vi "PrefDialog.vi"(8 "error in (no error)":errorcluster, 11 "MyPluginsBase in":refnum<class "NHRGridSim.lvclass">) -> (0 "error out":errorcluster, 1 "Save As":bool, 2 "Changed":bool, 3 "MyPluginsBase out":refnum<class "NHRGridSim.lvclass">)   [LabVIEW 2018, in "AcPwrPlugins.lvlib" / "NHRGridSim.lvclass"]
doc: "This VI opens up the modal preference dialog window and allows a user to configure the properties with new values, or keep the existing values from the last time the function was called. The user can also save the new values to a new file name and new type name using the save as button."
uses:
  NHRGridSim.lvclass
  C:/Program Files (x86)/National Instruments/LabVIEW 2018/user.lib/NIST/BaseClasses/BasePlugin_class/BasePlugin.lvclass
  C:/Users/Public/Projects/ICDAS/NistPluggableModules/AcPwr/AcPwrPlugins/AcPwrBaseClass/AcPwrBase.lvclass
  Measurements.ctl
  TypeDefs/MeasurementType.ctl
  TypeDefs/NHRGrid_Modes.ctl
  TypeDefs/Device(s)Settings.ctl
  TypeDefs/NHRGrid_InstrumentCluster_Tabs.ctl
  TypeDefs/NHRGrid_Configure_Tabs.ctl
  TypeDefs/NHRGrid_Ranges_Tabs.ctl
  TypeDefs/NHRGrid_SafetyTrips_Tabs.ctl
  TypeDefs/NHRGrid_SlewRates_Tabs.ctl
  TypeDefs/NHRGrid_Phases_Tabs.ctl
  TypeDefs/NHRGrid_UpdateSettings.ctl
  <userlib>/NIST/BaseClasses/BasePlugin_class/BasePlugin.lvclass/BasePlugin.ctl
  AcPwrBaseClass/AcPwrBase.lvclass/AcPwrBase.ctl
  TypeDefs/NHRGrid_ModeAdjust_Tabs.ctl
  <userlib>/NIST/BaseClasses/BasePlugin_class/Accessors/Read PluginIniFilePath.vi
  AcPwrBaseClass/Accessors/Read BaseConfig.vi
  AcPwrBaseClass/Accessors/Read BaseMeasurements.vi
  <userlib>/NIST/BaseClasses/BasePlugin_class/Accessors/Write PluginIniFilePath.vi
  <vilib>/Utility/config.llb/NI_LVConfig.lvlib
panel:
  in  "ModeVal":u8
  in  "ChassisTxt":string
  in  "Update":bool
  in  "Device(s)Settings":T1={"MeasName"="", "Instr1"={"Name"="", "Vout (V)"=0.0, "VType"="", "FreqOut (Hz)"=60.0, "Aperture (cycles)"=1, "Synchronization"=0, "Ranges"={"Voltage (V)"=0, "Current (A)"=1}, "Safety Trips"={"Vmin (V)"=0.0, "Vmin Time (s)"=-1.0, "Vmax (V)"=0.0, "Vmax Time (s)"=-1.0, "Imax Source (A)"=0.0, "I Src Time (s)"=-1.0, "Imax Sink (A)"=0.0, "I Snk Time (s)"=-1.0, "Pmax Source (W)"=0.0, "P Src Time (s)"=-1.0, "Pmax Sink (W)"=0.0, "P Snk Time (s)"=-1.0, "Abs Volt Peak"=0.0, "Enable Vpk"=FALSE, "Abs Curr Peak"=0.0, "Enable Ipk"=FALSE}, "Slew Rates"={"Voltage (V/s)"=866030.0, "Current (A/s)"=100000.0, "Power (W/s)"=3000000.0, "Frequency (Hz/s)"=500.0, "Phase Angle (Deg/s)"=50000.0}, "Phases"={"A-Volts (V)"=0.0, "B-Volts (V)"=0.0, "C-Volts (V)"=0.0, "A-Change at..."=0, "B-Angle (Deg)"=240, "C-Angle (Deg)"=120, "B-Change at..."=0, "C-Change at..."=0, "AngleTxt"="", "A-Wave Shape"=0, "B-Wave Shape"=0, "C-Wave Shape"=0}}, "Instr2"={"Name"="", "Vout (V)"=0.0, "VType"="", "FreqOut (Hz)"=60.0, "Aperture (cycles)"=1, "Synchronization"=0, "Ranges"={"Voltage (V)"=0, "Current (A)"=1}, "Safety Trips"={"Vmin (V)"=0.0, "Vmin Time (s)"=-1.0, "Vmax (V)"=0.0, "Vmax Time (s)"=-1.0, "Imax Source (A)"=0.0, "I Src Time (s)"=-1.0, "Imax Sink (A)"=0.0, "I Snk Time (s)"=-1.0, "Pmax Source (W)"=0.0, "P Src Time (s)"=-1.0, "Pmax Sink (W)"=0.0, "P Snk Time (s)"=-1.0, "Abs Volt Peak"=0.0, "Enable Vpk"=FALSE, "Abs Curr Peak"=0.0, "Enable Ipk"=FALSE}, "Slew Rates"={"Voltage (V/s)"=866030.0, "Current (A/s)"=100000.0, "Power (W/s)"=3000000.0, "Frequency (Hz/s)"=500.0, "Phase Angle (Deg/s)"=50000.0}, "Phases"={"A-Volts (V)"=0.0, "B-Volts (V)"=0.0, "C-Volts (V)"=0.0, "A-Change at..."=0, "B-Angle (Deg)"=240, "C-Angle (Deg)"=120, "B-Change at..."=0, "C-Change at..."=0, "AngleTxt"="", "A-Wave Shape"=0, "B-Wave Shape"=0, "C-Wave Shape"=0}}, "Instr3"={"Name"="", "Vout (V)"=0.0, "VType"="", "FreqOut (Hz)"=60.0, "Aperture (cycles)"=1, "Synchronization"=0, "Ranges"={"Voltage (V)"=0, "Current (A)"=1}, "Safety Trips"={"Vmin (V)"=0.0, "Vmin Time (s)"=-1.0, "Vmax (V)"=0.0, "Vmax Time (s)"=-1.0, "Imax Source (A)"=0.0, "I Src Time (s)"=-1.0, "Imax Sink (A)"=0.0, "I Snk Time (s)"=-1.0, "Pmax Source (W)"=0.0, "P Src Time (s)"=-1.0, "Pmax Sink (W)"=0.0, "P Snk Time (s)"=-1.0, "Abs Volt Peak"=0.0, "Enable Vpk"=FALSE, "Abs Curr Peak"=0.0, "Enable Ipk"=FALSE}, "Slew Rates"={"Voltage (V/s)"=866030.0, "Current (A/s)"=100000.0, "Power (W/s)"=3000000.0, "Frequency (Hz/s)"=500.0, "Phase Angle (Deg/s)"=50000.0}, "Phases"={"A-Volts (V)"=0.0, "B-Volts (V)"=0.0, "C-Volts (V)"=0.0, "A-Change at..."=0, "B-Angle (Deg)"=240, "C-Angle (Deg)"=120, "B-Change at..."=0, "C-Change at..."=0, "AngleTxt"="", "A-Wave Shape"=0, "B-Wave Shape"=0, "C-Wave Shape"=0}}, "Handle"="", "Reset"=FALSE, "Mode"=0, "ID Query"=FALSE, "Connected"=FALSE, "Chassis"=1, "VRangeVals1"=[], "SyncList1"=[], "Wave1A"=[], "Wave1B"=[], "Wave1C"=[], "SyncList2"=[], "SyncList3"=[], "VRangeVals3"=[], "VRangeVals2"=[], "CRangeVals1"=[], "CRangeVals3"=[], "CRangeVals2"=[], "TabPages"=[], "Wave2A"=[], "Wave2B"=[], "Wave2C"=[], "Wave3A"=[], "Wave3B"=[], "Wave3C"=[], "EnableCtrls"=[[1, 0, 0, 0, 0, 0, 0, 0, 0, 0, 0, 0, 0, 0, 0, 0, 0, 0], [1, 0, 0, 0, 0, 0, 0, 0, 0, 0, 0, 0, 0, 0, 0, 0, 0, 0], [1, 0, 0, 0, 0, 0, 0, 0, 0, 0, 0, 0, 0, 0, 0, 0, 0, 0]]} {"Chassis" min=1 max=8 step=1; "Mode" items=["3-Phase AC"=0, "AC"=1, "DC"=2, "AC - AC"=7, "AC - DC"=8, "DC - AC"=11, "DC - DC"=12, "2-Phase AC - AC"=5, "2-Phase AC - DC"=6, "AC - AC - AC"=3, "DC - DC - DC"=4, "AC - AC - DC"=9, "AC - DC - DC"=10, "AC - DC - AC"=13, "DC - AC - AC"=14, "DC - AC - DC"=15]; "Instr3"."Phases"."C-Wave Shape" items=["Sine", "User1", "User2", "User3"]; "Instr3"."Phases"."B-Wave Shape" items=["Sine", "User1", "User2", "User3"]; "Instr3"."Phases"."A-Wave Shape" items=["Sine", "User1", "User2", "User3"]; "Instr3"."Phases"."C-Change at..." min=0 max=359; "Instr3"."Phases"."B-Change at..." min=0 max=359; "Instr3"."Phases"."A-Change at..." min=0 max=359; "Instr3"."Phases"."C-Angle (Deg)" min=0 max=359; "Instr3"."Phases"."B-Angle (Deg)" min=0 max=359; "Instr3"."Phases"."C-Volts (V)" min=0.0 max=606.0; "Instr3"."Phases"."B-Volts (V)" min=0.0 max=606.0; "Instr3"."Phases"."A-Volts (V)" min=0.0 max=606.0; "Instr3"."Slew Rates"."Phase Angle (Deg/s)" min=0.1 max=50000.0; "Instr3"."Slew Rates"."Frequency (Hz/s)" min=0.01 max=500.0; "Instr3"."Slew Rates"."Power (W/s)" min=2.0 max=8000000.0; "Instr3"."Slew Rates"."Current (A/s)" min=0.2 max=2400000.0; "Instr3"."Slew Rates"."Voltage (V/s)" min=0.01 max=2000000.0; "Instr3"."Safety Trips"."Abs Curr Peak" min=0.0; "Instr3"."Safety Trips"."Abs Volt Peak" min=0.0; "Instr3"."Safety Trips"."P Snk Time (s)" min=-1.0 max=3600.0; "Instr3"."Safety Trips"."Pmax Sink (W)" min=0.0 max=436000.0 format="%#_7g"; "Instr3"."Safety Trips"."P Src Time (s)" min=-1.0 max=3600.0; "Instr3"."Safety Trips"."Pmax Source (W)" min=0.0 max=436000.0 format="%#_7g"; "Instr3"."Safety Trips"."I Snk Time (s)" min=-1.0 max=3600.0; "Instr3"."Safety Trips"."Imax Sink (A)" min=0.0 max=720.0; "Instr3"."Safety Trips"."I Src Time (s)" min=-1.0 max=3600.0; "Instr3"."Safety Trips"."Imax Source (A)" min=0.0 max=720.0; "Instr3"."Safety Trips"."Vmax Time (s)" min=-1.0 max=3600.0; "Instr3"."Safety Trips"."Vmax (V)" min=0.0 max=606.0; "Instr3"."Safety Trips"."Vmin Time (s)" min=-1.0 max=3600.0; "Instr3"."Safety Trips"."Vmin (V)" min=0.0 max=606.0; "Instr3"."Ranges"."Current (A)" items=["6", "30"]; "Instr3"."Ranges"."Voltage (V)" items=["303", "606"]; "Instr3"."Synchronization" items=["Immediate", "Sync to Phase A"]; "Instr3"."Aperture (cycles)" min=0 max=64; "Instr3"."FreqOut (Hz)" min=30.0 max=880.0; "Instr3"."Vout (V)" min=0.0 max=606.0; "Instr2"."Phases"."C-Wave Shape" items=["Sine", "User1", "User2", "User3"]; "Instr2"."Phases"."B-Wave Shape" items=["Sine", "User1", "User2", "User3"]; "Instr2"."Phases"."A-Wave Shape" items=["Sine", "User1", "User2", "User3"]; "Instr2"."Phases"."C-Change at..." min=0 max=359; "Instr2"."Phases"."B-Change at..." min=0 max=359; "Instr2"."Phases"."A-Change at..." min=0 max=359; "Instr2"."Phases"."C-Angle (Deg)" min=0 max=359; "Instr2"."Phases"."B-Angle (Deg)" min=0 max=359; "Instr2"."Phases"."C-Volts (V)" min=0.0 max=606.0; "Instr2"."Phases"."B-Volts (V)" min=0.0 max=606.0; "Instr2"."Phases"."A-Volts (V)" min=0.0 max=606.0; "Instr2"."Slew Rates"."Phase Angle (Deg/s)" min=0.1 max=50000.0; "Instr2"."Slew Rates"."Frequency (Hz/s)" min=0.01 max=500.0; "Instr2"."Slew Rates"."Power (W/s)" min=2.0 max=8000000.0; "Instr2"."Slew Rates"."Current (A/s)" min=0.2 max=2400000.0; "Instr2"."Slew Rates"."Voltage (V/s)" min=0.01 max=2000000.0; "Instr2"."Safety Trips"."Abs Curr Peak" min=0.0; "Instr2"."Safety Trips"."Abs Volt Peak" min=0.0; "Instr2"."Safety Trips"."P Snk Time (s)" min=-1.0 max=3600.0; "Instr2"."Safety Trips"."Pmax Sink (W)" min=0.0 max=436000.0 format="%#_7g"; "Instr2"."Safety Trips"."P Src Time (s)" min=-1.0 max=3600.0; "Instr2"."Safety Trips"."Pmax Source (W)" min=0.0 max=436000.0 format="%#_7g"; "Instr2"."Safety Trips"."I Snk Time (s)" min=-1.0 max=3600.0; "Instr2"."Safety Trips"."Imax Sink (A)" min=0.0 max=720.0; "Instr2"."Safety Trips"."I Src Time (s)" min=-1.0 max=3600.0; "Instr2"."Safety Trips"."Imax Source (A)" min=0.0 max=720.0; "Instr2"."Safety Trips"."Vmax Time (s)" min=-1.0 max=3600.0; "Instr2"."Safety Trips"."Vmax (V)" min=0.0 max=606.0; "Instr2"."Safety Trips"."Vmin Time (s)" min=-1.0 max=3600.0; "Instr2"."Safety Trips"."Vmin (V)" min=0.0 max=606.0; "Instr2"."Ranges"."Current (A)" items=["6", "30"]; "Instr2"."Ranges"."Voltage (V)" items=["303", "606"]; "Instr2"."Synchronization" items=["Immediate", "Sync to Phase A"]; "Instr2"."Aperture (cycles)" min=0 max=64; "Instr2"."FreqOut (Hz)" min=30.0 max=880.0; "Instr2"."Vout (V)" min=0.0 max=606.0; "Instr1"."Phases"."C-Wave Shape" items=["Sine", "User1", "User2", "User3"]; "Instr1"."Phases"."B-Wave Shape" items=["Sine", "User1", "User2", "User3"]; "Instr1"."Phases"."A-Wave Shape" items=["Sine", "User1", "User2", "User3"]; "Instr1"."Phases"."C-Change at..." min=0 max=359; "Instr1"."Phases"."B-Change at..." min=0 max=359; "Instr1"."Phases"."A-Change at..." min=0 max=359; "Instr1"."Phases"."C-Angle (Deg)" min=0 max=359; "Instr1"."Phases"."B-Angle (Deg)" min=0 max=359; "Instr1"."Phases"."C-Volts (V)" min=0.0 max=606.0; "Instr1"."Phases"."B-Volts (V)" min=0.0 max=606.0; "Instr1"."Phases"."A-Volts (V)" min=0.0 max=606.0; "Instr1"."Slew Rates"."Phase Angle (Deg/s)" min=0.1 max=50000.0; "Instr1"."Slew Rates"."Frequency (Hz/s)" min=0.01 max=500.0; "Instr1"."Slew Rates"."Power (W/s)" min=2.0 max=8000000.0; "Instr1"."Slew Rates"."Current (A/s)" min=0.2 max=2400000.0; "Instr1"."Slew Rates"."Voltage (V/s)" min=0.01 max=2000000.0; "Instr1"."Safety Trips"."Abs Curr Peak" min=0.0; "Instr1"."Safety Trips"."Abs Volt Peak" min=0.0; "Instr1"."Safety Trips"."P Snk Time (s)" min=-1.0 max=3600.0; "Instr1"."Safety Trips"."Pmax Sink (W)" min=0.0 max=436000.0 format="%#_7g"; "Instr1"."Safety Trips"."P Src Time (s)" min=-1.0 max=3600.0; "Instr1"."Safety Trips"."Pmax Source (W)" min=0.0 max=436000.0 format="%#_7g"; "Instr1"."Safety Trips"."I Snk Time (s)" min=-1.0 max=3600.0; "Instr1"."Safety Trips"."Imax Sink (A)" min=0.0 max=720.0; "Instr1"."Safety Trips"."I Src Time (s)" min=-1.0 max=3600.0; "Instr1"."Safety Trips"."Imax Source (A)" min=0.0 max=720.0; "Instr1"."Safety Trips"."Vmax Time (s)" min=-1.0 max=3600.0; "Instr1"."Safety Trips"."Vmax (V)" min=0.0 max=606.0; "Instr1"."Safety Trips"."Vmin Time (s)" min=-1.0 max=3600.0; "Instr1"."Safety Trips"."Vmin (V)" min=0.0 max=606.0; "Instr1"."Ranges"."Current (A)" items=["6", "30"]; "Instr1"."Ranges"."Voltage (V)" items=["303", "606"]; "Instr1"."Synchronization" items=["Immediate", "Sync to Phase A"]; "Instr1"."Aperture (cycles)" min=0 max=64; "Instr1"."FreqOut (Hz)" min=30.0 max=880.0; "Instr1"."Vout (V)" min=0.0 max=606.0}
  in  "Chassis":i32=1 min=1 max=8 step=1
  in  "MeasName":string
  out "Connected":bool
  in  "ID Query":bool
  in  "Mode":T8 items=["3-Phase AC"=0, "AC"=1, "DC"=2, "AC - AC"=7, "AC - DC"=8, "DC - AC"=11, "DC - DC"=12, "2-Phase AC - AC"=5, "2-Phase AC - DC"=6, "AC - AC - AC"=3, "DC - DC - DC"=4, "AC - AC - DC"=9, "AC - DC - DC"=10, "AC - DC - AC"=13, "DC - AC - AC"=14, "DC - AC - DC"=15]
  in  "Reset":bool
  in  "Handle":string
  in  "Instruments":enum32{"Page 1", "Page 2", "Page 3"}(tab)
  in  "Instr1":T2={"Name"="", "Vout (V)"=0.0, "VType"="", "FreqOut (Hz)"=60.0, "Aperture (cycles)"=1, "Synchronization"=0, "Ranges"={"Voltage (V)"=0, "Current (A)"=1}, "Safety Trips"={"Vmin (V)"=0.0, "Vmin Time (s)"=-1.0, "Vmax (V)"=0.0, "Vmax Time (s)"=-1.0, "Imax Source (A)"=0.0, "I Src Time (s)"=-1.0, "Imax Sink (A)"=0.0, "I Snk Time (s)"=-1.0, "Pmax Source (W)"=0.0, "P Src Time (s)"=-1.0, "Pmax Sink (W)"=0.0, "P Snk Time (s)"=-1.0, "Abs Volt Peak"=0.0, "Enable Vpk"=FALSE, "Abs Curr Peak"=0.0, "Enable Ipk"=FALSE}, "Slew Rates"={"Voltage (V/s)"=866030.0, "Current (A/s)"=100000.0, "Power (W/s)"=3000000.0, "Frequency (Hz/s)"=500.0, "Phase Angle (Deg/s)"=50000.0}, "Phases"={"A-Volts (V)"=0.0, "B-Volts (V)"=0.0, "C-Volts (V)"=0.0, "A-Change at..."=0, "B-Angle (Deg)"=240, "C-Angle (Deg)"=120, "B-Change at..."=0, "C-Change at..."=0, "AngleTxt"="", "A-Wave Shape"=0, "B-Wave Shape"=0, "C-Wave Shape"=0}} {"Phases"."C-Wave Shape" items=["Sine", "User1", "User2", "User3"]; "Phases"."B-Wave Shape" items=["Sine", "User1", "User2", "User3"]; "Phases"."A-Wave Shape" items=["Sine", "User1", "User2", "User3"]; "Phases"."C-Change at..." min=0 max=359; "Phases"."B-Change at..." min=0 max=359; "Phases"."A-Change at..." min=0 max=359; "Phases"."C-Angle (Deg)" min=0 max=359; "Phases"."B-Angle (Deg)" min=0 max=359; "Phases"."C-Volts (V)" min=0.0 max=606.0; "Phases"."B-Volts (V)" min=0.0 max=606.0; "Phases"."A-Volts (V)" min=0.0 max=606.0; "Slew Rates"."Phase Angle (Deg/s)" min=0.1 max=50000.0; "Slew Rates"."Frequency (Hz/s)" min=0.01 max=500.0; "Slew Rates"."Power (W/s)" min=2.0 max=8000000.0; "Slew Rates"."Current (A/s)" min=0.2 max=2400000.0; "Slew Rates"."Voltage (V/s)" min=0.01 max=2000000.0; "Safety Trips"."Abs Curr Peak" min=0.0; "Safety Trips"."Abs Volt Peak" min=0.0; "Safety Trips"."P Snk Time (s)" min=-1.0 max=3600.0; "Safety Trips"."Pmax Sink (W)" min=0.0 max=436000.0 format="%#_7g"; "Safety Trips"."P Src Time (s)" min=-1.0 max=3600.0; "Safety Trips"."Pmax Source (W)" min=0.0 max=436000.0 format="%#_7g"; "Safety Trips"."I Snk Time (s)" min=-1.0 max=3600.0; "Safety Trips"."Imax Sink (A)" min=0.0 max=720.0; "Safety Trips"."I Src Time (s)" min=-1.0 max=3600.0; "Safety Trips"."Imax Source (A)" min=0.0 max=720.0; "Safety Trips"."Vmax Time (s)" min=-1.0 max=3600.0; "Safety Trips"."Vmax (V)" min=0.0 max=606.0; "Safety Trips"."Vmin Time (s)" min=-1.0 max=3600.0; "Safety Trips"."Vmin (V)" min=0.0 max=606.0; "Ranges"."Current (A)" items=["6", "30"]; "Ranges"."Voltage (V)" items=["303", "606"]; "Synchronization" items=["Immediate", "Sync to Phase A"]; "Aperture (cycles)" min=0 max=64; "FreqOut (Hz)" min=30.0 max=880.0; "Vout (V)" min=0.0 max=606.0}
  in  "Instr2":T2={"Name"="", "Vout (V)"=0.0, "VType"="", "FreqOut (Hz)"=60.0, "Aperture (cycles)"=1, "Synchronization"=0, "Ranges"={"Voltage (V)"=0, "Current (A)"=1}, "Safety Trips"={"Vmin (V)"=0.0, "Vmin Time (s)"=-1.0, "Vmax (V)"=0.0, "Vmax Time (s)"=-1.0, "Imax Source (A)"=0.0, "I Src Time (s)"=-1.0, "Imax Sink (A)"=0.0, "I Snk Time (s)"=-1.0, "Pmax Source (W)"=0.0, "P Src Time (s)"=-1.0, "Pmax Sink (W)"=0.0, "P Snk Time (s)"=-1.0, "Abs Volt Peak"=0.0, "Enable Vpk"=FALSE, "Abs Curr Peak"=0.0, "Enable Ipk"=FALSE}, "Slew Rates"={"Voltage (V/s)"=866030.0, "Current (A/s)"=100000.0, "Power (W/s)"=3000000.0, "Frequency (Hz/s)"=500.0, "Phase Angle (Deg/s)"=50000.0}, "Phases"={"A-Volts (V)"=0.0, "B-Volts (V)"=0.0, "C-Volts (V)"=0.0, "A-Change at..."=0, "B-Angle (Deg)"=240, "C-Angle (Deg)"=120, "B-Change at..."=0, "C-Change at..."=0, "AngleTxt"="", "A-Wave Shape"=0, "B-Wave Shape"=0, "C-Wave Shape"=0}} {"Phases"."C-Wave Shape" items=["Sine", "User1", "User2", "User3"]; "Phases"."B-Wave Shape" items=["Sine", "User1", "User2", "User3"]; "Phases"."A-Wave Shape" items=["Sine", "User1", "User2", "User3"]; "Phases"."C-Change at..." min=0 max=359; "Phases"."B-Change at..." min=0 max=359; "Phases"."A-Change at..." min=0 max=359; "Phases"."C-Angle (Deg)" min=0 max=359; "Phases"."B-Angle (Deg)" min=0 max=359; "Phases"."C-Volts (V)" min=0.0 max=606.0; "Phases"."B-Volts (V)" min=0.0 max=606.0; "Phases"."A-Volts (V)" min=0.0 max=606.0; "Slew Rates"."Phase Angle (Deg/s)" min=0.1 max=50000.0; "Slew Rates"."Frequency (Hz/s)" min=0.01 max=500.0; "Slew Rates"."Power (W/s)" min=2.0 max=8000000.0; "Slew Rates"."Current (A/s)" min=0.2 max=2400000.0; "Slew Rates"."Voltage (V/s)" min=0.01 max=2000000.0; "Safety Trips"."Abs Curr Peak" min=0.0; "Safety Trips"."Abs Volt Peak" min=0.0; "Safety Trips"."P Snk Time (s)" min=-1.0 max=3600.0; "Safety Trips"."Pmax Sink (W)" min=0.0 max=436000.0 format="%#_7g"; "Safety Trips"."P Src Time (s)" min=-1.0 max=3600.0; "Safety Trips"."Pmax Source (W)" min=0.0 max=436000.0 format="%#_7g"; "Safety Trips"."I Snk Time (s)" min=-1.0 max=3600.0; "Safety Trips"."Imax Sink (A)" min=0.0 max=720.0; "Safety Trips"."I Src Time (s)" min=-1.0 max=3600.0; "Safety Trips"."Imax Source (A)" min=0.0 max=720.0; "Safety Trips"."Vmax Time (s)" min=-1.0 max=3600.0; "Safety Trips"."Vmax (V)" min=0.0 max=606.0; "Safety Trips"."Vmin Time (s)" min=-1.0 max=3600.0; "Safety Trips"."Vmin (V)" min=0.0 max=606.0; "Ranges"."Current (A)" items=["6", "30"]; "Ranges"."Voltage (V)" items=["303", "606"]; "Synchronization" items=["Immediate", "Sync to Phase A"]; "Aperture (cycles)" min=0 max=64; "FreqOut (Hz)" min=30.0 max=880.0; "Vout (V)" min=0.0 max=606.0}
  in  "Instr3":T2={"Name"="", "Vout (V)"=0.0, "VType"="", "FreqOut (Hz)"=60.0, "Aperture (cycles)"=1, "Synchronization"=0, "Ranges"={"Voltage (V)"=0, "Current (A)"=1}, "Safety Trips"={"Vmin (V)"=0.0, "Vmin Time (s)"=-1.0, "Vmax (V)"=0.0, "Vmax Time (s)"=-1.0, "Imax Source (A)"=0.0, "I Src Time (s)"=-1.0, "Imax Sink (A)"=0.0, "I Snk Time (s)"=-1.0, "Pmax Source (W)"=0.0, "P Src Time (s)"=-1.0, "Pmax Sink (W)"=0.0, "P Snk Time (s)"=-1.0, "Abs Volt Peak"=0.0, "Enable Vpk"=FALSE, "Abs Curr Peak"=0.0, "Enable Ipk"=FALSE}, "Slew Rates"={"Voltage (V/s)"=866030.0, "Current (A/s)"=100000.0, "Power (W/s)"=3000000.0, "Frequency (Hz/s)"=500.0, "Phase Angle (Deg/s)"=50000.0}, "Phases"={"A-Volts (V)"=0.0, "B-Volts (V)"=0.0, "C-Volts (V)"=0.0, "A-Change at..."=0, "B-Angle (Deg)"=240, "C-Angle (Deg)"=120, "B-Change at..."=0, "C-Change at..."=0, "AngleTxt"="", "A-Wave Shape"=0, "B-Wave Shape"=0, "C-Wave Shape"=0}} {"Phases"."C-Wave Shape" items=["Sine", "User1", "User2", "User3"]; "Phases"."B-Wave Shape" items=["Sine", "User1", "User2", "User3"]; "Phases"."A-Wave Shape" items=["Sine", "User1", "User2", "User3"]; "Phases"."C-Change at..." min=0 max=359; "Phases"."B-Change at..." min=0 max=359; "Phases"."A-Change at..." min=0 max=359; "Phases"."C-Angle (Deg)" min=0 max=359; "Phases"."B-Angle (Deg)" min=0 max=359; "Phases"."C-Volts (V)" min=0.0 max=606.0; "Phases"."B-Volts (V)" min=0.0 max=606.0; "Phases"."A-Volts (V)" min=0.0 max=606.0; "Slew Rates"."Phase Angle (Deg/s)" min=0.1 max=50000.0; "Slew Rates"."Frequency (Hz/s)" min=0.01 max=500.0; "Slew Rates"."Power (W/s)" min=2.0 max=8000000.0; "Slew Rates"."Current (A/s)" min=0.2 max=2400000.0; "Slew Rates"."Voltage (V/s)" min=0.01 max=2000000.0; "Safety Trips"."Abs Curr Peak" min=0.0; "Safety Trips"."Abs Volt Peak" min=0.0; "Safety Trips"."P Snk Time (s)" min=-1.0 max=3600.0; "Safety Trips"."Pmax Sink (W)" min=0.0 max=436000.0 format="%#_7g"; "Safety Trips"."P Src Time (s)" min=-1.0 max=3600.0; "Safety Trips"."Pmax Source (W)" min=0.0 max=436000.0 format="%#_7g"; "Safety Trips"."I Snk Time (s)" min=-1.0 max=3600.0; "Safety Trips"."Imax Sink (A)" min=0.0 max=720.0; "Safety Trips"."I Src Time (s)" min=-1.0 max=3600.0; "Safety Trips"."Imax Source (A)" min=0.0 max=720.0; "Safety Trips"."Vmax Time (s)" min=-1.0 max=3600.0; "Safety Trips"."Vmax (V)" min=0.0 max=606.0; "Safety Trips"."Vmin Time (s)" min=-1.0 max=3600.0; "Safety Trips"."Vmin (V)" min=0.0 max=606.0; "Ranges"."Current (A)" items=["6", "30"]; "Ranges"."Voltage (V)" items=["303", "606"]; "Synchronization" items=["Immediate", "Sync to Phase A"]; "Aperture (cycles)" min=0 max=64; "FreqOut (Hz)" min=30.0 max=880.0; "Vout (V)" min=0.0 max=606.0}
  in  "Measurements":T9 {"Instrument Number" items=["1", "2", "3"]}
  in  "btnSaveAs":bool
  in  "Measurement RefreshTime (ms)":u32
  in  "btnSave":bool
  in  "btnCancel":bool
  # "@ 12 kW each"
  # "Row = Instrument\nColumn: 0-Name, 1-FreqOut, 2-Sync, 3-AVolts, 4-BVolts, 5-CVolts, 6-BAngle, 7-CAngle, 8-AChange, 9-BChange, 10-CChange, 11-AWave, 12-BWave, 13-CWave, 14-SlewCurr, 15-SlewPower, 16-SlewFreq, 17-SlewPhase"
  # "0= Enabled, 1= Disabled, 2= Disabled and Greyed"
  # "Degrees with Respect to Phase A"
  # "Voltages (L-N)"
  # "Degrees for Synchronization"
  # "AC Phase Waveform"
  # "Degrees with Respect to Phase A"
  # "Voltages (L-N)"
  # "Degrees for Synchronization"
  # "AC Phase Waveform"
  # "Degrees with Respect to Phase A"
  # "Voltages (L-N)"
  # "Degrees for Synchronization"
  # "AC Phase Waveform"
  # "Degrees with Respect to Phase A"
  # "Voltages (L-N)"
  # "Degrees for Synchronization"
  # "AC Phase Waveform"
  # "Degrees with Respect to Phase A"
  # "Voltages (L-N)"
  # "Degrees for Synchronization"
  # "AC Phase Waveform"
  # "Degrees with Respect to Phase A"
  # "Voltages (L-N)"
  # "Degrees for Synchronization"
  # "AC Phase Waveform"
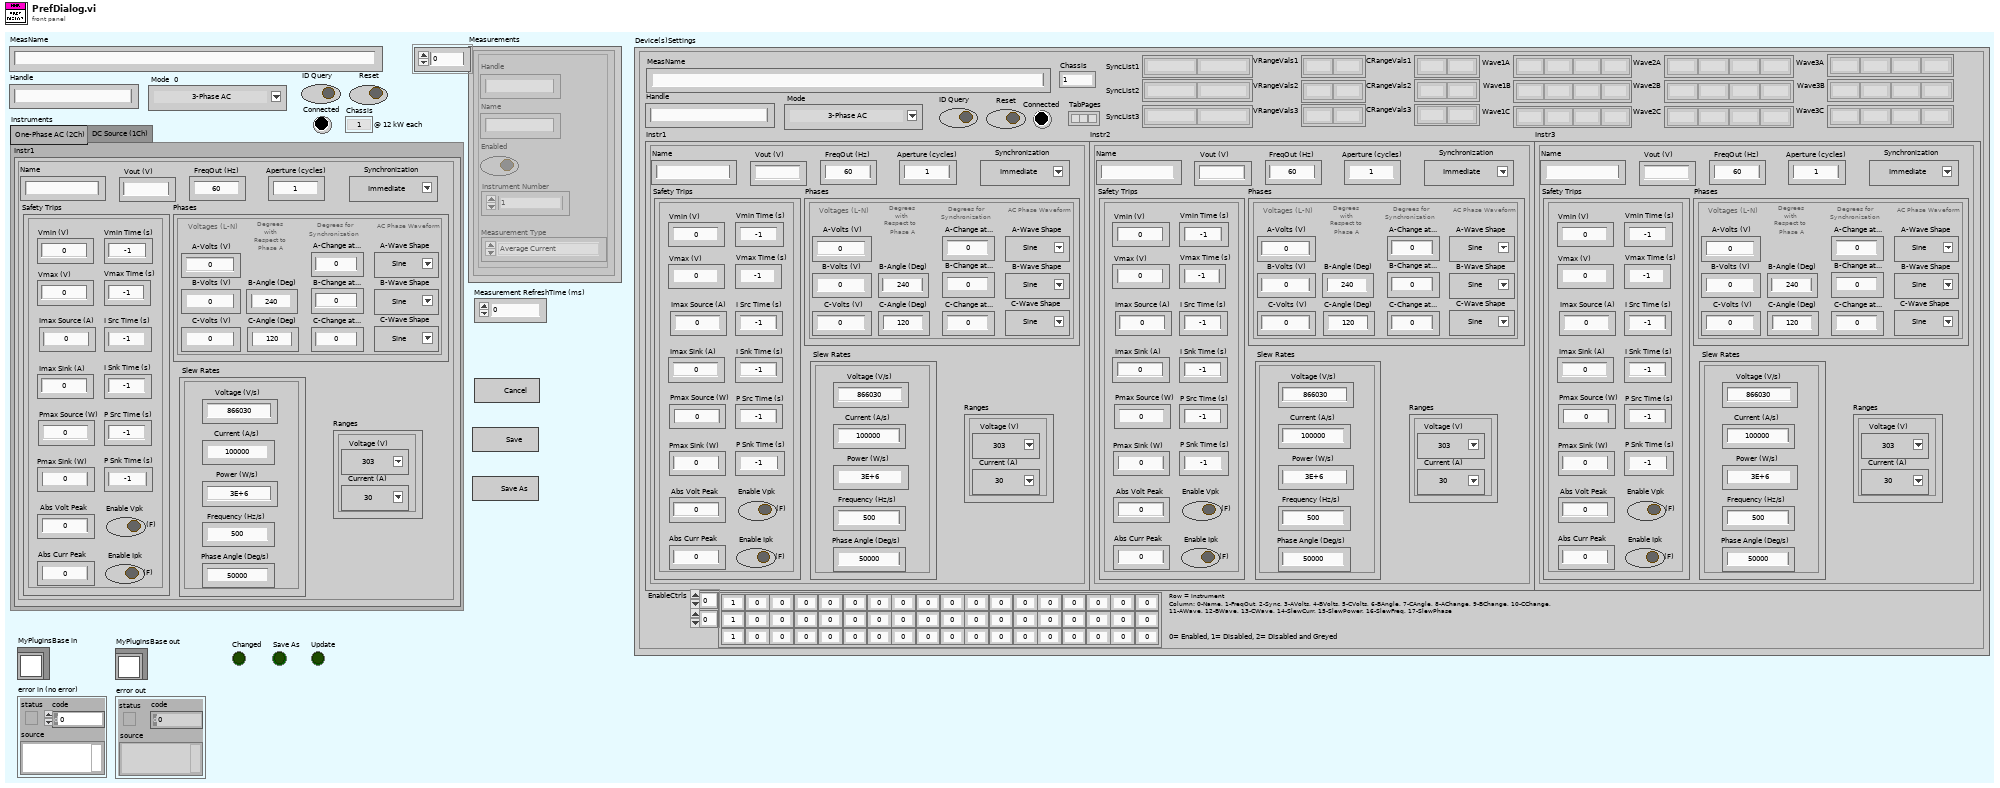
[diagram p1: front panel]
types:
  T1 = typedef "AcPwrPlugins.lvlib/NHRGridSim.lvclass/Device(s)Settings.ctl" = cluster{"MeasName":string, "Instr1":T2, "Instr2":T2, "Instr3":T2, "Handle":string, "Reset":bool, "Mode":T8, "ID Query":bool, "Connected":bool, "Chassis":i32, "VRangeVals1":string[], "SyncList1":string[], "Wave1A":string[], "Wave1B":string[], "Wave1C":string[], "SyncList2":string[], "SyncList3":string[], "VRangeVals3":string[], "VRangeVals2":string[], "CRangeVals1":string[], "CRangeVals3":string[], "CRangeVals2":string[], "TabPages":bool[], "Wave2A":string[], "Wave2B":string[], "Wave2C":string[], "Wave3A":string[], "Wave3B":string[], "Wave3C":string[], "EnableCtrls":i8[][]}
  T2 = typedef "AcPwrPlugins.lvlib/NHRGridSim.lvclass/NHRGrid_InstrumentCluster_Tabs.ctl" = cluster{"Name":string, "Vout (V)":dbl, "VType":string, "FreqOut (Hz)":dbl, "Aperture (cycles)":i32, "Synchronization":T3, "Ranges":T4, "Safety Trips":T5, "Slew Rates":T6, "Phases":T7}
  T3 = typedef "AcPwrPlugins.lvlib/NHRGridSim.lvclass/NHRGrid_Configure_Tabs.ctl" = u16
  T4 = typedef "AcPwrPlugins.lvlib/NHRGridSim.lvclass/NHRGrid_Ranges_Tabs.ctl" = cluster{"Voltage (V)":u16, "Current (A)":u16}
  T5 = typedef "AcPwrPlugins.lvlib/NHRGridSim.lvclass/NHRGrid_SafetyTrips_Tabs.ctl" = cluster{"Vmin (V)":dbl, "Vmin Time (s)":dbl, "Vmax (V)":dbl, "Vmax Time (s)":dbl, "Imax Source (A)":dbl, "I Src Time (s)":dbl, "Imax Sink (A)":dbl, "I Snk Time (s)":dbl, "Pmax Source (W)":dbl, "P Src Time (s)":dbl, "Pmax Sink (W)":dbl, "P Snk Time (s)":dbl, "Abs Volt Peak":dbl, "Enable Vpk":bool, "Abs Curr Peak":dbl, "Enable Ipk":bool}
  T6 = typedef "AcPwrPlugins.lvlib/NHRGridSim.lvclass/NHRGrid_SlewRates_Tabs.ctl" = cluster{"Voltage (V/s)":dbl, "Current (A/s)":dbl, "Power (W/s)":dbl, "Frequency (Hz/s)":dbl, "Phase Angle (Deg/s)":dbl}
  T7 = typedef "AcPwrPlugins.lvlib/NHRGridSim.lvclass/NHRGrid_Phases_Tabs.ctl" = cluster{"A-Volts (V)":dbl, "B-Volts (V)":dbl, "C-Volts (V)":dbl, "A-Change at...":i32, "B-Angle (Deg)":i32, "C-Angle (Deg)":i32, "B-Change at...":i32, "C-Change at...":i32, "AngleTxt":string, "A-Wave Shape":u16, "B-Wave Shape":u16, "C-Wave Shape":u16}
  T8 = typedef "AcPwrPlugins.lvlib/NHRGridSim.lvclass/NHRGrid_Modes.ctl" = u8
  T9 = typedef "AcPwrPlugins.lvlib/NHRGridSim.lvclass/Measurements.ctl" = cluster{"Handle":string, "Name":string, "Enabled ":bool, "Measurement Value":dbl, "Instrument Number ":i32, "Measurement Type ":T10}[]
  T10 = typedef "AcPwrPlugins.lvlib/NHRGridSim.lvclass/MeasurementType.ctl" = enum16{"Average Current", "Average Voltage"}
  T11 = enum32{"Invalid", "Default", "Floating", "Floating/Auto-Hide", "Modal"}
  T12 = enum32{"Invalid", "Standard", "Closed", "Hidden", "Minimized", "Maximized"}
  T13 = typedef "AcPwrPlugins.lvlib/NHRGridSim.lvclass/NHRGrid_UpdateSettings.ctl" = enum16{"VRanges", "CRanges", "Syncs", "Waves", "Load", "Tabs", "Values", "Waves1", "Waves2", "Waves3", "EnableNames", "EnableFreq", "EnableSync", "EnableVoltsA", "EnableVoltsB", "EnableVoltsC", "EnablePhaseB", "EnablePhaseC", "EnableChangeA", "EnableChangeB", "EnableChangeC", "EnableWavesA", "EnableWavesB", "EnableWavesC", "EnableCurrSlew", "EnablePowSlew", "EnableFreqSlew", "EnablePhaseSlew", "SaveEnables1", "SaveEnables2", "SaveEnables3", "SaveEnables4", "SaveEnables5", "SaveEnables6", "Array"}
  T14 = typedef "AcPwrPlugins.lvlib/NHRGridSim.lvclass/NHRGrid_ModeAdjust_Tabs.ctl" = enum16{"ShowTabs", "InstrNames", "VoltRanges", "ConfigSync", "Safety", "Phases", "FreqOut", "PhaseEnable", "ChangeEnable", "VoltsEnable", "Vtype", "Description", "CurrRanges", "VoutCoerce", "VSlewCoerce", "CSlewCoerce", "PSlewCoerce", "F&PhCoerce", "--- Available ---", "TripTCoerce1", "TripTCoerce2", "TripTCoerce3", "VPhaseCoerce", "WaveLists", "SetMode", "SetAperture", "Set V Slew", "Set I Slew", "Set F Slew", "Set P Slew", "Set Ang Slew", "SetVout", "WaveEnable", "SyncEnable", "SlewsCurr", "SlewsPow", "SlewsFreq", "SlewsPhase"}
  T15 = enum8{"Enabled", "Disabled", "Disabled and Grayed Out"}
  T16 = typedef "AcPwrPlugins.lvlib/AcPwrBase.lvclass/BaseConfig.ctl" = cluster{"Frequency":dbl, "FrequencyRange":dbl[], "Phases":T17[], "Name":string, "PluginConfigVariant":variant, "PluginMeasVariant":variant}
  T17 = typedef "AcPwrPlugins.lvlib/AcPwrBase.lvclass/Phase.ctl" = cluster{"Name":string, "Enabled":bool, "VoltageLevel":dbl, "Handle":string, "VoltageRange":dbl[], "Connected":bool, "CurrentLimit":dbl, "Waveform":string}
  T18 = typedef "AcPwrPlugins.lvlib/AcPwrBase.lvclass/BaseMeasurements.ctl" = cluster{"Handle":string, "Name":string, "Enabled":bool, "Measurement Value":dbl, "btnMeasFetch":bool, "Chroma Hold Peak Current Measurement":bool, "Chroma Measurement Type":T19, "Chroma Protection Status String":string, "NHRDC Fetch Method":i32, "NHRDC Fetch Time (s)":sgl, "NHRDC Measurement Type":i32, "NHRGridSim Measurement Type ":enum16{"Average Current", "Max Current", "Min Current", "Average Voltage", "Max Voltage", "Min Voltage", "Average True Power", "Max True Power", "Min True Power", "Average Apparent Power", "Max Apparent Power", "Min Apparent Power", "Power Factor", "Crest Factor"}, "NHRGridSim Phase ":i32, "PPS Measurement Type ":enum16{"Voltage RMS L-N", "Voltage RMS L-L", "Frequency", "Current RMS", "Current Peak", "Crest Factor", "Power Factor", "Power VA", "Real Power"}, "PPS Channel Name":enum16{"A", "B", "C"}}[]
  T19 = typedef "AcPwrPlugins.lvlib/ChromaAcLoad.lvclass/MeasurementType.ctl" = enum16{"Voltage (Vrms or V)", "Current (Arms or A)", "Power (W)", "Peak Voltage (V)", "Peak Current (A)", "Peak Power (W)", "Frequency (Hz)", "Resistance (Ohms)", "Voltage Overshoot (V)", "Positive Peak Current (A)", "Voltage Undershoot (V)", "Negative Peak Current (A)", "Apparent Power (VA)", "Reacitive Power (VAR)", "Voltage THD", "Power Factor", "Current's Crest Factor"}
  T20 = typedef "NI_LVConfig.lvlib/Config Data RefNum.ctl" = refnum<k1>
  T21 = enum8{"Enabled", "Disabled", "Disabled and Grayed Out"}[]
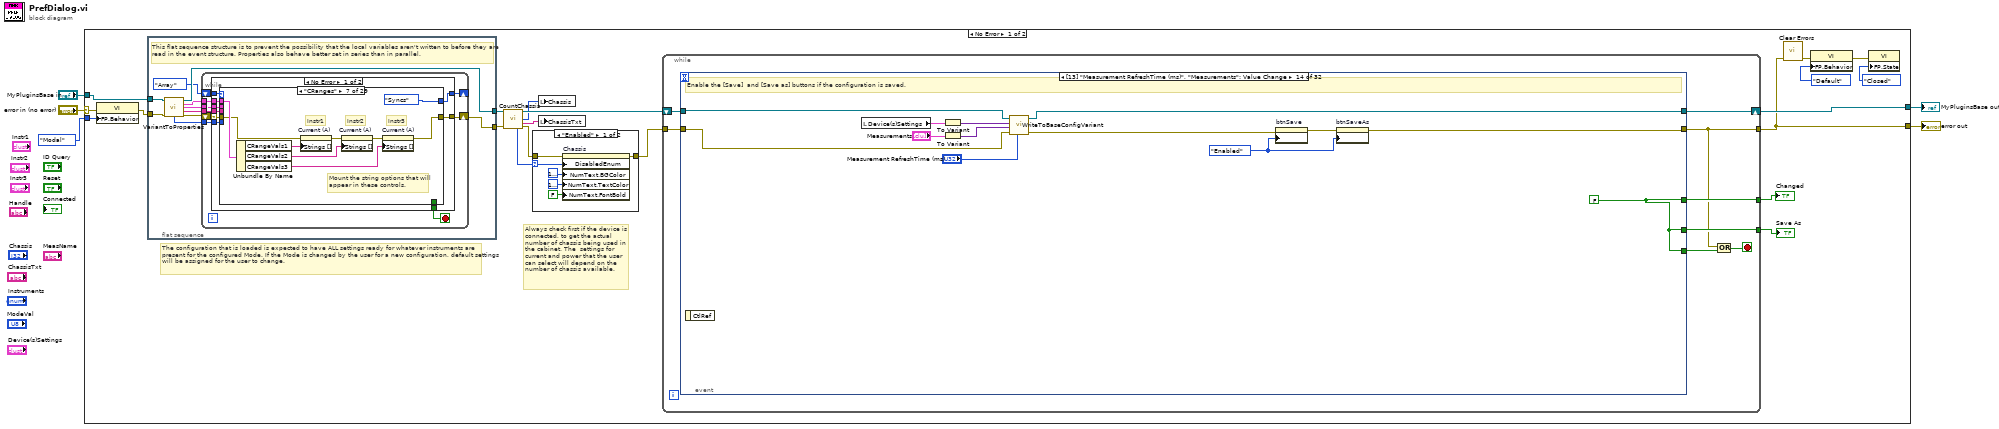
[diagram p0: block diagram]
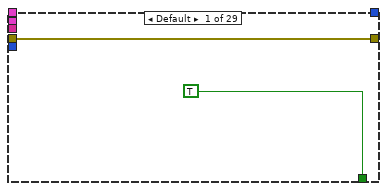
[diagram p2: hidden frame]
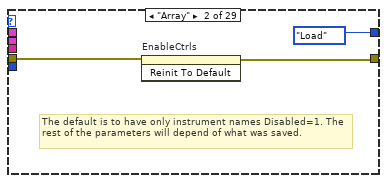
[diagram p3: hidden frame]
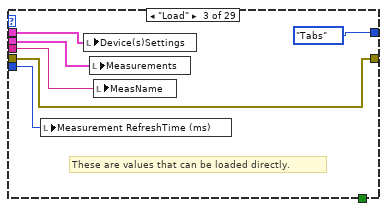
[diagram p4: hidden frame]
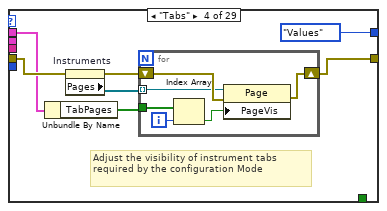
[diagram p5: hidden frame]
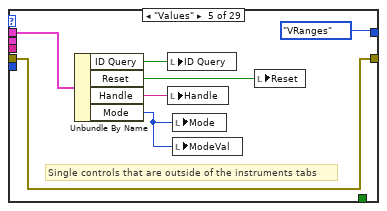
[diagram p6: hidden frame]
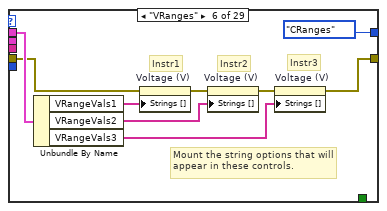
[diagram p7: hidden frame]
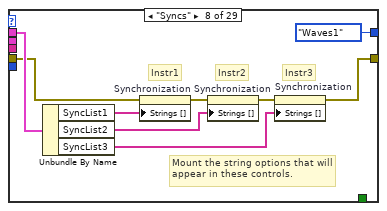
[diagram p8: hidden frame]
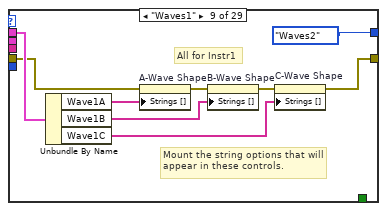
[diagram p9: hidden frame]
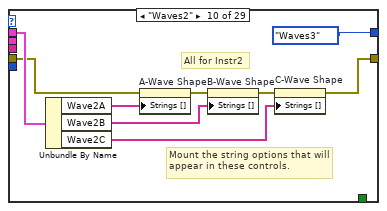
[diagram p10: hidden frame]
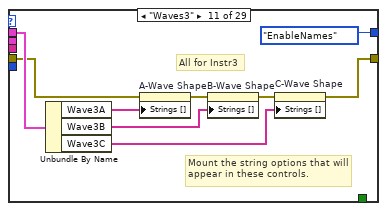
[diagram p11: hidden frame]
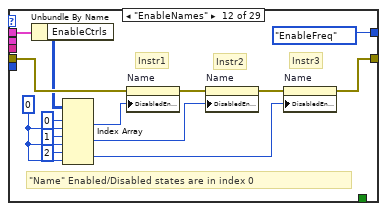
[diagram p12: hidden frame]
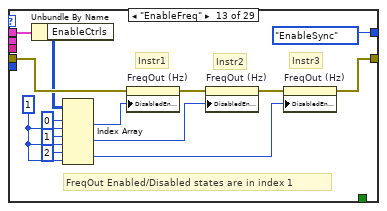
[diagram p13: hidden frame]
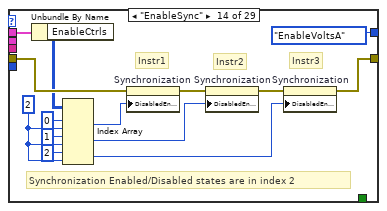
[diagram p14: hidden frame]
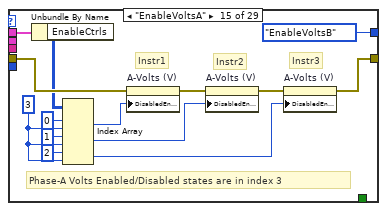
[diagram p15: hidden frame]
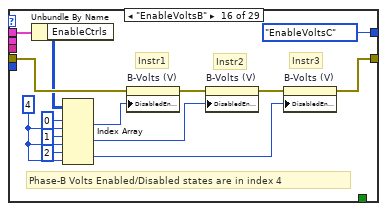
[diagram p16: hidden frame]
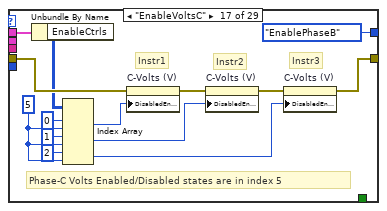
[diagram p17: hidden frame]
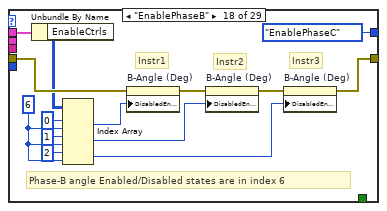
[diagram p18: hidden frame]
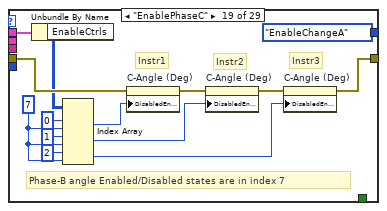
[diagram p19: hidden frame]
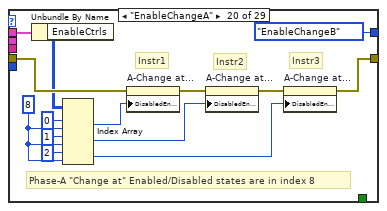
[diagram p20: hidden frame]
diagram:
  n1 = case shown="No Error" "error in (no error)" {
    selector: "error in (no error)" -> [w24 w3636]
    tunnel: "MyPluginsBase in" -> [w16 w3635]
    tunnel: [w20 w3635] -> w3
    tunnel: [w15 w3636] -> w2
    tunnel: T11."Modal" ("Front Panel Window:Behavior") -> [w18 _]
    frame No Error {
      # "The configuration that is loaded is expected to have ALL settings ready for whatever instruments are present for the configured Mode. If the Mode is changed by the user for a new configuration, default settings will be assigned for the user to change."
      # "Always check first if the device is connected, to get the actual number of chassis being used in the cabinet. The  settings for current and power that the user can select will depend on the number of chassis available."
      n2 = property class="VI"(error in=w24, "FP.Behavior"=w18) -> (error out=w17:errorcluster)  [unwired: 1 in, 1 out]
      n3 = flat-sequence {
        tunnel: [w35] -> w11
        tunnel: w17 -> [w34]
        tunnel: w16 -> [w33]
        tunnel: [w27] -> w6
        frame #0 {
          # "This flat sequence structure is to prevent the possibility that the local variables aren't written to before they are read in the event structure. Properties also behave better set in series than in parallel."
          n4 = call "VariantToProperties.vi"("NHRGridSim in"=w33, "error in (no error)"=w34) -> ("NHRGridSim out"=w35:refnum<class "NHRGridSim.lvclass">, "Device(s)Settings"=w32:T1, "Measurements"=w31:T9, "MeasName"=w29:string, "Measurement Refresh Time (ms)"=w30:u32, "error out"=w28:errorcluster)  [unwired: 8 in]
          n5 = while {
            tunnel: w32 -> [w43]
            tunnel: w31 -> [w42]
            tunnel: w30 -> [w41]
            tunnel: w29 -> [w40]
            shift-right: [w38] -> w27
            shift-left: w28 -> [w39]
            shift-right: [w37] -> _
            shift-left: NHRGrid_UpdateSettings."Array" -> [w44]
            stop <- w36 stop-if-true
            n6 = case shown="No Error" w39 {
              selector: w39 -> [w48 w391]
              tunnel: w44 -> [w53 w393]
              tunnel: w43 -> [w52 _]
              tunnel: w42 -> [w51 _]
              tunnel: w41 -> [w50 _]
              tunnel: w40 -> [w49 _]
              tunnel: [w47 w391] -> w38
              tunnel: [w46 w393] -> w37
              tunnel: [w45 TRUE] -> w36
              frame No Error {
                n7 = case shown="\"CRanges\"" w53 {
                  tunnel: w52 -> [_ _ w61 w67 w83 w92 w101 w111 w119 w128 w138 w152 w166 w180 w194 w208 w222 w236 w250 w264 w278 w292 w306 w320 w334 w348 w362 w376 w390]
                  tunnel: w51 -> [_ _ w63 _ _ _ _ _ _ _ _ _ _ _ _ _ _ _ _ _ _ _ _ _ _ _ _ _ _]
                  tunnel: w50 -> [_ _ w64 _ _ _ _ _ _ _ _ _ _ _ _ _ _ _ _ _ _ _ _ _ _ _ _ _ _]
                  tunnel: w49 -> [_ _ w62 _ _ _ _ _ _ _ _ _ _ _ _ _ _ _ _ _ _ _ _ _ _ _ _ _ _]
                  tunnel: w48 -> [w55 w57 w59 w68 w78 w88 w97 w107 w115 w124 w134 w151 w165 w179 w193 w207 w221 w235 w249 w263 w277 w291 w305 w319 w333 w347 w361 w375 w389]
                  tunnel: [_ NHRGrid_UpdateSettings."Load" NHRGrid_UpdateSettings."Tabs" NHRGrid_UpdateSettings."Values" NHRGrid_UpdateSettings."VRanges" NHRGrid_UpdateSettings."CRanges" NHRGrid_UpdateSettings."Syncs" NHRGrid_UpdateSettings."Waves1" NHRGrid_UpdateSettings."Waves2" NHRGrid_UpdateSettings."Waves3" NHRGrid_UpdateSettings."EnableNames" NHRGrid_UpdateSettings."EnableFreq" NHRGrid_UpdateSettings."EnableSync" NHRGrid_UpdateSettings."EnableVoltsA" NHRGrid_UpdateSettings."EnableVoltsB" NHRGrid_UpdateSettings."EnableVoltsC" NHRGrid_UpdateSettings."EnablePhaseB" NHRGrid_UpdateSettings."EnablePhaseC" NHRGrid_UpdateSettings."EnableChangeA" NHRGrid_UpdateSettings."EnableChangeB" NHRGrid_UpdateSettings."EnableChangeC" NHRGrid_UpdateSettings."EnableWavesA" NHRGrid_UpdateSettings."EnableWavesB" NHRGrid_UpdateSettings."EnableWavesC" NHRGrid_UpdateSettings."EnableCurrSlew" NHRGrid_UpdateSettings."EnablePowSlew" NHRGrid_UpdateSettings."EnableFreqSlew" NHRGrid_UpdateSettings."EnablePhaseSlew" _] -> w46
                  tunnel: [w55 w56 w59 w66 w78 w85 w94 w104 w112 w121 w131 w148 w162 w176 w190 w204 w218 w232 w246 w260 w274 w288 w302 w316 w330 w344 w358 w372 w386] -> w47
                  tunnel: [TRUE _ _ _ _ _ _ _ _ _ _ _ _ _ _ _ _ _ _ _ _ _ _ _ _ _ _ _ TRUE] -> w45
                  frame Default {
                  }
                  frame "Array" {
                    # "The default is to have only instrument names Disabled=1. The rest of the parameters will depend of what was saved."
                    n8 = invoke on="EnableCtrls" class="Arr (strict)" method="Reinit To Default"(error in=w57) -> (error out=w56:errorcluster)  [unwired: 2 in, 2 out]
                  }
                  frame "Load" {
                    # "These are values that can be loaded directly."
                    n9 = local write "Measurement RefreshTime (ms)"(w64) -> ()
                    n10 = local write "Device(s)Settings"(w61) -> ()
                    n11 = local write "Measurements"(w63) -> ()
                    n12 = local write "MeasName"(w62) -> ()
                  }
                  frame "Tabs" {
                    # "Adjust the visibility of instrument tabs required by the configuration Mode"
                    n13 = Unbundle By Name(w67) -> ("TabPages"=w71:bool[])
                    n14 = property on="Instruments" class="TabCtl (strict)"(error in=w68) -> (error out=w70:errorcluster, "Pages"=w69:refnum<vi>[])  [unwired: 1 in, 1 out]
                    n15 = for {
                      tunnel: w69 -> [w73] mode=indexing
                      tunnel: w71 -> [w76]
                      shift-right: [w72] -> w66
                      shift-left: w70 -> [w74]
                      i -> [w77]
                      n16 = Index Array(array=w76, index=w77) -> (element=w75:bool)
                      n17 = property class="Page"(reference=w73, error in=w74, "PageVis"=w75) -> (error out=w72:errorcluster)  [unwired: 1 out]
                    }
                  }
                  frame "Values" {
                    # "Single controls that are outside of the instruments tabs"
                    n18 = Unbundle By Name(w83) -> ("ID Query"=w82:bool, "Reset"=w81:bool, "Handle"=w80:string, "Mode"=w79:T8)
                    n19 = local write "ID Query"(w82) -> ()
                    n20 = local write "Handle"(w80) -> ()
                    n21 = local write "Mode"(w79) -> ()
                    n22 = local write "ModeVal"(w79) -> ()
                    n23 = local write "Reset"(w81) -> ()
                  }
                  frame "VRanges" {
                    # "Mount the string options that will appear in these controls."
                    # "Instr3"
                    # "Instr2"
                    # "Instr1"
                    n24 = Unbundle By Name(w92) -> ("VRangeVals1"=w91:string[], "VRangeVals2"=w90:string[], "VRangeVals3"=w89:string[])
                    n25 = property on="Voltage (V)" class="Ring (strict)"(error in=w88, "Strings []"=w91) -> (error out=w87:errorcluster)  [unwired: 1 in, 1 out]
                    n26 = property on="Voltage (V)" class="Ring (strict)"(error in=w87, "Strings []"=w90) -> (error out=w86:errorcluster)  [unwired: 1 in, 1 out]
                    n27 = property on="Voltage (V)" class="Ring (strict)"(error in=w86, "Strings []"=w89) -> (error out=w85:errorcluster)  [unwired: 1 in, 1 out]
                  }
                  frame "CRanges" {
                    # "Mount the string options that will appear in these controls."
                    # "Instr3"
                    # "Instr2"
                    # "Instr1"
                    n28 = Unbundle By Name(w101) -> ("CRangeVals1"=w100:string[], "CRangeVals2"=w99:string[], "CRangeVals3"=w98:string[])
                    n29 = property on="Current (A)" class="Ring (strict)"(error in=w97, "Strings []"=w100) -> (error out=w96:errorcluster)  [unwired: 1 in, 1 out]
                    n30 = property on="Current (A)" class="Ring (strict)"(error in=w96, "Strings []"=w99) -> (error out=w95:errorcluster)  [unwired: 1 in, 1 out]
                    n31 = property on="Current (A)" class="Ring (strict)"(error in=w95, "Strings []"=w98) -> (error out=w94:errorcluster)  [unwired: 1 in, 1 out]
                  }
                  frame "Syncs" {
                    # "Mount the string options that will appear in these controls."
                    # "Instr3"
                    # "Instr2"
                    # "Instr1"
                    n32 = Unbundle By Name(w111) -> ("SyncList1"=w110:string[], "SyncList2"=w109:string[], "SyncList3"=w108:string[])
                    n33 = property on="Synchronization" class="Ring (strict)"(error in=w107, "Strings []"=w110) -> (error out=w106:errorcluster)  [unwired: 1 in, 1 out]
                    n34 = property on="Synchronization" class="Ring (strict)"(error in=w106, "Strings []"=w109) -> (error out=w105:errorcluster)  [unwired: 1 in, 1 out]
                    n35 = property on="Synchronization" class="Ring (strict)"(error in=w105, "Strings []"=w108) -> (error out=w104:errorcluster)  [unwired: 1 in, 1 out]
                  }
                  frame "Waves1" {
                    # "All for Instr1"
                    # "Mount the string options that will appear in these controls."
                    n36 = Unbundle By Name(w119) -> ("Wave1A"=w118:string[], "Wave1B"=w117:string[], "Wave1C"=w116:string[])
                    n37 = property on="A-Wave Shape" class="Ring (strict)"(error in=w115, "Strings []"=w118) -> (error out=w114:errorcluster)  [unwired: 1 in, 1 out]
                    n38 = property on="B-Wave Shape" class="Ring (strict)"(error in=w114, "Strings []"=w117) -> (error out=w113:errorcluster)  [unwired: 1 in, 1 out]
                    n39 = property on="C-Wave Shape" class="Ring (strict)"(error in=w113, "Strings []"=w116) -> (error out=w112:errorcluster)  [unwired: 1 in, 1 out]
                  }
                  frame "Waves2" {
                    # "Mount the string options that will appear in these controls."
                    # "All for Instr2"
                    n40 = Unbundle By Name(w128) -> ("Wave2A"=w127:string[], "Wave2B"=w126:string[], "Wave2C"=w125:string[])
                    n41 = property on="A-Wave Shape" class="Ring (strict)"(error in=w124, "Strings []"=w127) -> (error out=w123:errorcluster)  [unwired: 1 in, 1 out]
                    n42 = property on="B-Wave Shape" class="Ring (strict)"(error in=w123, "Strings []"=w126) -> (error out=w122:errorcluster)  [unwired: 1 in, 1 out]
                    n43 = property on="C-Wave Shape" class="Ring (strict)"(error in=w122, "Strings []"=w125) -> (error out=w121:errorcluster)  [unwired: 1 in, 1 out]
                  }
                  frame "Waves3" {
                    # "Mount the string options that will appear in these controls."
                    # "All for Instr3"
                    n44 = Unbundle By Name(w138) -> ("Wave3A"=w137:string[], "Wave3B"=w136:string[], "Wave3C"=w135:string[])
                    n45 = property on="A-Wave Shape" class="Ring (strict)"(error in=w134, "Strings []"=w137) -> (error out=w133:errorcluster)  [unwired: 1 in, 1 out]
                    n46 = property on="B-Wave Shape" class="Ring (strict)"(error in=w133, "Strings []"=w136) -> (error out=w132:errorcluster)  [unwired: 1 in, 1 out]
                    n47 = property on="C-Wave Shape" class="Ring (strict)"(error in=w132, "Strings []"=w135) -> (error out=w131:errorcluster)  [unwired: 1 in, 1 out]
                  }
                  frame "EnableNames" {
                    w145 = 0 ("disabled index (col)")
                    # "Instr3"
                    # "Instr2"
                    # "Instr1"
                    # "\"Name\" Enabled/Disabled states are in index 0"
                    n48 = Unbundle By Name(w152) -> ("EnableCtrls"=w146:i8[][])
                    n49 = Index Array(array=w146, index (row) #1=0 ("disabled index (row)"), index (col) #1=w145, index (row) #2=1 ("disabled index (row)"), index (col) #2=w145, index (row) #3=2 ("disabled index (row)"), index (col) #3=w145) -> (element #1=w144:i8, element #2=w140:i8, element #3=w139:i8)
                    n50 = property on="Name" class="Str"(error in=w151, "DisabledEnum"=w144) -> (error out=w150:errorcluster)  [unwired: 1 in, 1 out]
                    n51 = property on="Name" class="Str"(error in=w150, "DisabledEnum"=w140) -> (error out=w149:errorcluster)  [unwired: 1 in, 1 out]
                    n52 = property on="Name" class="Str"(error in=w149, "DisabledEnum"=w139) -> (error out=w148:errorcluster)  [unwired: 1 in, 1 out]
                  }
                  frame "EnableFreq" {
                    w159 = 1 ("disabled index (col)")
                    # "Instr3"
                    # "Instr2"
                    # "Instr1"
                    # "FreqOut Enabled/Disabled states are in index 1"
                    n53 = Unbundle By Name(w166) -> ("EnableCtrls"=w160:i8[][])
                    n54 = Index Array(array=w160, index (row) #1=0 ("disabled index (row)"), index (col) #1=w159, index (row) #2=1 ("disabled index (row)"), index (col) #2=w159, index (row) #3=2 ("disabled index (row)"), index (col) #3=w159) -> (element #1=w158:i8, element #2=w154:i8, element #3=w153:i8)
                    n55 = property on="FreqOut (Hz)" class="DigNum (strict)"(error in=w165, "DisabledEnum"=w158) -> (error out=w164:errorcluster)  [unwired: 1 in, 1 out]
                    n56 = property on="FreqOut (Hz)" class="DigNum (strict)"(error in=w164, "DisabledEnum"=w154) -> (error out=w163:errorcluster)  [unwired: 1 in, 1 out]
                    n57 = property on="FreqOut (Hz)" class="DigNum (strict)"(error in=w163, "DisabledEnum"=w153) -> (error out=w162:errorcluster)  [unwired: 1 in, 1 out]
                  }
                  frame "EnableSync" {
                    w173 = 2 ("disabled index (col)")
                    # "Instr3"
                    # "Instr2"
                    # "Instr1"
                    # "Synchronization Enabled/Disabled states are in index 2"
                    n58 = Unbundle By Name(w180) -> ("EnableCtrls"=w174:i8[][])
                    n59 = Index Array(array=w174, index (row) #1=0 ("disabled index (row)"), index (col) #1=w173, index (row) #2=1 ("disabled index (row)"), index (col) #2=w173, index (row) #3=2 ("disabled index (row)"), index (col) #3=w173) -> (element #1=w172:i8, element #2=w168:i8, element #3=w167:i8)
                    n60 = property on="Synchronization" class="Ring (strict)"(error in=w179, "DisabledEnum"=w172) -> (error out=w178:errorcluster)  [unwired: 1 in, 1 out]
                    n61 = property on="Synchronization" class="Ring (strict)"(error in=w178, "DisabledEnum"=w168) -> (error out=w177:errorcluster)  [unwired: 1 in, 1 out]
                    n62 = property on="Synchronization" class="Ring (strict)"(error in=w177, "DisabledEnum"=w167) -> (error out=w176:errorcluster)  [unwired: 1 in, 1 out]
                  }
                  frame "EnableVoltsA" {
                    w188 = 3 ("disabled index (col)")
                    # "Instr3"
                    # "Instr2"
                    # "Instr1"
                    # "Phase-A Volts Enabled/Disabled states are in index 3"
                    n63 = Unbundle By Name(w194) -> ("EnableCtrls"=w189:i8[][])
                    n64 = Index Array(array=w189, index (row) #1=0 ("disabled index (row)"), index (col) #1=w188, index (row) #2=1 ("disabled index (row)"), index (col) #2=w188, index (row) #3=2 ("disabled index (row)"), index (col) #3=w188) -> (element #1=w187:i8, element #2=w183:i8, element #3=w182:i8)
                    n65 = property on="A-Volts (V)" class="DigNum (strict)"(error in=w193, "DisabledEnum"=w187) -> (error out=w192:errorcluster)  [unwired: 1 in, 1 out]
                    n66 = property on="A-Volts (V)" class="DigNum (strict)"(error in=w192, "DisabledEnum"=w183) -> (error out=w191:errorcluster)  [unwired: 1 in, 1 out]
                    n67 = property on="A-Volts (V)" class="DigNum (strict)"(error in=w191, "DisabledEnum"=w182) -> (error out=w190:errorcluster)  [unwired: 1 in, 1 out]
                  }
                  frame "EnableVoltsB" {
                    w202 = 4 ("disabled index (col)")
                    # "Instr3"
                    # "Instr2"
                    # "Instr1"
                    # "Phase-B Volts Enabled/Disabled states are in index 4"
                    n68 = Unbundle By Name(w208) -> ("EnableCtrls"=w203:i8[][])
                    n69 = Index Array(array=w203, index (row) #1=0 ("disabled index (row)"), index (col) #1=w202, index (row) #2=1 ("disabled index (row)"), index (col) #2=w202, index (row) #3=2 ("disabled index (row)"), index (col) #3=w202) -> (element #1=w201:i8, element #2=w197:i8, element #3=w196:i8)
                    n70 = property on="B-Volts (V)" class="DigNum (strict)"(error in=w207, "DisabledEnum"=w201) -> (error out=w206:errorcluster)  [unwired: 1 in, 1 out]
                    n71 = property on="B-Volts (V)" class="DigNum (strict)"(error in=w206, "DisabledEnum"=w197) -> (error out=w205:errorcluster)  [unwired: 1 in, 1 out]
                    n72 = property on="B-Volts (V)" class="DigNum (strict)"(error in=w205, "DisabledEnum"=w196) -> (error out=w204:errorcluster)  [unwired: 1 in, 1 out]
                  }
                  frame "EnableVoltsC" {
                    w216 = 5 ("disabled index (col)")
                    # "Instr3"
                    # "Instr2"
                    # "Instr1"
                    # "Phase-C Volts Enabled/Disabled states are in index 5"
                    n73 = Unbundle By Name(w222) -> ("EnableCtrls"=w217:i8[][])
                    n74 = Index Array(array=w217, index (row) #1=0 ("disabled index (row)"), index (col) #1=w216, index (row) #2=1 ("disabled index (row)"), index (col) #2=w216, index (row) #3=2 ("disabled index (row)"), index (col) #3=w216) -> (element #1=w215:i8, element #2=w211:i8, element #3=w210:i8)
                    n75 = property on="C-Volts (V)" class="DigNum (strict)"(error in=w221, "DisabledEnum"=w215) -> (error out=w220:errorcluster)  [unwired: 1 in, 1 out]
                    n76 = property on="C-Volts (V)" class="DigNum (strict)"(error in=w220, "DisabledEnum"=w211) -> (error out=w219:errorcluster)  [unwired: 1 in, 1 out]
                    n77 = property on="C-Volts (V)" class="DigNum (strict)"(error in=w219, "DisabledEnum"=w210) -> (error out=w218:errorcluster)  [unwired: 1 in, 1 out]
                  }
                  frame "EnablePhaseB" {
                    w230 = 6 ("disabled index (col)")
                    # "Instr3"
                    # "Instr2"
                    # "Instr1"
                    # "Phase-B angle Enabled/Disabled states are in index 6"
                    n78 = Unbundle By Name(w236) -> ("EnableCtrls"=w231:i8[][])
                    n79 = Index Array(array=w231, index (row) #1=0 ("disabled index (row)"), index (col) #1=w230, index (row) #2=1 ("disabled index (row)"), index (col) #2=w230, index (row) #3=2 ("disabled index (row)"), index (col) #3=w230) -> (element #1=w229:i8, element #2=w225:i8, element #3=w224:i8)
                    n80 = property on="B-Angle (Deg)" class="DigNum (strict)"(error in=w235, "DisabledEnum"=w229) -> (error out=w234:errorcluster)  [unwired: 1 in, 1 out]
                    n81 = property on="B-Angle (Deg)" class="DigNum (strict)"(error in=w234, "DisabledEnum"=w225) -> (error out=w233:errorcluster)  [unwired: 1 in, 1 out]
                    n82 = property on="B-Angle (Deg)" class="DigNum (strict)"(error in=w233, "DisabledEnum"=w224) -> (error out=w232:errorcluster)  [unwired: 1 in, 1 out]
                  }
                  frame "EnablePhaseC" {
                    w244 = 7 ("disabled index (col)")
                    # "Instr3"
                    # "Instr2"
                    # "Instr1"
                    # "Phase-B angle Enabled/Disabled states are in index 7"
                    n83 = Unbundle By Name(w250) -> ("EnableCtrls"=w245:i8[][])
                    n84 = Index Array(array=w245, index (row) #1=0 ("disabled index (row)"), index (col) #1=w244, index (row) #2=1 ("disabled index (row)"), index (col) #2=w244, index (row) #3=2 ("disabled index (row)"), index (col) #3=w244) -> (element #1=w243:i8, element #2=w239:i8, element #3=w238:i8)
                    n85 = property on="C-Angle (Deg)" class="DigNum (strict)"(error in=w249, "DisabledEnum"=w243) -> (error out=w248:errorcluster)  [unwired: 1 in, 1 out]
                    n86 = property on="C-Angle (Deg)" class="DigNum (strict)"(error in=w248, "DisabledEnum"=w239) -> (error out=w247:errorcluster)  [unwired: 1 in, 1 out]
                    n87 = property on="C-Angle (Deg)" class="DigNum (strict)"(error in=w247, "DisabledEnum"=w238) -> (error out=w246:errorcluster)  [unwired: 1 in, 1 out]
                  }
                  frame "EnableChangeA" {
                    w258 = 8 ("disabled index (col)")
                    # "Instr3"
                    # "Instr2"
                    # "Instr1"
                    # "Phase-A \"Change at\" Enabled/Disabled states are in index 8"
                    n88 = Unbundle By Name(w264) -> ("EnableCtrls"=w259:i8[][])
                    n89 = Index Array(array=w259, index (row) #1=0 ("disabled index (row)"), index (col) #1=w258, index (row) #2=1 ("disabled index (row)"), index (col) #2=w258, index (row) #3=2 ("disabled index (row)"), index (col) #3=w258) -> (element #1=w257:i8, element #2=w253:i8, element #3=w252:i8)
                    n90 = property on="A-Change at..." class="DigNum (strict)"(error in=w263, "DisabledEnum"=w257) -> (error out=w262:errorcluster)  [unwired: 1 in, 1 out]
                    n91 = property on="A-Change at..." class="DigNum (strict)"(error in=w262, "DisabledEnum"=w253) -> (error out=w261:errorcluster)  [unwired: 1 in, 1 out]
                    n92 = property on="A-Change at..." class="DigNum (strict)"(error in=w261, "DisabledEnum"=w252) -> (error out=w260:errorcluster)  [unwired: 1 in, 1 out]
                  }
                  frame "EnableChangeB" {
                    w272 = 9 ("disabled index (col)")
                    # "Instr3"
                    # "Instr2"
                    # "Instr1"
                    # "Phase-B \"Change at\" Enabled/Disabled states are in index 9"
                    n93 = Unbundle By Name(w278) -> ("EnableCtrls"=w273:i8[][])
                    n94 = Index Array(array=w273, index (row) #1=0 ("disabled index (row)"), index (col) #1=w272, index (row) #2=1 ("disabled index (row)"), index (col) #2=w272, index (row) #3=2 ("disabled index (row)"), index (col) #3=w272) -> (element #1=w271:i8, element #2=w267:i8, element #3=w266:i8)
                    n95 = property on="B-Change at..." class="DigNum (strict)"(error in=w277, "DisabledEnum"=w271) -> (error out=w276:errorcluster)  [unwired: 1 in, 1 out]
                    n96 = property on="B-Change at..." class="DigNum (strict)"(error in=w276, "DisabledEnum"=w267) -> (error out=w275:errorcluster)  [unwired: 1 in, 1 out]
                    n97 = property on="B-Change at..." class="DigNum (strict)"(error in=w275, "DisabledEnum"=w266) -> (error out=w274:errorcluster)  [unwired: 1 in, 1 out]
                  }
                  frame "EnableChangeC" {
                    w286 = 10 ("disabled index (col)")
                    # "Instr3"
                    # "Instr2"
                    # "Instr1"
                    # "Phase-C \"Change at\" Enabled/Disabled states are in index 10"
                    n98 = Unbundle By Name(w292) -> ("EnableCtrls"=w287:i8[][])
                    n99 = Index Array(array=w287, index (row) #1=0 ("disabled index (row)"), index (col) #1=w286, index (row) #2=1 ("disabled index (row)"), index (col) #2=w286, index (row) #3=2 ("disabled index (row)"), index (col) #3=w286) -> (element #1=w285:i8, element #2=w281:i8, element #3=w280:i8)
                    n100 = property on="C-Change at..." class="DigNum (strict)"(error in=w291, "DisabledEnum"=w285) -> (error out=w290:errorcluster)  [unwired: 1 in, 1 out]
                    n101 = property on="C-Change at..." class="DigNum (strict)"(error in=w290, "DisabledEnum"=w281) -> (error out=w289:errorcluster)  [unwired: 1 in, 1 out]
                    n102 = property on="C-Change at..." class="DigNum (strict)"(error in=w289, "DisabledEnum"=w280) -> (error out=w288:errorcluster)  [unwired: 1 in, 1 out]
                  }
                  frame "EnableWavesA" {
                    w300 = 11 ("disabled index (col)")
                    # "Instr3"
                    # "Instr2"
                    # "Instr1"
                    # "Phase-A waves Enabled/Disabled states are in index 11"
                    n103 = Unbundle By Name(w306) -> ("EnableCtrls"=w301:i8[][])
                    n104 = Index Array(array=w301, index (row) #1=0 ("disabled index (row)"), index (col) #1=w300, index (row) #2=1 ("disabled index (row)"), index (col) #2=w300, index (row) #3=2 ("disabled index (row)"), index (col) #3=w300) -> (element #1=w299:i8, element #2=w295:i8, element #3=w294:i8)
                    n105 = property on="A-Wave Shape" class="Ring (strict)"(error in=w305, "DisabledEnum"=w299) -> (error out=w304:errorcluster)  [unwired: 1 in, 1 out]
                    n106 = property on="A-Wave Shape" class="Ring (strict)"(error in=w304, "DisabledEnum"=w295) -> (error out=w303:errorcluster)  [unwired: 1 in, 1 out]
                    n107 = property on="A-Wave Shape" class="Ring (strict)"(error in=w303, "DisabledEnum"=w294) -> (error out=w302:errorcluster)  [unwired: 1 in, 1 out]
                  }
                  frame "EnableWavesB" {
                    w314 = 12 ("disabled index (col)")
                    # "Instr3"
                    # "Instr2"
                    # "Instr1"
                    # "Phase-B waves Enabled/Disabled states are in index 12"
                    n108 = Unbundle By Name(w320) -> ("EnableCtrls"=w315:i8[][])
                    n109 = Index Array(array=w315, index (row) #1=0 ("disabled index (row)"), index (col) #1=w314, index (row) #2=1 ("disabled index (row)"), index (col) #2=w314, index (row) #3=2 ("disabled index (row)"), index (col) #3=w314) -> (element #1=w313:i8, element #2=w309:i8, element #3=w308:i8)
                    n110 = property on="B-Wave Shape" class="Ring (strict)"(error in=w319, "DisabledEnum"=w313) -> (error out=w318:errorcluster)  [unwired: 1 in, 1 out]
                    n111 = property on="B-Wave Shape" class="Ring (strict)"(error in=w318, "DisabledEnum"=w309) -> (error out=w317:errorcluster)  [unwired: 1 in, 1 out]
                    n112 = property on="B-Wave Shape" class="Ring (strict)"(error in=w317, "DisabledEnum"=w308) -> (error out=w316:errorcluster)  [unwired: 1 in, 1 out]
                  }
                  frame "EnableWavesC" {
                    w328 = 13 ("disabled index (col)")
                    # "Instr3"
                    # "Instr2"
                    # "Instr1"
                    # "Phase-C waves Enabled/Disabled states are in index 13"
                    n113 = Unbundle By Name(w334) -> ("EnableCtrls"=w329:i8[][])
                    n114 = Index Array(array=w329, index (row) #1=0 ("disabled index (row)"), index (col) #1=w328, index (row) #2=1 ("disabled index (row)"), index (col) #2=w328, index (row) #3=2 ("disabled index (row)"), index (col) #3=w328) -> (element #1=w327:i8, element #2=w323:i8, element #3=w322:i8)
                    n115 = property on="C-Wave Shape" class="Ring (strict)"(error in=w333, "DisabledEnum"=w327) -> (error out=w332:errorcluster)  [unwired: 1 in, 1 out]
                    n116 = property on="C-Wave Shape" class="Ring (strict)"(error in=w332, "DisabledEnum"=w323) -> (error out=w331:errorcluster)  [unwired: 1 in, 1 out]
                    n117 = property on="C-Wave Shape" class="Ring (strict)"(error in=w331, "DisabledEnum"=w322) -> (error out=w330:errorcluster)  [unwired: 1 in, 1 out]
                  }
                  frame "EnableCurrSlew" {
                    w342 = 14 ("disabled index (col)")
                    # "Instr3"
                    # "Instr2"
                    # "Instr1"
                    # "Current slew Enabled/Disabled states are in index 14"
                    n118 = Unbundle By Name(w348) -> ("EnableCtrls"=w343:i8[][])
                    n119 = Index Array(array=w343, index (row) #1=0 ("disabled index (row)"), index (col) #1=w342, index (row) #2=1 ("disabled index (row)"), index (col) #2=w342, index (row) #3=2 ("disabled index (row)"), index (col) #3=w342) -> (element #1=w341:i8, element #2=w337:i8, element #3=w336:i8)
                    n120 = property on="Current (A/s)" class="DigNum (strict)"(error in=w347, "DisabledEnum"=w341) -> (error out=w346:errorcluster)  [unwired: 1 in, 1 out]
                    n121 = property on="Current (A/s)" class="DigNum (strict)"(error in=w346, "DisabledEnum"=w337) -> (error out=w345:errorcluster)  [unwired: 1 in, 1 out]
                    n122 = property on="Current (A/s)" class="DigNum (strict)"(error in=w345, "DisabledEnum"=w336) -> (error out=w344:errorcluster)  [unwired: 1 in, 1 out]
                  }
                  frame "EnablePowSlew" {
                    w356 = 15 ("disabled index (col)")
                    # "Instr3"
                    # "Instr2"
                    # "Instr1"
                    # "Power slew Enabled/Disabled states are in index 15"
                    n123 = Unbundle By Name(w362) -> ("EnableCtrls"=w357:i8[][])
                    n124 = Index Array(array=w357, index (row) #1=0 ("disabled index (row)"), index (col) #1=w356, index (row) #2=1 ("disabled index (row)"), index (col) #2=w356, index (row) #3=2 ("disabled index (row)"), index (col) #3=w356) -> (element #1=w355:i8, element #2=w351:i8, element #3=w350:i8)
                    n125 = property on="Power (W/s)" class="DigNum (strict)"(error in=w361, "DisabledEnum"=w355) -> (error out=w360:errorcluster)  [unwired: 1 in, 1 out]
                    n126 = property on="Power (W/s)" class="DigNum (strict)"(error in=w360, "DisabledEnum"=w351) -> (error out=w359:errorcluster)  [unwired: 1 in, 1 out]
                    n127 = property on="Power (W/s)" class="DigNum (strict)"(error in=w359, "DisabledEnum"=w350) -> (error out=w358:errorcluster)  [unwired: 1 in, 1 out]
                  }
                  frame "EnableFreqSlew" {
                    w370 = 16 ("disabled index (col)")
                    # "Instr3"
                    # "Instr2"
                    # "Instr1"
                    # "Frequency slew Enabled/Disabled states are in index 16"
                    n128 = Unbundle By Name(w376) -> ("EnableCtrls"=w371:i8[][])
                    n129 = Index Array(array=w371, index (row) #1=0 ("disabled index (row)"), index (col) #1=w370, index (row) #2=1 ("disabled index (row)"), index (col) #2=w370, index (row) #3=2 ("disabled index (row)"), index (col) #3=w370) -> (element #1=w369:i8, element #2=w365:i8, element #3=w364:i8)
                    n130 = property on="Frequency (Hz/s)" class="DigNum (strict)"(error in=w375, "DisabledEnum"=w369) -> (error out=w374:errorcluster)  [unwired: 1 in, 1 out]
                    n131 = property on="Frequency (Hz/s)" class="DigNum (strict)"(error in=w374, "DisabledEnum"=w365) -> (error out=w373:errorcluster)  [unwired: 1 in, 1 out]
                    n132 = property on="Frequency (Hz/s)" class="DigNum (strict)"(error in=w373, "DisabledEnum"=w364) -> (error out=w372:errorcluster)  [unwired: 1 in, 1 out]
                  }
                  frame "EnablePhaseSlew" {
                    w384 = 17 ("disabled index (col)")
                    # "Instr3"
                    # "Instr2"
                    # "Instr1"
                    # "Frequency slew Enabled/Disabled states are in index 17"
                    n133 = Unbundle By Name(w390) -> ("EnableCtrls"=w385:i8[][])
                    n134 = Index Array(array=w385, index (row) #1=0 ("disabled index (row)"), index (col) #1=w384, index (row) #2=1 ("disabled index (row)"), index (col) #2=w384, index (row) #3=2 ("disabled index (row)"), index (col) #3=w384) -> (element #1=w383:i8, element #2=w379:i8, element #3=w378:i8)
                    n135 = property on="Phase Angle (Deg/s)" class="DigNum (strict)"(error in=w389, "DisabledEnum"=w383) -> (error out=w388:errorcluster)  [unwired: 1 in, 1 out]
                    n136 = property on="Phase Angle (Deg/s)" class="DigNum (strict)"(error in=w388, "DisabledEnum"=w379) -> (error out=w387:errorcluster)  [unwired: 1 in, 1 out]
                    n137 = property on="Phase Angle (Deg/s)" class="DigNum (strict)"(error in=w387, "DisabledEnum"=w378) -> (error out=w386:errorcluster)  [unwired: 1 in, 1 out]
                  }
                }
              }
              frame Error {
                # "If the config file gives an error, discard the config procedure."
              }
            }
          }
        }
      }
      n138 = call-dynamic "CountChassis.vi"("NhRegenGridSim in"=w11, "error in (no error)"=w6) -> ("NhRegenGridSim out"=w13:refnum<class "NHRGridSim.lvclass">, "Chassis"=w10:u32, "ChassisTxt"=w9:string, "ChassisStatus"=w8:T15, "error out"=w7:errorcluster)  [unwired: 8 in, 1 out]
      n139 = case shown="\"Enabled\"" w8 {
        selector: w8 -> [w399 w405]
        tunnel: w7 -> [w398 w404]
        tunnel: [w397 w403] -> w12
        frame "Enabled" {
          n140 = property on="Chassis" class="DigNum (strict)"(error in=w398, "DisabledEnum"=w399, "NumText.BGColor"=u32 16777225, "NumText.TextColor"=u32 16777228, "NumText.FontBold"=FALSE ("Numeric Text.Font:Bold")) -> (error out=w397:errorcluster)  [unwired: 1 in, 1 out]
        }
        frame "Disabled", Default {
          n141 = property on="Chassis" class="DigNum (strict)"(error in=w404, "DisabledEnum"=w405, "NumText.BGColor"=u32 16777228, "NumText.TextColor"=u32 6618880, "NumText.FontBold"=TRUE ("Numeric Text.Font:Bold")) -> (error out=w403:errorcluster)  [unwired: 1 in, 1 out]
        }
      }
      n142 = local write "Chassis"(w10) -> ()
      n143 = local write "ChassisTxt"(w9) -> ()
      n144 = while {
        shift-right: [w411] -> w20
        shift-left: w13 -> [w412]
        tunnel: [w413] -> w25
        tunnel: [w409] -> w19
        tunnel: w12 -> [w410]
        tunnel: [w406] -> w15
        stop <- w408 stop-if-true
        n145 = event shown="[13] \"Measurement RefreshTime (ms)\", \"Measurements\": Value Change" {
          selector: _ -> [_ _ _ _ _ _ _ _ _ _ _ _ _ _ _ _ _ _ _ _ _ _ _ _ _ _ _ _ _ _ _ _]
          dyn-events: _ -> [_ _ _ _ _ _ _ _ _ _ _ _ _ _ _ _ _ _ _ _ _ _ _ _ _ _ _ _ _ _ _ _]
          timeout: _ -> [_ _ _ _ _ _ _ _ _ _ _ _ _ _ _ _ _ _ _ _ _ _ _ _ _ _ _ _ _ _ _ _]
          tunnel: [w414 w439 w455 _ w824 w2389 w2418 w2721 w2769 w2809 w2833 w2857 w2878 w2892 w2914 w2992 w3021 w3044 w3178 w3204 w3246 w3296 w3322 w3344 w3359 w3384 w3460 w3489 w3511 w3574 w3604 w3624] -> w413
          tunnel: [TRUE w439 w455 _ w824 w2389 w2418 w2721 w2769 w2809 w2833 w2857 w2878 w2892 w2914 w2992 w3021 w3044 w3178 w3204 w3246 w3296 w3322 w3344 w3359 w3384 w3460 w3489 w3511 w3574 w3604 w3624] -> w407
          tunnel: w412 -> [w416 w420 w454 w491 w827 w2390 w2419 w2722 w2770 w2810 w2834 w2858 w2879 w2891 w2915 w2993 w3022 w3047 w3180 w3206 w3248 w3298 w3324 w3346 w3361 w3385 w3461 w3490 w3512 w3576 w3606 w3626]
          tunnel: [w416 w428 w451 w491 w827 w2390 w2419 w2722 w2770 w2810 w2834 w2858 w2879 w2884 w2915 w2993 w3022 w3047 w3180 w3206 w3248 w3298 w3324 w3346 w3361 w3385 w3461 w3490 w3512 w3576 w3606 w3626] -> w411
          tunnel: [w415 w438 w452 w488 w820 w2386 w2395 w2719 w2767 w2807 w2831 w2855 w2872 w2880 w2910 w2988 w3017 w3035 w3172 w3198 w3243 w3293 w3319 w3339 w3354 w3375 w3451 w3480 w3508 w3571 w3601 w3621] -> w406
          tunnel: w410 -> [w415 w419 w453 w490 w825 w2380 w2405 w2703 w2751 w2799 w2823 w2853 w2873 w2885 w2903 w2980 w3009 w3037 w3173 w3199 w3236 w3286 w3312 w3340 w3355 w3372 w3449 w3478 w3505 w3567 w3597 w3617]
          tunnel: [w414 FALSE w455 _ w824 w2389 w2418 w2721 w2769 w2809 w2833 w2857 w2878 w2892 w2914 w2992 w3021 w3044 w3178 w3204 w3246 w3296 w3322 w3344 w3359 w3384 w3460 w3489 w3511 w3574 w3604 w3624] -> w409
          event "btnCancel": Value Change {
            w414 = FALSE
            # "Cancel the configuration operation with saving any changes"
            n146 = event-data() -> ()  [unwired: 1 in, 1 out]
          }
          event "btnSave": Value Change {
            w439 = TRUE ("StartMeas")
            # "Always write a false to the .ini file since the initialize function may have been called before the PrefDialog.vi"
            # "Save the changes made to the configuration properties"
            n147 = event-data() -> ()  [unwired: 1 in, 1 out]
            n148 = local read "Device(s)Settings"() -> (w418:T1)
            n149 = Bundle By Name(cluster=w418, "Connected"=FALSE) -> (w422:T1)
            n150 = local read "Measurement RefreshTime (ms)"() -> (w431:u32)
            n151 = local read "Measurements"() -> (w429:T9)
            n152 = To Variant(anything=w422) -> (Variant=w434:variant)
            n153 = To Variant(anything=w429) -> (Variant=w433:variant)
            n154 = call-dynamic "WriteToBaseConfigVariant.vi"("Measurement RefreshTime (ms)"=w431, "error in (no error)"=w419, "Meas"=w433, "Config"=w434, "NHRGridSim in"=w420) -> ("error out"=w432:errorcluster, "NHRGridSim out"=w421:refnum<class "NHRGridSim.lvclass">)  [unwired: 5 in]
            n155 = property class="NHRGridSim.lvclass"(reference=w421, error in=w432) -> (reference out=w428:refnum<class "NHRGridSim.lvclass">, error out=w427:errorcluster, "Accessors:PluginIniFilePath"=w430:path, "Accessors:BaseConfig"=w426:T16, "Accessors:BaseMeasurements"=w425:T18)
            n156 = local read "Measurement RefreshTime (ms)"() -> (w424:u32)
            n157 = call <vilib>:"Open Config Data.vi"("error in (no error)"=w427, "create file if necessary (T)"=FALSE, "configuration file path"=w430) -> ("error out"=w435:errorcluster, "refnum"=w436:T20)  [unwired: 6 in, 1 out]
            n158 = call-dynamic "WriteFile.vi"("Measurement Refresh Time (ms)"=w424, "Refnum in"=w436, "error in (no error)"=w435, "BaseMeasurements"=w425, "BaseConfiguration"=w426, "NHRGridSim in"=w421) -> ("error out"=w438:errorcluster)  [unwired: 4 in, 1 out]
          }
          event "btnSaveAs": Value Change {
            # "Save the configuration properties to a different file in the same location as the original file."
            n159 = event-data() -> ()  [unwired: 1 in, 1 out]
            n160 = property class="NHRGridSim.lvclass"(reference=w454, error in=w453) -> (reference out=w450:refnum<class "NHRGridSim.lvclass">, error out=w444:errorcluster, "Accessors:PluginIniFilePath"=w445:path)
            n161 = local read "Device(s)Settings"() -> (w447:T1)
            n162 = local read "Measurements"() -> (w449:T9)
            n163 = local read "Measurement RefreshTime (ms)"() -> (w448:u32)
            n164 = call "SaveAsFileDialog.vi"("error in"=w444, "Current File"=w445) -> ("error out"=w443:errorcluster, "Cancelled?"=w441:bool, "selected file path"=w442:path, "Current File out"=w446:path)  [unwired: 6 in]
            n165 = case shown="False" w441 {
              tunnel: [TRUE FALSE] -> w455
              tunnel: [w483 w485] -> w452
              tunnel: [w482 w487] -> w451
              tunnel: w450 -> [w469 w487]
              tunnel: w449 -> [w467 _]
              tunnel: w448 -> [w465 _]
              tunnel: w447 -> [w458 _]
              tunnel: w443 -> [w463 w485]
              tunnel: w446 -> [w462 _]
              tunnel: w442 -> [w461 _]
              frame False {
                # "Always write a false to the .ini file since the initialize function may have been called before the PrefDialog.vi"
                n166 = Bundle By Name(cluster=w458, "Connected"=FALSE) -> (w459:T1)
                n167 = Copy(8:w463, 10:w461, 11:w462) -> (0:w472:errorcluster, 3:w479:path)  [unwired: 2 in, 1 out]
                n168 = To Variant(anything=w467) -> (Variant=w466:variant)
                n169 = To Variant(anything=w458) -> (Variant=w468:variant)
                n170 = call-dynamic "WriteToBaseConfigVariant.vi"("Measurement RefreshTime (ms)"=w465, "error in (no error)"=w472, "Meas"=w466, "Config"=w468, "NHRGridSim in"=w469) -> ("error out"=w471:errorcluster, "NHRGridSim out"=w470:refnum<class "NHRGridSim.lvclass">)  [unwired: 5 in]
                n171 = property class="NHRGridSim.lvclass"(reference=w470, error in=w471, "Accessors:PluginIniFilePath"=w479) -> (reference out=w482:refnum<class "NHRGridSim.lvclass">, error out=w476:errorcluster, "Accessors:PluginIniFilePath"=w478:path, "Accessors:BaseConfig"=w477:T16, "Accessors:BaseMeasurements"=w474:T18)
                n172 = To Variant(anything=w467) -> (Variant=w473:variant)
                n173 = To Variant(anything=w459) -> (Variant=w481:variant)
                n174 = call-dynamic "WriteToBaseConfigVariant.vi"("Measurement RefreshTime (ms)"=w465, "error in (no error)"=w476, "Meas"=w473, "Config"=w481, "NHRGridSim in"=w482) -> ("error out"=w475:errorcluster, "NHRGridSim out"=w480:refnum<class "NHRGridSim.lvclass">)  [unwired: 5 in]
                n175 = call <vilib>:"Open Config Data.vi"("error in (no error)"=w475, "create file if necessary (T)"=FALSE, "configuration file path"=w478) -> ("error out"=w456:errorcluster, "refnum"=w457:T20)  [unwired: 6 in, 1 out]
                n176 = call-dynamic "WriteFile.vi"("Measurement Refresh Time (ms)"=w465, "Refnum in"=w457, "error in (no error)"=w456, "BaseMeasurements"=w474, "BaseConfiguration"=w477, "NHRGridSim in"=w480) -> ("error out"=w483:errorcluster)  [unwired: 4 in, 1 out]
              }
              frame True {
              }
            }
          }
          event "Update": Value Change {
            # "The reason to save the user available selections of the Voltage Range, Current Range, Configure Instrument, and AC Wave Shape controls is because the options that these controls will show to the user vary depending on Mode. If they were not stored in separate arrays from the index value of the present selection in the control, there would be no way to either save the options to or read them from a INI file. The Mode control doesn't need this treatment because the list of Mode options never changes. Saving the Mode value is enough."
            # "Populate the Device(s)Settings cluster every time that a change in the settings of the PrefDialog controls is made"
            n177 = event-data() -> ()  [unwired: 1 in, 1 out]
            n178 = while {
              shift-right: [w495] -> _
              shift-left: NHRGrid_UpdateSettings."VRanges" -> [w496]
              shift-right: [w492] -> w488
              shift-left: w490 -> [w493]
              stop <- w494 stop-if-true
              # "The frames are to avoid race conditions writing to the Device(s)Settings cluster."
              n179 = case shown="\"SaveEnables1\"" w496 {
                tunnel: [NHRGrid_UpdateSettings."CRanges" NHRGrid_UpdateSettings."Syncs" NHRGrid_UpdateSettings."Waves" NHRGrid_UpdateSettings."Values" NHRGrid_UpdateSettings."SaveEnables1" NHRGrid_UpdateSettings."SaveEnables2" NHRGrid_UpdateSettings."SaveEnables3" NHRGrid_UpdateSettings."SaveEnables4" NHRGrid_UpdateSettings."SaveEnables5" NHRGrid_UpdateSettings."SaveEnables6" _] -> w495
                tunnel: [FALSE FALSE FALSE FALSE FALSE FALSE FALSE FALSE FALSE FALSE TRUE] -> w494
                tunnel: w493 -> [w501 w521 w541 w561 w594 w641 w659 w687 w727 w758 w792]
                tunnel: [w498 w520 w538 w558 w593 w623 w649 w690 w724 w755 w783] -> w492
                frame "VRanges", Default {
                  # "The list of options for the Voltage Range changes depending on Mode. Save  the present list of V Range options in the instruments."
                  n180 = flat-sequence {
                    tunnel: w501 -> [w510]
                    tunnel: [w513] -> w500
                    tunnel: [w507] -> w499
                    tunnel: w500 -> [w516]
                    tunnel: [w515] -> w498
                    tunnel: w499 -> [w515]
                    frame #0 {
                      # "These are the actual ones to save."
                      # "These are only for feedback."
                      # "Instr1"
                      # "Instr2"
                      # "Instr3"
                      # "Instr3"
                      # "Instr2"
                      # "Instr1"
                      n181 = property on="Voltage (V)" class="Ring (strict)"(error in=w510) -> (error out=w512:errorcluster, "Strings []"=w503:string[])  [unwired: 1 in, 1 out]
                      n182 = property on="Voltage (V)" class="Ring (strict)"(error in=w512) -> (error out=w511:errorcluster, "Strings []"=w504:string[])  [unwired: 1 in, 1 out]
                      n183 = property on="Voltage (V)" class="Ring (strict)"(error in=w511) -> (error out=w506:errorcluster, "Strings []"=w505:string[])  [unwired: 1 in, 1 out]
                      n184 = property on="Voltage (V)" class="Ring (strict)"(error in=w506, "Strings []"=w505) -> (error out=w508:errorcluster)  [unwired: 1 in, 1 out]
                      n185 = property on="Voltage (V)" class="Ring (strict)"(error in=w508, "Strings []"=w504) -> (error out=w509:errorcluster)  [unwired: 1 in, 1 out]
                      n186 = property on="Voltage (V)" class="Ring (strict)"(error in=w509, "Strings []"=w503) -> (error out=w507:errorcluster)  [unwired: 1 in, 1 out]
                      n187 = local read "Device(s)Settings"() -> (w514:T1)
                      n188 = Bundle By Name(cluster=w514, "VRangeVals3"=w505, "VRangeVals2"=w504, "VRangeVals1"=w503) -> (w513:T1)
                    }
                    frame #1 {
                      n189 = local write "Device(s)Settings"(w516) -> ()
                    }
                  }
                }
                frame "CRanges" {
                  # "The list of options for the Current Range changes depending on Mode. Save  the present list of options in the instruments."
                  n190 = flat-sequence {
                    tunnel: w521 -> [w532]
                    tunnel: [w526] -> w519
                    tunnel: [w533] -> w518
                    tunnel: [w536] -> w520
                    tunnel: w519 -> [w536]
                    tunnel: w518 -> [w535]
                    frame #0 {
                      # "These are the actual ones to save."
                      # "These are only for feedback."
                      # "Instr1"
                      # "Instr2"
                      # "Instr3"
                      # "Instr3"
                      # "Instr2"
                      # "Instr1"
                      n191 = property on="Current (A)" class="Ring (strict)"(error in=w532) -> (error out=w531:errorcluster, "Strings []"=w523:string[])  [unwired: 1 in, 1 out]
                      n192 = property on="Current (A)" class="Ring (strict)"(error in=w531) -> (error out=w530:errorcluster, "Strings []"=w524:string[])  [unwired: 1 in, 1 out]
                      n193 = property on="Current (A)" class="Ring (strict)"(error in=w530) -> (error out=w527:errorcluster, "Strings []"=w525:string[])  [unwired: 1 in, 1 out]
                      n194 = property on="Current (A)" class="Ring (strict)"(error in=w527, "Strings []"=w525) -> (error out=w528:errorcluster)  [unwired: 1 in, 1 out]
                      n195 = property on="Current (A)" class="Ring (strict)"(error in=w528, "Strings []"=w524) -> (error out=w529:errorcluster)  [unwired: 1 in, 1 out]
                      n196 = property on="Current (A)" class="Ring (strict)"(error in=w529, "Strings []"=w523) -> (error out=w526:errorcluster)  [unwired: 1 in, 1 out]
                      n197 = local read "Device(s)Settings"() -> (w534:T1)
                      n198 = Bundle By Name(cluster=w534, "CRangeVals3"=w525, "CRangeVals2"=w524, "CRangeVals1"=w523) -> (w533:T1)
                    }
                    frame #1 {
                      n199 = local write "Device(s)Settings"(w535) -> ()
                    }
                  }
                }
                frame "Syncs" {
                  # "The list of options for the Synchronization control changes depending on Mode. Save the present list of options in the instruments."
                  n200 = flat-sequence {
                    tunnel: w541 -> [w552]
                    tunnel: [w553] -> w540
                    tunnel: [w547] -> w539
                    tunnel: w540 -> [w556]
                    tunnel: w539 -> [w555]
                    tunnel: [w555] -> w538
                    frame #0 {
                      # "Update the values in Device(s)Settings controls too"
                      # "Instr1"
                      # "Instr2"
                      # "Instr3"
                      # "Instr3"
                      # "Instr2"
                      # "Instr1"
                      n201 = property on="Synchronization" class="Ring (strict)"(error in=w552) -> (error out=w551:errorcluster, "Strings []"=w543:string[])  [unwired: 1 in, 1 out]
                      n202 = property on="Synchronization" class="Ring (strict)"(error in=w551) -> (error out=w550:errorcluster, "Strings []"=w544:string[])  [unwired: 1 in, 1 out]
                      n203 = property on="Synchronization" class="Ring (strict)"(error in=w550) -> (error out=w546:errorcluster, "Strings []"=w545:string[])  [unwired: 1 in, 1 out]
                      n204 = property on="Synchronization" class="Ring (strict)"(error in=w546, "Strings []"=w545) -> (error out=w548:errorcluster)  [unwired: 1 in, 1 out]
                      n205 = property on="Synchronization" class="Ring (strict)"(error in=w548, "Strings []"=w544) -> (error out=w549:errorcluster)  [unwired: 1 in, 1 out]
                      n206 = local read "Device(s)Settings"() -> (w554:T1)
                      n207 = property on="Synchronization" class="Ring (strict)"(error in=w549, "Strings []"=w543) -> (error out=w547:errorcluster)  [unwired: 1 in, 1 out]
                      n208 = Bundle By Name(cluster=w554, "SyncList3"=w545, "SyncList2"=w544, "SyncList1"=w543) -> (w553:T1)
                    }
                    frame #1 {
                      n209 = local write "Device(s)Settings"(w556) -> ()
                    }
                  }
                }
                frame "Waves" {
                  # "The list of options for the AC phase waveforms changes depending on Mode. Save  the present list of options in the instruments."
                  n210 = flat-sequence {
                    tunnel: w561 -> [w567]
                    tunnel: [w563] -> w560
                    tunnel: w560 -> [w578]
                    tunnel: [w573] -> w559
                    tunnel: w559 -> [w588]
                    tunnel: [w584] -> w558
                    frame #0 {
                      # "Instr1"
                      n211 = property on="A-Wave Shape" class="Ring (strict)"(error in=w567) -> (error out=w566:errorcluster, "Strings []"=w572:string[])  [unwired: 1 in, 1 out]
                      n212 = property on="B-Wave Shape" class="Ring (strict)"(error in=w567) -> (error out=w565:errorcluster, "Strings []"=w571:string[])  [unwired: 1 in, 1 out]
                      n213 = property on="C-Wave Shape" class="Ring (strict)"(error in=w567) -> (error out=w564:errorcluster, "Strings []"=w570:string[])  [unwired: 1 in, 1 out]
                      n214 = local read "Device(s)Settings"() -> (w569:T1)
                      n215 = Bundle By Name(cluster=w569, "Wave1A"=w572, "Wave1B"=w571, "Wave1C"=w570) -> (w568:T1)
                      n216 = local write "Device(s)Settings"(w568) -> ()
                      n217 = Merge Errors(w566, w565, w564) -> (w563:errorcluster)
                    }
                    frame #1 {
                      # "Instr2"
                      n218 = property on="A-Wave Shape" class="Ring (strict)"(error in=w578) -> (error out=w574:errorcluster, "Strings []"=w582:string[])  [unwired: 1 in, 1 out]
                      n219 = property on="B-Wave Shape" class="Ring (strict)"(error in=w578) -> (error out=w575:errorcluster, "Strings []"=w581:string[])  [unwired: 1 in, 1 out]
                      n220 = property on="C-Wave Shape" class="Ring (strict)"(error in=w578) -> (error out=w576:errorcluster, "Strings []"=w580:string[])  [unwired: 1 in, 1 out]
                      n221 = local read "Device(s)Settings"() -> (w579:T1)
                      n222 = Bundle By Name(cluster=w579, "Wave2A"=w582, "Wave2B"=w581, "Wave2C"=w580) -> (w577:T1)
                      n223 = local write "Device(s)Settings"(w577) -> ()
                      n224 = Merge Errors(w574, w575, w576) -> (w573:errorcluster)
                    }
                    frame #2 {
                      # "Instr3"
                      n225 = property on="A-Wave Shape" class="Ring (strict)"(error in=w588) -> (error out=w585:errorcluster, "Strings []"=w592:string[])  [unwired: 1 in, 1 out]
                      n226 = property on="B-Wave Shape" class="Ring (strict)"(error in=w588) -> (error out=w586:errorcluster, "Strings []"=w591:string[])  [unwired: 1 in, 1 out]
                      n227 = property on="C-Wave Shape" class="Ring (strict)"(error in=w588) -> (error out=w587:errorcluster, "Strings []"=w590:string[])  [unwired: 1 in, 1 out]
                      n228 = local read "Device(s)Settings"() -> (w589:T1)
                      n229 = Bundle By Name(cluster=w589, "Wave3A"=w592, "Wave3B"=w591, "Wave3C"=w590) -> (w583:T1)
                      n230 = local write "Device(s)Settings"(w583) -> ()
                      n231 = Merge Errors(w585, w586, w587) -> (w584:errorcluster)
                    }
                  }
                }
                frame "Values" {
                  # "Exchange the data that can be passed directly between the Instruments and the Device(s)Settings cluster."
                  n232 = flat-sequence {
                    tunnel: [w603] -> w597
                    tunnel: [w599] -> w595
                    tunnel: w594 -> [w599]
                    tunnel: w597 -> [w612]
                    tunnel: w595 -> [w611]
                    tunnel: [w611] -> w593
                    frame #0 {
                      # "This will take care of passing everything that is simply a value or an indexed setting choice. Some controls will share values directly. The clusters will only pass values, the properties of some of their controls need to be specified in a different way or Device(s)Settings will have no way to register them."
                      n233 = local read "Instr1"() -> (w602:T2)
                      n234 = local read "Instr3"() -> (w600:T2)
                      n235 = local read "ID Query"() -> (w609:bool)
                      n236 = local read "Reset"() -> (w607:bool)
                      n237 = local read "Instr2"() -> (w601:T2)
                      n238 = local read "MeasName"() -> (w605:string)
                      n239 = local read "Connected"() -> (w608:bool)
                      n240 = local read "Mode"() -> (w610:T8)
                      n241 = local read "Handle"() -> (w606:string)
                      n242 = local read "Device(s)Settings"() -> (w604:T1)
                      n243 = Bundle By Name(cluster=w604, "MeasName"=w605, "Instr1"=w602, "Instr2"=w601, "Instr3"=w600, "Handle"=w606, "Reset"=w607, "Connected"=w608, "ID Query"=w609, "Mode"=w610) -> (w603:T1)
                    }
                    frame #1 {
                      n244 = local write "Device(s)Settings"(w612) -> ()
                    }
                  }
                }
                frame "SaveEnables1" {
                  # "Instr3"
                  # "Instr2"
                  # "Instr1"
                  # "Instr3"
                  # "Instr2"
                  # "Instr1"
                  # "Instr3"
                  # "Instr2"
                  # "Instr1"
                  n245 = property on="Name" class="Str"(error in=w641) -> (error out=w644:errorcluster, "DisabledEnum"=w614:T15)  [unwired: 1 in, 1 out]
                  n246 = local read "Device(s)Settings"() -> (w642:T1)
                  n247 = property on="Name" class="Str"(error in=w644) -> (error out=w645:errorcluster, "DisabledEnum"=w615:T15)  [unwired: 1 in, 1 out]
                  n248 = Unbundle By Name(w642) -> ("EnableCtrls"=w617:i8[][])
                  n249 = property on="Name" class="Str"(error in=w645) -> (error out=w636:errorcluster, "DisabledEnum"=w616:T15)  [unwired: 1 in, 1 out]
                  n250 = Build Array(w614, w615, w616) -> (w613:T21)
                  n251 = property on="FreqOut (Hz)" class="DigNum (strict)"(error in=w636) -> (error out=w640:errorcluster, "DisabledEnum"=w633:T15)  [unwired: 1 in, 1 out]
                  n252 = Replace Array Subset(array=w617, new element=w613, index (col)=0 ("disabled index (col)")) -> (w618:i8[][])  [unwired: 1 in]
                  n253 = property on="FreqOut (Hz)" class="DigNum (strict)"(error in=w640) -> (error out=w639:errorcluster, "DisabledEnum"=w634:T15)  [unwired: 1 in, 1 out]
                  n254 = property on="FreqOut (Hz)" class="DigNum (strict)"(error in=w639) -> (error out=w630:errorcluster, "DisabledEnum"=w635:T15)  [unwired: 1 in, 1 out]
                  n255 = Build Array(w633, w634, w635) -> (w637:T21)
                  n256 = property on="Synchronization" class="Ring (strict)"(error in=w630) -> (error out=w632:errorcluster, "DisabledEnum"=w626:T15)  [unwired: 1 in, 1 out]
                  n257 = Replace Array Subset(array=w618, new element=w637, index (col)=1 ("disabled index (col)")) -> (w627:i8[][])  [unwired: 1 in]
                  n258 = property on="Synchronization" class="Ring (strict)"(error in=w632) -> (error out=w631:errorcluster, "DisabledEnum"=w625:T15)  [unwired: 1 in, 1 out]
                  n259 = property on="Synchronization" class="Ring (strict)"(error in=w631) -> (error out=w623:errorcluster, "DisabledEnum"=w624:T15)  [unwired: 1 in, 1 out]
                  n260 = Build Array(w626, w625, w624) -> (w628:T21)
                  n261 = local read "Device(s)Settings"() -> (w643:T1)
                  n262 = Replace Array Subset(array=w627, new element=w628, index (col)=2 ("disabled index (col)")) -> (w622:i8[][])  [unwired: 1 in]
                  n263 = Bundle By Name(cluster=w643, "EnableCtrls"=w622) -> (w621:T1)
                  n264 = local write "Device(s)Settings"(w621) -> ()
                }
                frame "SaveEnables2" {
                  # "Instr3"
                  # "Instr2"
                  # "Instr1"
                  # "Instr3"
                  # "Instr2"
                  # "Instr1"
                  # "Instr3"
                  # "Instr2"
                  # "Instr1"
                  n265 = property on="A-Volts (V)" class="DigNum (strict)"(error in=w659) -> (error out=w661:errorcluster, "DisabledEnum"=w654:T15)  [unwired: 1 in, 1 out]
                  n266 = local read "Device(s)Settings"() -> (w677:T1)
                  n267 = property on="A-Volts (V)" class="DigNum (strict)"(error in=w661) -> (error out=w660:errorcluster, "DisabledEnum"=w655:T15)  [unwired: 1 in, 1 out]
                  n268 = property on="A-Volts (V)" class="DigNum (strict)"(error in=w660) -> (error out=w658:errorcluster, "DisabledEnum"=w656:T15)  [unwired: 1 in, 1 out]
                  n269 = Unbundle By Name(w677) -> ("EnableCtrls"=w676:i8[][])
                  n270 = Build Array(w654, w655, w656) -> (w675:T21)
                  n271 = property on="B-Volts (V)" class="DigNum (strict)"(error in=w658) -> (error out=w663:errorcluster, "DisabledEnum"=w651:T15)  [unwired: 1 in, 1 out]
                  n272 = Replace Array Subset(array=w676, new element=w675, index (col)=3 ("disabled index (col)")) -> (w672:i8[][])  [unwired: 1 in]
                  n273 = property on="B-Volts (V)" class="DigNum (strict)"(error in=w663) -> (error out=w662:errorcluster, "DisabledEnum"=w652:T15)  [unwired: 1 in, 1 out]
                  n274 = property on="B-Volts (V)" class="DigNum (strict)"(error in=w662) -> (error out=w657:errorcluster, "DisabledEnum"=w653:T15)  [unwired: 1 in, 1 out]
                  n275 = Build Array(w651, w652, w653) -> (w673:T21)
                  n276 = Replace Array Subset(array=w672, new element=w673, index (col)=4 ("disabled index (col)")) -> (w669:i8[][])  [unwired: 1 in]
                  n277 = property on="C-Volts (V)" class="DigNum (strict)"(error in=w657) -> (error out=w665:errorcluster, "DisabledEnum"=w647:T15)  [unwired: 1 in, 1 out]
                  n278 = property on="C-Volts (V)" class="DigNum (strict)"(error in=w665) -> (error out=w664:errorcluster, "DisabledEnum"=w648:T15)  [unwired: 1 in, 1 out]
                  n279 = property on="C-Volts (V)" class="DigNum (strict)"(error in=w664) -> (error out=w649:errorcluster, "DisabledEnum"=w650:T15)  [unwired: 1 in, 1 out]
                  n280 = Build Array(w647, w648, w650) -> (w670:T21)
                  n281 = local read "Device(s)Settings"() -> (w679:T1)
                  n282 = Replace Array Subset(array=w669, new element=w670, index (col)=5 ("disabled index (col)")) -> (w668:i8[][])  [unwired: 1 in]
                  n283 = Bundle By Name(cluster=w679, "EnableCtrls"=w668) -> (w667:T1)
                  n284 = local write "Device(s)Settings"(w667) -> ()
                }
                frame "SaveEnables3" {
                  # "Instr3"
                  # "Instr2"
                  # "Instr1"
                  # "Instr3"
                  # "Instr2"
                  # "Instr1"
                  # "Instr3"
                  # "Instr2"
                  # "Instr1"
                  n285 = property on="B-Angle (Deg)" class="DigNum (strict)"(error in=w687) -> (error out=w695:errorcluster, "DisabledEnum"=w681:T15)  [unwired: 1 in, 1 out]
                  n286 = local read "Device(s)Settings"() -> (w711:T1)
                  n287 = property on="B-Angle (Deg)" class="DigNum (strict)"(error in=w695) -> (error out=w694:errorcluster, "DisabledEnum"=w682:T15)  [unwired: 1 in, 1 out]
                  n288 = Unbundle By Name(w711) -> ("EnableCtrls"=w710:i8[][])
                  n289 = property on="B-Angle (Deg)" class="DigNum (strict)"(error in=w694) -> (error out=w688:errorcluster, "DisabledEnum"=w683:T15)  [unwired: 1 in, 1 out]
                  n290 = Build Array(w681, w682, w683) -> (w709:T21)
                  n291 = property on="C-Angle (Deg)" class="DigNum (strict)"(error in=w688) -> (error out=w697:errorcluster, "DisabledEnum"=w684:T15)  [unwired: 1 in, 1 out]
                  n292 = Replace Array Subset(array=w710, new element=w709, index (col)=6 ("disabled index (col)")) -> (w706:i8[][])  [unwired: 1 in]
                  n293 = property on="C-Angle (Deg)" class="DigNum (strict)"(error in=w697) -> (error out=w696:errorcluster, "DisabledEnum"=w685:T15)  [unwired: 1 in, 1 out]
                  n294 = property on="C-Angle (Deg)" class="DigNum (strict)"(error in=w696) -> (error out=w689:errorcluster, "DisabledEnum"=w686:T15)  [unwired: 1 in, 1 out]
                  n295 = Build Array(w684, w685, w686) -> (w707:T21)
                  n296 = property on="A-Change at..." class="DigNum (strict)"(error in=w689) -> (error out=w699:errorcluster, "DisabledEnum"=w691:T15)  [unwired: 1 in, 1 out]
                  n297 = Replace Array Subset(array=w706, new element=w707, index (col)=7 ("disabled index (col)")) -> (w703:i8[][])  [unwired: 1 in]
                  n298 = property on="A-Change at..." class="DigNum (strict)"(error in=w699) -> (error out=w698:errorcluster, "DisabledEnum"=w692:T15)  [unwired: 1 in, 1 out]
                  n299 = property on="A-Change at..." class="DigNum (strict)"(error in=w698) -> (error out=w690:errorcluster, "DisabledEnum"=w693:T15)  [unwired: 1 in, 1 out]
                  n300 = Build Array(w691, w692, w693) -> (w704:T21)
                  n301 = local read "Device(s)Settings"() -> (w713:T1)
                  n302 = Replace Array Subset(array=w703, new element=w704, index (col)=8 ("disabled index (col)")) -> (w702:i8[][])  [unwired: 1 in]
                  n303 = Bundle By Name(cluster=w713, "EnableCtrls"=w702) -> (w701:T1)
                  n304 = local write "Device(s)Settings"(w701) -> ()
                }
                frame "SaveEnables4" {
                  # "Instr3"
                  # "Instr2"
                  # "Instr1"
                  # "Instr3"
                  # "Instr2"
                  # "Instr1"
                  # "Instr3"
                  # "Instr2"
                  # "Instr1"
                  n305 = property on="B-Change at..." class="DigNum (strict)"(error in=w727) -> (error out=w729:errorcluster, "DisabledEnum"=w715:T15)  [unwired: 1 in, 1 out]
                  n306 = local read "Device(s)Settings"() -> (w745:T1)
                  n307 = property on="B-Change at..." class="DigNum (strict)"(error in=w729) -> (error out=w728:errorcluster, "DisabledEnum"=w716:T15)  [unwired: 1 in, 1 out]
                  n308 = property on="B-Change at..." class="DigNum (strict)"(error in=w728) -> (error out=w726:errorcluster, "DisabledEnum"=w717:T15)  [unwired: 1 in, 1 out]
                  n309 = Unbundle By Name(w745) -> ("EnableCtrls"=w744:i8[][])
                  n310 = Build Array(w715, w716, w717) -> (w743:T21)
                  n311 = property on="C-Change at..." class="DigNum (strict)"(error in=w726) -> (error out=w731:errorcluster, "DisabledEnum"=w718:T15)  [unwired: 1 in, 1 out]
                  n312 = Replace Array Subset(array=w744, new element=w743, index (col)=9 ("disabled index (col)")) -> (w740:i8[][])  [unwired: 1 in]
                  n313 = property on="C-Change at..." class="DigNum (strict)"(error in=w731) -> (error out=w730:errorcluster, "DisabledEnum"=w719:T15)  [unwired: 1 in, 1 out]
                  n314 = property on="C-Change at..." class="DigNum (strict)"(error in=w730) -> (error out=w725:errorcluster, "DisabledEnum"=w720:T15)  [unwired: 1 in, 1 out]
                  n315 = Build Array(w718, w719, w720) -> (w741:T21)
                  n316 = property on="A-Wave Shape" class="Ring (strict)"(error in=w725) -> (error out=w733:errorcluster, "DisabledEnum"=w721:T15)  [unwired: 1 in, 1 out]
                  n317 = Replace Array Subset(array=w740, new element=w741, index (col)=10 ("disabled index (col)")) -> (w737:i8[][])  [unwired: 1 in]
                  n318 = property on="A-Wave Shape" class="Ring (strict)"(error in=w733) -> (error out=w732:errorcluster, "DisabledEnum"=w722:T15)  [unwired: 1 in, 1 out]
                  n319 = property on="A-Wave Shape" class="Ring (strict)"(error in=w732) -> (error out=w724:errorcluster, "DisabledEnum"=w723:T15)  [unwired: 1 in, 1 out]
                  n320 = Build Array(w721, w722, w723) -> (w738:T21)
                  n321 = local read "Device(s)Settings"() -> (w747:T1)
                  n322 = Replace Array Subset(array=w737, new element=w738, index (col)=11 ("disabled index (col)")) -> (w736:i8[][])  [unwired: 1 in]
                  n323 = Bundle By Name(cluster=w747, "EnableCtrls"=w736) -> (w735:T1)
                  n324 = local write "Device(s)Settings"(w735) -> ()
                }
                frame "SaveEnables5" {
                  # "Instr1"
                  # "Instr3"
                  # "Instr2"
                  # "Instr1"
                  # "Instr3"
                  # "Instr2"
                  # "Instr1"
                  # "Instr3"
                  # "Instr2"
                  # "Instr1"
                  n325 = property on="B-Wave Shape" class="Ring (strict)"(error in=w758) -> (error out=w763:errorcluster, "DisabledEnum"=w759:T15)  [unwired: 1 in, 1 out]
                  n326 = local read "Device(s)Settings"() -> (w779:T1)
                  n327 = property on="B-Wave Shape" class="Ring (strict)"(error in=w763) -> (error out=w762:errorcluster, "DisabledEnum"=w760:T15)  [unwired: 1 in, 1 out]
                  n328 = property on="B-Wave Shape" class="Ring (strict)"(error in=w762) -> (error out=w757:errorcluster, "DisabledEnum"=w761:T15)  [unwired: 1 in, 1 out]
                  n329 = Unbundle By Name(w779) -> ("EnableCtrls"=w778:i8[][])
                  n330 = Build Array(w759, w760, w761) -> (w777:T21)
                  n331 = property on="C-Wave Shape" class="Ring (strict)"(error in=w757) -> (error out=w765:errorcluster, "DisabledEnum"=w752:T15)  [unwired: 1 in, 1 out]
                  n332 = Replace Array Subset(array=w778, new element=w777, index (col)=12 ("disabled index (col)")) -> (w774:i8[][])  [unwired: 1 in]
                  n333 = property on="C-Wave Shape" class="Ring (strict)"(error in=w765) -> (error out=w764:errorcluster, "DisabledEnum"=w753:T15)  [unwired: 1 in, 1 out]
                  n334 = property on="C-Wave Shape" class="Ring (strict)"(error in=w764) -> (error out=w756:errorcluster, "DisabledEnum"=w754:T15)  [unwired: 1 in, 1 out]
                  n335 = Build Array(w752, w753, w754) -> (w775:T21)
                  n336 = property on="Current (A/s)" class="DigNum (strict)"(error in=w756) -> (error out=w767:errorcluster, "DisabledEnum"=w749:T15)  [unwired: 1 in, 1 out]
                  n337 = Replace Array Subset(array=w774, new element=w775, index (col)=13 ("disabled index (col)")) -> (w771:i8[][])  [unwired: 1 in]
                  n338 = property on="Current (A/s)" class="DigNum (strict)"(error in=w767) -> (error out=w766:errorcluster, "DisabledEnum"=w750:T15)  [unwired: 1 in, 1 out]
                  n339 = property on="Current (A/s)" class="DigNum (strict)"(error in=w766) -> (error out=w755:errorcluster, "DisabledEnum"=w751:T15)  [unwired: 1 in, 1 out]
                  n340 = Build Array(w749, w750, w751) -> (w772:T21)
                  n341 = local read "Device(s)Settings"() -> (w781:T1)
                  n342 = Replace Array Subset(array=w771, new element=w772, index (col)=14 ("disabled index (col)")) -> (w770:i8[][])  [unwired: 1 in]
                  n343 = Bundle By Name(cluster=w781, "EnableCtrls"=w770) -> (w769:T1)
                  n344 = local write "Device(s)Settings"(w769) -> ()
                }
                frame "SaveEnables6" {
                  # "Instr1"
                  # "Instr3"
                  # "Instr2"
                  # "Instr1"
                  # "Instr3"
                  # "Instr2"
                  # "Instr1"
                  # "Instr3"
                  # "Instr2"
                  # "Instr1"
                  n345 = property on="Power (W/s)" class="DigNum (strict)"(error in=w792) -> (error out=w797:errorcluster, "DisabledEnum"=w793:T15)  [unwired: 1 in, 1 out]
                  n346 = local read "Device(s)Settings"() -> (w812:T1)
                  n347 = property on="Power (W/s)" class="DigNum (strict)"(error in=w797) -> (error out=w796:errorcluster, "DisabledEnum"=w794:T15)  [unwired: 1 in, 1 out]
                  n348 = property on="Power (W/s)" class="DigNum (strict)"(error in=w796) -> (error out=w791:errorcluster, "DisabledEnum"=w795:T15)  [unwired: 1 in, 1 out]
                  n349 = Unbundle By Name(w812) -> ("EnableCtrls"=w811:i8[][])
                  n350 = Build Array(w793, w794, w795) -> (w810:T21)
                  n351 = property on="Frequency (Hz/s)" class="DigNum (strict)"(error in=w791) -> (error out=w799:errorcluster, "DisabledEnum"=w790:T15)  [unwired: 1 in, 1 out]
                  n352 = Replace Array Subset(array=w811, new element=w810, index (col)=15 ("disabled index (col)")) -> (w807:i8[][])  [unwired: 1 in]
                  n353 = property on="Frequency (Hz/s)" class="DigNum (strict)"(error in=w799) -> (error out=w798:errorcluster, "DisabledEnum"=w789:T15)  [unwired: 1 in, 1 out]
                  n354 = property on="Frequency (Hz/s)" class="DigNum (strict)"(error in=w798) -> (error out=w787:errorcluster, "DisabledEnum"=w788:T15)  [unwired: 1 in, 1 out]
                  n355 = Build Array(w790, w789, w788) -> (w808:T21)
                  n356 = property on="Phase Angle (Deg/s)" class="DigNum (strict)"(error in=w787) -> (error out=w801:errorcluster, "DisabledEnum"=w786:T15)  [unwired: 1 in, 1 out]
                  n357 = Replace Array Subset(array=w807, new element=w808, index (col)=16 ("disabled index (col)")) -> (w804:i8[][])  [unwired: 1 in]
                  n358 = property on="Phase Angle (Deg/s)" class="DigNum (strict)"(error in=w801) -> (error out=w800:errorcluster, "DisabledEnum"=w785:T15)  [unwired: 1 in, 1 out]
                  n359 = property on="Phase Angle (Deg/s)" class="DigNum (strict)"(error in=w800) -> (error out=w783:errorcluster, "DisabledEnum"=w784:T15)  [unwired: 1 in, 1 out]
                  n360 = Build Array(w786, w785, w784) -> (w805:T21)
                  n361 = local read "Device(s)Settings"() -> (w814:T1)
                  n362 = Replace Array Subset(array=w804, new element=w805, index (col)=17 ("disabled index (col)")) -> (w803:i8[][])  [unwired: 1 in]
                  n363 = Bundle By Name(cluster=w814, "EnableCtrls"=w803) -> (w802:T1)
                  n364 = local write "Device(s)Settings"(w802) -> ()
                }
              }
            }
          }
          event Value Change {
            w821 = T15."Enabled" ("Disabled")
            w824 = FALSE ("StartMeas")
            # "Update Device(s)Settings"
            n365 = event-data() -> ()  [unwired: 1 in, 1 out]
            n366 = while {
              shift-right: [w830] -> _
              shift-left: NHRGrid_ModeAdjust_Tabs."ShowTabs" ("AcPwrPlugins.lvlib:NHRGridSim.lvclass:NHRGrid_ModeAdjust_Tabs") -> [w832]
              shift-right: [w831] -> w818
              shift-left: w825 -> [w828]
              stop <- w829 stop-if-true
              n367 = case shown="No Error" w828 {
                selector: w828 -> [w833 w2378]
                tunnel: w832 -> [w837 w2376]
                tunnel: [w836 w2378] -> w831
                tunnel: [w835 w2376] -> w830
                tunnel: [w834 TRUE] -> w829
                frame No Error {
                  n368 = case shown="\"WaveEnable\"" w837 {
                    tunnel: w833 -> [w847 w903 w950 w1040 w1073 w1077 w1129 w1319 w1348 w1386 w1428 w1449 w1483 w1697 w1757 w1780 w1930 w1976 w2031 w2052 w2091 w2130 w2169 w2208 w2227 w2238 w2255 w2295 w2311]
                    tunnel: [w838 w893 w955 w1039 w1070 w1076 w1117 w1301 w1335 w1377 w1417 w1448 w1474 w1687 w1753 w1778 w1927 w1974 w2036 w2042 w2081 w2120 w2159 w2211 w2230 w2249 w2254 w2276 w2312] -> w836
                    tunnel: [NHRGrid_ModeAdjust_Tabs."InstrNames" ("AcPwrPlugins.lvlib:NHRGridSim.lvclass:NHRGrid_ModeAdjust_Tabs") NHRGrid_ModeAdjust_Tabs."VoltRanges" ("AcPwrPlugins.lvlib:NHRGridSim.lvclass:NHRGrid_ModeAdjust_Tabs") NHRGrid_ModeAdjust_Tabs."ConfigSync" ("AcPwrPlugins.lvlib:NHRGridSim.lvclass:NHRGrid_ModeAdjust_Tabs") NHRGrid_ModeAdjust_Tabs."Safety" ("AcPwrPlugins.lvlib:NHRGridSim.lvclass:NHRGrid_ModeAdjust_Tabs") NHRGrid_ModeAdjust_Tabs."Phases" ("AcPwrPlugins.lvlib:NHRGridSim.lvclass:NHRGrid_ModeAdjust_Tabs") NHRGrid_ModeAdjust_Tabs."FreqOut" ("AcPwrPlugins.lvlib:NHRGridSim.lvclass:NHRGrid_ModeAdjust_Tabs") NHRGrid_ModeAdjust_Tabs."PhaseEnable" ("AcPwrPlugins.lvlib:NHRGridSim.lvclass:NHRGrid_ModeAdjust_Tabs") NHRGrid_ModeAdjust_Tabs."SyncEnable" ("AcPwrPlugins.lvlib:NHRGridSim.lvclass:NHRGrid_ModeAdjust_Tabs") NHRGrid_ModeAdjust_Tabs."ChangeEnable" ("AcPwrPlugins.lvlib:NHRGridSim.lvclass:NHRGrid_ModeAdjust_Tabs") NHRGrid_ModeAdjust_Tabs."VoltsEnable" ("AcPwrPlugins.lvlib:NHRGridSim.lvclass:NHRGrid_ModeAdjust_Tabs") NHRGrid_ModeAdjust_Tabs."Vtype" ("AcPwrPlugins.lvlib:NHRGridSim.lvclass:NHRGrid_ModeAdjust_Tabs") NHRGrid_ModeAdjust_Tabs."Description" ("AcPwrPlugins.lvlib:NHRGridSim.lvclass:NHRGrid_ModeAdjust_Tabs") NHRGrid_ModeAdjust_Tabs."CurrRanges" ("AcPwrPlugins.lvlib:NHRGridSim.lvclass:NHRGrid_ModeAdjust_Tabs") NHRGrid_ModeAdjust_Tabs."VoutCoerce" ("AcPwrPlugins.lvlib:NHRGridSim.lvclass:NHRGrid_ModeAdjust_Tabs") NHRGrid_ModeAdjust_Tabs."VSlewCoerce" ("AcPwrPlugins.lvlib:NHRGridSim.lvclass:NHRGrid_ModeAdjust_Tabs") NHRGrid_ModeAdjust_Tabs."CSlewCoerce" ("AcPwrPlugins.lvlib:NHRGridSim.lvclass:NHRGrid_ModeAdjust_Tabs") NHRGrid_ModeAdjust_Tabs."PSlewCoerce" ("AcPwrPlugins.lvlib:NHRGridSim.lvclass:NHRGrid_ModeAdjust_Tabs") NHRGrid_ModeAdjust_Tabs."F&PhCoerce" ("AcPwrPlugins.lvlib:NHRGridSim.lvclass:NHRGrid_ModeAdjust_Tabs") NHRGrid_ModeAdjust_Tabs."SlewsCurr" ("AcPwrPlugins.lvlib:NHRGridSim.lvclass:NHRGrid_ModeAdjust_Tabs") NHRGrid_ModeAdjust_Tabs."SlewsPow" ("AcPwrPlugins.lvlib:NHRGridSim.lvclass:NHRGrid_ModeAdjust_Tabs") NHRGrid_ModeAdjust_Tabs."SlewsFreq" ("AcPwrPlugins.lvlib:NHRGridSim.lvclass:NHRGrid_ModeAdjust_Tabs") NHRGrid_ModeAdjust_Tabs."SlewsPhase" ("AcPwrPlugins.lvlib:NHRGridSim.lvclass:NHRGrid_ModeAdjust_Tabs") NHRGrid_ModeAdjust_Tabs."TripTCoerce1" ("AcPwrPlugins.lvlib:NHRGridSim.lvclass:NHRGrid_ModeAdjust_Tabs") NHRGrid_ModeAdjust_Tabs."TripTCoerce2" ("AcPwrPlugins.lvlib:NHRGridSim.lvclass:NHRGrid_ModeAdjust_Tabs") NHRGrid_ModeAdjust_Tabs."TripTCoerce3" ("AcPwrPlugins.lvlib:NHRGridSim.lvclass:NHRGrid_ModeAdjust_Tabs") NHRGrid_ModeAdjust_Tabs."VPhaseCoerce" ("AcPwrPlugins.lvlib:NHRGridSim.lvclass:NHRGrid_ModeAdjust_Tabs") NHRGrid_ModeAdjust_Tabs."WaveLists" ("AcPwrPlugins.lvlib:NHRGridSim.lvclass:NHRGrid_ModeAdjust_Tabs") NHRGrid_ModeAdjust_Tabs."WaveEnable" ("AcPwrPlugins.lvlib:NHRGridSim.lvclass:NHRGrid_ModeAdjust_Tabs") NHRGrid_ModeAdjust_Tabs."ShowTabs" ("AcPwrPlugins.lvlib:NHRGridSim.lvclass:NHRGrid_ModeAdjust_Tabs")] -> w835
                    tunnel: [FALSE FALSE FALSE FALSE FALSE FALSE FALSE FALSE FALSE FALSE FALSE FALSE FALSE FALSE FALSE FALSE FALSE FALSE FALSE FALSE FALSE FALSE FALSE FALSE FALSE FALSE FALSE FALSE TRUE] -> w834
                    frame "ShowTabs", Default {
                      # "Get the reference of each instrument tab."
                      # "Store the visibility properties of the tabs so that they can be loaded from a config file the same way."
                      # "Mode determines number of instruments (and their respective tabs) visible on each configuration."
                      n369 = property on="Instruments" class="TabCtl (strict)"(error in=w847) -> (error out=w846:errorcluster, "Pages"=w849:refnum<vi>[])  [unwired: 1 in, 1 out]
                      n370 = local read "Mode"() -> (w848:T8)
                      n371 = for {
                        tunnel: w849 -> [w855] mode=indexing
                        tunnel: w848 -> [w856]
                        shift-right: [w852] -> w843
                        shift-left: w846 -> [w853]
                        tunnel: [w851] -> w842 mode=indexing
                        tunnel: [w850] -> w840
                        i -> [w854]
                        n372 = case shown="0..2, Default" w856 {
                          tunnel: w855 -> [w869 w883 w890]
                          tunnel: w854 -> [w864 w878 _]
                          tunnel: w853 -> [w862 w876 w888]
                          tunnel: [w861 w875 w887] -> w852
                          tunnel: [w860 w874 w886] -> w851
                          tunnel: [w857 w873 w884] -> w850
                          frame 0..2, Default {
                            w858 = FALSE ("x .or. y?")
                            # "Only Tab1 should be enabled"
                            n373 = Equal?(x=0, y=w864) -> (x = y?=w865:bool)
                            n374 = Select(t=TRUE ("x .or. y?"), s=w865, f=FALSE ("x .or. y?")) -> (s? t:f=w868:bool)
                            n375 = property class="Page"(reference=w869, error in=w862, "PageVis"=w868) -> (reference out=w860:refnum<vi>, error out=w861:errorcluster)
                            n376 = Build Array(TRUE ("x .or. y?"), w858, w858) -> (w857:bool[])
                          }
                          frame 5..8, 11, 12 {
                            # "Only tabs 1 and 3 should be enabled"
                            n377 = Equal?(x=1, y=w878) -> (x = y?=w879:bool)
                            n378 = Select(t=FALSE ("x .or. y?"), s=w879, f=TRUE ("x .or. y?")) -> (s? t:f=w882:bool)
                            n379 = property class="Page"(reference=w883, error in=w876, "PageVis"=w882) -> (reference out=w874:refnum<vi>, error out=w875:errorcluster)
                            n380 = Build Array(TRUE ("x .or. y?"), FALSE ("x .or. y?"), TRUE ("x .or. y?")) -> (w873:bool[])
                          }
                          frame 3, 4, 9, 10, 13..15 {
                            w885 = TRUE ("x .or. y?")
                            # "All three tabs should be enabled"
                            n381 = property class="Page"(reference=w890, error in=w888, "PageVis"=TRUE ("x .or. y?")) -> (reference out=w886:refnum<vi>, error out=w887:errorcluster)
                            n382 = Build Array(w885, w885, w885) -> (w884:bool[])
                          }
                        }
                      }
                      n383 = local read "Device(s)Settings"() -> (w841:T1)
                      n384 = Close Reference(reference=w842, error in (no error)=w843) -> (error out=w838:errorcluster)
                      n385 = Bundle By Name(cluster=w841, "TabPages"=w840) -> (w839:T1)
                      n386 = local write "Device(s)Settings"(w839) -> ()
                    }
                    frame "InstrNames" {
                      w899 = T15."Disabled" ("Disabled")
                      # "Store the same status given to the Name controls in Device(s)Settings for later retrieval."
                      # "Instr3"
                      # "Instr2"
                      # "Instr1"
                      # "In some Modes Instr2 becomes the same as Instr1"
                      # "Don't allow the user to alter the default name assigned to each instrument"
                      # "Logcial Instrument Name assigned for each Mode"
                      n387 = local read "Mode"() -> (w904:T8)
                      n388 = case shown="Default" w904 {
                        tunnel: w903 -> [w941 w945]
                        tunnel: [w941 w945] -> w902
                        frame Default {
                          n389 = local read "Instr1"() -> (w943:T2)
                          n390 = Bundle By Name(cluster=w943, "Name"="AC1") -> (w944:T2)
                          n391 = local write "Instr1"(w944) -> ()
                        }
                        frame 2, 4, 11, 12, 14, 15 {
                          n392 = local read "Instr1"() -> (w947:T2)
                          n393 = Bundle By Name(cluster=w947, "Name"="DC1") -> (w948:T2)
                          n394 = local write "Instr1"(w948) -> ()
                        }
                      }
                      n395 = case shown="Default" w904 {
                        tunnel: w902 -> [w925 w929 w933 w937]
                        tunnel: [w925 w929 w933 w937] -> w901
                        frame Default {
                          n396 = local read "Instr2"() -> (w927:T2)
                          n397 = Bundle By Name(cluster=w927, "Name"="AC1") -> (w928:T2)
                          n398 = local write "Instr2"(w928) -> ()
                        }
                        frame 2, 11, 12 {
                          n399 = local read "Instr2"() -> (w931:T2)
                          n400 = Bundle By Name(cluster=w931, "Name"="DC1") -> (w932:T2)
                          n401 = local write "Instr2"(w932) -> ()
                        }
                        frame 3, 9, 14, 15 {
                          n402 = local read "Instr2"() -> (w935:T2)
                          n403 = Bundle By Name(cluster=w935, "Name"="AC2") -> (w936:T2)
                          n404 = local write "Instr2"(w936) -> ()
                        }
                        frame 4, 10, 13 {
                          n405 = local read "Instr2"() -> (w939:T2)
                          n406 = Bundle By Name(cluster=w939, "Name"="DC2") -> (w940:T2)
                          n407 = local write "Instr2"(w940) -> ()
                        }
                      }
                      n408 = case shown="0, 1" w904 {
                        tunnel: w901 -> [w909 w913 w917 w921]
                        tunnel: [w909 w913 w917 w921] -> w894
                        frame Default {
                          n409 = local read "Instr3"() -> (w911:T2)
                          n410 = Bundle By Name(cluster=w911, "Name"="AC3") -> (w912:T2)
                          n411 = local write "Instr3"(w912) -> ()
                        }
                        frame 0, 1 {
                          n412 = local read "Instr3"() -> (w915:T2)
                          n413 = Bundle By Name(cluster=w915, "Name"="AC1") -> (w916:T2)
                          n414 = local write "Instr3"(w916) -> ()
                        }
                        frame 2 {
                          n415 = local read "Instr3"() -> (w919:T2)
                          n416 = Bundle By Name(cluster=w919, "Name"="DC1") -> (w920:T2)
                          n417 = local write "Instr3"(w920) -> ()
                        }
                        frame 4, 6, 8..10, 12 {
                          n418 = local read "Instr3"() -> (w923:T2)
                          n419 = Bundle By Name(cluster=w923, "Name"="DC3") -> (w924:T2)
                          n420 = local write "Instr3"(w924) -> ()
                        }
                      }
                      n421 = property on="Name" class="Str"(error in=w894, "DisabledEnum"=w899) -> (error out=w906:errorcluster)  [unwired: 1 in, 1 out]
                      n422 = local read "Device(s)Settings"() -> (w896:T1)
                      n423 = property on="Name" class="Str"(error in=w906, "DisabledEnum"=w899) -> (error out=w905:errorcluster)  [unwired: 1 in, 1 out]
                      n424 = Unbundle By Name(w896) -> ("EnableCtrls"=w900:i8[][])
                      n425 = Build Array(w899, w899, w899) -> (w897:T21)
                      n426 = property on="Name" class="Str"(error in=w905, "DisabledEnum"=w899) -> (error out=w891:errorcluster)  [unwired: 1 in, 1 out]
                      n427 = Replace Array Subset(array=w900, new element=w897, index (col)=0 ("disabled index (col)")) -> (w895:i8[][])  [unwired: 1 in]
                      n428 = property on="EnableCtrls" class="Arr (strict)"(error in=w894, "Value"=w895) -> (error out=w892:errorcluster)  [unwired: 1 in, 1 out]
                      n429 = Merge Errors(w892, w891) -> (w893:errorcluster)
                    }
                    frame "VoltRanges" {
                      # "Instr3"
                      # "Instr2"
                      # "Instr1"
                      # "Multiphase, single phase, and DC instruments have different voltage ranges"
                      n430 = flat-sequence {
                        tunnel: [w1017] -> w949
                        tunnel: w950 -> [w1017]
                        frame #0 {
                          # "Reinitialize all Vout values and set the voltage range in all instruments to the maximum."
                          n431 = local read "Instr1"() -> (w1028:T2)
                          n432 = Bundle By Name(cluster=w1028, "Vout (V)"=0.0 ("Value"), "Ranges.Voltage (V)"=u16 1) -> (w1029:T2)
                          n433 = local read "Instr3"() -> (w1020:T2)
                          n434 = Bundle By Name(cluster=w1020, "Vout (V)"=0.0 ("Value"), "Ranges.Voltage (V)"=u16 1) -> (w1021:T2)
                          n435 = local read "Instr2"() -> (w1023:T2)
                          n436 = Bundle By Name(cluster=w1023, "Vout (V)"=0.0 ("Value"), "Ranges.Voltage (V)"=u16 1) -> (w1022:T2)
                          n437 = local write "Instr1"(w1029) -> ()
                          n438 = local write "Instr3"(w1021) -> ()
                          n439 = local write "Instr2"(w1022) -> ()
                        }
                      }
                      n440 = local read "Mode"() -> (w954:T8)
                      n441 = case shown="1, 3, 7" w954 {
                        tunnel: [w960 w963 w966 w970 w976 w982 w988 w994 w999 w1006 w1011] -> w953
                        tunnel: [w960 w963 w966 w970 w976 w982 w987 w994 w1000 w1005 w1012] -> w952
                        tunnel: [w960 w963 w966 w969 w975 w981 w987 w993 w999 w1005 w1011] -> w951
                        frame 0, Default {
                          # "3-Phase is the only one with\n303/606 V range"
                          n442 = Build Array("303", "606") -> (w960:string[])
                        }
                        frame 1, 3, 7 {
                          # "All One-Phase AC 175/350 V"
                          n443 = Build Array("175", "350") -> (w963:string[])
                        }
                        frame 2, 4, 12 {
                          # "All DC 200/400 V"
                          n444 = Build Array("200", "400") -> (w966:string[])
                        }
                        frame 5 {
                          # "Two-Phase 350/500 V\n and One-Phase AC 175/350 V"
                          n445 = Build Array("350", "500") -> (w970:string[])
                          n446 = Build Array("175", "350") -> (w969:string[])
                        }
                        frame 6 {
                          # "Two-Phase 350/500 V\nand DC 200/400 V"
                          n447 = Build Array("350", "500") -> (w976:string[])
                          n448 = Build Array("200", "400") -> (w975:string[])
                        }
                        frame 8, 9 {
                          # "AC- AC- DC"
                          n449 = Build Array("175", "350") -> (w982:string[])
                          n450 = Build Array("200", "400") -> (w981:string[])
                        }
                        frame 10 {
                          # "AC - DC - DC"
                          n451 = Build Array("175", "350") -> (w988:string[])
                          n452 = Build Array("200", "400") -> (w987:string[])
                        }
                        frame 11 {
                          # "DC - DC - AC"
                          n453 = Build Array("200", "400") -> (w994:string[])
                          n454 = Build Array("175", "350") -> (w993:string[])
                        }
                        frame 13 {
                          # "AC - DC - AC"
                          n455 = Build Array("175", "350") -> (w999:string[])
                          n456 = Build Array("200", "400") -> (w1000:string[])
                        }
                        frame 14 {
                          # "DC - AC - AC"
                          n457 = Build Array("200", "400") -> (w1006:string[])
                          n458 = Build Array("175", "350") -> (w1005:string[])
                        }
                        frame 15 {
                          # "DC - AC - DC"
                          n459 = Build Array("200", "400") -> (w1011:string[])
                          n460 = Build Array("175", "350") -> (w1012:string[])
                        }
                      }
                      n461 = property on="Voltage (V)" class="Ring (strict)"(error in=w949, "Strings []"=w953) -> (error out=w956:errorcluster)  [unwired: 1 in, 1 out]
                      n462 = property on="Voltage (V)" class="Ring (strict)"(error in=w956, "Strings []"=w952) -> (error out=w957:errorcluster)  [unwired: 1 in, 1 out]
                      n463 = property on="Voltage (V)" class="Ring (strict)"(error in=w957, "Strings []"=w951) -> (error out=w955:errorcluster)  [unwired: 1 in, 1 out]
                    }
                    frame "ConfigSync" {
                      # "Set the values also in the Device(s)Settings instruments"
                      # "Set the Sync selections to be \"Immediate\" by default"
                      # "Instr3"
                      # "Instr2"
                      # "Instr1"
                      # "Multiphase instruments  will have a \"Sync to Phase A\" configuration available; Single phase ones will be just \"Sync\". For DC, this setting is irrelevant."
                      n464 = local read "Mode"() -> (w1043:T8)
                      n465 = case shown="Default" w1043 {
                        tunnel: [w1057 w1062 w1067] -> w1036
                        tunnel: [w1057 w1062 w1067] -> w1035
                        tunnel: [w1057 w1061 w1067] -> w1034
                        tunnel: w1040 -> [w1056 w1060 w1066]
                        tunnel: [w1056 w1060 w1066] -> w1033
                        frame 0 {
                          # "Three-phase Mode"
                          n466 = Build Array("Immediate" ("element"), "Sync to Phase A" ("element")) -> (w1057:string[])
                        }
                        frame 5, 6 {
                          w1063 = "Immediate" ("element")
                          # "Two-phase Mode for Instr1/2"
                          n467 = Build Array(w1063, "Sync to Phase A" ("element")) -> (w1062:string[])
                          n468 = Build Array(w1063, "Sync" ("element")) -> (w1061:string[])
                        }
                        frame Default {
                          # "Instruments with no phases"
                          n469 = Build Array("Immediate" ("element"), "Sync" ("element")) -> (w1067:string[])
                        }
                      }
                      n470 = property on="Synchronization" class="Ring (strict)"(error in=w1033, "Strings []"=w1036) -> (error out=w1041:errorcluster)  [unwired: 1 in, 1 out]
                      n471 = property on="Synchronization" class="Ring (strict)"(error in=w1033, "Strings []"=w1036) -> (error out=w1038:errorcluster)  [unwired: 1 in, 1 out]
                      n472 = property on="Synchronization" class="Ring (strict)"(error in=w1041, "Strings []"=w1035) -> (error out=w1042:errorcluster)  [unwired: 1 in, 1 out]
                      n473 = property on="Synchronization" class="Ring (strict)"(error in=w1038, "Strings []"=w1035) -> (error out=w1037:errorcluster)  [unwired: 1 in, 1 out]
                      n474 = property on="Synchronization" class="Ring (strict)"(error in=w1042, "Strings []"=w1034) -> (error out=w1031:errorcluster)  [unwired: 1 in, 1 out]
                      n475 = property on="Synchronization" class="Ring (strict)"(error in=w1037, "Strings []"=w1034) -> (error out=w1030:errorcluster)  [unwired: 1 in, 1 out]
                      n476 = Merge Errors(w1030, w1031) -> (w1032:errorcluster)
                      n477 = flat-sequence {
                        tunnel: w1032 -> [w1048]
                        tunnel: [w1048] -> w1039
                        frame #0 {
                          w1046 = T3 0 items=["Immediate", "Sync to Phase A"] ("Synchronization")
                          w1047 = T3 0 items=["Immediate", "Sync to Phase A"] ("Synchronization")
                          w1053 = T3 0 items=["Immediate", "Sync to Phase A"] ("Synchronization")
                          n478 = local read "Instr1"() -> (w1055:T2)
                          n479 = Bundle By Name(cluster=w1055, "Synchronization"=w1053) -> (w1054:T2)
                          n480 = local read "Instr2"() -> (w1051:T2)
                          n481 = Bundle By Name(cluster=w1051, "Synchronization"=w1047) -> (w1052:T2)
                          n482 = local read "Instr3"() -> (w1050:T2)
                          n483 = Bundle By Name(cluster=w1050, "Synchronization"=w1046) -> (w1049:T2)
                          n484 = local write "Instr1"(w1054) -> ()
                          n485 = local write "Instr2"(w1052) -> ()
                          n486 = local write "Instr3"(w1049) -> ()
                        }
                      }
                    }
                    frame "Safety" {
                      # "Instr3"
                      # "Instr2"
                      # "Instr1"
                      # "Recall the default cluster values for the \"Safety Trips\" in all instruments"
                      n487 = invoke on="Safety Trips" class="Clust (strict)" method="Reinit To Default"(error in=w1073) -> (error out=w1072:errorcluster)  [unwired: 2 in, 2 out]
                      n488 = invoke on="Safety Trips" class="Clust (strict)" method="Reinit To Default"(error in=w1072) -> (error out=w1071:errorcluster)  [unwired: 2 in, 2 out]
                      n489 = invoke on="Safety Trips" class="Clust (strict)" method="Reinit To Default"(error in=w1071) -> (error out=w1070:errorcluster)  [unwired: 2 in, 2 out]
                    }
                    frame "Phases" {
                      # "Set the default phase angles for the multiphase Mode cases. Also, initialize all phase voltage values to 0, and Apertures to 1"
                      n490 = local read "Mode"() -> (w1078:T8)
                      n491 = case shown="Default" w1078 {
                        tunnel: w1077 -> [w1088 w1098 w1110]
                        tunnel: [w1088 w1098 w1110] -> w1076
                        frame 0 {
                          w1081 = 0.0 ("Phases.B-Volts (V)")
                          w1082 = 0.0 ("Phases.B-Volts (V)")
                          w1083 = 0.0 ("Phases.B-Volts (V)")
                          w1087 = 120 ("Phases.C-Angle (Deg)")
                          w1089 = 240 ("Phases.B-Angle (Deg)")
                          # "Three Phase Mode: all Instrs have B=240, C=120 degrees"
                          n492 = local read "Instr1"() -> (w1090:T2)
                          n493 = Bundle By Name(cluster=w1090, "Phases.B-Angle (Deg)"=w1089, "Aperture (cycles)"=1, "Phases.A-Volts (V)"=w1083, "Phases.B-Volts (V)"=w1083, "Phases.C-Volts (V)"=w1083, "Phases.C-Angle (Deg)"=w1087) -> (w1091:T2)
                          n494 = local write "Instr1"(w1091) -> ()
                          n495 = local read "Instr2"() -> (w1093:T2)
                          n496 = Bundle By Name(cluster=w1093, "Phases.B-Angle (Deg)"=w1089, "Aperture (cycles)"=1, "Phases.A-Volts (V)"=w1082, "Phases.B-Volts (V)"=w1082, "Phases.C-Volts (V)"=w1082, "Phases.C-Angle (Deg)"=w1087) -> (w1092:T2)
                          n497 = local write "Instr2"(w1092) -> ()
                          n498 = local read "Instr3"() -> (w1094:T2)
                          n499 = Bundle By Name(cluster=w1094, "Phases.B-Angle (Deg)"=w1089, "Aperture (cycles)"=1, "Phases.A-Volts (V)"=w1081, "Phases.B-Volts (V)"=w1081, "Phases.C-Volts (V)"=w1081, "Phases.C-Angle (Deg)"=w1087) -> (w1095:T2)
                          n500 = local write "Instr3"(w1095) -> ()
                        }
                        frame Default {
                          w1096 = 1 ("Aperture (cycles)")
                          w1097 = 0 ("Phases.B-Angle (Deg)")
                          # "Modes with no phases: all Instrs to B=0, C=0"
                          n501 = local read "Instr1"() -> (w1099:T2)
                          n502 = Bundle By Name(cluster=w1099, "Phases.B-Angle (Deg)"=w1097, "Phases.C-Angle (Deg)"=w1097, "Phases.A-Volts (V)"=w1097, "Phases.B-Volts (V)"=w1097, "Phases.C-Volts (V)"=w1097, "Aperture (cycles)"=w1096) -> (w1100:T2)
                          n503 = local write "Instr1"(w1100) -> ()
                          n504 = local read "Instr2"() -> (w1102:T2)
                          n505 = Bundle By Name(cluster=w1102, "Phases.B-Angle (Deg)"=w1097, "Phases.C-Angle (Deg)"=w1097, "Phases.A-Volts (V)"=w1097, "Phases.B-Volts (V)"=w1097, "Phases.C-Volts (V)"=w1097, "Aperture (cycles)"=w1096) -> (w1101:T2)
                          n506 = local write "Instr2"(w1101) -> ()
                          n507 = local read "Instr3"() -> (w1103:T2)
                          n508 = Bundle By Name(cluster=w1103, "Phases.B-Angle (Deg)"=w1097, "Phases.C-Angle (Deg)"=w1097, "Phases.A-Volts (V)"=w1097, "Phases.B-Volts (V)"=w1097, "Phases.C-Volts (V)"=w1097, "Aperture (cycles)"=w1096) -> (w1104:T2)
                          n509 = local write "Instr3"(w1104) -> ()
                        }
                        frame 5, 6 {
                          w1109 = 0 ("Phases.C-Angle (Deg)")
                          w1107 = 180 ("Phases.B-Angle (Deg)")
                          # "Two Phase Modes, B=180 applies only for Instr1/2, all others are B=0, C=0"
                          n510 = local read "Instr1"() -> (w1111:T2)
                          n511 = Bundle By Name(cluster=w1111, "Phases.B-Angle (Deg)"=w1107, "Aperture (cycles)"=1, "Phases.C-Angle (Deg)"=w1109, "Phases.A-Volts (V)"=w1109, "Phases.B-Volts (V)"=w1109, "Phases.C-Volts (V)"=w1109) -> (w1112:T2)
                          n512 = local write "Instr1"(w1112) -> ()
                          n513 = local read "Instr2"() -> (w1114:T2)
                          n514 = Bundle By Name(cluster=w1114, "Phases.B-Angle (Deg)"=w1107, "Aperture (cycles)"=1 ("Phases.B-Angle (Deg)"), "Phases.C-Angle (Deg)"=w1109, "Phases.A-Volts (V)"=w1109, "Phases.B-Volts (V)"=w1109, "Phases.C-Volts (V)"=w1109) -> (w1113:T2)
                          n515 = local write "Instr2"(w1113) -> ()
                          n516 = local read "Instr3"() -> (w1115:T2)
                          n517 = Bundle By Name(cluster=w1115, "Aperture (cycles)"=1, "Phases.B-Angle (Deg)"=w1109, "Phases.C-Angle (Deg)"=w1109, "Phases.A-Volts (V)"=w1109, "Phases.B-Volts (V)"=w1109, "Phases.C-Volts (V)"=w1109) -> (w1116:T2)
                          n518 = local write "Instr3"(w1116) -> ()
                        }
                      }
                    }
                    frame "FreqOut" {
                      # "Store the same status given to the FreqOut controls in Device(s)Settings for later retrieval. Frequencies are column index 1 in the array."
                      # "Instr3"
                      # "Instr2"
                      # "Instr1"
                      # "0= Enabled       1= Disabled       2 = Disabled and Greyed Out"
                      # "AC instruments will have 60 Hz by default. Disable the DC ones."
                      n519 = local read "Mode"() -> (w1132:T8)
                      n520 = case shown="0, 1, 3, 5, 7, Default" w1132 {
                        tunnel: [w1138 w1158 w1178 w1199 w1220 w1241 w1262 w1283] -> w1121
                        tunnel: [w1137 w1157 w1177 w1198 w1219 w1240 w1261 w1282] -> w1122
                        tunnel: [w1136 w1156 w1176 w1197 w1218 w1239 w1260 w1281] -> w1123
                        tunnel: [w1135 w1155 w1175 w1196 w1217 w1238 w1259 w1280] -> w1120
                        tunnel: w1129 -> [w1135 w1155 w1175 w1196 w1217 w1238 w1259 w1280]
                        frame 0, 1, 3, 5, 7, Default {
                          w1139 = 60.0 ("x")
                          # "All AC instruments have 60 Hz default and Frequency setting enabled"
                          n521 = Not Equal To 0?(x=w1139) -> (x != 0?=w1151:bool)
                          n522 = local read "Instr1"() -> (w1153:T2)
                          n523 = Bundle By Name(cluster=w1153, "FreqOut (Hz)"=w1139) -> (w1154:T2)
                          n524 = Select(t=0.0, s=w1151, f=2.0) -> (s? t:f=w1136:dbl)
                          n525 = local write "Instr1"(w1154) -> ()
                          n526 = Not Equal To 0?(x=w1139) -> (x != 0?=w1148:bool)
                          n527 = local read "Instr2"() -> (w1146:T2)
                          n528 = Bundle By Name(cluster=w1146, "FreqOut (Hz)"=w1139) -> (w1145:T2)
                          n529 = Select(t=0.0, s=w1148, f=2.0) -> (s? t:f=w1137:dbl)
                          n530 = local write "Instr2"(w1145) -> ()
                          n531 = Not Equal To 0?(x=w1139) -> (x != 0?=w1141:bool)
                          n532 = local read "Instr3"() -> (w1143:T2)
                          n533 = Bundle By Name(cluster=w1143, "FreqOut (Hz)"=w1139) -> (w1144:T2)
                          n534 = Select(t=0.0, s=w1141, f=2.0) -> (s? t:f=w1138:dbl)
                          n535 = local write "Instr3"(w1144) -> ()
                        }
                        frame 2, 4, 12 {
                          w1159 = 0.0 ("x")
                          # "All DC instruments have 0 Hz default and Frequency setting disabled"
                          n536 = Not Equal To 0?(x=w1159) -> (x != 0?=w1171:bool)
                          n537 = local read "Instr1"() -> (w1173:T2)
                          n538 = Bundle By Name(cluster=w1173, "FreqOut (Hz)"=w1159) -> (w1174:T2)
                          n539 = Select(t=0.0, s=w1171, f=2.0) -> (s? t:f=w1156:dbl)
                          n540 = local write "Instr1"(w1174) -> ()
                          n541 = Not Equal To 0?(x=w1159) -> (x != 0?=w1168:bool)
                          n542 = local read "Instr2"() -> (w1166:T2)
                          n543 = Bundle By Name(cluster=w1166, "FreqOut (Hz)"=w1159) -> (w1165:T2)
                          n544 = Select(t=0.0, s=w1168, f=2.0) -> (s? t:f=w1157:dbl)
                          n545 = local write "Instr2"(w1165) -> ()
                          n546 = Not Equal To 0?(x=w1159) -> (x != 0?=w1161:bool)
                          n547 = local read "Instr3"() -> (w1163:T2)
                          n548 = Bundle By Name(cluster=w1163, "FreqOut (Hz)"=w1159) -> (w1164:T2)
                          n549 = Select(t=0.0, s=w1161, f=2.0) -> (s? t:f=w1158:dbl)
                          n550 = local write "Instr3"(w1164) -> ()
                        }
                        frame 6, 8, 9 {
                          w1179 = 0.0 ("x")
                          w1180 = 60.0 ("x")
                          # "Instruments are AC - AC - DC"
                          n551 = Not Equal To 0?(x=w1180) -> (x != 0?=w1192:bool)
                          n552 = local read "Instr1"() -> (w1194:T2)
                          n553 = Bundle By Name(cluster=w1194, "FreqOut (Hz)"=w1180) -> (w1195:T2)
                          n554 = Select(t=0.0, s=w1192, f=2.0) -> (s? t:f=w1176:dbl)
                          n555 = local write "Instr1"(w1195) -> ()
                          n556 = Not Equal To 0?(x=w1180) -> (x != 0?=w1189:bool)
                          n557 = local read "Instr2"() -> (w1187:T2)
                          n558 = Bundle By Name(cluster=w1187, "FreqOut (Hz)"=w1180) -> (w1186:T2)
                          n559 = Select(t=0.0, s=w1189, f=2.0) -> (s? t:f=w1177:dbl)
                          n560 = local write "Instr2"(w1186) -> ()
                          n561 = Not Equal To 0?(x=w1179) -> (x != 0?=w1182:bool)
                          n562 = local read "Instr3"() -> (w1184:T2)
                          n563 = Bundle By Name(cluster=w1184, "FreqOut (Hz)"=w1179) -> (w1185:T2)
                          n564 = Select(t=0.0, s=w1182, f=2.0) -> (s? t:f=w1178:dbl)
                          n565 = local write "Instr3"(w1185) -> ()
                        }
                        frame 10 {
                          w1200 = 0.0 ("x")
                          w1201 = 60.0 ("x")
                          # "Instruments are AC - DC - DC"
                          n566 = Not Equal To 0?(x=w1201) -> (x != 0?=w1213:bool)
                          n567 = local read "Instr1"() -> (w1215:T2)
                          n568 = Bundle By Name(cluster=w1215, "FreqOut (Hz)"=w1201) -> (w1216:T2)
                          n569 = Select(t=0.0, s=w1213, f=2.0) -> (s? t:f=w1197:dbl)
                          n570 = local write "Instr1"(w1216) -> ()
                          n571 = Not Equal To 0?(x=w1200) -> (x != 0?=w1210:bool)
                          n572 = local read "Instr2"() -> (w1208:T2)
                          n573 = Bundle By Name(cluster=w1208, "FreqOut (Hz)"=w1200) -> (w1207:T2)
                          n574 = Select(t=0.0, s=w1210, f=2.0) -> (s? t:f=w1198:dbl)
                          n575 = local write "Instr2"(w1207) -> ()
                          n576 = Not Equal To 0?(x=w1200) -> (x != 0?=w1203:bool)
                          n577 = local read "Instr3"() -> (w1205:T2)
                          n578 = Bundle By Name(cluster=w1205, "FreqOut (Hz)"=w1200) -> (w1206:T2)
                          n579 = Select(t=0.0, s=w1203, f=2.0) -> (s? t:f=w1199:dbl)
                          n580 = local write "Instr3"(w1206) -> ()
                        }
                        frame 11 {
                          w1222 = 60.0 ("x")
                          w1221 = 0.0 ("x")
                          # "Instruments are DC - DC - AC"
                          n581 = Not Equal To 0?(x=w1221) -> (x != 0?=w1234:bool)
                          n582 = local read "Instr1"() -> (w1236:T2)
                          n583 = Bundle By Name(cluster=w1236, "FreqOut (Hz)"=w1221) -> (w1237:T2)
                          n584 = Select(t=0.0, s=w1234, f=2.0) -> (s? t:f=w1218:dbl)
                          n585 = local write "Instr1"(w1237) -> ()
                          n586 = Not Equal To 0?(x=w1221) -> (x != 0?=w1231:bool)
                          n587 = local read "Instr2"() -> (w1229:T2)
                          n588 = Bundle By Name(cluster=w1229, "FreqOut (Hz)"=w1221) -> (w1228:T2)
                          n589 = Select(t=0.0, s=w1231, f=2.0) -> (s? t:f=w1219:dbl)
                          n590 = local write "Instr2"(w1228) -> ()
                          n591 = Not Equal To 0?(x=w1222) -> (x != 0?=w1224:bool)
                          n592 = local read "Instr3"() -> (w1226:T2)
                          n593 = Bundle By Name(cluster=w1226, "FreqOut (Hz)"=w1222) -> (w1227:T2)
                          n594 = Select(t=0.0, s=w1224, f=2.0) -> (s? t:f=w1220:dbl)
                          n595 = local write "Instr3"(w1227) -> ()
                        }
                        frame 13 {
                          w1243 = 0.0 ("x")
                          w1242 = 60.0 ("x")
                          # "Instruments are AC - DC - AC"
                          n596 = Not Equal To 0?(x=w1242) -> (x != 0?=w1255:bool)
                          n597 = local read "Instr1"() -> (w1257:T2)
                          n598 = Bundle By Name(cluster=w1257, "FreqOut (Hz)"=w1242) -> (w1258:T2)
                          n599 = Select(t=0.0, s=w1255, f=2.0) -> (s? t:f=w1239:dbl)
                          n600 = local write "Instr1"(w1258) -> ()
                          n601 = Not Equal To 0?(x=w1243) -> (x != 0?=w1252:bool)
                          n602 = local read "Instr2"() -> (w1250:T2)
                          n603 = Bundle By Name(cluster=w1250, "FreqOut (Hz)"=w1243) -> (w1249:T2)
                          n604 = Select(t=0.0, s=w1252, f=2.0) -> (s? t:f=w1240:dbl)
                          n605 = local write "Instr2"(w1249) -> ()
                          n606 = Not Equal To 0?(x=w1242) -> (x != 0?=w1245:bool)
                          n607 = local read "Instr3"() -> (w1247:T2)
                          n608 = Bundle By Name(cluster=w1247, "FreqOut (Hz)"=w1242) -> (w1248:T2)
                          n609 = Select(t=0.0, s=w1245, f=2.0) -> (s? t:f=w1241:dbl)
                          n610 = local write "Instr3"(w1248) -> ()
                        }
                        frame 14 {
                          w1263 = 60.0 ("x")
                          w1264 = 0.0 ("x")
                          # "Instruments are DC - AC - AC"
                          n611 = Not Equal To 0?(x=w1264) -> (x != 0?=w1276:bool)
                          n612 = local read "Instr1"() -> (w1278:T2)
                          n613 = Bundle By Name(cluster=w1278, "FreqOut (Hz)"=w1264) -> (w1279:T2)
                          n614 = Select(t=0.0, s=w1276, f=2.0) -> (s? t:f=w1260:dbl)
                          n615 = local write "Instr1"(w1279) -> ()
                          n616 = Not Equal To 0?(x=w1263) -> (x != 0?=w1273:bool)
                          n617 = local read "Instr2"() -> (w1271:T2)
                          n618 = Bundle By Name(cluster=w1271, "FreqOut (Hz)"=w1263) -> (w1270:T2)
                          n619 = Select(t=0.0, s=w1273, f=2.0) -> (s? t:f=w1261:dbl)
                          n620 = local write "Instr2"(w1270) -> ()
                          n621 = Not Equal To 0?(x=w1263) -> (x != 0?=w1266:bool)
                          n622 = local read "Instr3"() -> (w1268:T2)
                          n623 = Bundle By Name(cluster=w1268, "FreqOut (Hz)"=w1263) -> (w1269:T2)
                          n624 = Select(t=0.0, s=w1266, f=2.0) -> (s? t:f=w1262:dbl)
                          n625 = local write "Instr3"(w1269) -> ()
                        }
                        frame 15 {
                          w1285 = 60.0 ("x")
                          w1284 = 0.0 ("x")
                          # "Instruments are DC - AC - DC"
                          n626 = Not Equal To 0?(x=w1284) -> (x != 0?=w1297:bool)
                          n627 = local read "Instr1"() -> (w1299:T2)
                          n628 = Bundle By Name(cluster=w1299, "FreqOut (Hz)"=w1284) -> (w1300:T2)
                          n629 = Select(t=0.0, s=w1297, f=2.0) -> (s? t:f=w1281:dbl)
                          n630 = local write "Instr1"(w1300) -> ()
                          n631 = Not Equal To 0?(x=w1285) -> (x != 0?=w1294:bool)
                          n632 = local read "Instr2"() -> (w1292:T2)
                          n633 = Bundle By Name(cluster=w1292, "FreqOut (Hz)"=w1285) -> (w1291:T2)
                          n634 = Select(t=0.0, s=w1294, f=2.0) -> (s? t:f=w1282:dbl)
                          n635 = local write "Instr2"(w1291) -> ()
                          n636 = Not Equal To 0?(x=w1284) -> (x != 0?=w1287:bool)
                          n637 = local read "Instr3"() -> (w1289:T2)
                          n638 = Bundle By Name(cluster=w1289, "FreqOut (Hz)"=w1284) -> (w1290:T2)
                          n639 = Select(t=0.0, s=w1287, f=2.0) -> (s? t:f=w1283:dbl)
                          n640 = local write "Instr3"(w1290) -> ()
                        }
                      }
                      n641 = property on="FreqOut (Hz)" class="DigNum (strict)"(error in=w1120, "DisabledEnum"=w1123) -> (error out=w1130:errorcluster)  [unwired: 1 in, 1 out]
                      n642 = property on="EnableCtrls" class="Arr (strict)"(error in=w1120) -> (error out=w1125:errorcluster, "Value"=w1126:i8[][])  [unwired: 1 in, 1 out]
                      n643 = Build Array(w1123, w1122, w1121) -> (w1127:dbl[])
                      n644 = property on="FreqOut (Hz)" class="DigNum (strict)"(error in=w1130, "DisabledEnum"=w1122) -> (error out=w1131:errorcluster)  [unwired: 1 in, 1 out]
                      n645 = Replace Array Subset(array=w1126, new element=w1127, index (col)=1 ("disabled index (col)")) -> (w1124:i8[][])  [unwired: 1 in]
                      n646 = property on="FreqOut (Hz)" class="DigNum (strict)"(error in=w1131, "DisabledEnum"=w1121) -> (error out=w1119:errorcluster)  [unwired: 1 in, 1 out]
                      n647 = property on="EnableCtrls" class="Arr (strict)"(error in=w1125, "Value"=w1124) -> (error out=w1118:errorcluster)  [unwired: 1 in, 1 out]
                      n648 = Merge Errors(w1119, w1118) -> (w1117:errorcluster)
                    }
                    frame "PhaseEnable" {
                      # "Store the same status given to the phase angle controls in Device(s)Settings for later retrieval. These are column indexes 6 and 7 in the array."
                      # "Instr3"
                      # "Instr2"
                      # "Instr1"
                      # "The Phase shift angles are only meaningful for the multiphase cases"
                      n649 = local read "Mode"() -> (w1325:T8)
                      n650 = case shown="Default" w1325 {
                        tunnel: [w1330 w1332 w1334] -> w1308
                        tunnel: [w1329 w1332 w1334] -> w1305
                        tunnel: [w1330 w1332 w1334] -> w1309
                        tunnel: [w1329 w1332 w1334] -> w1306
                        tunnel: [w1329 w1332 w1334] -> w1310
                        tunnel: [w1329 w1332 w1334] -> w1307
                        tunnel: w1319 -> [w1328 w1331 w1333]
                        tunnel: [w1328 w1331 w1333] -> w1318
                        frame 5, 6 {
                          w1329 = T15."Disabled and Grayed Out" ("Disabled")
                          w1330 = T15."Enabled" ("Disabled")
                          # "The Two-Phase Modes need only the B-Angle, and only for Instr1/2"
                        }
                        frame 0 {
                          w1332 = T15."Enabled" ("Disabled")
                          # "The three phase Mode needs both angles for Instr1/2/3"
                        }
                        frame Default {
                          w1334 = T15."Disabled and Grayed Out" ("Disabled")
                          # "B-Angle and C-Angle are not used\nfor most of the Modes"
                        }
                      }
                      n651 = property on="B-Angle (Deg)" class="DigNum (strict)"(error in=w1318, "DisabledEnum"=w1308) -> (error out=w1320:errorcluster)  [unwired: 1 in, 1 out]
                      n652 = property on="C-Angle (Deg)" class="DigNum (strict)"(error in=w1320, "DisabledEnum"=w1305) -> (error out=w1321:errorcluster)  [unwired: 1 in, 1 out]
                      n653 = property on="B-Angle (Deg)" class="DigNum (strict)"(error in=w1321, "DisabledEnum"=w1309) -> (error out=w1322:errorcluster)  [unwired: 1 in, 1 out]
                      n654 = property on="C-Angle (Deg)" class="DigNum (strict)"(error in=w1322, "DisabledEnum"=w1306) -> (error out=w1323:errorcluster)  [unwired: 1 in, 1 out]
                      n655 = property on="B-Angle (Deg)" class="DigNum (strict)"(error in=w1323, "DisabledEnum"=w1310) -> (error out=w1324:errorcluster)  [unwired: 1 in, 1 out]
                      n656 = Build Array(w1308, w1309, w1310) -> (w1317:T21)
                      n657 = property on="C-Angle (Deg)" class="DigNum (strict)"(error in=w1324, "DisabledEnum"=w1307) -> (error out=w1303:errorcluster)  [unwired: 1 in, 1 out]
                      n658 = property on="EnableCtrls" class="Arr (strict)"(error in=w1303) -> (error out=w1316:errorcluster, "Value"=w1315:i8[][])  [unwired: 1 in, 1 out]
                      n659 = Build Array(w1305, w1306, w1307) -> (w1304:T21)
                      n660 = Replace Array Subset(array=w1315, new element=w1317, index (col)=6 ("disabled index (col)")) -> (w1312:i8[][])  [unwired: 1 in]
                      n661 = Replace Array Subset(array=w1312, new element=w1304, index (col)=7 ("disabled index (col)")) -> (w1311:i8[][])  [unwired: 1 in]
                      n662 = property on="EnableCtrls" class="Arr (strict)"(error in=w1316, "Value"=w1311) -> (error out=w1302:errorcluster)  [unwired: 1 in, 1 out]
                      n663 = Merge Errors(w1302, w1303) -> (w1301:errorcluster)
                    }
                    frame "SyncEnable" {
                      # "Store the same status given to the Synchronization controls in Device(s)Settings for later retrieval. Synchronizations are column index 2 in the array."
                      # "Instr3"
                      # "Instr2"
                      # "Instr1"
                      # "Synchronization settings are irrelevant for DC instruments. Enable it only for AC ones."
                      n664 = local read "Mode"() -> (w1349:T8)
                      n665 = case shown="0, 1, 3, 5, 7, Default" w1349 {
                        tunnel: [w1353 w1355 w1358 w1361 T15."Enabled" ("Disabled") w1365 w1368 T15."Disabled and Grayed Out" ("Disabled")] -> w1337
                        tunnel: [w1353 w1355 w1358 w1361 w1362 T15."Disabled and Grayed Out" ("Disabled") T15."Enabled" ("Disabled") w1371] -> w1338
                        tunnel: [w1353 w1355 T15."Disabled and Grayed Out" ("Disabled") T15."Enabled" ("Disabled") w1362 w1365 w1368 w1371] -> w1339
                        tunnel: w1348 -> [w1352 w1354 w1357 w1360 w1363 w1367 w1370 w1373]
                        tunnel: [w1352 w1354 w1357 w1360 w1363 w1367 w1370 w1373] -> w1347
                        frame 0, 1, 3, 5, 7, Default {
                          w1353 = T15."Enabled" ("Disabled")
                          # "AC - AC - AC"
                        }
                        frame 2, 4, 12 {
                          w1355 = T15."Disabled and Grayed Out" ("Disabled")
                          # "DC - DC - DC"
                        }
                        frame 6, 8, 9 {
                          w1358 = T15."Enabled" ("Disabled")
                          # "AC - AC - DC"
                        }
                        frame 11 {
                          w1361 = T15."Disabled and Grayed Out" ("Disabled")
                          # "DC - DC - AC"
                        }
                        frame 10 {
                          w1362 = T15."Disabled and Grayed Out" ("Disabled")
                          # "AC - DC - DC"
                        }
                        frame 13 {
                          w1365 = T15."Enabled" ("Disabled")
                          # "AC - DC - AC"
                        }
                        frame 15 {
                          w1368 = T15."Disabled and Grayed Out" ("Disabled")
                          # "DC - AC - DC"
                        }
                        frame 14 {
                          w1371 = T15."Enabled" ("Disabled")
                          # "DC - AC - AC"
                        }
                      }
                      n666 = property on="Synchronization" class="Ring (strict)"(error in=w1347, "DisabledEnum"=w1337) -> (error out=w1346:errorcluster)  [unwired: 1 in, 1 out]
                      n667 = property on="Synchronization" class="Ring (strict)"(error in=w1346, "DisabledEnum"=w1338) -> (error out=w1345:errorcluster)  [unwired: 1 in, 1 out]
                      n668 = property on="Synchronization" class="Ring (strict)"(error in=w1345, "DisabledEnum"=w1339) -> (error out=w1336:errorcluster)  [unwired: 1 in, 1 out]
                      n669 = Build Array(w1337, w1338, w1339) -> (w1344:T21)
                      n670 = property on="EnableCtrls" class="Arr (strict)"(error in=w1336) -> (error out=w1343:errorcluster, "Value"=w1342:i8[][])  [unwired: 1 in, 1 out]
                      n671 = Replace Array Subset(array=w1342, new element=w1344, index (col)=2 ("disabled index (col)")) -> (w1341:i8[][])  [unwired: 1 in]
                      n672 = property on="EnableCtrls" class="Arr (strict)"(error in=w1343, "Value"=w1341) -> (error out=w1335:errorcluster)  [unwired: 1 in, 1 out]
                    }
                    frame "ChangeEnable" {
                      w1375 = T15."Disabled and Grayed Out" ("Disabled")
                      w1395 = 0 ("Value")
                      w1400 = 0 ("Value")
                      w1401 = 0 ("Value")
                      # "Store the same status given to the 'Change at' controls in Device(s)Settings for later retrieval. Changes are column indexes 8, 9, & 10 in the array."
                      # "Since all instruments were set to have Synchronization as \"Immediate\" by default, the angle setting doesn't need to be used until the user either selects \"Sync\" or \"Synct to Phase A\" later to set the values. Therefore, have them all initially disabled."
                      # "Initialize all changes to 0 degrees"
                      # "\"Change at\" is only used for AC instruments, but by default all instruments will have their controls disabled."
                      n673 = property on="A-Change at..." class="DigNum (strict)"(error in=w1386, "DisabledEnum"=w1375) -> (error out=w1387:errorcluster)  [unwired: 1 in, 1 out]
                      n674 = local read "Instr1"() -> (w1402:T2)
                      n675 = Bundle By Name(cluster=w1402, "Phases.A-Change at..."=w1401, "Phases.B-Change at..."=w1401, "Phases.C-Change at..."=w1401) -> (w1403:T2)
                      n676 = property on="B-Change at..." class="DigNum (strict)"(error in=w1387, "DisabledEnum"=w1375) -> (error out=w1388:errorcluster)  [unwired: 1 in, 1 out]
                      n677 = property on="C-Change at..." class="DigNum (strict)"(error in=w1388, "DisabledEnum"=w1375) -> (error out=w1389:errorcluster)  [unwired: 1 in, 1 out]
                      n678 = local write "Instr1"(w1403) -> ()
                      n679 = property on="A-Change at..." class="DigNum (strict)"(error in=w1389, "DisabledEnum"=w1375) -> (error out=w1390:errorcluster)  [unwired: 1 in, 1 out]
                      n680 = local read "Instr2"() -> (w1399:T2)
                      n681 = Bundle By Name(cluster=w1399, "Phases.A-Change at..."=w1400, "Phases.B-Change at..."=w1400, "Phases.C-Change at..."=w1400) -> (w1398:T2)
                      n682 = property on="B-Change at..." class="DigNum (strict)"(error in=w1390, "DisabledEnum"=w1375) -> (error out=w1391:errorcluster)  [unwired: 1 in, 1 out]
                      n683 = property on="C-Change at..." class="DigNum (strict)"(error in=w1391, "DisabledEnum"=w1375) -> (error out=w1392:errorcluster)  [unwired: 1 in, 1 out]
                      n684 = local write "Instr2"(w1398) -> ()
                      n685 = property on="A-Change at..." class="DigNum (strict)"(error in=w1392, "DisabledEnum"=w1375) -> (error out=w1393:errorcluster)  [unwired: 1 in, 1 out]
                      n686 = local read "Instr3"() -> (w1396:T2)
                      n687 = Bundle By Name(cluster=w1396, "Phases.A-Change at..."=w1395, "Phases.B-Change at..."=w1395, "Phases.C-Change at..."=w1395) -> (w1397:T2)
                      n688 = property on="B-Change at..." class="DigNum (strict)"(error in=w1393, "DisabledEnum"=w1375) -> (error out=w1394:errorcluster)  [unwired: 1 in, 1 out]
                      n689 = property on="C-Change at..." class="DigNum (strict)"(error in=w1394, "DisabledEnum"=w1375) -> (error out=w1376:errorcluster)  [unwired: 1 in, 1 out]
                      n690 = local write "Instr3"(w1397) -> ()
                      n691 = Build Array(w1375, w1375, w1375) -> (w1374:T21)
                      n692 = property on="EnableCtrls" class="Arr (strict)"(error in=w1376) -> (error out=w1382:errorcluster, "Value"=w1381:i8[][])  [unwired: 1 in, 1 out]
                      n693 = Replace Array Subset(array=w1381, new element=w1374, index (col)=8 ("disabled index (col)")) -> (w1383:i8[][])  [unwired: 1 in]
                      n694 = Replace Array Subset(array=w1383, new element=w1374, index (col)=9 ("disabled index (col)")) -> (w1384:i8[][])  [unwired: 1 in]
                      n695 = Replace Array Subset(array=w1384, new element=w1374, index (col)=10 ("disabled index (col)")) -> (w1385:i8[][])  [unwired: 1 in]
                      n696 = property on="EnableCtrls" class="Arr (strict)"(error in=w1382, "Value"=w1385) -> (error out=w1377:errorcluster)  [unwired: 1 in, 1 out]
                    }
                    frame "VoltsEnable" {
                      # "Store the same status given to the phase voltage controls in Device(s)Settings for later retrieval. Phase Vs are column indexes 3, 4, & 5 in the array."
                      # "2 = Disabled and Greyed"
                      # "Instr3"
                      # "Instr2"
                      # "Instr1"
                      # "Phase voltages should be used only for multi-phase Modes"
                      n697 = local read "Mode"() -> (w1438:T8)
                      n698 = case shown="Default" w1438 {
                        tunnel: [w1441 w1444 w1447] -> w1416
                        tunnel: [w1441 w1444 w1447] -> w1413
                        tunnel: [w1441 w1444 w1445] -> w1409
                        tunnel: [w1441 w1444 w1447] -> w1415
                        tunnel: [w1441 w1444 w1447] -> w1412
                        tunnel: [w1441 w1444 w1445] -> w1408
                        tunnel: [w1441 w1444 w1445] -> w1414
                        tunnel: [w1441 w1444 w1445] -> w1411
                        tunnel: [w1441 w1444 w1445] -> w1407
                        tunnel: w1428 -> [w1442 w1443 w1446]
                        tunnel: [w1442 w1443 w1446] -> w1429
                        frame Default {
                          w1441 = u8 2
                          # "Most Mode cases\ndon't have phases"
                        }
                        frame 0 {
                          w1444 = T15."Enabled" ("Disabled")
                          # "The three phase Mode"
                        }
                        frame 5, 6 {
                          w1445 = u8 2
                          w1447 = T15."Enabled" ("Disabled")
                          # "The two phase\nA and B for Instr1/2"
                        }
                      }
                      n699 = property on="A-Volts (V)" class="DigNum (strict)"(error in=w1429, "DisabledEnum"=w1416) -> (error out=w1437:errorcluster)  [unwired: 1 in, 1 out]
                      n700 = property on="B-Volts (V)" class="DigNum (strict)"(error in=w1437, "DisabledEnum"=w1413) -> (error out=w1436:errorcluster)  [unwired: 1 in, 1 out]
                      n701 = property on="C-Volts (V)" class="DigNum (strict)"(error in=w1436, "DisabledEnum"=w1409) -> (error out=w1435:errorcluster)  [unwired: 1 in, 1 out]
                      n702 = property on="A-Volts (V)" class="DigNum (strict)"(error in=w1435, "DisabledEnum"=w1415) -> (error out=w1434:errorcluster)  [unwired: 1 in, 1 out]
                      n703 = property on="B-Volts (V)" class="DigNum (strict)"(error in=w1434, "DisabledEnum"=w1412) -> (error out=w1433:errorcluster)  [unwired: 1 in, 1 out]
                      n704 = property on="C-Volts (V)" class="DigNum (strict)"(error in=w1433, "DisabledEnum"=w1408) -> (error out=w1432:errorcluster)  [unwired: 1 in, 1 out]
                      n705 = property on="A-Volts (V)" class="DigNum (strict)"(error in=w1432, "DisabledEnum"=w1414) -> (error out=w1431:errorcluster)  [unwired: 1 in, 1 out]
                      n706 = property on="B-Volts (V)" class="DigNum (strict)"(error in=w1431, "DisabledEnum"=w1411) -> (error out=w1430:errorcluster)  [unwired: 1 in, 1 out]
                      n707 = property on="C-Volts (V)" class="DigNum (strict)"(error in=w1430, "DisabledEnum"=w1407) -> (error out=w1418:errorcluster)  [unwired: 1 in, 1 out]
                      n708 = Build Array(w1416, w1415, w1414) -> (w1422:u8[])
                      n709 = Build Array(w1413, w1412, w1411) -> (w1410:u8[])
                      n710 = Build Array(w1409, w1408, w1407) -> (w1406:u8[])
                      n711 = property on="EnableCtrls" class="Arr (strict)"(error in=w1418) -> (error out=w1424:errorcluster, "Value"=w1423:i8[][])  [unwired: 1 in, 1 out]
                      n712 = Replace Array Subset(array=w1423, new element=w1422, index (col)=3 ("disabled index (col)")) -> (w1425:i8[][])  [unwired: 1 in]
                      n713 = Replace Array Subset(array=w1425, new element=w1410, index (col)=4 ("disabled index (col)")) -> (w1426:i8[][])  [unwired: 1 in]
                      n714 = Replace Array Subset(array=w1426, new element=w1406, index (col)=5 ("disabled index (col)")) -> (w1427:i8[][])  [unwired: 1 in]
                      n715 = property on="EnableCtrls" class="Arr (strict)"(error in=w1424, "Value"=w1427) -> (error out=w1417:errorcluster)  [unwired: 1 in, 1 out]
                    }
                    frame "Vtype" {
                      # "Notify the user about the instrument voltage reference for the Vout value"
                      n716 = local read "Mode"() -> (w1450:T8)
                      n717 = case shown="Default" w1450 {
                        selector: w1450 -> [w1455 _]
                        tunnel: w1449 -> [w1453 w1465]
                        tunnel: [w1453 w1465] -> w1448
                        frame 0, 5, 6 {
                          w1457 = "(L-L)" ("element")
                          # "Multiphase cases have Vout as Line-to-Line between phases"
                          n718 = Equal To 0?(x=w1455) -> (x = 0?=w1458:bool)
                          n719 = Select(t=w1457, s=w1458, f="(L-N)" ("element")) -> (s? t:f=w1456:string)
                          n720 = local read "Instr1"() -> (w1463:T2)
                          n721 = local read "Instr2"() -> (w1462:T2)
                          n722 = local read "Instr3"() -> (w1459:T2)
                          n723 = Bundle By Name(cluster=w1463, "VType"=w1457) -> (w1464:T2)
                          n724 = Bundle By Name(cluster=w1462, "VType"=w1457) -> (w1461:T2)
                          n725 = Bundle By Name(cluster=w1459, "VType"=w1456) -> (w1460:T2)
                          n726 = local write "Instr1"(w1464) -> ()
                          n727 = local write "Instr2"(w1461) -> ()
                          n728 = local write "Instr3"(w1460) -> ()
                        }
                        frame Default {
                          w1466 = "(L-N)" ("element")
                          # "For all other instances Vout is Line-to-Neutral"
                          n729 = local read "Instr1"() -> (w1471:T2)
                          n730 = local read "Instr2"() -> (w1470:T2)
                          n731 = local read "Instr3"() -> (w1467:T2)
                          n732 = Bundle By Name(cluster=w1471, "VType"=w1466) -> (w1472:T2)
                          n733 = Bundle By Name(cluster=w1470, "VType"=w1466) -> (w1469:T2)
                          n734 = Bundle By Name(cluster=w1467, "VType"=w1466) -> (w1468:T2)
                          n735 = local write "Instr1"(w1472) -> ()
                          n736 = local write "Instr2"(w1469) -> ()
                          n737 = local write "Instr3"(w1468) -> ()
                        }
                      }
                    }
                    frame "Description" {
                      # "Give a better description of the instrument in its Tab caption than the default Instrumnet name"
                      n738 = property on="Instruments" class="TabCtl (strict)"(error in=w1483) -> (error out=w1482:errorcluster, "Pages"=w1485:refnum<vi>[])  [unwired: 1 in, 1 out]
                      n739 = local read "Mode"() -> (w1484:T8)
                      n740 = for {
                        tunnel: w1485 -> [w1494] mode=indexing
                        tunnel: w1484 -> [w1495]
                        shift-right: [w1491] -> w1475
                        shift-left: w1482 -> [w1492]
                        tunnel: "Three-Phase AC" ("element") -> [w1490]
                        tunnel: "One-Phase AC" ("element") -> [w1489]
                        tunnel: "DC Source" ("element") -> [w1488]
                        tunnel: "Two-Phase AC" ("element") -> [w1487]
                        tunnel: [w1486] -> w1473 mode=indexing
                        i -> [w1493]
                        n741 = case shown="1" w1495 {
                          tunnel: w1494 -> [w1503 w1511 w1519 w1527 w1535 w1550 w1565 w1580 w1595 w1608 w1621 w1634 w1647 w1660 w1673 w1686]
                          tunnel: w1493 -> [_ _ _ _ _ w1546 w1561 w1576 w1591 w1601 w1613 w1626 w1640 w1649 w1662 w1675]
                          tunnel: w1492 -> [w1502 w1510 w1518 w1526 w1534 w1549 w1564 w1579 w1594 w1607 w1620 w1633 w1646 w1659 w1672 w1685]
                          tunnel: [w1501 w1509 w1517 w1525 w1533 w1548 w1563 w1578 w1593 w1606 w1619 w1632 w1645 w1658 w1671 w1684] -> w1491
                          tunnel: w1490 -> [w1498 _ _ _ _ _ _ _ _ _ _ _ _ _ _ _]
                          tunnel: w1489 -> [_ w1506 _ w1522 _ w1541 w1556 _ w1582 w1598 w1616 w1630 _ w1655 w1668 w1682]
                          tunnel: w1488 -> [_ _ w1513 _ w1529 _ w1552 w1567 w1583 _ w1617 w1629 w1636 w1656 w1669 w1681]
                          tunnel: w1487 -> [_ _ _ _ _ w1538 _ w1569 _ _ _ _ _ _ _ _]
                          tunnel: [w1496 w1504 w1512 w1520 w1528 w1536 w1551 w1566 w1581 w1596 w1609 w1622 w1635 w1648 w1661 w1674] -> w1486
                          frame 0, Default {
                            n742 = Concatenate Strings(w1498, " (3Ch)" ("string")) -> (w1499:string)
                            n743 = property class="Page"(reference=w1503, error in=w1502, "IndependentLabel"=TRUE ("Independent Label"), "TabCaption"=w1499) -> (reference out=w1496:refnum<vi>, error out=w1501:errorcluster)
                          }
                          frame 1 {
                            n744 = Concatenate Strings(w1506, " (3Ch)" ("string")) -> (w1505:string)
                            n745 = property class="Page"(reference=w1511, error in=w1510, "TabCaption"=w1505, "IndependentLabel"=TRUE ("Independent Label")) -> (reference out=w1504:refnum<vi>, error out=w1509:errorcluster)
                          }
                          frame 2 {
                            n746 = Concatenate Strings(w1513, " (3Ch)" ("string")) -> (w1514:string)
                            n747 = property class="Page"(reference=w1519, error in=w1518, "TabCaption"=w1514, "IndependentLabel"=TRUE ("Independent Label")) -> (reference out=w1512:refnum<vi>, error out=w1517:errorcluster)
                          }
                          frame 3 {
                            n748 = Concatenate Strings(w1522, " (1Ch)" ("string")) -> (w1521:string)
                            n749 = property class="Page"(reference=w1527, error in=w1526, "TabCaption"=w1521, "IndependentLabel"=TRUE ("Independent Label")) -> (reference out=w1520:refnum<vi>, error out=w1525:errorcluster)
                          }
                          frame 4 {
                            n750 = Concatenate Strings(w1529, " (1Ch)" ("string")) -> (w1530:string)
                            n751 = property class="Page"(reference=w1535, error in=w1534, "TabCaption"=w1530, "IndependentLabel"=TRUE ("Independent Label")) -> (reference out=w1528:refnum<vi>, error out=w1533:errorcluster)
                          }
                          frame 5 {
                            n752 = Equal?(x=w1546, y=2 ("x")) -> (x = y?=w1537:bool)
                            n753 = Concatenate Strings(w1541, " (1Ch)" ("string")) -> (w1543:string)
                            n754 = Concatenate Strings(w1538, " (2Ch)" ("string")) -> (w1540:string)
                            n755 = Select(t=w1543, s=w1537, f=w1540) -> (s? t:f=w1544:string)
                            n756 = property class="Page"(reference=w1550, error in=w1549, "TabCaption"=w1544, "IndependentLabel"=TRUE ("Independent Label")) -> (reference out=w1536:refnum<vi>, error out=w1548:errorcluster)
                          }
                          frame 11 {
                            n757 = Equal?(x=w1561, y=2 ("x")) -> (x = y?=w1553:bool)
                            n758 = Concatenate Strings(w1556, " (1Ch)" ("string")) -> (w1558:string)
                            n759 = Concatenate Strings(w1552, " (2Ch)" ("string")) -> (w1555:string)
                            n760 = Select(t=w1558, s=w1553, f=w1555) -> (s? t:f=w1559:string)
                            n761 = property class="Page"(reference=w1565, error in=w1564, "TabCaption"=w1559, "IndependentLabel"=TRUE ("Independent Label")) -> (reference out=w1551:refnum<vi>, error out=w1563:errorcluster)
                          }
                          frame 6 {
                            n762 = Equal?(x=w1576, y=2 ("x")) -> (x = y?=w1568:bool)
                            n763 = Concatenate Strings(w1567, " (1Ch)" ("string")) -> (w1573:string)
                            n764 = Concatenate Strings(w1569, " (2Ch)" ("string")) -> (w1571:string)
                            n765 = Select(t=w1573, s=w1568, f=w1571) -> (s? t:f=w1574:string)
                            n766 = property class="Page"(reference=w1580, error in=w1579, "TabCaption"=w1574, "IndependentLabel"=TRUE ("Independent Label")) -> (reference out=w1566:refnum<vi>, error out=w1578:errorcluster)
                          }
                          frame 8 {
                            n767 = Equal?(x=w1591, y=2 ("x")) -> (x = y?=w1584:bool)
                            n768 = Concatenate Strings(w1583, " (1Ch)" ("string")) -> (w1588:string)
                            n769 = Concatenate Strings(w1582, " (2Ch)" ("string")) -> (w1586:string)
                            n770 = Select(t=w1588, s=w1584, f=w1586) -> (s? t:f=w1589:string)
                            n771 = property class="Page"(reference=w1595, error in=w1594, "TabCaption"=w1589, "IndependentLabel"=TRUE ("Independent Label")) -> (reference out=w1581:refnum<vi>, error out=w1593:errorcluster)
                          }
                          frame 7 {
                            n772 = Equal?(x=w1601, y=2 ("x")) -> (x = y?=w1604:bool)
                            n773 = Select(t=" (1Ch)" ("string"), s=w1604, f=" (2Ch)" ("string")) -> (s? t:f=w1597:string)
                            n774 = Concatenate Strings(w1598, w1597) -> (w1599:string)
                            n775 = property class="Page"(reference=w1608, error in=w1607, "TabCaption"=w1599, "IndependentLabel"=TRUE ("Independent Label")) -> (reference out=w1596:refnum<vi>, error out=w1606:errorcluster)
                          }
                          frame 9 {
                            n776 = Equal?(x=w1613, y=2 ("x")) -> (x = y?=w1618:bool)
                            n777 = Select(t=w1617, s=w1618, f=w1616) -> (s? t:f=w1611:string)
                            n778 = Concatenate Strings(w1611, " (1Ch)" ("string")) -> (w1610:string)
                            n779 = property class="Page"(reference=w1621, error in=w1620, "TabCaption"=w1610, "IndependentLabel"=TRUE ("Independent Label")) -> (reference out=w1609:refnum<vi>, error out=w1619:errorcluster)
                          }
                          frame 10 {
                            n780 = Equal?(x=w1626, y=0 ("x")) -> (x = y?=w1631:bool)
                            n781 = Select(t=w1630, s=w1631, f=w1629) -> (s? t:f=w1623:string)
                            n782 = Concatenate Strings(w1623, " (1Ch)" ("string")) -> (w1624:string)
                            n783 = property class="Page"(reference=w1634, error in=w1633, "TabCaption"=w1624, "IndependentLabel"=TRUE ("Independent Label")) -> (reference out=w1622:refnum<vi>, error out=w1632:errorcluster)
                          }
                          frame 12 {
                            n784 = Equal?(x=w1640, y=2 ("x")) -> (x = y?=w1643:bool)
                            n785 = Select(t=" (1Ch)" ("string"), s=w1643, f=" (2Ch)" ("string")) -> (s? t:f=w1637:string)
                            n786 = Concatenate Strings(w1636, w1637) -> (w1638:string)
                            n787 = property class="Page"(reference=w1647, error in=w1646, "TabCaption"=w1638, "IndependentLabel"=TRUE ("Independent Label")) -> (reference out=w1635:refnum<vi>, error out=w1645:errorcluster)
                          }
                          frame 13 {
                            n788 = Equal?(x=w1649, y=1 ("x")) -> (x = y?=w1657:bool)
                            n789 = Select(t=w1656, s=w1657, f=w1655) -> (s? t:f=w1651:string)
                            n790 = Concatenate Strings(w1651, " (1Ch)" ("string")) -> (w1652:string)
                            n791 = property class="Page"(reference=w1660, error in=w1659, "TabCaption"=w1652, "IndependentLabel"=TRUE ("Independent Label")) -> (reference out=w1648:refnum<vi>, error out=w1658:errorcluster)
                          }
                          frame 14 {
                            n792 = Equal?(x=w1662, y=0 ("x")) -> (x = y?=w1670:bool)
                            n793 = Select(t=w1669, s=w1670, f=w1668) -> (s? t:f=w1664:string)
                            n794 = Concatenate Strings(w1664, " (1Ch)" ("string")) -> (w1665:string)
                            n795 = property class="Page"(reference=w1673, error in=w1672, "TabCaption"=w1665, "IndependentLabel"=TRUE ("Independent Label")) -> (reference out=w1661:refnum<vi>, error out=w1671:errorcluster)
                          }
                          frame 15 {
                            n796 = Equal?(x=w1675, y=1 ("x")) -> (x = y?=w1683:bool)
                            n797 = Select(t=w1682, s=w1683, f=w1681) -> (s? t:f=w1677:string)
                            n798 = Concatenate Strings(w1677, " (1Ch)" ("string")) -> (w1678:string)
                            n799 = property class="Page"(reference=w1686, error in=w1685, "TabCaption"=w1678, "IndependentLabel"=TRUE ("Independent Label")) -> (reference out=w1674:refnum<vi>, error out=w1684:errorcluster)
                          }
                        }
                      }
                      n800 = Close Reference(reference=w1473, error in (no error)=w1475) -> (error out=w1474:errorcluster)
                    }
                    frame "CurrRanges" {
                      # "The frame ensures that this is done before updating the values of Device(s)Settings."
                      # "The current range options are variable because they depend on the number of chassis turned on in the device. Determine the correct values and populate the control option list."
                      # "1 = index of the option to pick from the range list, which will be the largest value available, determined by the number of chassis turned on."
                      # "Set range value to maximum"
                      # "Multiphase, single phase, and DC instruments have different current ranges"
                      n801 = local read "Chassis"() -> (w1696:i32)
                      n802 = local read "Mode"() -> (w1700:T8)
                      n803 = Multiply(x=w1696, y=6) -> (x*y=w1699:i32)
                      n804 = Multiply(x=30, y=w1696) -> (x*y=w1698:i32)
                      n805 = case shown="1, 2" w1700 {
                        tunnel: w1699 -> [w1721 w1725 w1739]
                        tunnel: w1698 -> [w1718 w1722 w1738]
                        tunnel: [w1715 w1729 w1735] -> w1693
                        tunnel: w1697 -> [w1714 w1728 w1741]
                        tunnel: [w1713 w1727 w1737] -> w1691
                        tunnel: [w1713 w1727 w1737] -> w1692
                        tunnel: [w1713 w1727 w1736] -> w1690
                        frame Default {
                          w1719 = "%d" ("format string")
                          n806 = Format Into String(format string=w1719, error in=w1714, w1721) -> (resulting string=w1717:string, error out=w1720:errorcluster)  [unwired: 1 in]
                          n807 = Format Into String(format string=w1719, error in=w1720, w1718) -> (resulting string=w1716:string, error out=w1715:errorcluster)  [unwired: 1 in]
                          n808 = Build Array(w1717, w1716) -> (w1713:string[])
                        }
                        frame 1, 2 {
                          w1723 = 3 ("y")
                          w1732 = "%d" ("format string")
                          n809 = Multiply(x=w1725, y=w1723) -> (x*y=w1726:i32)
                          n810 = Multiply(x=w1723, y=w1722) -> (x*y=w1724:i32)
                          n811 = Format Into String(format string=w1732, error in=w1728, w1726) -> (resulting string=w1731:string, error out=w1733:errorcluster)  [unwired: 1 in]
                          n812 = Format Into String(format string=w1732, error in=w1733, w1724) -> (resulting string=w1730:string, error out=w1729:errorcluster)  [unwired: 1 in]
                          n813 = Build Array(w1731, w1730) -> (w1727:string[])
                        }
                        frame 7, 8, 11, 12 {
                          w1740 = "%d" ("format string")
                          w1745 = 2 ("y")
                          n814 = Format Into String(format string=w1740, error in=w1741, w1739) -> (resulting string=w1743:string, error out=w1744:errorcluster)  [unwired: 1 in]
                          n815 = Format Into String(format string=w1740, error in=w1744, w1738) -> (resulting string=w1742:string, error out=w1734:errorcluster)  [unwired: 1 in]
                          n816 = Multiply(x=w1739, y=w1745) -> (x*y=w1747:i32)
                          n817 = Multiply(x=w1745, y=w1738) -> (x*y=w1746:i32)
                          n818 = Build Array(w1743, w1742) -> (w1736:string[])
                          n819 = Format Into String(format string=w1740, error in=w1734, w1747) -> (resulting string=w1749:string, error out=w1750:errorcluster)  [unwired: 1 in]
                          n820 = Format Into String(format string=w1740, error in=w1750, w1746) -> (resulting string=w1748:string, error out=w1735:errorcluster)  [unwired: 1 in]
                          n821 = Build Array(w1749, w1748) -> (w1737:string[])
                        }
                      }
                      n822 = property on="Current (A)" class="Ring (strict)"(error in=w1693, "Strings []"=w1691) -> (error out=w1694:errorcluster)  [unwired: 1 in, 1 out]
                      n823 = property on="Current (A)" class="Ring (strict)"(error in=w1694, "Strings []"=w1692) -> (error out=w1695:errorcluster)  [unwired: 1 in, 1 out]
                      n824 = property on="Current (A)" class="Ring (strict)"(error in=w1695, "Strings []"=w1690) -> (error out=w1688:errorcluster)  [unwired: 1 in, 1 out]
                      n825 = flat-sequence {
                        tunnel: u16 1 ("Ranges.Current (A)") -> [w1706]
                        tunnel: [w1705] -> w1687
                        tunnel: w1688 -> [w1705]
                        frame #0 {
                          n826 = local read "Instr1"() -> (w1711:T2)
                          n827 = Bundle By Name(cluster=w1711, "Ranges.Current (A)"=w1706) -> (w1712:T2)
                          n828 = local read "Instr2"() -> (w1710:T2)
                          n829 = Bundle By Name(cluster=w1710, "Ranges.Current (A)"=w1706) -> (w1709:T2)
                          n830 = local read "Instr3"() -> (w1707:T2)
                          n831 = Bundle By Name(cluster=w1707, "Ranges.Current (A)"=w1706) -> (w1708:T2)
                          n832 = local write "Instr1"(w1712) -> ()
                          n833 = local write "Instr2"(w1709) -> ()
                          n834 = local write "Instr3"(w1708) -> ()
                        }
                      }
                    }
                    frame "VoutCoerce" {
                      # "Instr3"
                      # "Instr2"
                      # "Instr1"
                      # "Then adjust Vout maximum value to be the same"
                      # "Extract the maximum value of the V range"
                      # "This will prevent later having to check for valid Vout entries"
                      # "1=Coerce"
                      # "Ensure that user can not set Vout more than Vrange maximum of the selected Mode"
                      n835 = property on="Voltage (V)" class="Ring (strict)"(error in=w1757) -> (error out=w1771:errorcluster, "Strings []"=w1772:string[])  [unwired: 1 in, 1 out]
                      n836 = Array Max & Min(array=w1772) -> (max value=w1770:string)  [unwired: 3 out]
                      n837 = Scan From String(format string="%d", input string=w1770, error in=w1771) -> (error out=w1767:errorcluster, output 1=w1769:i32)  [unwired: 2 in, 2 out]
                      n838 = property on="Vout (V)" class="DigNum (strict)"(error in=w1767, "Maximum"=w1769, "OutOfRngActMax"=u8 1 ("Response to Value Outside Limits:Maximum")) -> (error out=w1752:errorcluster)  [unwired: 1 in, 1 out]
                      n839 = property on="Voltage (V)" class="Ring (strict)"(error in=w1752) -> (error out=w1766:errorcluster, "Strings []"=w1764:string[])  [unwired: 1 in, 1 out]
                      n840 = Array Max & Min(array=w1764) -> (max value=w1765:string)  [unwired: 3 out]
                      n841 = Scan From String(format string="%d", input string=w1765, error in=w1766) -> (error out=w1761:errorcluster, output 1=w1762:i32)  [unwired: 2 in, 2 out]
                      n842 = property on="Vout (V)" class="DigNum (strict)"(error in=w1761, "Maximum"=w1762, "OutOfRngActMax"=u8 1 ("Response to Value Outside Limits:Maximum")) -> (error out=w1751:errorcluster)  [unwired: 1 in, 1 out]
                      n843 = property on="Voltage (V)" class="Ring (strict)"(error in=w1751) -> (error out=w1759:errorcluster, "Strings []"=w1760:string[])  [unwired: 1 in, 1 out]
                      n844 = Array Max & Min(array=w1760) -> (max value=w1758:string)  [unwired: 3 out]
                      n845 = Scan From String(format string="%d", input string=w1758, error in=w1759) -> (error out=w1754:errorcluster, output 1=w1755:i32)  [unwired: 2 in, 2 out]
                      n846 = property on="Vout (V)" class="DigNum (strict)"(error in=w1754, "Maximum"=w1755, "OutOfRngActMax"=u8 1 ("Response to Value Outside Limits:Maximum")) -> (error out=w1753:errorcluster)  [unwired: 1 in, 1 out]
                    }
                    frame "VSlewCoerce" {
                      # "Instr3"
                      # "Instr2"
                      # "Instr1"
                      # "This will prevent later having to check for valid V Slew entries"
                      # "Voltage slew limits depend on Mode"
                      n847 = local read "Mode"() -> (w1779:T8)
                      n848 = case shown="1" w1779 {
                        tunnel: w1780 -> [w1790 w1800 w1810 w1820 w1833 w1837 w1850 w1864 w1883 w1898 w1912 w1925]
                        tunnel: [w1789 w1799 w1809 w1819 w1832 w1836 w1849 w1862 w1884 w1897 w1910 w1923] -> w1778
                        frame 0, Default {
                          w1787 = 1730000.0 ("Response to Value Outside Limits:Maximum")
                          w1788 = 0.0173 ("Response to Value Outside Limits:Maximum")
                          w1783 = 866030.0 ("Response to Value Outside Limits:Maximum")
                          w1784 = u8 1 ("Response to Value Outside Limits:Maximum")
                          w1785 = u8 1 ("Response to Value Outside Limits:Maximum")
                          w1786 = u8 1 ("Response to Value Outside Limits:Maximum")
                          n849 = property on="Voltage (V/s)" class="DigNum (strict)"(error in=w1790, "Minimum"=w1788, "Maximum"=w1787, "OutOfRngActMin"=w1786, "OutOfRngActMax"=w1786, "Value"=w1783) -> (error out=w1791:errorcluster)  [unwired: 1 in, 1 out]
                          n850 = property on="Voltage (V/s)" class="DigNum (strict)"(error in=w1791, "Minimum"=w1788, "Maximum"=w1787, "OutOfRngActMin"=w1785, "OutOfRngActMax"=w1785, "Value"=w1783) -> (error out=w1792:errorcluster)  [unwired: 1 in, 1 out]
                          n851 = property on="Voltage (V/s)" class="DigNum (strict)"(error in=w1792, "Minimum"=w1788, "Maximum"=w1787, "OutOfRngActMin"=w1784, "OutOfRngActMax"=w1784, "Value"=w1783) -> (error out=w1789:errorcluster)  [unwired: 1 in, 1 out]
                        }
                        frame 1 {
                          w1798 = 1000000.0 ("Response to Value Outside Limits:Maximum")
                          w1797 = 0.01 ("Response to Value Outside Limits:Maximum")
                          w1793 = 500000.0 ("Response to Value Outside Limits:Maximum")
                          w1794 = u8 1 ("Response to Value Outside Limits:Maximum")
                          w1796 = u8 1 ("Response to Value Outside Limits:Maximum")
                          w1795 = u8 1 ("Response to Value Outside Limits:Maximum")
                          n852 = property on="Voltage (V/s)" class="DigNum (strict)"(error in=w1800, "Minimum"=w1797, "Maximum"=w1798, "OutOfRngActMin"=w1795, "OutOfRngActMax"=w1795, "Value"=w1793) -> (error out=w1801:errorcluster)  [unwired: 1 in, 1 out]
                          n853 = property on="Voltage (V/s)" class="DigNum (strict)"(error in=w1801, "Minimum"=w1797, "Maximum"=w1798, "OutOfRngActMin"=w1796, "OutOfRngActMax"=w1796, "Value"=w1793) -> (error out=w1802:errorcluster)  [unwired: 1 in, 1 out]
                          n854 = property on="Voltage (V/s)" class="DigNum (strict)"(error in=w1802, "Minimum"=w1797, "Maximum"=w1798, "OutOfRngActMin"=w1794, "OutOfRngActMax"=w1794, "Value"=w1793) -> (error out=w1799:errorcluster)  [unwired: 1 in, 1 out]
                        }
                        frame 2, 4, 12 {
                          w1803 = 20000.0 ("Response to Value Outside Limits:Maximum")
                          w1804 = 0.01 ("Response to Value Outside Limits:Maximum")
                          w1805 = 20000.0 ("Response to Value Outside Limits:Maximum")
                          w1808 = u8 1 ("Response to Value Outside Limits:Maximum")
                          w1807 = u8 1 ("Response to Value Outside Limits:Maximum")
                          w1806 = u8 1 ("Response to Value Outside Limits:Maximum")
                          n855 = property on="Voltage (V/s)" class="DigNum (strict)"(error in=w1810, "Minimum"=w1804, "Maximum"=w1803, "OutOfRngActMin"=w1806, "OutOfRngActMax"=w1806, "Value"=w1805) -> (error out=w1811:errorcluster)  [unwired: 1 in, 1 out]
                          n856 = property on="Voltage (V/s)" class="DigNum (strict)"(error in=w1811, "Minimum"=w1804, "Maximum"=w1803, "OutOfRngActMin"=w1807, "OutOfRngActMax"=w1807, "Value"=w1805) -> (error out=w1812:errorcluster)  [unwired: 1 in, 1 out]
                          n857 = property on="Voltage (V/s)" class="DigNum (strict)"(error in=w1812, "Minimum"=w1804, "Maximum"=w1803, "OutOfRngActMin"=w1808, "OutOfRngActMax"=w1808, "Value"=w1805) -> (error out=w1809:errorcluster)  [unwired: 1 in, 1 out]
                        }
                        frame 3, 7 {
                          w1813 = 1000000.0 ("Response to Value Outside Limits:Maximum")
                          w1814 = 0.01 ("Response to Value Outside Limits:Maximum")
                          w1815 = 500000.0 ("Response to Value Outside Limits:Maximum")
                          w1818 = u8 1 ("Response to Value Outside Limits:Maximum")
                          w1817 = u8 1 ("Response to Value Outside Limits:Maximum")
                          w1816 = u8 1 ("Response to Value Outside Limits:Maximum")
                          n858 = property on="Voltage (V/s)" class="DigNum (strict)"(error in=w1820, "Minimum"=w1814, "Maximum"=w1813, "OutOfRngActMin"=w1816, "OutOfRngActMax"=w1816, "Value"=w1815) -> (error out=w1822:errorcluster)  [unwired: 1 in, 1 out]
                          n859 = property on="Voltage (V/s)" class="DigNum (strict)"(error in=w1822, "Minimum"=w1814, "Maximum"=w1813, "OutOfRngActMin"=w1817, "OutOfRngActMax"=w1817, "Value"=w1815) -> (error out=w1821:errorcluster)  [unwired: 1 in, 1 out]
                          n860 = property on="Voltage (V/s)" class="DigNum (strict)"(error in=w1821, "Minimum"=w1814, "Maximum"=w1813, "OutOfRngActMin"=w1818, "OutOfRngActMax"=w1818, "Value"=w1815) -> (error out=w1819:errorcluster)  [unwired: 1 in, 1 out]
                        }
                        frame 5 {
                          w1823 = 2000000.0 ("Response to Value Outside Limits:Maximum")
                          w1824 = 0.02 ("Response to Value Outside Limits:Maximum")
                          w1827 = 1000000.0 ("Response to Value Outside Limits:Maximum")
                          w1830 = u8 1 ("Response to Value Outside Limits:Maximum")
                          w1829 = u8 1 ("Response to Value Outside Limits:Maximum")
                          w1828 = u8 1 ("Response to Value Outside Limits:Maximum")
                          n861 = property on="Voltage (V/s)" class="DigNum (strict)"(error in=w1833, "Minimum"=w1824, "Maximum"=w1823, "OutOfRngActMin"=w1828, "OutOfRngActMax"=w1828, "Value"=w1827) -> (error out=w1835:errorcluster)  [unwired: 1 in, 1 out]
                          n862 = property on="Voltage (V/s)" class="DigNum (strict)"(error in=w1835, "Minimum"=w1824, "Maximum"=w1823, "OutOfRngActMin"=w1829, "OutOfRngActMax"=w1829, "Value"=w1827) -> (error out=w1834:errorcluster)  [unwired: 1 in, 1 out]
                          n863 = property on="Voltage (V/s)" class="DigNum (strict)"(error in=w1834, "Minimum"=0.01 ("Response to Value Outside Limits:Maximum"), "Maximum"=1000000.0 ("Response to Value Outside Limits:Maximum"), "OutOfRngActMin"=w1830, "OutOfRngActMax"=w1830, "Value"=500000.0 ("Response to Value Outside Limits:Maximum")) -> (error out=w1832:errorcluster)  [unwired: 1 in, 1 out]
                        }
                        frame 6 {
                          w1838 = 2000000.0 ("Response to Value Outside Limits:Maximum")
                          w1839 = 0.02 ("Response to Value Outside Limits:Maximum")
                          w1845 = 1000000.0 ("Response to Value Outside Limits:Maximum")
                          w1842 = u8 1 ("Response to Value Outside Limits:Maximum")
                          w1843 = u8 1 ("Response to Value Outside Limits:Maximum")
                          w1844 = u8 1 ("Response to Value Outside Limits:Maximum")
                          n864 = property on="Voltage (V/s)" class="DigNum (strict)"(error in=w1837, "Minimum"=w1839, "Maximum"=w1838, "OutOfRngActMin"=w1844, "OutOfRngActMax"=w1844, "Value"=w1845) -> (error out=w1848:errorcluster)  [unwired: 1 in, 1 out]
                          n865 = property on="Voltage (V/s)" class="DigNum (strict)"(error in=w1848, "Minimum"=w1839, "Maximum"=w1838, "OutOfRngActMin"=w1843, "OutOfRngActMax"=w1843, "Value"=w1845) -> (error out=w1847:errorcluster)  [unwired: 1 in, 1 out]
                          n866 = property on="Voltage (V/s)" class="DigNum (strict)"(error in=w1847, "Minimum"=0.01 ("Response to Value Outside Limits:Maximum"), "Maximum"=20000.0 ("Response to Value Outside Limits:Maximum"), "OutOfRngActMin"=w1842, "OutOfRngActMax"=w1842, "Value"=20000.0 ("Response to Value Outside Limits:Maximum")) -> (error out=w1836:errorcluster)  [unwired: 1 in, 1 out]
                        }
                        frame 8, 9 {
                          w1851 = 1000000.0 ("Response to Value Outside Limits:Maximum")
                          w1852 = 0.01 ("Response to Value Outside Limits:Maximum")
                          w1858 = 500000.0 ("Response to Value Outside Limits:Maximum")
                          w1857 = u8 1 ("Response to Value Outside Limits:Maximum")
                          w1856 = u8 1 ("Response to Value Outside Limits:Maximum")
                          w1855 = u8 1 ("Response to Value Outside Limits:Maximum")
                          n867 = property on="Voltage (V/s)" class="DigNum (strict)"(error in=w1850, "Minimum"=w1852, "Maximum"=w1851, "OutOfRngActMin"=w1855, "OutOfRngActMax"=w1855, "Value"=w1858) -> (error out=w1861:errorcluster)  [unwired: 1 in, 1 out]
                          n868 = property on="Voltage (V/s)" class="DigNum (strict)"(error in=w1861, "Minimum"=w1852, "Maximum"=w1851, "OutOfRngActMin"=w1856, "OutOfRngActMax"=w1856, "Value"=w1858) -> (error out=w1860:errorcluster)  [unwired: 1 in, 1 out]
                          n869 = property on="Voltage (V/s)" class="DigNum (strict)"(error in=w1860, "Minimum"=0.01 ("Response to Value Outside Limits:Maximum"), "Maximum"=20000.0 ("Response to Value Outside Limits:Maximum"), "OutOfRngActMin"=w1857, "OutOfRngActMax"=w1857, "Value"=20000.0 ("Response to Value Outside Limits:Maximum")) -> (error out=w1849:errorcluster)  [unwired: 1 in, 1 out]
                        }
                        frame 10 {
                          w1867 = 20000.0 ("Response to Value Outside Limits:Maximum")
                          w1868 = 0.01 ("Response to Value Outside Limits:Maximum")
                          w1870 = 20000.0 ("Response to Value Outside Limits:Maximum")
                          w1872 = u8 1 ("Response to Value Outside Limits:Maximum")
                          w1871 = u8 1 ("Response to Value Outside Limits:Maximum")
                          w1863 = u8 1 ("Response to Value Outside Limits:Maximum")
                          n870 = property on="Voltage (V/s)" class="DigNum (strict)"(error in=w1864, "Minimum"=0.01 ("Response to Value Outside Limits:Maximum"), "Maximum"=1000000.0 ("Response to Value Outside Limits:Maximum"), "OutOfRngActMin"=w1863, "OutOfRngActMax"=w1863, "Value"=500000.0 ("Response to Value Outside Limits:Maximum")) -> (error out=w1874:errorcluster)  [unwired: 1 in, 1 out]
                          n871 = property on="Voltage (V/s)" class="DigNum (strict)"(error in=w1874, "Minimum"=w1868, "Maximum"=w1867, "OutOfRngActMin"=w1871, "OutOfRngActMax"=w1871, "Value"=w1870) -> (error out=w1873:errorcluster)  [unwired: 1 in, 1 out]
                          n872 = property on="Voltage (V/s)" class="DigNum (strict)"(error in=w1873, "Minimum"=w1868, "Maximum"=w1867, "OutOfRngActMin"=w1872, "OutOfRngActMax"=w1872, "Value"=w1870) -> (error out=w1862:errorcluster)  [unwired: 1 in, 1 out]
                        }
                        frame 11 {
                          w1875 = 20000.0 ("Response to Value Outside Limits:Maximum")
                          w1876 = 0.01 ("Response to Value Outside Limits:Maximum")
                          w1879 = 20000.0 ("Response to Value Outside Limits:Maximum")
                          w1880 = u8 1 ("Response to Value Outside Limits:Maximum")
                          w1881 = u8 1 ("Response to Value Outside Limits:Maximum")
                          w1882 = u8 1 ("Response to Value Outside Limits:Maximum")
                          n873 = property on="Voltage (V/s)" class="DigNum (strict)"(error in=w1883, "Minimum"=w1876, "Maximum"=w1875, "OutOfRngActMin"=w1882, "OutOfRngActMax"=w1882, "Value"=w1879) -> (error out=w1887:errorcluster)  [unwired: 1 in, 1 out]
                          n874 = property on="Voltage (V/s)" class="DigNum (strict)"(error in=w1887, "Minimum"=w1876, "Maximum"=w1875, "OutOfRngActMin"=w1881, "OutOfRngActMax"=w1881, "Value"=w1879) -> (error out=w1886:errorcluster)  [unwired: 1 in, 1 out]
                          n875 = property on="Voltage (V/s)" class="DigNum (strict)"(error in=w1886, "Minimum"=0.01 ("Response to Value Outside Limits:Maximum"), "Maximum"=1000000.0 ("Response to Value Outside Limits:Maximum"), "OutOfRngActMin"=w1880, "OutOfRngActMax"=w1880, "Value"=500000.0 ("Response to Value Outside Limits:Maximum")) -> (error out=w1884:errorcluster)  [unwired: 1 in, 1 out]
                        }
                        frame 13 {
                          w1889 = 1000000.0 ("Response to Value Outside Limits:Maximum")
                          w1890 = 0.01 ("Response to Value Outside Limits:Maximum")
                          w1888 = 500000.0 ("Response to Value Outside Limits:Maximum")
                          w1894 = u8 1 ("Response to Value Outside Limits:Maximum")
                          w1895 = u8 1 ("Response to Value Outside Limits:Maximum")
                          w1896 = u8 1 ("Response to Value Outside Limits:Maximum")
                          n876 = property on="Voltage (V/s)" class="DigNum (strict)"(error in=w1898, "Minimum"=w1890, "Maximum"=w1889, "OutOfRngActMin"=w1896, "OutOfRngActMax"=w1896, "Value"=w1888) -> (error out=w1900:errorcluster)  [unwired: 1 in, 1 out]
                          n877 = property on="Voltage (V/s)" class="DigNum (strict)"(error in=w1900, "Minimum"=0.01 ("Response to Value Outside Limits:Maximum"), "Maximum"=20000.0 ("Response to Value Outside Limits:Maximum"), "OutOfRngActMin"=w1895, "OutOfRngActMax"=w1895, "Value"=20000.0 ("Response to Value Outside Limits:Maximum")) -> (error out=w1899:errorcluster)  [unwired: 1 in, 1 out]
                          n878 = property on="Voltage (V/s)" class="DigNum (strict)"(error in=w1899, "Minimum"=w1890, "Maximum"=w1889, "OutOfRngActMin"=w1894, "OutOfRngActMax"=w1894, "Value"=w1888) -> (error out=w1897:errorcluster)  [unwired: 1 in, 1 out]
                        }
                        frame 14 {
                          w1903 = 1000000.0 ("Response to Value Outside Limits:Maximum")
                          w1904 = 0.01 ("Response to Value Outside Limits:Maximum")
                          w1906 = 500000.0 ("Response to Value Outside Limits:Maximum")
                          w1909 = u8 1 ("Response to Value Outside Limits:Maximum")
                          w1908 = u8 1 ("Response to Value Outside Limits:Maximum")
                          w1907 = u8 1 ("Response to Value Outside Limits:Maximum")
                          n879 = property on="Voltage (V/s)" class="DigNum (strict)"(error in=w1912, "Minimum"=0.01 ("Response to Value Outside Limits:Maximum"), "Maximum"=20000.0 ("Response to Value Outside Limits:Maximum"), "OutOfRngActMin"=w1907, "OutOfRngActMax"=w1907, "Value"=20000.0 ("Response to Value Outside Limits:Maximum")) -> (error out=w1911:errorcluster)  [unwired: 1 in, 1 out]
                          n880 = property on="Voltage (V/s)" class="DigNum (strict)"(error in=w1911, "Minimum"=w1904, "Maximum"=w1903, "OutOfRngActMin"=w1908, "OutOfRngActMax"=w1908, "Value"=w1906) -> (error out=w1913:errorcluster)  [unwired: 1 in, 1 out]
                          n881 = property on="Voltage (V/s)" class="DigNum (strict)"(error in=w1913, "Minimum"=w1904, "Maximum"=w1903, "OutOfRngActMin"=w1909, "OutOfRngActMax"=w1909, "Value"=w1906) -> (error out=w1910:errorcluster)  [unwired: 1 in, 1 out]
                        }
                        frame 15 {
                          w1916 = 20000.0 ("Response to Value Outside Limits:Maximum")
                          w1917 = 0.01 ("Response to Value Outside Limits:Maximum")
                          w1915 = 20000.0 ("Response to Value Outside Limits:Maximum")
                          w1919 = u8 1 ("Response to Value Outside Limits:Maximum")
                          w1920 = u8 1 ("Response to Value Outside Limits:Maximum")
                          w1918 = u8 1 ("Response to Value Outside Limits:Maximum")
                          n882 = property on="Voltage (V/s)" class="DigNum (strict)"(error in=w1925, "Minimum"=w1917, "Maximum"=w1916, "OutOfRngActMin"=w1918, "OutOfRngActMax"=w1918, "Value"=w1915) -> (error out=w1924:errorcluster)  [unwired: 1 in, 1 out]
                          n883 = property on="Voltage (V/s)" class="DigNum (strict)"(error in=w1924, "Minimum"=0.01 ("Response to Value Outside Limits:Maximum"), "Maximum"=1000000.0 ("Response to Value Outside Limits:Maximum"), "OutOfRngActMin"=w1920, "OutOfRngActMax"=w1920, "Value"=500000.0 ("Response to Value Outside Limits:Maximum")) -> (error out=w1926:errorcluster)  [unwired: 1 in, 1 out]
                          n884 = property on="Voltage (V/s)" class="DigNum (strict)"(error in=w1926, "Minimum"=w1917, "Maximum"=w1916, "OutOfRngActMin"=w1919, "OutOfRngActMax"=w1919, "Value"=w1915) -> (error out=w1923:errorcluster)  [unwired: 1 in, 1 out]
                        }
                      }
                    }
                    frame "CSlewCoerce" {
                      # "Instr3"
                      # "Instr2"
                      # "Instr1"
                      # "# of Chassis"
                      # "This will prevent later having to check for valid Current Slew entries"
                      # "Current slew limits depend on Mode"
                      n885 = local read "Chassis"() -> (w1928:i32)
                      n886 = local read "Mode"() -> (w1929:T8)
                      n887 = case shown="1, 2" w1929 {
                        tunnel: w1930 -> [w1939 w1951 w1960]
                        tunnel: w1928 -> [w1942 w1954 w1968]
                        tunnel: [w1938 w1950 w1959] -> w1927
                        frame 0, 3..6, 9, 10, 13..15, Default {
                          w1935 = u8 1 ("Response to Value Outside Limits:Maximum")
                          w1936 = u8 1 ("Response to Value Outside Limits:Maximum")
                          w1937 = u8 1 ("Response to Value Outside Limits:Maximum")
                          n888 = Multiply(x=0.2 ("Response to Value Outside Limits:Maximum"), y=w1942) -> (x*y=w1934:dbl)
                          n889 = Multiply(x=w1942, y=100000.0 ("Response to Value Outside Limits:Maximum")) -> (x*y=w1933:dbl)
                          n890 = property on="Current (A/s)" class="DigNum (strict)"(error in=w1939, "Minimum"=w1934, "Maximum"=w1933, "OutOfRngActMin"=w1937, "OutOfRngActMax"=w1937, "Value"=w1933) -> (error out=w1940:errorcluster)  [unwired: 1 in, 1 out]
                          n891 = property on="Current (A/s)" class="DigNum (strict)"(error in=w1940, "Minimum"=w1934, "Maximum"=w1933, "OutOfRngActMin"=w1936, "OutOfRngActMax"=w1936, "Value"=w1933) -> (error out=w1941:errorcluster)  [unwired: 1 in, 1 out]
                          n892 = property on="Current (A/s)" class="DigNum (strict)"(error in=w1941, "Minimum"=w1934, "Maximum"=w1933, "OutOfRngActMin"=w1935, "OutOfRngActMax"=w1935, "Value"=w1933) -> (error out=w1938:errorcluster)  [unwired: 1 in, 1 out]
                        }
                        frame 1, 2 {
                          w1947 = u8 1 ("Response to Value Outside Limits:Maximum")
                          w1948 = u8 1 ("Response to Value Outside Limits:Maximum")
                          w1949 = u8 1 ("Response to Value Outside Limits:Maximum")
                          n893 = Multiply(x=w1954, y=300000.0 ("Response to Value Outside Limits:Maximum")) -> (x*y=w1945:dbl)
                          n894 = Multiply(x=0.6 ("Response to Value Outside Limits:Maximum"), y=w1954) -> (x*y=w1946:dbl)
                          n895 = property on="Current (A/s)" class="DigNum (strict)"(error in=w1951, "Minimum"=w1946, "Maximum"=w1945, "OutOfRngActMin"=w1949, "OutOfRngActMax"=w1949, "Value"=w1945) -> (error out=w1952:errorcluster)  [unwired: 1 in, 1 out]
                          n896 = property on="Current (A/s)" class="DigNum (strict)"(error in=w1952, "Minimum"=w1946, "Maximum"=w1945, "OutOfRngActMin"=w1948, "OutOfRngActMax"=w1948, "Value"=w1945) -> (error out=w1953:errorcluster)  [unwired: 1 in, 1 out]
                          n897 = property on="Current (A/s)" class="DigNum (strict)"(error in=w1953, "Minimum"=w1946, "Maximum"=w1945, "OutOfRngActMin"=w1947, "OutOfRngActMax"=w1947, "Value"=w1945) -> (error out=w1950:errorcluster)  [unwired: 1 in, 1 out]
                        }
                        frame 7, 8, 11, 12 {
                          w1964 = u8 1 ("Response to Value Outside Limits:Maximum")
                          w1962 = u8 1 ("Response to Value Outside Limits:Maximum")
                          w1961 = u8 1 ("Response to Value Outside Limits:Maximum")
                          n898 = Multiply(x=w1968, y=200000.0 ("Response to Value Outside Limits:Maximum")) -> (x*y=w1957:dbl)
                          n899 = Multiply(x=0.4 ("Response to Value Outside Limits:Maximum"), y=w1968) -> (x*y=w1958:dbl)
                          n900 = property on="Current (A/s)" class="DigNum (strict)"(error in=w1960, "Minimum"=w1958, "Maximum"=w1957, "OutOfRngActMin"=w1961, "OutOfRngActMax"=w1961, "Value"=w1957) -> (error out=w1966:errorcluster)  [unwired: 1 in, 1 out]
                          n901 = property on="Current (A/s)" class="DigNum (strict)"(error in=w1966, "Minimum"=w1958, "Maximum"=w1957, "OutOfRngActMin"=w1962, "OutOfRngActMax"=w1962, "Value"=w1957) -> (error out=w1967:errorcluster)  [unwired: 1 in, 1 out]
                          n902 = Multiply(x=w1968, y=100000.0 ("Response to Value Outside Limits:Maximum")) -> (x*y=w1963:dbl)
                          n903 = Multiply(x=0.2 ("Response to Value Outside Limits:Maximum"), y=w1968) -> (x*y=w1965:dbl)
                          n904 = property on="Current (A/s)" class="DigNum (strict)"(error in=w1967, "Minimum"=w1965, "Maximum"=w1963, "OutOfRngActMin"=w1964, "OutOfRngActMax"=w1964, "Value"=w1963) -> (error out=w1959:errorcluster)  [unwired: 1 in, 1 out]
                        }
                      }
                    }
                    frame "PSlewCoerce" {
                      # "Instr3"
                      # "Instr2"
                      # "Instr1"
                      # "# of Chassis"
                      # "This will prevent later having to check for valid Power Slew entries"
                      # "Power (test) slew limits depend on Mode"
                      n905 = local read "Chassis"() -> (w1973:i32)
                      n906 = local read "Mode"() -> (w1975:T8)
                      n907 = case shown="0..2, Default" w1975 {
                        tunnel: w1976 -> [w1984 w1999 w2010]
                        tunnel: w1973 -> [w1988 w2000 w2014]
                        tunnel: [w1981 w1996 w2013] -> w1974
                        frame 0..2, Default {
                          w1985 = u8 1 ("Response to Value Outside Limits:Maximum")
                          w1986 = u8 1 ("Response to Value Outside Limits:Maximum")
                          w1987 = u8 1 ("Response to Value Outside Limits:Maximum")
                          n908 = Multiply(x=6.0 ("Response to Value Outside Limits:Maximum"), y=w1988) -> (x*y=w1980:dbl)
                          n909 = Multiply(x=w1988, y=3000000.0 ("Response to Value Outside Limits:Maximum")) -> (x*y=w1979:dbl)
                          n910 = property on="Power (W/s)" class="DigNum (strict)"(error in=w1984, "Minimum"=w1980, "Maximum"=w1979, "OutOfRngActMin"=w1987, "OutOfRngActMax"=w1987, "Value"=w1979) -> (error out=w1983:errorcluster)  [unwired: 1 in, 1 out]
                          n911 = property on="Power (W/s)" class="DigNum (strict)"(error in=w1983, "Minimum"=w1980, "Maximum"=w1979, "OutOfRngActMin"=w1986, "OutOfRngActMax"=w1986, "Value"=w1979) -> (error out=w1982:errorcluster)  [unwired: 1 in, 1 out]
                          n912 = property on="Power (W/s)" class="DigNum (strict)"(error in=w1982, "Minimum"=w1980, "Maximum"=w1979, "OutOfRngActMin"=w1985, "OutOfRngActMax"=w1985, "Value"=w1979) -> (error out=w1981:errorcluster)  [unwired: 1 in, 1 out]
                        }
                        frame 3, 4, 9, 10, 13..15 {
                          w1995 = u8 1 ("Response to Value Outside Limits:Maximum")
                          w1994 = u8 1 ("Response to Value Outside Limits:Maximum")
                          w1993 = u8 1 ("Response to Value Outside Limits:Maximum")
                          n913 = Multiply(x=w2000, y=1000000.0 ("Response to Value Outside Limits:Maximum")) -> (x*y=w1991:dbl)
                          n914 = Multiply(x=2.0 ("Response to Value Outside Limits:Maximum"), y=w2000) -> (x*y=w1992:dbl)
                          n915 = property on="Power (W/s)" class="DigNum (strict)"(error in=w1999, "Minimum"=w1992, "Maximum"=w1991, "OutOfRngActMin"=w1993, "OutOfRngActMax"=w1993, "Value"=w1991) -> (error out=w1998:errorcluster)  [unwired: 1 in, 1 out]
                          n916 = property on="Power (W/s)" class="DigNum (strict)"(error in=w1998, "Minimum"=w1992, "Maximum"=w1991, "OutOfRngActMin"=w1994, "OutOfRngActMax"=w1994, "Value"=w1991) -> (error out=w1997:errorcluster)  [unwired: 1 in, 1 out]
                          n917 = property on="Power (W/s)" class="DigNum (strict)"(error in=w1997, "Minimum"=w1992, "Maximum"=w1991, "OutOfRngActMin"=w1995, "OutOfRngActMax"=w1995, "Value"=w1991) -> (error out=w1996:errorcluster)  [unwired: 1 in, 1 out]
                        }
                        frame 5..8, 11, 12 {
                          w2007 = u8 1 ("Response to Value Outside Limits:Maximum")
                          w2005 = u8 1 ("Response to Value Outside Limits:Maximum")
                          w2003 = u8 1 ("Response to Value Outside Limits:Maximum")
                          n918 = Multiply(x=w2014, y=2000000.0 ("Response to Value Outside Limits:Maximum")) -> (x*y=w2004:dbl)
                          n919 = Multiply(x=4.0 ("Response to Value Outside Limits:Maximum"), y=w2014) -> (x*y=w2006:dbl)
                          n920 = property on="Power (W/s)" class="DigNum (strict)"(error in=w2010, "Minimum"=w2006, "Maximum"=w2004, "OutOfRngActMin"=w2003, "OutOfRngActMax"=w2003, "Value"=w2004) -> (error out=w2011:errorcluster)  [unwired: 1 in, 1 out]
                          n921 = property on="Power (W/s)" class="DigNum (strict)"(error in=w2011, "Minimum"=w2006, "Maximum"=w2004, "OutOfRngActMin"=w2005, "OutOfRngActMax"=w2005, "Value"=w2004) -> (error out=w2012:errorcluster)  [unwired: 1 in, 1 out]
                          n922 = Multiply(x=w2014, y=1000000.0 ("Response to Value Outside Limits:Maximum")) -> (x*y=w2008:dbl)
                          n923 = Multiply(x=2.0 ("Response to Value Outside Limits:Maximum"), y=w2014) -> (x*y=w2009:dbl)
                          n924 = property on="Power (W/s)" class="DigNum (strict)"(error in=w2012, "Minimum"=w2009, "Maximum"=w2008, "OutOfRngActMin"=w2007, "OutOfRngActMax"=w2007, "Value"=w2008) -> (error out=w2013:errorcluster)  [unwired: 1 in, 1 out]
                        }
                      }
                    }
                    frame "F&PhCoerce" {
                      w2019 = 50000.0 ("Response to Value Outside Limits:Maximum")
                      w2020 = 0.1 ("Response to Value Outside Limits:Maximum")
                      w2023 = u8 1 ("Response to Value Outside Limits:Maximum")
                      w2022 = u8 1 ("Response to Value Outside Limits:Maximum")
                      w2021 = u8 1 ("Response to Value Outside Limits:Maximum")
                      w2027 = 500.0 ("Response to Value Outside Limits:Maximum")
                      w2030 = 0.01 ("Response to Value Outside Limits:Maximum")
                      w2026 = u8 1 ("Response to Value Outside Limits:Maximum")
                      w2029 = u8 1 ("Response to Value Outside Limits:Maximum")
                      w2028 = u8 1 ("Response to Value Outside Limits:Maximum")
                      # "These apply for all instruments"
                      # "Frequency slew limits and Phase Angle slew limits don't depend on Mode and always have the same values."
                      n925 = property on="Frequency (Hz/s)" class="DigNum (strict)"(error in=w2031, "Minimum"=w2030, "Maximum"=w2027, "OutOfRngActMin"=w2028, "OutOfRngActMax"=w2028, "Value"=w2027) -> (error out=w2035:errorcluster)  [unwired: 1 in, 1 out]
                      n926 = property on="Phase Angle (Deg/s)" class="DigNum (strict)"(error in=w2031, "Minimum"=w2020, "Maximum"=w2019, "OutOfRngActMin"=w2021, "OutOfRngActMax"=w2021, "Value"=w2019) -> (error out=w2025:errorcluster)  [unwired: 1 in, 1 out]
                      n927 = property on="Frequency (Hz/s)" class="DigNum (strict)"(error in=w2035, "Minimum"=w2030, "Maximum"=w2027, "OutOfRngActMin"=w2029, "OutOfRngActMax"=w2029, "Value"=w2027) -> (error out=w2034:errorcluster)  [unwired: 1 in, 1 out]
                      n928 = property on="Phase Angle (Deg/s)" class="DigNum (strict)"(error in=w2025, "Minimum"=w2020, "Maximum"=w2019, "OutOfRngActMin"=w2022, "OutOfRngActMax"=w2022, "Value"=w2019) -> (error out=w2024:errorcluster)  [unwired: 1 in, 1 out]
                      n929 = property on="Frequency (Hz/s)" class="DigNum (strict)"(error in=w2034, "Minimum"=w2030, "Maximum"=w2027, "OutOfRngActMin"=w2026, "OutOfRngActMax"=w2026, "Value"=w2027) -> (error out=w2033:errorcluster)  [unwired: 1 in, 1 out]
                      n930 = property on="Phase Angle (Deg/s)" class="DigNum (strict)"(error in=w2024, "Minimum"=w2020, "Maximum"=w2019, "OutOfRngActMin"=w2023, "OutOfRngActMax"=w2023, "Value"=w2019) -> (error out=w2032:errorcluster)  [unwired: 1 in, 1 out]
                      n931 = Merge Errors(w2033, w2032) -> (w2036:errorcluster)
                    }
                    frame "SlewsCurr" {
                      # "Instr3"
                      # "Instr2"
                      # "Instr1"
                      # "Store the same status given to the Current slew controls in Device(s)Settings for later retrieval. Current slews are column index 14 in the array."
                      # "2= Disabled and Greyed"
                      # "Slew types have specific avilability depending if the instrument is AC or DC. Current slew is avilable for DC only."
                      n932 = local read "Mode"() -> (w2053:T8)
                      n933 = case shown="0, 1, 3, 5, 7, Default" w2053 {
                        tunnel: [w2056 w2058 w2060 2 ("disabled index (col)") w2066 w2070 T15."Enabled" ("Disabled") w2076] -> w2039
                        tunnel: [w2056 w2058 w2060 w2063 w2066 T15."Enabled" ("Disabled") w2072 2 ("disabled index (col)")] -> w2040
                        tunnel: [w2056 w2058 T15."Enabled" ("Disabled") w2063 2 ("disabled index (col)") w2070 w2072 w2076] -> w2041
                        tunnel: w2052 -> [w2057 w2059 w2062 w2065 w2068 w2071 w2074 w2077]
                        tunnel: [w2057 w2059 w2062 w2065 w2068 w2071 w2074 w2077] -> w2051
                        frame 0, 1, 3, 5, 7, Default {
                          w2056 = 2 ("disabled index (col)")
                          # "AC - AC - AC"
                        }
                        frame 2, 4, 12 {
                          w2058 = T15."Enabled" ("Disabled")
                          # "DC - DC - DC"
                        }
                        frame 6, 8, 9 {
                          w2060 = 2 ("disabled index (col)")
                          # "AC - AC - DC"
                        }
                        frame 10 {
                          w2063 = T15."Enabled" ("Disabled")
                          # "AC - DC - DC"
                        }
                        frame 11 {
                          w2066 = T15."Enabled" ("Disabled")
                          # "DC - DC - AC"
                        }
                        frame 13 {
                          w2070 = 2 ("disabled index (col)")
                          # "AC - DC - AC"
                        }
                        frame 14 {
                          w2072 = 2 ("disabled index (col)")
                          # "DC - AC - AC"
                        }
                        frame 15 {
                          w2076 = T15."Enabled" ("Disabled")
                          # "DC - AC - DC"
                        }
                      }
                      n934 = property on="Current (A/s)" class="DigNum (strict)"(error in=w2051, "DisabledEnum"=w2039) -> (error out=w2050:errorcluster)  [unwired: 1 in, 1 out]
                      n935 = property on="Current (A/s)" class="DigNum (strict)"(error in=w2050, "DisabledEnum"=w2040) -> (error out=w2049:errorcluster)  [unwired: 1 in, 1 out]
                      n936 = property on="Current (A/s)" class="DigNum (strict)"(error in=w2049, "DisabledEnum"=w2041) -> (error out=w2043:errorcluster)  [unwired: 1 in, 1 out]
                      n937 = property on="EnableCtrls" class="Arr (strict)"(error in=w2043) -> (error out=w2047:errorcluster, "Value"=w2046:i8[][])  [unwired: 1 in, 1 out]
                      n938 = Build Array(w2039, w2040, w2041) -> (w2048:i32[])
                      n939 = Replace Array Subset(array=w2046, new element=w2048, index (col)=14 ("disabled index (col)")) -> (w2045:i8[][])  [unwired: 1 in]
                      n940 = property on="EnableCtrls" class="Arr (strict)"(error in=w2047, "Value"=w2045) -> (error out=w2042:errorcluster)  [unwired: 1 in, 1 out]
                    }
                    frame "SlewsPow" {
                      # "Instr3"
                      # "Instr2"
                      # "Instr1"
                      # "Store the same status given to the Power slew controls in Device(s)Settings for later retrieval. Power slews are column index 15 in the array."
                      # "2= Disabled and Greyed"
                      # "Slew types have specific avilability depending if the instrument is AC or DC. Power slew is avilable for DC only."
                      n941 = local read "Mode"() -> (w2092:T8)
                      n942 = case shown="0, 1, 3, 5, 7, Default" w2092 {
                        tunnel: [w2095 w2097 w2099 2 ("disabled index (col)") w2105 w2109 T15."Enabled" ("Disabled") w2115] -> w2078
                        tunnel: [w2095 w2097 w2099 w2102 w2105 T15."Enabled" ("Disabled") w2111 2 ("disabled index (col)")] -> w2079
                        tunnel: [w2095 w2097 T15."Enabled" ("Disabled") w2102 2 ("disabled index (col)") w2109 w2111 w2115] -> w2080
                        tunnel: w2091 -> [w2096 w2098 w2101 w2104 w2107 w2110 w2113 w2116]
                        tunnel: [w2096 w2098 w2101 w2104 w2107 w2110 w2113 w2116] -> w2090
                        frame 0, 1, 3, 5, 7, Default {
                          w2095 = 2 ("disabled index (col)")
                          # "AC - AC - AC"
                        }
                        frame 2, 4, 12 {
                          w2097 = T15."Enabled" ("Disabled")
                          # "DC - DC - DC"
                        }
                        frame 6, 8, 9 {
                          w2099 = 2 ("disabled index (col)")
                          # "AC - AC - DC"
                        }
                        frame 10 {
                          w2102 = T15."Enabled" ("Disabled")
                          # "AC - DC - DC"
                        }
                        frame 11 {
                          w2105 = T15."Enabled" ("Disabled")
                          # "DC - DC - AC"
                        }
                        frame 13 {
                          w2109 = 2 ("disabled index (col)")
                          # "AC - DC - AC"
                        }
                        frame 14 {
                          w2111 = 2 ("disabled index (col)")
                          # "DC - AC - AC"
                        }
                        frame 15 {
                          w2115 = T15."Enabled" ("Disabled")
                          # "DC - AC - DC"
                        }
                      }
                      n943 = property on="Power (W/s)" class="DigNum (strict)"(error in=w2090, "DisabledEnum"=w2078) -> (error out=w2089:errorcluster)  [unwired: 1 in, 1 out]
                      n944 = property on="Power (W/s)" class="DigNum (strict)"(error in=w2089, "DisabledEnum"=w2079) -> (error out=w2088:errorcluster)  [unwired: 1 in, 1 out]
                      n945 = property on="Power (W/s)" class="DigNum (strict)"(error in=w2088, "DisabledEnum"=w2080) -> (error out=w2082:errorcluster)  [unwired: 1 in, 1 out]
                      n946 = property on="EnableCtrls" class="Arr (strict)"(error in=w2082) -> (error out=w2086:errorcluster, "Value"=w2085:i8[][])  [unwired: 1 in, 1 out]
                      n947 = Build Array(w2078, w2079, w2080) -> (w2087:i32[])
                      n948 = Replace Array Subset(array=w2085, new element=w2087, index (col)=15 ("disabled index (col)")) -> (w2084:i8[][])  [unwired: 1 in]
                      n949 = property on="EnableCtrls" class="Arr (strict)"(error in=w2086, "Value"=w2084) -> (error out=w2081:errorcluster)  [unwired: 1 in, 1 out]
                    }
                    frame "SlewsFreq" {
                      # "Instr3"
                      # "Instr2"
                      # "Instr1"
                      # "Store the same status given to the Frequency slew controls in Device(s)Settings for later retrieval. Frequency slews are column index 16 in the array."
                      # "2= Disabled and Greyed"
                      # "Slew types have specific avilability depending if the instrument is AC or DC. Frequency slew is avilable for AC only."
                      n950 = local read "Mode"() -> (w2131:T8)
                      n951 = case shown="0, 1, 3, 5, 7, Default" w2131 {
                        tunnel: [w2135 w2136 w2140 w2141 T15."Enabled" ("Disabled") w2148 w2150 2 ("disabled index (col)")] -> w2117
                        tunnel: [w2135 w2136 w2140 w2141 w2144 2 ("disabled index (col)") T15."Enabled" ("Disabled") w2154] -> w2118
                        tunnel: [w2135 w2136 2 ("disabled index (col)") T15."Enabled" ("Disabled") w2144 w2148 w2150 w2154] -> w2119
                        tunnel: w2130 -> [w2134 w2137 w2139 w2143 w2145 w2149 w2152 w2155]
                        tunnel: [w2134 w2137 w2139 w2143 w2145 w2149 w2152 w2155] -> w2129
                        frame 0, 1, 3, 5, 7, Default {
                          w2135 = T15."Enabled" ("Disabled")
                          # "AC - AC - AC"
                        }
                        frame 2, 4, 12 {
                          w2136 = 2 ("disabled index (col)")
                          # "DC - DC - DC"
                        }
                        frame 6, 8, 9 {
                          w2140 = T15."Enabled" ("Disabled")
                          # "AC - AC - DC"
                        }
                        frame 11 {
                          w2141 = 2 ("disabled index (col)")
                          # "DC - DC - AC"
                        }
                        frame 10 {
                          w2144 = 2 ("disabled index (col)")
                          # "AC - DC - DC"
                        }
                        frame 13 {
                          w2148 = T15."Enabled" ("Disabled")
                          # "AC - DC - AC"
                        }
                        frame 15 {
                          w2150 = 2 ("disabled index (col)")
                          # "DC - AC - DC"
                        }
                        frame 14 {
                          w2154 = T15."Enabled" ("Disabled")
                          # "DC - AC - AC"
                        }
                      }
                      n952 = property on="Frequency (Hz/s)" class="DigNum (strict)"(error in=w2129, "DisabledEnum"=w2117) -> (error out=w2128:errorcluster)  [unwired: 1 in, 1 out]
                      n953 = property on="Frequency (Hz/s)" class="DigNum (strict)"(error in=w2128, "DisabledEnum"=w2118) -> (error out=w2127:errorcluster)  [unwired: 1 in, 1 out]
                      n954 = property on="Frequency (Hz/s)" class="DigNum (strict)"(error in=w2127, "DisabledEnum"=w2119) -> (error out=w2121:errorcluster)  [unwired: 1 in, 1 out]
                      n955 = property on="EnableCtrls" class="Arr (strict)"(error in=w2121) -> (error out=w2125:errorcluster, "Value"=w2124:i8[][])  [unwired: 1 in, 1 out]
                      n956 = Build Array(w2117, w2118, w2119) -> (w2126:i32[])
                      n957 = Replace Array Subset(array=w2124, new element=w2126, index (col)=16 ("disabled index (col)")) -> (w2123:i8[][])  [unwired: 1 in]
                      n958 = property on="EnableCtrls" class="Arr (strict)"(error in=w2125, "Value"=w2123) -> (error out=w2120:errorcluster)  [unwired: 1 in, 1 out]
                    }
                    frame "SlewsPhase" {
                      # "Instr3"
                      # "Instr2"
                      # "Instr1"
                      # "Store the same status given to the Phase Angle slew controls in Device(s)Settings for later retrieval. Phase Angle slews are column index 17 in the array."
                      # "2= Disabled and Greyed"
                      # "Slew types have specific avilability depending if the instrument is AC or DC. Phase Angle slew is avilable for AC only."
                      n959 = local read "Mode"() -> (w2170:T8)
                      n960 = case shown="0, 1, 3, 5, 7, Default" w2170 {
                        tunnel: [w2174 w2175 w2179 w2180 T15."Enabled" ("Disabled") w2187 w2189 2 ("disabled index (col)")] -> w2156
                        tunnel: [w2174 w2175 w2179 w2180 w2183 2 ("disabled index (col)") T15."Enabled" ("Disabled") w2193] -> w2157
                        tunnel: [w2174 w2175 2 ("disabled index (col)") T15."Enabled" ("Disabled") w2183 w2187 w2189 w2193] -> w2158
                        tunnel: w2169 -> [w2173 w2176 w2178 w2182 w2184 w2188 w2191 w2194]
                        tunnel: [w2173 w2176 w2178 w2182 w2184 w2188 w2191 w2194] -> w2168
                        frame 0, 1, 3, 5, 7, Default {
                          w2174 = T15."Enabled" ("Disabled")
                          # "AC - AC - AC"
                        }
                        frame 2, 4, 12 {
                          w2175 = 2 ("disabled index (col)")
                          # "DC - DC - DC"
                        }
                        frame 6, 8, 9 {
                          w2179 = T15."Enabled" ("Disabled")
                          # "AC - AC - DC"
                        }
                        frame 11 {
                          w2180 = 2 ("disabled index (col)")
                          # "DC - DC - AC"
                        }
                        frame 10 {
                          w2183 = 2 ("disabled index (col)")
                          # "AC - DC - DC"
                        }
                        frame 13 {
                          w2187 = T15."Enabled" ("Disabled")
                          # "AC - DC - AC"
                        }
                        frame 15 {
                          w2189 = 2 ("disabled index (col)")
                          # "DC - AC - DC"
                        }
                        frame 14 {
                          w2193 = T15."Enabled" ("Disabled")
                          # "DC - AC - AC"
                        }
                      }
                      n961 = property on="Phase Angle (Deg/s)" class="DigNum (strict)"(error in=w2168, "DisabledEnum"=w2156) -> (error out=w2167:errorcluster)  [unwired: 1 in, 1 out]
                      n962 = property on="Phase Angle (Deg/s)" class="DigNum (strict)"(error in=w2167, "DisabledEnum"=w2157) -> (error out=w2166:errorcluster)  [unwired: 1 in, 1 out]
                      n963 = property on="Phase Angle (Deg/s)" class="DigNum (strict)"(error in=w2166, "DisabledEnum"=w2158) -> (error out=w2160:errorcluster)  [unwired: 1 in, 1 out]
                      n964 = Build Array(w2156, w2157, w2158) -> (w2165:i32[])
                      n965 = property on="EnableCtrls" class="Arr (strict)"(error in=w2160) -> (error out=w2164:errorcluster, "Value"=w2163:i8[][])  [unwired: 1 in, 1 out]
                      n966 = Replace Array Subset(array=w2163, new element=w2165, index (col)=17 ("disabled index (col)")) -> (w2162:i8[][])  [unwired: 1 in]
                      n967 = property on="EnableCtrls" class="Arr (strict)"(error in=w2164, "Value"=w2162) -> (error out=w2159:errorcluster)  [unwired: 1 in, 1 out]
                    }
                    frame "TripTCoerce1" {
                      w2195 = -1.0 ("Response to Value Outside Limits:Maximum")
                      w2201 = u8 1 ("Response to Value Outside Limits:Maximum")
                      w2203 = u8 1 ("Response to Value Outside Limits:Maximum")
                      w2202 = u8 1 ("Response to Value Outside Limits:Maximum")
                      w2196 = 3600.0 ("Response to Value Outside Limits:Maximum")
                      w2197 = -1.0 ("Response to Value Outside Limits:Maximum")
                      w2198 = u8 1 ("Response to Value Outside Limits:Maximum")
                      w2199 = u8 1 ("Response to Value Outside Limits:Maximum")
                      w2200 = u8 1 ("Response to Value Outside Limits:Maximum")
                      # "These are all for INSTR1 only"
                      # "Time trips for Instr1: trips are treated the same way for all modes and instruments"
                      n968 = property on="I Snk Time (s)" class="DigNum (strict)"(error in=w2208, "Value"=w2197, "Minimum"=w2197, "OutOfRngActMin"=w2200, "OutOfRngActMax"=w2200, "Maximum"=w2196) -> (error out=w2210:errorcluster)  [unwired: 1 in, 1 out]
                      n969 = property on="P Src Time (s)" class="DigNum (strict)"(error in=w2208, "Maximum"=w2196, "OutOfRngActMin"=w2202, "OutOfRngActMax"=w2202, "Value"=w2195, "Minimum"=w2195) -> (error out=w2207:errorcluster)  [unwired: 1 in, 1 out]
                      n970 = property on="I Src Time (s)" class="DigNum (strict)"(error in=w2210, "Value"=w2197, "Minimum"=w2197, "OutOfRngActMin"=w2199, "OutOfRngActMax"=w2199, "Maximum"=w2196) -> (error out=w2209:errorcluster)  [unwired: 1 in, 1 out]
                      n971 = property on="Vmax Time (s)" class="DigNum (strict)"(error in=w2207, "Maximum"=w2196, "OutOfRngActMin"=w2203, "OutOfRngActMax"=w2203, "Value"=w2195, "Minimum"=w2195) -> (error out=w2206:errorcluster)  [unwired: 1 in, 1 out]
                      n972 = property on="P Snk Time (s)" class="DigNum (strict)"(error in=w2209, "Value"=w2197, "Minimum"=w2197, "OutOfRngActMin"=w2198, "OutOfRngActMax"=w2198, "Maximum"=w2196) -> (error out=w2204:errorcluster)  [unwired: 1 in, 1 out]
                      n973 = property on="Vmin Time (s)" class="DigNum (strict)"(error in=w2206, "Maximum"=w2196, "OutOfRngActMin"=w2201, "OutOfRngActMax"=w2201, "Value"=w2195, "Minimum"=w2195) -> (error out=w2205:errorcluster)  [unwired: 1 in, 1 out]
                      n974 = Merge Errors(w2204, w2205) -> (w2211:errorcluster)
                    }
                    frame "TripTCoerce2" {
                      w2214 = -1.0 ("Response to Value Outside Limits:Maximum")
                      w2216 = 3600.0 ("Response to Value Outside Limits:Maximum")
                      w2217 = u8 1 ("Response to Value Outside Limits:Maximum")
                      w2218 = u8 1 ("Response to Value Outside Limits:Maximum")
                      w2219 = u8 1 ("Response to Value Outside Limits:Maximum")
                      w2215 = -1.0 ("Response to Value Outside Limits:Maximum")
                      w2220 = u8 1 ("Response to Value Outside Limits:Maximum")
                      w2221 = u8 1 ("Response to Value Outside Limits:Maximum")
                      w2222 = u8 1 ("Response to Value Outside Limits:Maximum")
                      # "These are all for INSTR2 only"
                      # "Time trips for Instr2: trips are treated the same way for all modes and instruments"
                      n975 = property on="I Snk Time (s)" class="DigNum (strict)"(error in=w2227, "Value"=w2215, "Minimum"=w2215, "OutOfRngActMin"=w2222, "OutOfRngActMax"=w2222, "Maximum"=w2216) -> (error out=w2229:errorcluster)  [unwired: 1 in, 1 out]
                      n976 = property on="P Src Time (s)" class="DigNum (strict)"(error in=w2227, "Maximum"=w2216, "OutOfRngActMin"=w2219, "OutOfRngActMax"=w2219, "Value"=w2214, "Minimum"=w2214) -> (error out=w2226:errorcluster)  [unwired: 1 in, 1 out]
                      n977 = property on="I Src Time (s)" class="DigNum (strict)"(error in=w2229, "Value"=w2215, "Minimum"=w2215, "OutOfRngActMin"=w2221, "OutOfRngActMax"=w2221, "Maximum"=w2216) -> (error out=w2228:errorcluster)  [unwired: 1 in, 1 out]
                      n978 = property on="Vmax Time (s)" class="DigNum (strict)"(error in=w2226, "Maximum"=w2216, "OutOfRngActMin"=w2218, "OutOfRngActMax"=w2218, "Value"=w2214, "Minimum"=w2214) -> (error out=w2225:errorcluster)  [unwired: 1 in, 1 out]
                      n979 = property on="P Snk Time (s)" class="DigNum (strict)"(error in=w2228, "Value"=w2215, "Minimum"=w2215, "OutOfRngActMin"=w2220, "OutOfRngActMax"=w2220, "Maximum"=w2216) -> (error out=w2223:errorcluster)  [unwired: 1 in, 1 out]
                      n980 = property on="Vmin Time (s)" class="DigNum (strict)"(error in=w2225, "Maximum"=w2216, "OutOfRngActMin"=w2217, "OutOfRngActMax"=w2217, "Value"=w2214, "Minimum"=w2214) -> (error out=w2224:errorcluster)  [unwired: 1 in, 1 out]
                      n981 = Merge Errors(w2223, w2224) -> (w2230:errorcluster)
                    }
                    frame "TripTCoerce3" {
                      w2233 = -1.0 ("Response to Value Outside Limits:Maximum")
                      w2235 = 3600.0 ("Response to Value Outside Limits:Maximum")
                      w2248 = u8 1 ("Response to Value Outside Limits:Maximum")
                      w2247 = u8 1 ("Response to Value Outside Limits:Maximum")
                      w2246 = u8 1 ("Response to Value Outside Limits:Maximum")
                      w2234 = -1.0 ("Response to Value Outside Limits:Maximum")
                      w2243 = u8 1 ("Response to Value Outside Limits:Maximum")
                      w2244 = u8 1 ("Response to Value Outside Limits:Maximum")
                      w2245 = u8 1 ("Response to Value Outside Limits:Maximum")
                      # "These are all for INSTR3 only"
                      # "Time trips for Instr3: trips are treated the same way for all modes and instruments"
                      n982 = property on="I Snk Time (s)" class="DigNum (strict)"(error in=w2238, "Value"=w2234, "Minimum"=w2234, "OutOfRngActMin"=w2245, "OutOfRngActMax"=w2245, "Maximum"=w2235) -> (error out=w2242:errorcluster)  [unwired: 1 in, 1 out]
                      n983 = property on="P Src Time (s)" class="DigNum (strict)"(error in=w2238, "Maximum"=w2235, "OutOfRngActMin"=w2246, "OutOfRngActMax"=w2246, "Value"=w2233, "Minimum"=w2233) -> (error out=w2237:errorcluster)  [unwired: 1 in, 1 out]
                      n984 = property on="I Src Time (s)" class="DigNum (strict)"(error in=w2242, "Value"=w2234, "Minimum"=w2234, "OutOfRngActMin"=w2244, "OutOfRngActMax"=w2244, "Maximum"=w2235) -> (error out=w2241:errorcluster)  [unwired: 1 in, 1 out]
                      n985 = property on="Vmax Time (s)" class="DigNum (strict)"(error in=w2237, "Maximum"=w2235, "OutOfRngActMin"=w2247, "OutOfRngActMax"=w2247, "Value"=w2233, "Minimum"=w2233) -> (error out=w2236:errorcluster)  [unwired: 1 in, 1 out]
                      n986 = property on="P Snk Time (s)" class="DigNum (strict)"(error in=w2241, "Value"=w2234, "Minimum"=w2234, "OutOfRngActMin"=w2243, "OutOfRngActMax"=w2243, "Maximum"=w2235) -> (error out=w2240:errorcluster)  [unwired: 1 in, 1 out]
                      n987 = property on="Vmin Time (s)" class="DigNum (strict)"(error in=w2236, "Maximum"=w2235, "OutOfRngActMin"=w2248, "OutOfRngActMax"=w2248, "Value"=w2233, "Minimum"=w2233) -> (error out=w2239:errorcluster)  [unwired: 1 in, 1 out]
                      n988 = Merge Errors(w2240, w2239) -> (w2249:errorcluster)
                    }
                    frame "VPhaseCoerce" {
                      # "INSTR1 is the only one that can have pahse voltages, and they are not allowed to be more than 350 V individually."
                      n989 = local read "Mode"() -> (w2253:T8)
                      n990 = case shown="Default" w2253 {
                        tunnel: w2255 -> [w2262 w2271 w2274]
                        tunnel: [w2259 w2269 w2274] -> w2254
                        frame 0 {
                          w2258 = u8 1 ("Response to Value Outside Limits:Maximum")
                          # "1= Coerce"
                          # "Will give 349.87 max per phase, not exactly 350. Otherwise, they would exceed the 606V maximum when combined."
                          # "For Thee-Phase the value cannot be exactly 350 or it will yield more than Vout=606 V"
                          n991 = Square Root(x=3.0) -> (sqrt(x)=w2264:dbl)
                          n992 = Divide(x=606.0 ("Response to Value Outside Limits:Maximum"), y=w2264) -> (x/y=w2257:dbl)
                          n993 = property on="A-Volts (V)" class="DigNum (strict)"(error in=w2262, "Maximum"=w2257, "OutOfRngActMax"=w2258) -> (error out=w2261:errorcluster)  [unwired: 1 in, 1 out]
                          n994 = property on="B-Volts (V)" class="DigNum (strict)"(error in=w2261, "Maximum"=w2257, "OutOfRngActMax"=w2258) -> (error out=w2260:errorcluster)  [unwired: 1 in, 1 out]
                          n995 = property on="C-Volts (V)" class="DigNum (strict)"(error in=w2260, "Maximum"=w2257, "OutOfRngActMax"=w2258) -> (error out=w2259:errorcluster)  [unwired: 1 in, 1 out]
                        }
                        frame 5, 6 {
                          w2272 = 350.0 ("Response to Value Outside Limits:Maximum")
                          w2270 = u8 1 ("Response to Value Outside Limits:Maximum")
                          # "Also, the sum of both phases for the Two-Phase mode cannot exceed the total 500 V maximum. This is managed in the other code sections dedicated to control Vout and the phase voltages."
                          # "Instr3 will be 1-Phase\\Channel. Not affected."
                          # "The Two-Phase Modes can have the exact maximum value of 350 on each phase"
                          n996 = property on="A-Volts (V)" class="DigNum (strict)"(error in=w2271, "Maximum"=w2272, "OutOfRngActMax"=w2270) -> (error out=w2273:errorcluster)  [unwired: 1 in, 1 out]
                          n997 = property on="B-Volts (V)" class="DigNum (strict)"(error in=w2273, "Maximum"=w2272, "OutOfRngActMax"=w2270) -> (error out=w2269:errorcluster)  [unwired: 1 in, 1 out]
                          n998 = local read "Instr3"() -> (w2267:T2)
                          n999 = Bundle By Name(cluster=w2267, "Vout (V)"=0.0) -> (w2268:T2)
                          n1000 = local write "Instr3"(w2268) -> ()
                        }
                        frame Default {
                          # "This does not apply for the other Modes that are not multi-phase."
                        }
                      }
                    }
                    frame "WaveLists" {
                      w2286 = 0 ("Value")
                      w2285 = 0 ("Value")
                      w2284 = 0 ("Value")
                      w2275 = string[] ["Sine", "User1", "User2", "User3"] ("Strings []")
                      # "If the user wants different waveforms than the default Sine, Triangular, etc. provided by the unit, they have to be loaded separately by following the procedure explained in the device manual, and then saved in the configuration to be recalled later."
                      # "Instr3"
                      # "Instr2"
                      # "Instr1"
                      # "0= First index = Sine"
                      # "By default the waveform shape will be set always to Sine"
                      # "Save the default AC Wave Shape control list of options for each instrument"
                      n1001 = property on="A-Wave Shape" class="Ring (strict)"(error in=w2295, "Strings []"=w2275) -> (error out=w2294:errorcluster)  [unwired: 1 in, 1 out]
                      n1002 = property on="B-Wave Shape" class="Ring (strict)"(error in=w2294, "Strings []"=w2275) -> (error out=w2283:errorcluster)  [unwired: 1 in, 1 out]
                      n1003 = property on="C-Wave Shape" class="Ring (strict)"(error in=w2283, "Strings []"=w2275) -> (error out=w2278:errorcluster)  [unwired: 1 in, 1 out]
                      n1004 = local read "Instr1"() -> (w2291:T2)
                      n1005 = Bundle By Name(cluster=w2291, "Phases.A-Wave Shape"=w2284, "Phases.B-Wave Shape"=w2284, "Phases.C-Wave Shape"=w2284) -> (w2292:T2)
                      n1006 = local write "Instr1"(w2292) -> ()
                      n1007 = property on="A-Wave Shape" class="Ring (strict)"(error in=w2278, "Strings []"=w2275) -> (error out=w2281:errorcluster)  [unwired: 1 in, 1 out]
                      n1008 = property on="B-Wave Shape" class="Ring (strict)"(error in=w2281, "Strings []"=w2275) -> (error out=w2282:errorcluster)  [unwired: 1 in, 1 out]
                      n1009 = local read "Instr2"() -> (w2290:T2)
                      n1010 = Bundle By Name(cluster=w2290, "Phases.A-Wave Shape"=w2285, "Phases.B-Wave Shape"=w2285, "Phases.C-Wave Shape"=w2285) -> (w2289:T2)
                      n1011 = property on="C-Wave Shape" class="Ring (strict)"(error in=w2282, "Strings []"=w2275) -> (error out=w2277:errorcluster)  [unwired: 1 in, 1 out]
                      n1012 = local write "Instr2"(w2289) -> ()
                      n1013 = property on="A-Wave Shape" class="Ring (strict)"(error in=w2277, "Strings []"=w2275) -> (error out=w2280:errorcluster)  [unwired: 1 in, 1 out]
                      n1014 = local read "Instr3"() -> (w2287:T2)
                      n1015 = Bundle By Name(cluster=w2287, "Phases.A-Wave Shape"=w2286, "Phases.B-Wave Shape"=w2286, "Phases.C-Wave Shape"=w2286) -> (w2288:T2)
                      n1016 = property on="B-Wave Shape" class="Ring (strict)"(error in=w2280, "Strings []"=w2275) -> (error out=w2279:errorcluster)  [unwired: 1 in, 1 out]
                      n1017 = property on="C-Wave Shape" class="Ring (strict)"(error in=w2279, "Strings []"=w2275) -> (error out=w2276:errorcluster)  [unwired: 1 in, 1 out]
                      n1018 = local write "Instr3"(w2288) -> ()
                    }
                    frame "WaveEnable" {
                      # "C"
                      # "B"
                      # "A"
                      # "Store the same status given to the Wave Shape controls in Device(s)Settings for later retrieval. Wave Shapes are column indexes 11, 12 & 13 in the array."
                      # "Instr3"
                      # "Instr2"
                      # "Instr1"
                      # "2 = Disabled and Greyed Out, it was replaced only for space convenience."
                      # "Only AC instruments should have AC waveform selection enabled."
                      n1019 = local read "Mode"() -> (w2297:T8)
                      n1020 = case shown="1, 3" w2297 {
                        selector: w2297 -> [_ _ _ w2347 w2358 _ _ _ _ _]
                        tunnel: [w2333 w2337 w2340 w2342 w2353 T15."Enabled" ("Disabled") w2363 T15."Enabled" ("Disabled") w2370 w2374] -> w2307
                        tunnel: [w2333 w2335 w2340 w2342 w2352 w2360 w2363 w2367 w2370 w2374] -> w2303
                        tunnel: [w2333 w2335 w2340 u8 2 w2352 w2360 w2363 w2367 w2370 w2374] -> w2299
                        tunnel: [w2333 w2337 w2340 w2342 w2353 w2360 w2363 w2367 T15."Enabled" ("Disabled") T15."Enabled" ("Disabled")] -> w2308
                        tunnel: [w2333 w2336 w2340 w2342 w2351 w2360 w2363 w2367 w2370 w2374] -> w2304
                        tunnel: [w2333 w2336 w2340 w2348 w2351 w2360 w2363 w2367 w2370 w2374] -> w2300
                        tunnel: [w2333 w2337 w2340 w2345 w2356 w2360 T15."Enabled" ("Disabled") T15."Enabled" ("Disabled") T15."Enabled" ("Disabled") w2374] -> w2309
                        tunnel: [w2333 w2338 w2340 w2348 w2351 w2360 w2363 w2367 w2370 w2374] -> w2305
                        tunnel: [w2333 w2338 w2340 w2348 w2351 w2360 w2363 w2367 w2370 w2374] -> w2301
                        tunnel: [w2332 w2334 w2339 w2341 w2350 w2359 w2362 w2365 w2369 w2373] -> w2310
                        tunnel: w2311 -> [w2332 w2334 w2339 w2341 w2350 w2359 w2362 w2365 w2369 w2373]
                        frame 0, Default {
                          w2333 = T15."Enabled" ("Disabled")
                          # "Three-Phase can enable all phases."
                        }
                        frame 1, 3 {
                          w2335 = u8 2
                          w2336 = u8 2
                          w2337 = T15."Enabled" ("Disabled")
                          w2338 = u8 2
                          # "All instruments are One-Phase AC"
                        }
                        frame 2, 4, 12 {
                          w2340 = u8 2
                          # "All disabled and greyed out"
                          # "All instruments are DC"
                        }
                        frame 5, 6 {
                          w2348 = u8 2
                          w2342 = T15."Enabled" ("Disabled")
                          # "5 = Instr3 is AC"
                          # "Two-Phase can enable A and B for Instr1 and Instr2. Instr3 depends on Mode."
                          n1021 = Equal?(x=w2347, y=u8 5) -> (x = y?=w2344:bool)
                          n1022 = Select(t=w2342, s=w2344, f=u8 2) -> (s? t:f=w2345:u8)
                        }
                        frame 7..9 {
                          w2351 = u8 2
                          w2352 = u8 2
                          w2353 = T15."Enabled" ("Disabled")
                          # "7 = Instr3 is AC"
                          # "Instr1 and Instr2 are One-Phase AC.\nInstr3 depends on Mode."
                          n1023 = Equal?(x=w2358, y=u8 7) -> (x = y?=w2355:bool)
                          n1024 = Select(t=w2353, s=w2355, f=u8 2) -> (s? t:f=w2356:u8)
                        }
                        frame 10 {
                          w2360 = u8 2
                          # "AC - DC - DC"
                        }
                        frame 11 {
                          w2363 = u8 2
                          # "DC - DC - AC"
                        }
                        frame 13 {
                          w2367 = u8 2
                          # "AC - DC - AC"
                        }
                        frame 14 {
                          w2370 = u8 2
                          # "DC - AC - AC"
                        }
                        frame 15 {
                          w2374 = u8 2
                          # "DC - AC - DC"
                        }
                      }
                      n1025 = local write "ModeVal"(w2297) -> ()
                      n1026 = property on="A-Wave Shape" class="Ring (strict)"(error in=w2310, "DisabledEnum"=w2307) -> (error out=w2330:errorcluster)  [unwired: 1 in, 1 out]
                      n1027 = property on="B-Wave Shape" class="Ring (strict)"(error in=w2330, "DisabledEnum"=w2303) -> (error out=w2329:errorcluster)  [unwired: 1 in, 1 out]
                      n1028 = property on="C-Wave Shape" class="Ring (strict)"(error in=w2329, "DisabledEnum"=w2299) -> (error out=w2328:errorcluster)  [unwired: 1 in, 1 out]
                      n1029 = property on="A-Wave Shape" class="Ring (strict)"(error in=w2328, "DisabledEnum"=w2308) -> (error out=w2327:errorcluster)  [unwired: 1 in, 1 out]
                      n1030 = property on="B-Wave Shape" class="Ring (strict)"(error in=w2327, "DisabledEnum"=w2304) -> (error out=w2326:errorcluster)  [unwired: 1 in, 1 out]
                      n1031 = property on="C-Wave Shape" class="Ring (strict)"(error in=w2326, "DisabledEnum"=w2300) -> (error out=w2325:errorcluster)  [unwired: 1 in, 1 out]
                      n1032 = property on="A-Wave Shape" class="Ring (strict)"(error in=w2325, "DisabledEnum"=w2309) -> (error out=w2324:errorcluster)  [unwired: 1 in, 1 out]
                      n1033 = property on="B-Wave Shape" class="Ring (strict)"(error in=w2324, "DisabledEnum"=w2305) -> (error out=w2323:errorcluster)  [unwired: 1 in, 1 out]
                      n1034 = property on="C-Wave Shape" class="Ring (strict)"(error in=w2323, "DisabledEnum"=w2301) -> (error out=w2314:errorcluster)  [unwired: 1 in, 1 out]
                      n1035 = Build Array(w2303, w2304, w2305) -> (w2302:u8[])
                      n1036 = Build Array(w2307, w2308, w2309) -> (w2306:u8[])
                      n1037 = Build Array(w2299, w2300, w2301) -> (w2298:u8[])
                      n1038 = property on="EnableCtrls" class="Arr (strict)"(error in=w2314) -> (error out=w2313:errorcluster, "Value"=w2318:i8[][])  [unwired: 1 in, 1 out]
                      n1039 = Replace Array Subset(array=w2318, new element=w2306, index (col)=11 ("disabled index (col)")) -> (w2319:i8[][])  [unwired: 1 in]
                      n1040 = Replace Array Subset(array=w2319, new element=w2302, index (col)=12 ("disabled index (col)")) -> (w2320:i8[][])  [unwired: 1 in]
                      n1041 = Replace Array Subset(array=w2320, new element=w2298, index (col)=13 ("disabled index (col)")) -> (w2321:i8[][])  [unwired: 1 in]
                      n1042 = property on="EnableCtrls" class="Arr (strict)"(error in=w2313, "Value"=w2321) -> (error out=w2312:errorcluster)  [unwired: 1 in, 1 out]
                    }
                  }
                }
                frame Error {
                  # "In case of error, this will pass over the state machine. Helpful while debugging to avoid so many cases."
                }
              }
            }
            n1043 = property on="Update" class="Bool (strict)"(error in=w818) -> (error out=w819:errorcluster, "Value"=w816:bool)  [unwired: 1 in, 1 out]
            n1044 = property on="btnSaveAs" class="Bool"(error in=w818, "DisabledEnum"=w821) -> (error out=w823:errorcluster)  [unwired: 1 in, 1 out]
            n1045 = property on="btnSave" class="Bool"(error in=w818, "DisabledEnum"=w821) -> (error out=w822:errorcluster)  [unwired: 1 in, 1 out]
            n1046 = property on="Update" class="Bool (strict)"(error in=w819, "Val(Sgnl)"=w816) -> (error out=w817:errorcluster)  [unwired: 1 in, 1 out]
            n1047 = Merge Errors(w822, w823, w817) -> (w820:errorcluster)
          }
          event "Chassis": Value Change {
            w2385 = T15."Enabled" ("Disabled")
            w2389 = FALSE ("StartMeas")
            # "Let the \"Mode Change\" event fix all the other settings, specially the Current and Power ones, to reflect the new value of Chassis."
            # "Update Device(s)Settings"
            n1048 = event-data() -> ()  [unwired: 1 in, 6 out]
            n1049 = property on="Mode" class="Ring (strict)"(error in=w2380) -> (error out=w2383:errorcluster, "Value"=w2382:T8)  [unwired: 1 in, 1 out]
            n1050 = property on="Mode" class="Ring (strict)"(error in=w2383, "Val(Sgnl)"=w2382) -> (error out=w2381:errorcluster)  [unwired: 1 in, 1 out]
            n1051 = property on="Update" class="Bool (strict)"(error in=w2381) -> (error out=w2388:errorcluster, "Value"=w2379:bool)  [unwired: 1 in, 1 out]
            n1052 = property on="Update" class="Bool (strict)"(error in=w2388, "Val(Sgnl)"=w2379) -> (error out=w2384:errorcluster)  [unwired: 1 in, 1 out]
            n1053 = property on="btnSaveAs" class="Bool"(error in=w2384, "DisabledEnum"=w2385) -> (error out=w2387:errorcluster)  [unwired: 1 in, 1 out]
            n1054 = property on="btnSave" class="Bool"(error in=w2387, "DisabledEnum"=w2385) -> (error out=w2386:errorcluster)  [unwired: 1 in, 1 out]
          }
          event Value Change {
            w2391 = T15."Enabled" ("Disabled")
            w2418 = FALSE ("StartMeas")
            # "Update Device(s)Settings"
            # "If the user changes the Synchronization setting, the AC instruments need to made available their adequate \"Change at\" angles depending on Mode."
            n1055 = event-data() -> ("NewVal"=w2407:T3)  [unwired: 1 in]
            n1056 = Equal To 0?(x=w2407) -> (x = 0?=w2409:bool)
            n1057 = case shown="True" w2409 {
              selector: w2409 -> [w2420 w2423]
              tunnel: [T15."Enabled" ("Disabled") 2] -> w2408
              tunnel: w2405 -> [w2421 w2424]
              tunnel: [w2421 w2424] -> w2404
              tunnel: [w2420 w2423] -> w2402
              tunnel: [w2420 w2423] -> w2401
              tunnel: [w2420 w2423] -> w2400
              frame False {
              }
              frame True {
                # "2 = Disbaled and Greyed Out for short"
              }
            }
            n1058 = local read "Mode"() -> (w2417:T8)
            n1059 = case shown="0, Default" w2417 {
              tunnel: [w2469 w2511 w2552 w2585 w2603 w2624 w2654 w2684] -> w2414
              tunnel: [w2469 w2512 w2552 w2586 w2603 w2624 w2655 w2684] -> w2413
              tunnel: [w2469 w2512 w2552 w2586 w2603 T15."Disabled and Grayed Out" ("Disabled") w2655 w2684] -> w2412
              tunnel: [TRUE TRUE TRUE FALSE FALSE TRUE TRUE TRUE] -> w2416
              tunnel: [TRUE TRUE TRUE FALSE FALSE FALSE FALSE FALSE] -> w2415
              tunnel: [w2460 w2496 w2544 w2580 w2598 w2618 w2646 w2676] -> w2411
              tunnel: w2404 -> [w2455 w2499 w2540 w2579 w2597 w2614 w2644 w2674]
              tunnel: w2408 -> [w2469 w2511 _ w2585 _ w2624 w2654 _]
              tunnel: w2407 -> [w2462 w2503 w2545 w2582 w2600 w2619 w2649 w2679]
              tunnel: [w2456 w2497 w2538 w2579 w2597 w2617 w2645 w2675] -> w2403
              tunnel: w2402 -> [w2461 w2502 w2541 w2581 w2599 w2616 w2647 w2678]
              tunnel: w2401 -> [w2459 w2501 w2543 _ _ w2615 w2648 w2677]
              tunnel: w2400 -> [w2458 w2500 w2542 _ _ _ _ _]
              tunnel: [w2457 w2498 w2539 w2579 w2597 w2614 w2644 w2674] -> w2399
              frame 0, Default {
                # "The three instruments have to show the same Sync setting"
                # "Instr1 works as Instr1/2/3"
                # "Three-Phase enables all angles in all instruments"
                n1060 = case shown="True" w2461 {
                  tunnel: [w2488 w2490] -> w2460
                  tunnel: w2455 -> [w2488 w2489]
                  frame False {
                  }
                  frame True {
                    n1061 = property on="A-Change at..." class="DigNum (strict)"(error in=w2489, "Value"=0) -> (error out=w2495:errorcluster)  [unwired: 1 in, 1 out]
                    n1062 = property on="B-Change at..." class="DigNum (strict)"(error in=w2495, "Value"=0) -> (error out=w2494:errorcluster)  [unwired: 1 in, 1 out]
                    n1063 = property on="C-Change at..." class="DigNum (strict)"(error in=w2494, "Value"=0) -> (error out=w2490:errorcluster)  [unwired: 1 in, 1 out]
                  }
                }
                n1064 = case shown="True" w2459 {
                  tunnel: w2455 -> [w2480 w2482]
                  tunnel: [w2480 w2481] -> w2456
                  frame False {
                  }
                  frame True {
                    n1065 = property on="A-Change at..." class="DigNum (strict)"(error in=w2482, "Value"=0) -> (error out=w2487:errorcluster)  [unwired: 1 in, 1 out]
                    n1066 = property on="B-Change at..." class="DigNum (strict)"(error in=w2487, "Value"=0) -> (error out=w2486:errorcluster)  [unwired: 1 in, 1 out]
                    n1067 = property on="C-Change at..." class="DigNum (strict)"(error in=w2486, "Value"=0) -> (error out=w2481:errorcluster)  [unwired: 1 in, 1 out]
                  }
                }
                n1068 = case shown="True" w2458 {
                  tunnel: w2455 -> [w2472 w2474]
                  tunnel: [w2472 w2473] -> w2457
                  frame False {
                  }
                  frame True {
                    n1069 = property on="A-Change at..." class="DigNum (strict)"(error in=w2474, "Value"=0) -> (error out=w2479:errorcluster)  [unwired: 1 in, 1 out]
                    n1070 = property on="B-Change at..." class="DigNum (strict)"(error in=w2479, "Value"=0) -> (error out=w2478:errorcluster)  [unwired: 1 in, 1 out]
                    n1071 = property on="C-Change at..." class="DigNum (strict)"(error in=w2478, "Value"=0) -> (error out=w2473:errorcluster)  [unwired: 1 in, 1 out]
                  }
                }
                n1072 = local read "Device(s)Settings"() -> (w2467:T1)
                n1073 = Bundle By Name(cluster=w2467, "Instr1.Synchronization"=w2462, "Instr2.Synchronization"=w2462, "Instr3.Synchronization"=w2462) -> (w2468:T1)
                n1074 = local read "Instr2"() -> (w2466:T2)
                n1075 = Bundle By Name(cluster=w2466, "Synchronization"=w2462) -> (w2465:T2)
                n1076 = local read "Instr3"() -> (w2463:T2)
                n1077 = Bundle By Name(cluster=w2463, "Synchronization"=w2462) -> (w2464:T2)
                n1078 = local write "Instr2"(w2465) -> ()
                n1079 = local write "Instr3"(w2464) -> ()
                n1080 = local write "Device(s)Settings"(w2468) -> ()
              }
              frame 1 {
                w2512 = T15."Disabled and Grayed Out" ("Disabled")
                # "The three instruments have to show the same Sync setting"
                # "Instr1 works as Instr1/2/3"
                # "Instr1 as one AC single-phase instrument"
                n1081 = case shown="False" w2502 {
                  tunnel: [w2530 w2532] -> w2496
                  tunnel: w2499 -> [w2530 w2531]
                  frame False {
                  }
                  frame True {
                    n1082 = property on="A-Change at..." class="DigNum (strict)"(error in=w2531, "Value"=0) -> (error out=w2537:errorcluster)  [unwired: 1 in, 1 out]
                    n1083 = property on="B-Change at..." class="DigNum (strict)"(error in=w2537, "Value"=0) -> (error out=w2536:errorcluster)  [unwired: 1 in, 1 out]
                    n1084 = property on="C-Change at..." class="DigNum (strict)"(error in=w2536, "Value"=0) -> (error out=w2532:errorcluster)  [unwired: 1 in, 1 out]
                  }
                }
                n1085 = case shown="False" w2501 {
                  tunnel: w2499 -> [w2522 w2524]
                  tunnel: [w2522 w2523] -> w2497
                  frame False {
                  }
                  frame True {
                    n1086 = property on="A-Change at..." class="DigNum (strict)"(error in=w2524, "Value"=0) -> (error out=w2529:errorcluster)  [unwired: 1 in, 1 out]
                    n1087 = property on="B-Change at..." class="DigNum (strict)"(error in=w2529, "Value"=0) -> (error out=w2528:errorcluster)  [unwired: 1 in, 1 out]
                    n1088 = property on="C-Change at..." class="DigNum (strict)"(error in=w2528, "Value"=0) -> (error out=w2523:errorcluster)  [unwired: 1 in, 1 out]
                  }
                }
                n1089 = case shown="False" w2500 {
                  tunnel: w2499 -> [w2514 w2516]
                  tunnel: [w2514 w2515] -> w2498
                  frame False {
                  }
                  frame True {
                    n1090 = property on="A-Change at..." class="DigNum (strict)"(error in=w2516, "Value"=0) -> (error out=w2521:errorcluster)  [unwired: 1 in, 1 out]
                    n1091 = property on="B-Change at..." class="DigNum (strict)"(error in=w2521, "Value"=0) -> (error out=w2520:errorcluster)  [unwired: 1 in, 1 out]
                    n1092 = property on="C-Change at..." class="DigNum (strict)"(error in=w2520, "Value"=0) -> (error out=w2515:errorcluster)  [unwired: 1 in, 1 out]
                  }
                }
                n1093 = local read "Device(s)Settings"() -> (w2508:T1)
                n1094 = Bundle By Name(cluster=w2508, "Instr1.Synchronization"=w2503, "Instr2.Synchronization"=w2503, "Instr3.Synchronization"=w2503) -> (w2509:T1)
                n1095 = local read "Instr3"() -> (w2504:T2)
                n1096 = Bundle By Name(cluster=w2504, "Synchronization"=w2503) -> (w2505:T2)
                n1097 = local read "Instr2"() -> (w2507:T2)
                n1098 = Bundle By Name(cluster=w2507, "Synchronization"=w2503) -> (w2506:T2)
                n1099 = local write "Instr3"(w2505) -> ()
                n1100 = local write "Instr2"(w2506) -> ()
                n1101 = local write "Device(s)Settings"(w2509) -> ()
              }
              frame 2 {
                w2552 = T15."Disabled and Grayed Out" ("Disabled")
                # "The three instruments have to show the same Sync setting"
                # "Instr1 works as Instr1/2/3"
                # "Instr1 as one DC single-channel instrument"
                n1102 = case shown="False" w2541 {
                  tunnel: [w2571 w2573] -> w2544
                  tunnel: w2540 -> [w2571 w2572]
                  frame False {
                  }
                  frame True {
                    n1103 = property on="A-Change at..." class="DigNum (strict)"(error in=w2572, "Value"=0) -> (error out=w2578:errorcluster)  [unwired: 1 in, 1 out]
                    n1104 = property on="B-Change at..." class="DigNum (strict)"(error in=w2578, "Value"=0) -> (error out=w2577:errorcluster)  [unwired: 1 in, 1 out]
                    n1105 = property on="C-Change at..." class="DigNum (strict)"(error in=w2577, "Value"=0) -> (error out=w2573:errorcluster)  [unwired: 1 in, 1 out]
                  }
                }
                n1106 = case shown="False" w2543 {
                  tunnel: w2540 -> [w2563 w2565]
                  tunnel: [w2563 w2564] -> w2538
                  frame False {
                  }
                  frame True {
                    n1107 = property on="A-Change at..." class="DigNum (strict)"(error in=w2565, "Value"=0) -> (error out=w2570:errorcluster)  [unwired: 1 in, 1 out]
                    n1108 = property on="B-Change at..." class="DigNum (strict)"(error in=w2570, "Value"=0) -> (error out=w2569:errorcluster)  [unwired: 1 in, 1 out]
                    n1109 = property on="C-Change at..." class="DigNum (strict)"(error in=w2569, "Value"=0) -> (error out=w2564:errorcluster)  [unwired: 1 in, 1 out]
                  }
                }
                n1110 = case shown="False" w2542 {
                  tunnel: w2540 -> [w2555 w2557]
                  tunnel: [w2555 w2556] -> w2539
                  frame False {
                  }
                  frame True {
                    n1111 = property on="A-Change at..." class="DigNum (strict)"(error in=w2557, "Value"=0) -> (error out=w2562:errorcluster)  [unwired: 1 in, 1 out]
                    n1112 = property on="B-Change at..." class="DigNum (strict)"(error in=w2562, "Value"=0) -> (error out=w2561:errorcluster)  [unwired: 1 in, 1 out]
                    n1113 = property on="C-Change at..." class="DigNum (strict)"(error in=w2561, "Value"=0) -> (error out=w2556:errorcluster)  [unwired: 1 in, 1 out]
                  }
                }
                n1114 = local read "Device(s)Settings"() -> (w2550:T1)
                n1115 = Bundle By Name(cluster=w2550, "Instr1.Synchronization"=w2545, "Instr2.Synchronization"=w2545, "Instr3.Synchronization"=w2545) -> (w2551:T1)
                n1116 = local read "Instr2"() -> (w2549:T2)
                n1117 = Bundle By Name(cluster=w2549, "Synchronization"=w2545) -> (w2548:T2)
                n1118 = local read "Instr3"() -> (w2546:T2)
                n1119 = Bundle By Name(cluster=w2546, "Synchronization"=w2545) -> (w2547:T2)
                n1120 = local write "Instr2"(w2548) -> ()
                n1121 = local write "Instr3"(w2547) -> ()
                n1122 = local write "Device(s)Settings"(w2551) -> ()
              }
              frame 3, 9, 10, 13 {
                w2586 = T15."Disabled and Grayed Out" ("Disabled")
                # "Pass the setting only to Instr1 in Device(s)Settings."
                # "Instr1 works independently"
                # "Instr1 alone as one AC single-phase instrument"
                n1123 = case shown="True" w2581 {
                  tunnel: [w2589 w2591] -> w2580
                  tunnel: w2579 -> [w2589 w2590]
                  frame False {
                  }
                  frame True {
                    n1124 = property on="A-Change at..." class="DigNum (strict)"(error in=w2590, "Value"=0) -> (error out=w2596:errorcluster)  [unwired: 1 in, 1 out]
                    n1125 = property on="B-Change at..." class="DigNum (strict)"(error in=w2596, "Value"=0) -> (error out=w2595:errorcluster)  [unwired: 1 in, 1 out]
                    n1126 = property on="C-Change at..." class="DigNum (strict)"(error in=w2595, "Value"=0) -> (error out=w2591:errorcluster)  [unwired: 1 in, 1 out]
                  }
                }
                n1127 = local read "Device(s)Settings"() -> (w2583:T1)
                n1128 = Bundle By Name(cluster=w2583, "Instr1.Synchronization"=w2582) -> (w2584:T1)
                n1129 = local write "Device(s)Settings"(w2584) -> ()
              }
              frame 4, 14, 15 {
                w2603 = T15."Disabled and Grayed Out" ("Disabled")
                # "Pass the setting only to Instr1 in Device(s)Settings."
                # "Instr1 works independently"
                # "Instr1 alone as one DC single-channel instrument"
                n1130 = case shown="False" w2599 {
                  tunnel: [w2606 w2608] -> w2598
                  tunnel: w2597 -> [w2606 w2607]
                  frame False {
                  }
                  frame True {
                    n1131 = property on="A-Change at..." class="DigNum (strict)"(error in=w2607, "Value"=0) -> (error out=w2613:errorcluster)  [unwired: 1 in, 1 out]
                    n1132 = property on="B-Change at..." class="DigNum (strict)"(error in=w2613, "Value"=0) -> (error out=w2612:errorcluster)  [unwired: 1 in, 1 out]
                    n1133 = property on="C-Change at..." class="DigNum (strict)"(error in=w2612, "Value"=0) -> (error out=w2608:errorcluster)  [unwired: 1 in, 1 out]
                  }
                }
                n1134 = local read "Device(s)Settings"() -> (w2601:T1)
                n1135 = Bundle By Name(cluster=w2601, "Instr1.Synchronization"=w2600) -> (w2602:T1)
                n1136 = local write "Device(s)Settings"(w2602) -> ()
              }
              frame 5, 6 {
                # "Pass only Instr1 and Instr2 settings to Device(s)Settings."
                # "Instr1 works as Instr1/2 only"
                # "Instr1/Instr2 as one AC Two-Phase instrument"
                n1137 = case shown="False" w2616 {
                  tunnel: [w2636 w2638] -> w2618
                  tunnel: w2614 -> [w2636 w2637]
                  frame False {
                  }
                  frame True {
                    n1138 = property on="A-Change at..." class="DigNum (strict)"(error in=w2637, "Value"=0) -> (error out=w2643:errorcluster)  [unwired: 1 in, 1 out]
                    n1139 = property on="B-Change at..." class="DigNum (strict)"(error in=w2643, "Value"=0) -> (error out=w2642:errorcluster)  [unwired: 1 in, 1 out]
                    n1140 = property on="C-Change at..." class="DigNum (strict)"(error in=w2642, "Value"=0) -> (error out=w2638:errorcluster)  [unwired: 1 in, 1 out]
                  }
                }
                n1141 = local read "Device(s)Settings"() -> (w2622:T1)
                n1142 = Bundle By Name(cluster=w2622, "Instr1.Synchronization"=w2619, "Instr2.Synchronization"=w2619) -> (w2623:T1)
                n1143 = case shown="False" w2615 {
                  tunnel: w2614 -> [w2628 w2630]
                  tunnel: [w2628 w2629] -> w2617
                  frame False {
                  }
                  frame True {
                    n1144 = property on="A-Change at..." class="DigNum (strict)"(error in=w2630, "Value"=0) -> (error out=w2635:errorcluster)  [unwired: 1 in, 1 out]
                    n1145 = property on="B-Change at..." class="DigNum (strict)"(error in=w2635, "Value"=0) -> (error out=w2634:errorcluster)  [unwired: 1 in, 1 out]
                    n1146 = property on="C-Change at..." class="DigNum (strict)"(error in=w2634, "Value"=0) -> (error out=w2629:errorcluster)  [unwired: 1 in, 1 out]
                  }
                }
                n1147 = local read "Instr2"() -> (w2621:T2)
                n1148 = Bundle By Name(cluster=w2621, "Synchronization"=w2619) -> (w2620:T2)
                n1149 = local write "Instr2"(w2620) -> ()
                n1150 = local write "Device(s)Settings"(w2623) -> ()
              }
              frame 7, 8 {
                w2655 = T15."Disabled and Grayed Out" ("Disabled")
                # "Pass only Instr1 and Instr2 settings to Device(s)Settings."
                # "Instr1 works as Instr1/2 only"
                # "Instr1/Instr2 as one AC single-phase instrument"
                n1151 = case shown="False" w2647 {
                  tunnel: [w2666 w2668] -> w2646
                  tunnel: w2644 -> [w2666 w2667]
                  frame False {
                  }
                  frame True {
                    n1152 = property on="A-Change at..." class="DigNum (strict)"(error in=w2667, "Value"=0) -> (error out=w2673:errorcluster)  [unwired: 1 in, 1 out]
                    n1153 = property on="B-Change at..." class="DigNum (strict)"(error in=w2673, "Value"=0) -> (error out=w2672:errorcluster)  [unwired: 1 in, 1 out]
                    n1154 = property on="C-Change at..." class="DigNum (strict)"(error in=w2672, "Value"=0) -> (error out=w2668:errorcluster)  [unwired: 1 in, 1 out]
                  }
                }
                n1155 = case shown="False" w2648 {
                  tunnel: w2644 -> [w2658 w2660]
                  tunnel: [w2658 w2659] -> w2645
                  frame False {
                  }
                  frame True {
                    n1156 = property on="A-Change at..." class="DigNum (strict)"(error in=w2660, "Value"=0) -> (error out=w2665:errorcluster)  [unwired: 1 in, 1 out]
                    n1157 = property on="B-Change at..." class="DigNum (strict)"(error in=w2665, "Value"=0) -> (error out=w2664:errorcluster)  [unwired: 1 in, 1 out]
                    n1158 = property on="C-Change at..." class="DigNum (strict)"(error in=w2664, "Value"=0) -> (error out=w2659:errorcluster)  [unwired: 1 in, 1 out]
                  }
                }
                n1159 = local read "Device(s)Settings"() -> (w2652:T1)
                n1160 = Bundle By Name(cluster=w2652, "Instr1.Synchronization"=w2649, "Instr2.Synchronization"=w2649) -> (w2653:T1)
                n1161 = local read "Instr2"() -> (w2651:T2)
                n1162 = Bundle By Name(cluster=w2651, "Synchronization"=w2649) -> (w2650:T2)
                n1163 = local write "Instr2"(w2650) -> ()
                n1164 = local write "Device(s)Settings"(w2653) -> ()
              }
              frame 11, 12 {
                w2684 = T15."Disabled and Grayed Out" ("Disabled")
                # "Pass only Instr1 and Instr2 settings to Device(s)Settings."
                # "Instr1 works as Instr1/2 only"
                # "Instr1/Instr2 as one DC single-channel instrument"
                n1165 = case shown="False" w2678 {
                  tunnel: [w2695 w2697] -> w2676
                  tunnel: w2674 -> [w2695 w2696]
                  frame False {
                  }
                  frame True {
                    n1166 = property on="A-Change at..." class="DigNum (strict)"(error in=w2696, "Value"=0) -> (error out=w2702:errorcluster)  [unwired: 1 in, 1 out]
                    n1167 = property on="B-Change at..." class="DigNum (strict)"(error in=w2702, "Value"=0) -> (error out=w2701:errorcluster)  [unwired: 1 in, 1 out]
                    n1168 = property on="C-Change at..." class="DigNum (strict)"(error in=w2701, "Value"=0) -> (error out=w2697:errorcluster)  [unwired: 1 in, 1 out]
                  }
                }
                n1169 = case shown="False" w2677 {
                  tunnel: w2674 -> [w2687 w2689]
                  tunnel: [w2687 w2688] -> w2675
                  frame False {
                  }
                  frame True {
                    n1170 = property on="A-Change at..." class="DigNum (strict)"(error in=w2689, "Value"=0) -> (error out=w2694:errorcluster)  [unwired: 1 in, 1 out]
                    n1171 = property on="B-Change at..." class="DigNum (strict)"(error in=w2694, "Value"=0) -> (error out=w2693:errorcluster)  [unwired: 1 in, 1 out]
                    n1172 = property on="C-Change at..." class="DigNum (strict)"(error in=w2693, "Value"=0) -> (error out=w2688:errorcluster)  [unwired: 1 in, 1 out]
                  }
                }
                n1173 = local read "Device(s)Settings"() -> (w2682:T1)
                n1174 = Bundle By Name(cluster=w2682, "Instr1.Synchronization"=w2679, "Instr2.Synchronization"=w2679) -> (w2683:T1)
                n1175 = local read "Instr2"() -> (w2681:T2)
                n1176 = Bundle By Name(cluster=w2681, "Synchronization"=w2679) -> (w2680:T2)
                n1177 = local write "Instr2"(w2680) -> ()
                n1178 = local write "Device(s)Settings"(w2683) -> ()
              }
            }
            n1179 = flat-sequence {
              tunnel: w2416 -> [w2436]
              tunnel: w2415 -> [w2435]
              tunnel: w2414 -> [w2434]
              tunnel: w2413 -> [w2433]
              tunnel: w2412 -> [w2432]
              tunnel: w2411 -> [w2431]
              tunnel: w2403 -> [w2429]
              tunnel: w2399 -> [w2430]
              tunnel: [w2428] -> w2398
              tunnel: [w2427] -> w2397
              tunnel: [w2426] -> w2396
              frame #0 {
                # "Enable/Disable the \"Change at\" controls as required."
                # "Instr1"
                n1180 = case shown="False" w2436 {
                  tunnel: w2434 -> [_ w2452]
                  tunnel: w2433 -> [_ w2451]
                  tunnel: w2432 -> [_ w2450]
                  tunnel: w2429 -> [w2447 w2449]
                  tunnel: [w2447 w2448] -> w2427
                  frame False {
                    # "Don't make any changes to Instr2"
                  }
                  frame True {
                    # "Instr2"
                    n1181 = property on="A-Change at..." class="DigNum (strict)"(error in=w2449, "DisabledEnum"=w2452) -> (error out=w2453:errorcluster)  [unwired: 1 in, 1 out]
                    n1182 = property on="B-Change at..." class="DigNum (strict)"(error in=w2453, "DisabledEnum"=w2451) -> (error out=w2454:errorcluster)  [unwired: 1 in, 1 out]
                    n1183 = property on="C-Change at..." class="DigNum (strict)"(error in=w2454, "DisabledEnum"=w2450) -> (error out=w2448:errorcluster)  [unwired: 1 in, 1 out]
                  }
                }
                n1184 = case shown="False" w2435 {
                  tunnel: w2434 -> [_ w2444]
                  tunnel: w2433 -> [_ w2443]
                  tunnel: w2432 -> [_ w2442]
                  tunnel: w2430 -> [w2439 w2441]
                  tunnel: [w2439 w2440] -> w2428
                  frame False {
                    # "Don't make any changes to Instr3"
                  }
                  frame True {
                    # "Instr3"
                    n1185 = property on="A-Change at..." class="DigNum (strict)"(error in=w2441, "DisabledEnum"=w2444) -> (error out=w2445:errorcluster)  [unwired: 1 in, 1 out]
                    n1186 = property on="B-Change at..." class="DigNum (strict)"(error in=w2445, "DisabledEnum"=w2443) -> (error out=w2446:errorcluster)  [unwired: 1 in, 1 out]
                    n1187 = property on="C-Change at..." class="DigNum (strict)"(error in=w2446, "DisabledEnum"=w2442) -> (error out=w2440:errorcluster)  [unwired: 1 in, 1 out]
                  }
                }
                n1188 = property on="A-Change at..." class="DigNum (strict)"(error in=w2431, "DisabledEnum"=w2434) -> (error out=w2437:errorcluster)  [unwired: 1 in, 1 out]
                n1189 = property on="B-Change at..." class="DigNum (strict)"(error in=w2437, "DisabledEnum"=w2433) -> (error out=w2438:errorcluster)  [unwired: 1 in, 1 out]
                n1190 = property on="C-Change at..." class="DigNum (strict)"(error in=w2438, "DisabledEnum"=w2432) -> (error out=w2426:errorcluster)  [unwired: 1 in, 1 out]
              }
            }
            n1191 = property on="Update" class="Bool (strict)"(error in=w2396) -> (error out=w2410:errorcluster, "Value"=w2406:bool)  [unwired: 1 in, 1 out]
            n1192 = property on="Update" class="Bool (strict)"(error in=w2410, "Val(Sgnl)"=w2406) -> (error out=w2394:errorcluster)  [unwired: 1 in, 1 out]
            n1193 = property on="btnSaveAs" class="Bool"(error in=w2397, "DisabledEnum"=w2391) -> (error out=w2393:errorcluster)  [unwired: 1 in, 1 out]
            n1194 = property on="btnSave" class="Bool"(error in=w2398, "DisabledEnum"=w2391) -> (error out=w2392:errorcluster)  [unwired: 1 in, 1 out]
            n1195 = Merge Errors(w2394, w2393, w2392) -> (w2395:errorcluster)
          }
          event Value Change {
            w2718 = T15."Enabled" ("Disabled")
            w2721 = FALSE ("StartMeas")
            # "If the index selection for the control is not equal to zero, it means that the option is not \"Immediate\" and then the adequate \"Change at\" controls need to be made available."
            # "Since these are properties of the \"Change at\" controls, and not their values, they'll be registered using the \"Update Device(s)Settings\" procedure so that this case doesn't get too complicated in structure."
            # "Update Device(s)Settings"
            # "The user can only access the Synchronization control in Instr2 when it is working as a separate instrument in its own panel. Otherwise, Instr1 is overriding it and already took care of Instr2 settings."
            n1196 = event-data() -> ("NewVal"=w2706:T3)  [unwired: 1 in]
            n1197 = Not Equal To 0?(x=w2706) -> (x != 0?=w2708:bool)
            n1198 = case shown="False" w2708 {
              tunnel: [T15."Disabled and Grayed Out" ("Disabled") T15."Enabled" ("Disabled")] -> w2707
              tunnel: [w2732 w2739] -> w2704
              tunnel: w2703 -> [w2731 w2739]
              frame False {
                # "Reset all to 0 if it becomes \"Immediate\""
                n1199 = property on="A-Change at..." class="DigNum (strict)"(error in=w2731, "Value"=0) -> (error out=w2737:errorcluster)  [unwired: 1 in, 1 out]
                n1200 = property on="B-Change at..." class="DigNum (strict)"(error in=w2737, "Value"=0) -> (error out=w2736:errorcluster)  [unwired: 1 in, 1 out]
                n1201 = property on="C-Change at..." class="DigNum (strict)"(error in=w2736, "Value"=0) -> (error out=w2732:errorcluster)  [unwired: 1 in, 1 out]
              }
              frame True {
              }
            }
            n1202 = local read "Mode"() -> (w2717:T8)
            n1203 = case shown="4, 10, 13" w2717 {
              tunnel: [w2742 w2745 w2748] -> w2715
              tunnel: [w2742 w2744 w2748] -> w2714
              tunnel: [w2742 w2744 w2748] -> w2713
              tunnel: [FALSE TRUE TRUE] -> w2716
              tunnel: [w2741 w2746 w2749] -> w2712
              tunnel: w2704 -> [w2741 w2746 w2749]
              tunnel: w2707 -> [_ w2745 _]
              frame Default {
                w2742 = T15."Enabled" ("Disabled")
                # "Instr2 is overriden by Instr1. No changes will be done to Instr2."
                # "Modes where Instr2 is not working by itself"
              }
              frame 3, 9, 14, 15 {
                w2744 = T15."Disabled and Grayed Out" ("Disabled")
                # "Modes where Instr2 is AC and available"
              }
              frame 4, 10, 13 {
                w2748 = T15."Disabled and Grayed Out" ("Disabled")
                # "Modes where Instr2 is DC and available"
              }
            }
            n1204 = case shown="True" w2716 {
              tunnel: w2715 -> [_ w2728]
              tunnel: w2714 -> [_ w2727]
              tunnel: w2713 -> [_ w2726]
              tunnel: w2712 -> [w2723 w2725]
              tunnel: [w2723 w2724] -> w2709
              frame False {
                # "Don't make any changes to Instr2"
              }
              frame True {
                # "Instr2"
                n1205 = property on="A-Change at..." class="DigNum (strict)"(error in=w2725, "DisabledEnum"=w2728) -> (error out=w2729:errorcluster)  [unwired: 1 in, 1 out]
                n1206 = property on="B-Change at..." class="DigNum (strict)"(error in=w2729, "DisabledEnum"=w2727) -> (error out=w2730:errorcluster)  [unwired: 1 in, 1 out]
                n1207 = property on="C-Change at..." class="DigNum (strict)"(error in=w2730, "DisabledEnum"=w2726) -> (error out=w2724:errorcluster)  [unwired: 1 in, 1 out]
              }
            }
            n1208 = property on="Update" class="Bool (strict)"(error in=w2709) -> (error out=w2711:errorcluster, "Value"=w2705:bool)  [unwired: 1 in, 1 out]
            n1209 = property on="Update" class="Bool (strict)"(error in=w2711, "Val(Sgnl)"=w2705) -> (error out=w2710:errorcluster)  [unwired: 1 in, 1 out]
            n1210 = property on="btnSaveAs" class="Bool"(error in=w2710, "DisabledEnum"=w2718) -> (error out=w2720:errorcluster)  [unwired: 1 in, 1 out]
            n1211 = property on="btnSave" class="Bool"(error in=w2720, "DisabledEnum"=w2718) -> (error out=w2719:errorcluster)  [unwired: 1 in, 1 out]
          }
          event Value Change {
            w2766 = T15."Enabled" ("Disabled")
            w2769 = FALSE ("StartMeas")
            # "If the index selection for the control is not equal to zero, it means that the option is not \"Immediate\" and then the adequate \"Change at\" controls need to be made available."
            # "Since these are properties of the \"Change at\" controls, and not their values, they'll be registered using the \"Update Device(s)Settings\" procedure so that this case doesn't get too complicated in structure."
            # "Update Device(s)Settings"
            # "Instr3 is available to the user most of the time to be able to change the Synchronization setting, except when Instr3 is overriden by Instr1."
            n1212 = event-data() -> ("NewVal"=w2754:T3)  [unwired: 1 in]
            n1213 = Not Equal To 0?(x=w2754) -> (x != 0?=w2756:bool)
            n1214 = case shown="False" w2756 {
              tunnel: [T15."Disabled and Grayed Out" ("Disabled") T15."Enabled" ("Disabled")] -> w2755
              tunnel: [w2779 w2787] -> w2752
              tunnel: w2751 -> [w2780 w2787]
              frame False {
                # "Reset all to 0 if it becomes \"Immediate\""
                n1215 = property on="A-Change at..." class="DigNum (strict)"(error in=w2780, "Value"=0) -> (error out=w2785:errorcluster)  [unwired: 1 in, 1 out]
                n1216 = property on="B-Change at..." class="DigNum (strict)"(error in=w2785, "Value"=0) -> (error out=w2784:errorcluster)  [unwired: 1 in, 1 out]
                n1217 = property on="C-Change at..." class="DigNum (strict)"(error in=w2784, "Value"=0) -> (error out=w2779:errorcluster)  [unwired: 1 in, 1 out]
              }
              frame True {
              }
            }
            n1218 = local read "Mode"() -> (w2765:T8)
            n1219 = case shown="0..2, Default" w2765 {
              tunnel: [w2790 w2793 w2796] -> w2763
              tunnel: [w2790 w2792 w2796] -> w2762
              tunnel: [w2790 w2792 w2796] -> w2761
              tunnel: [FALSE TRUE TRUE] -> w2764
              tunnel: [w2789 w2794 w2797] -> w2760
              tunnel: w2752 -> [w2789 w2794 w2797]
              tunnel: w2755 -> [_ w2793 _]
              frame 0..2, Default {
                w2790 = T15."Enabled" ("Disabled")
                # "Instr3 is overriden by Instr1. No changes will be done to Instr3."
                # "Modes where Instr3 is not working by itself"
              }
              frame 3, 5, 7, 11, 13, 14 {
                w2792 = T15."Disabled and Grayed Out" ("Disabled")
                # "Modes where Instr3 is AC and available"
              }
              frame 4, 6, 8..10, 12, 15 {
                w2796 = T15."Disabled and Grayed Out" ("Disabled")
                # "Modes where Instr3 is DC and available"
              }
            }
            n1220 = case shown="True" w2764 {
              tunnel: w2763 -> [_ w2776]
              tunnel: w2762 -> [_ w2775]
              tunnel: w2761 -> [_ w2774]
              tunnel: w2760 -> [w2771 w2773]
              tunnel: [w2771 w2772] -> w2757
              frame False {
                # "Don't make any changes to Instr3"
              }
              frame True {
                # "Instr3"
                n1221 = property on="A-Change at..." class="DigNum (strict)"(error in=w2773, "DisabledEnum"=w2776) -> (error out=w2777:errorcluster)  [unwired: 1 in, 1 out]
                n1222 = property on="B-Change at..." class="DigNum (strict)"(error in=w2777, "DisabledEnum"=w2775) -> (error out=w2778:errorcluster)  [unwired: 1 in, 1 out]
                n1223 = property on="C-Change at..." class="DigNum (strict)"(error in=w2778, "DisabledEnum"=w2774) -> (error out=w2772:errorcluster)  [unwired: 1 in, 1 out]
              }
            }
            n1224 = property on="Update" class="Bool (strict)"(error in=w2757) -> (error out=w2759:errorcluster, "Value"=w2753:bool)  [unwired: 1 in, 1 out]
            n1225 = property on="Update" class="Bool (strict)"(error in=w2759, "Val(Sgnl)"=w2753) -> (error out=w2758:errorcluster)  [unwired: 1 in, 1 out]
            n1226 = property on="btnSaveAs" class="Bool"(error in=w2758, "DisabledEnum"=w2766) -> (error out=w2768:errorcluster)  [unwired: 1 in, 1 out]
            n1227 = property on="btnSave" class="Bool"(error in=w2768, "DisabledEnum"=w2766) -> (error out=w2767:errorcluster)  [unwired: 1 in, 1 out]
          }
          event Value Change {
            w2806 = T15."Enabled" ("Disabled")
            w2809 = FALSE ("StartMeas")
            # "Aperture change is a value that does not affect others for the instrument. It only needs to be saved."
            n1228 = event-data() -> ()  [unwired: 1 in, 6 out]
            n1229 = local read "Mode"() -> (w2805:T8)
            n1230 = case shown="Default" w2805 {
              tunnel: [w2811 w2814 w2819] -> w2802
              tunnel: [w2811 w2813 w2818] -> w2801
              tunnel: [w2811 w2813 w2817] -> w2800
              frame 0..2 {
                # "Cases with Instr1 only"
                n1231 = local read "Instr1"() -> (w2812:T2)
                n1232 = Unbundle By Name(w2812) -> ("Aperture (cycles)"=w2811:i32)
              }
              frame 5..8, 11, 12 {
                # "Cases with Instr1 and Instr3"
                n1233 = local read "Instr1"() -> (w2816:T2)
                n1234 = local read "Instr3"() -> (w2815:T2)
                n1235 = Unbundle By Name(w2816) -> ("Aperture (cycles)"=w2813:i32)
                n1236 = Unbundle By Name(w2815) -> ("Aperture (cycles)"=w2814:i32)
              }
              frame Default {
                # "Cases with all instruments"
                n1237 = local read "Instr1"() -> (w2822:T2)
                n1238 = local read "Instr2"() -> (w2821:T2)
                n1239 = local read "Instr3"() -> (w2820:T2)
                n1240 = Unbundle By Name(w2821) -> ("Aperture (cycles)"=w2818:i32)
                n1241 = Unbundle By Name(w2822) -> ("Aperture (cycles)"=w2817:i32)
                n1242 = Unbundle By Name(w2820) -> ("Aperture (cycles)"=w2819:i32)
              }
            }
            n1243 = local read "Device(s)Settings"() -> (w2803:T1)
            n1244 = Bundle By Name(cluster=w2803, "Instr1.Aperture (cycles)"=w2800, "Instr2.Aperture (cycles)"=w2801, "Instr3.Aperture (cycles)"=w2802) -> (w2804:T1)
            n1245 = local write "Device(s)Settings"(w2804) -> ()
            n1246 = property on="btnSaveAs" class="Bool"(error in=w2799, "DisabledEnum"=w2806) -> (error out=w2808:errorcluster)  [unwired: 1 in, 1 out]
            n1247 = property on="btnSave" class="Bool"(error in=w2808, "DisabledEnum"=w2806) -> (error out=w2807:errorcluster)  [unwired: 1 in, 1 out]
          }
          event Value Change {
            w2830 = T15."Enabled" ("Disabled")
            w2833 = FALSE ("StartMeas")
            # "Frequency only affects AC instruments, so this event can only be activated depending on instrument and Mode.\n\"Mode change\" event already took care of enabling/disabling the Frequency controls in the different modes and instrumenst as needed."
            # "Frequency change is a value that does not affect others in the instrument. It only needs to be saved."
            n1248 = event-data() -> ()  [unwired: 1 in, 6 out]
            n1249 = local read "Mode"() -> (w2829:T8)
            n1250 = case shown="5..8, 11, 12" w2829 {
              tunnel: [w2835 w2838 w2843] -> w2826
              tunnel: [w2835 w2837 w2842] -> w2825
              tunnel: [w2835 w2837 w2841] -> w2824
              frame 0..2 {
                # "Cases with Instr1 only"
                n1251 = local read "Instr1"() -> (w2836:T2)
                n1252 = Unbundle By Name(w2836) -> ("FreqOut (Hz)"=w2835:dbl)
              }
              frame 5..8, 11, 12 {
                # "Cases with Instr1 and Instr3"
                n1253 = local read "Instr1"() -> (w2840:T2)
                n1254 = local read "Instr3"() -> (w2839:T2)
                n1255 = Unbundle By Name(w2840) -> ("FreqOut (Hz)"=w2837:dbl)
                n1256 = Unbundle By Name(w2839) -> ("FreqOut (Hz)"=w2838:dbl)
              }
              frame Default {
                # "Cases with all instruments"
                n1257 = local read "Instr1"() -> (w2846:T2)
                n1258 = local read "Instr2"() -> (w2845:T2)
                n1259 = local read "Instr3"() -> (w2844:T2)
                n1260 = Unbundle By Name(w2845) -> ("FreqOut (Hz)"=w2842:dbl)
                n1261 = Unbundle By Name(w2846) -> ("FreqOut (Hz)"=w2841:dbl)
                n1262 = Unbundle By Name(w2844) -> ("FreqOut (Hz)"=w2843:dbl)
              }
            }
            n1263 = local read "Device(s)Settings"() -> (w2827:T1)
            n1264 = Bundle By Name(cluster=w2827, "Instr1.FreqOut (Hz)"=w2824, "Instr2.FreqOut (Hz)"=w2825, "Instr3.FreqOut (Hz)"=w2826) -> (w2828:T1)
            n1265 = local write "Device(s)Settings"(w2828) -> ()
            n1266 = property on="btnSaveAs" class="Bool"(error in=w2823, "DisabledEnum"=w2830) -> (error out=w2832:errorcluster)  [unwired: 1 in, 1 out]
            n1267 = property on="btnSave" class="Bool"(error in=w2832, "DisabledEnum"=w2830) -> (error out=w2831:errorcluster)  [unwired: 1 in, 1 out]
          }
          event Value Change {
            w2854 = T15."Enabled" ("Disabled")
            w2857 = FALSE ("StartMeas")
            # "Pass all the values in the Safety Trips cluster of each Instrument to their Device(s)Settings counterparts"
            n1268 = event-data() -> ()  [unwired: 1 in, 6 out]
            n1269 = local read "Mode"() -> (w2852:T8)
            n1270 = case shown="0..2" w2852 {
              tunnel: [w2859 w2862 w2867] -> w2849
              tunnel: [w2859 w2861 w2866] -> w2848
              tunnel: [w2859 w2861 w2865] -> w2847
              frame 0..2 {
                # "Cases with Instr1 only"
                n1271 = local read "Instr1"() -> (w2860:T2)
                n1272 = Unbundle By Name(w2860) -> ("Safety Trips"=w2859:T5)
              }
              frame 5..8, 11, 12 {
                # "Cases with Instr1 and Instr3"
                n1273 = local read "Instr1"() -> (w2864:T2)
                n1274 = local read "Instr3"() -> (w2863:T2)
                n1275 = Unbundle By Name(w2864) -> ("Safety Trips"=w2861:T5)
                n1276 = Unbundle By Name(w2863) -> ("Safety Trips"=w2862:T5)
              }
              frame Default {
                # "Cases with all instruments"
                n1277 = local read "Instr1"() -> (w2870:T2)
                n1278 = local read "Instr2"() -> (w2869:T2)
                n1279 = local read "Instr3"() -> (w2868:T2)
                n1280 = Unbundle By Name(w2869) -> ("Safety Trips"=w2866:T5)
                n1281 = Unbundle By Name(w2870) -> ("Safety Trips"=w2865:T5)
                n1282 = Unbundle By Name(w2868) -> ("Safety Trips"=w2867:T5)
              }
            }
            n1283 = local read "Device(s)Settings"() -> (w2850:T1)
            n1284 = Bundle By Name(cluster=w2850, "Instr1.Safety Trips"=w2847, "Instr2.Safety Trips"=w2848, "Instr3.Safety Trips"=w2849) -> (w2851:T1)
            n1285 = local write "Device(s)Settings"(w2851) -> ()
            n1286 = property on="btnSaveAs" class="Bool"(error in=w2853, "DisabledEnum"=w2854) -> (error out=w2856:errorcluster)  [unwired: 1 in, 1 out]
            n1287 = property on="btnSave" class="Bool"(error in=w2856, "DisabledEnum"=w2854) -> (error out=w2855:errorcluster)  [unwired: 1 in, 1 out]
          }
          event "Handle", "MeasName", "ID Query", "Reset": Value Change {
            w2876 = T15."Enabled" ("Disabled")
            w2878 = FALSE ("StartMeas")
            # "The \"Update\" event call takes care of saving any changed controls"
            # "Update Device(s)Settings"
            # "These controls may be passed just as they are without processing or verification"
            n1288 = event-data() -> ()  [unwired: 1 in, 6 out]
            n1289 = property on="btnSave" class="Bool"(error in=w2873, "DisabledEnum"=w2876) -> (error out=w2875:errorcluster)  [unwired: 1 in, 1 out]
            n1290 = property on="btnSaveAs" class="Bool"(error in=w2875, "DisabledEnum"=w2876) -> (error out=w2874:errorcluster)  [unwired: 1 in, 1 out]
            n1291 = property on="Update" class="Bool (strict)"(error in=w2874) -> (error out=w2877:errorcluster, "Value"=w2871:bool)  [unwired: 1 in, 1 out]
            n1292 = property on="Update" class="Bool (strict)"(error in=w2877, "Val(Sgnl)"=w2871) -> (error out=w2872:errorcluster)  [unwired: 1 in, 1 out]
          }
          event "Measurement RefreshTime (ms)": Value Change {
            w2882 = T15."Enabled" ("Disabled")
            w2892 = FALSE
            # "Enable the [Save]  and [Save as] buttons if the configuration is saved."
            n1293 = event-data() -> ()  [unwired: 1 in, 1 out]
            n1294 = local read "Device(s)Settings"() -> (w2886:T1)
            n1295 = To Variant(anything=w2886) -> (Variant=w2890:variant)
            n1296 = To Variant(anything="Measurements") -> (Variant=w2887:variant)
            n1297 = call-dynamic "WriteToBaseConfigVariant.vi"("Measurement RefreshTime (ms)"="Measurement RefreshTime (ms)", "error in (no error)"=w2885, "Meas"=w2887, "Config"=w2890, "NHRGridSim in"=w2891) -> ("error out"=w2883:errorcluster, "NHRGridSim out"=w2884:refnum<class "NHRGridSim.lvclass">)  [unwired: 5 in]
            n1298 = property on="btnSave" class="Bool"(error in=w2883, "DisabledEnum"=w2882) -> (error out=w2881:errorcluster)  [unwired: 1 in, 1 out]
            n1299 = property on="btnSaveAs" class="Bool"(error in=w2881, "DisabledEnum"=w2882) -> (error out=w2880:errorcluster)  [unwired: 1 in, 1 out]
          }
          event Value Change {
            w2911 = T15."Enabled" ("Disabled")
            w2914 = FALSE ("StartMeas")
            # "For Instr1 the values of the phases must follow the value of Vout depending on being Three-Phase or Two-Phase mode. The rest of the modes are all for Single-Phase (AC) or Single-Channel (DC) instruments. The frame is to make sure that Instr1, Instr2 and Instr3 get updated before their changes are registered into their Device(s)Settings counterparts."
            # "Instr1"
            # "Turn indexed string into numeric."
            # "Get the present limits that the V Range control has, and the index of the present range selection."
            # "Update Device(s)Settings"
            # "When Vout is changed for Instr1, it requires more management than the other instruments because phases may be involved, and Instr1 may be overriding Instr2 and Instr3 too depending on Mode."
            n1300 = event-data() -> ("NewVal"=w2894:dbl)  [unwired: 1 in]
            n1301 = property on="Voltage (V)" class="Ring (strict)"(error in=w2903) -> (error out=w2907:errorcluster, "Strings []"=w2908:string[], "Value"=w2905:u16)  [unwired: 1 in, 1 out]
            n1302 = Index Array(array=w2908, index=w2905) -> (element=w2906:string)
            n1303 = Scan From String(format string="%f", input string=w2906, error in=w2907) -> (error out=w2898:errorcluster, output 1=w2895:dbl)  [unwired: 2 in, 2 out]
            n1304 = local read "Mode"() -> (w2893:T8)
            n1305 = Less?(x=w2895, y=w2894) -> (x < y?=w2896:bool)
            n1306 = Merge Errors(w2903, w2898) -> (w2902:errorcluster)
            n1307 = case shown="True" w2896 {
              tunnel: w2893 -> [_ w2962]
              frame False {
                # "No voltage range adjustment needed. Vout falls within present range."
              }
              frame True {
                w2961 = u16 1 ("Ranges.Voltage (V)")
                # "Increase range so that Vout can fit within it."
                n1308 = case shown="0..2" w2962 {
                  tunnel: w2961 -> [w2965 w2970 _]
                  frame 0..2 {
                    # "Instr1 overrides Instr2 and Instr3."
                    n1309 = local read "Instr2"() -> (w2968:T2)
                    n1310 = Bundle By Name(cluster=w2968, "Ranges.Voltage (V)"=w2965) -> (w2969:T2)
                    n1311 = local read "Instr3"() -> (w2967:T2)
                    n1312 = Bundle By Name(cluster=w2967, "Ranges.Voltage (V)"=w2965) -> (w2966:T2)
                    n1313 = local write "Instr2"(w2969) -> ()
                    n1314 = local write "Instr3"(w2966) -> ()
                  }
                  frame 5..8, 11, 12 {
                    # "Instr1 overrides Instr2 only."
                    n1315 = local read "Instr2"() -> (w2971:T2)
                    n1316 = Bundle By Name(cluster=w2971, "Ranges.Voltage (V)"=w2970) -> (w2972:T2)
                    n1317 = local write "Instr2"(w2972) -> ()
                  }
                  frame Default {
                    # "Neither Instr2 nor Instr3 are affected by Instr1 settings."
                    # "Instr1 is a single instrument itself."
                  }
                }
                n1318 = local read "Instr1"() -> (w2964:T2)
                n1319 = Bundle By Name(cluster=w2964, "Ranges.Voltage (V)"=w2961) -> (w2963:T2)
                n1320 = local write "Instr1"(w2963) -> ()
              }
            }
            n1321 = local read "Mode"() -> (w2899:T8)
            n1322 = flat-sequence {
              tunnel: w2894 -> [w2917]
              tunnel: w2902 -> [w2918]
              tunnel: [w2918] -> w2901
              tunnel: w2899 -> [w2916]
              frame #0 {
                n1323 = case shown="0" w2916 {
                  tunnel: w2917 -> [w2941 w2946 w2952 w2955 w2960]
                  tunnel: [w2940 w2946 w2950 w2955 w2960] -> w2921
                  tunnel: [w2940 w2946 w2950 w2955 w2959] -> w2920
                  tunnel: [w2940 w2946 0.0 ("NewVal") 0.0 ("NewVal") w2959] -> w2919
                  tunnel: [TRUE TRUE TRUE TRUE FALSE] -> w2923
                  tunnel: [TRUE TRUE FALSE FALSE FALSE] -> w2922
                  frame 0 {
                    # "Works as Instr1/2/3"
                    # "The three phase values are equal for (L-N)"
                    n1324 = Square Root(x=3.0) -> (sqrt(x)=w2942:dbl)
                    n1325 = Divide(x=w2941, y=w2942) -> (x/y=w2940:dbl)
                  }
                  frame 1, 2 {
                    # "Works as Instr1/2/3"
                    # "All three channels joined as a single output"
                  }
                  frame 5, 6 {
                    # "Works as Instr1/2 only"
                    # "Two channels joined as a Two-Phase output"
                    n1326 = Divide(x=w2952, y=2.0) -> (x/y=w2950:dbl)
                  }
                  frame 7, 8, 11, 12 {
                    # "Works as Instr1/2 only"
                    # "Two channels joined as a single output"
                  }
                  frame Default {
                    w2959 = 0.0 ("NewVal")
                    # "Works as Instr1 only"
                    # "Instr1 is alone and\nuses only one channel"
                  }
                }
                n1327 = case shown="True" w2922 {
                  tunnel: w2921 -> [_ w2929]
                  tunnel: w2920 -> [_ w2928]
                  tunnel: w2919 -> [_ w2927]
                  tunnel: w2917 -> [_ w2926]
                  frame False {
                  }
                  frame True {
                    n1328 = local read "Instr3"() -> (w2930:T2)
                    n1329 = Bundle By Name(cluster=w2930, "Phases.A-Volts (V)"=w2929, "Phases.B-Volts (V)"=w2928, "Phases.C-Volts (V)"=w2927, "Vout (V)"=w2926) -> (w2931:T2)
                    n1330 = local write "Instr3"(w2931) -> ()
                  }
                }
                n1331 = case shown="True" w2923 {
                  tunnel: w2921 -> [_ w2935]
                  tunnel: w2920 -> [_ w2934]
                  tunnel: w2919 -> [_ w2933]
                  tunnel: w2917 -> [_ w2932]
                  frame False {
                  }
                  frame True {
                    n1332 = local read "Instr2"() -> (w2937:T2)
                    n1333 = Bundle By Name(cluster=w2937, "Phases.A-Volts (V)"=w2935, "Phases.B-Volts (V)"=w2934, "Phases.C-Volts (V)"=w2933, "Vout (V)"=w2932) -> (w2936:T2)
                    n1334 = local write "Instr2"(w2936) -> ()
                  }
                }
                n1335 = local read "Instr1"() -> (w2924:T2)
                n1336 = Bundle By Name(cluster=w2924, "Vout (V)"=w2917, "Phases.A-Volts (V)"=w2921, "Phases.B-Volts (V)"=w2920, "Phases.C-Volts (V)"=w2919) -> (w2925:T2)
                n1337 = local write "Instr1"(w2925) -> ()
              }
            }
            n1338 = property on="Update" class="Bool (strict)"(error in=w2901) -> (error out=w2909:errorcluster, "Value"=w2897:bool)  [unwired: 1 in, 1 out]
            n1339 = property on="Update" class="Bool (strict)"(error in=w2909, "Val(Sgnl)"=w2897) -> (error out=w2900:errorcluster)  [unwired: 1 in, 1 out]
            n1340 = property on="btnSaveAs" class="Bool"(error in=w2900, "DisabledEnum"=w2911) -> (error out=w2913:errorcluster)  [unwired: 1 in, 1 out]
            n1341 = property on="btnSave" class="Bool"(error in=w2900, "DisabledEnum"=w2911) -> (error out=w2912:errorcluster)  [unwired: 1 in, 1 out]
            n1342 = Merge Errors(w2912, w2913) -> (w2910:errorcluster)
          }
          event Value Change {
            w2989 = T15."Enabled" ("Disabled")
            w2992 = FALSE ("StartMeas")
            # "There's no need to check for Mode because Instr2 can only appear in the interface to be operated by the user when it is working alone as a separate instrument."
            # "Instr2"
            # "Turn that indexed string into its actual numeric value."
            # "Get the present limits that the V Range control has, and the index of the present range selection."
            # "Update Device(s)Settings"
            # "Instr2 can only detect a Vout change when it's not being overriden by Instr1 and has its own instrument panel visible so that the user can operate its controls."
            n1343 = event-data() -> ("NewVal"=w2973:dbl)  [unwired: 1 in]
            n1344 = property on="Voltage (V)" class="Ring (strict)"(error in=w2980) -> (error out=w2985:errorcluster, "Strings []"=w2986:string[], "Value"=w2983:u16)  [unwired: 1 in, 1 out]
            n1345 = Index Array(array=w2986, index=w2983) -> (element=w2984:string)
            n1346 = Scan From String(format string="%f", input string=w2984, error in=w2985) -> (error out=w2976:errorcluster, output 1=w2974:dbl)  [unwired: 2 in, 2 out]
            n1347 = Merge Errors(w2980, w2976) -> (w2979:errorcluster)
            n1348 = Less?(x=w2974, y=w2973) -> (x < y?=w2981:bool)
            n1349 = case shown="True" w2981 {
              frame False {
                # "No voltage range adjustment needed. Vout falls within present range."
              }
              frame True {
                # "Increase range so that Vout can fit within it."
                n1350 = local read "Instr2"() -> (w3001:T2)
                n1351 = Bundle By Name(cluster=w3001, "Ranges.Voltage (V)"=u16 1) -> (w3000:T2)
                n1352 = local write "Instr2"(w3000) -> ()
              }
            }
            n1353 = flat-sequence {
              tunnel: w2979 -> [w2997]
              tunnel: [w2997] -> w2978
              tunnel: w2973 -> [w2994]
              frame #0 {
                w2998 = 0.0 ("NewVal")
                # "The frame is only to ensure that the cluster is updated before \"Update\" is called."
                n1354 = local read "Instr2"() -> (w2996:T2)
                n1355 = Bundle By Name(cluster=w2996, "Phases.C-Volts (V)"=w2998, "Phases.B-Volts (V)"=w2998, "Phases.A-Volts (V)"=w2994, "Vout (V)"=w2994) -> (w2995:T2)
                n1356 = local write "Instr2"(w2995) -> ()
              }
            }
            n1357 = property on="Update" class="Bool (strict)"(error in=w2978) -> (error out=w2987:errorcluster, "Value"=w2975:bool)  [unwired: 1 in, 1 out]
            n1358 = property on="Update" class="Bool (strict)"(error in=w2987, "Val(Sgnl)"=w2975) -> (error out=w2977:errorcluster)  [unwired: 1 in, 1 out]
            n1359 = property on="btnSaveAs" class="Bool"(error in=w2977, "DisabledEnum"=w2989) -> (error out=w2991:errorcluster)  [unwired: 1 in, 1 out]
            n1360 = property on="btnSave" class="Bool"(error in=w2977, "DisabledEnum"=w2989) -> (error out=w2990:errorcluster)  [unwired: 1 in, 1 out]
            n1361 = Merge Errors(w2990, w2991) -> (w2988:errorcluster)
          }
          event Value Change {
            w3018 = T15."Enabled" ("Disabled")
            w3021 = FALSE ("StartMeas")
            # "There's no need to check for Mode because Instr3 can only appear in the interface to be operated by the user when it is working alone as a separate instrument."
            # "Instr3"
            # "Turn that indexed string into its actual numeric value."
            # "Get the present limits that the V Range control has, and the index of the present range selection."
            # "Update Device(s)Settings"
            # "Instr3 can only detect a Vout change when it's not being overriden by Instr1 and has its own instrument panel visible so that the user can operate its controls."
            n1362 = event-data() -> ("NewVal"=w3002:dbl)  [unwired: 1 in]
            n1363 = property on="Voltage (V)" class="Ring (strict)"(error in=w3009) -> (error out=w3014:errorcluster, "Strings []"=w3015:string[], "Value"=w3012:u16)  [unwired: 1 in, 1 out]
            n1364 = Index Array(array=w3015, index=w3012) -> (element=w3013:string)
            n1365 = Scan From String(format string="%f", input string=w3013, error in=w3014) -> (error out=w3005:errorcluster, output 1=w3003:dbl)  [unwired: 2 in, 2 out]
            n1366 = Merge Errors(w3009, w3005) -> (w3008:errorcluster)
            n1367 = Less?(x=w3003, y=w3002) -> (x < y?=w3010:bool)
            n1368 = case shown="True" w3010 {
              frame False {
                # "No voltage range adjustment needed. Vout falls within present range."
              }
              frame True {
                # "Increase range so that Vout can fit within it."
                n1369 = local read "Instr3"() -> (w3030:T2)
                n1370 = Bundle By Name(cluster=w3030, "Ranges.Voltage (V)"=u16 1) -> (w3029:T2)
                n1371 = local write "Instr3"(w3029) -> ()
              }
            }
            n1372 = flat-sequence {
              tunnel: w3008 -> [w3026]
              tunnel: [w3026] -> w3007
              tunnel: w3002 -> [w3023]
              frame #0 {
                w3027 = 0.0 ("NewVal")
                # "The frame is only to ensure that the cluster is updated before \"Update\" is called."
                n1373 = local read "Instr3"() -> (w3025:T2)
                n1374 = Bundle By Name(cluster=w3025, "Phases.C-Volts (V)"=w3027, "Phases.B-Volts (V)"=w3027, "Phases.A-Volts (V)"=w3023, "Vout (V)"=w3023) -> (w3024:T2)
                n1375 = local write "Instr3"(w3024) -> ()
              }
            }
            n1376 = property on="Update" class="Bool (strict)"(error in=w3007) -> (error out=w3016:errorcluster, "Value"=w3004:bool)  [unwired: 1 in, 1 out]
            n1377 = property on="Update" class="Bool (strict)"(error in=w3016, "Val(Sgnl)"=w3004) -> (error out=w3006:errorcluster)  [unwired: 1 in, 1 out]
            n1378 = property on="btnSaveAs" class="Bool"(error in=w3006, "DisabledEnum"=w3018) -> (error out=w3020:errorcluster)  [unwired: 1 in, 1 out]
            n1379 = property on="btnSave" class="Bool"(error in=w3006, "DisabledEnum"=w3018) -> (error out=w3019:errorcluster)  [unwired: 1 in, 1 out]
            n1380 = Merge Errors(w3019, w3020) -> (w3017:errorcluster)
          }
          event Value Change {
            w3042 = T15."Enabled" ("Disabled")
            w3044 = FALSE ("StartMeas")
            # "Get all the present phase voltages in Instr1"
            # "Update Device(s)Settings"
            # "Only Instr1 can be configured to be multiphase. Therefore, it's the only instrument which provides user access to modify any phase voltages individually.\nThere's no need to check for \"Instr2.PhasesABC\" changes nor \"Instr3. PhasesABC\" changes, because those cases cannot be generated by the user."
            # "Instr1 is the only one that can change phase voltage values. Verify that any new phase voltage value is within range, and if it's not, force it to be."
            n1381 = event-data() -> ("CtlRef"=w3045:refnum<vi>)  [unwired: 1 in, 2 out]
            n1382 = local read "Instr1"() -> (w3041:T2)
            n1383 = Unbundle By Name(w3041) -> ("Phases.A-Volts (V)"=w3039:dbl, "Phases.B-Volts (V)"=w3040:dbl, "Phases.C-Volts (V)"=w3038:dbl)
            n1384 = local read "Mode"() -> (w3046:T8)
            n1385 = case shown="0" w3046 {
              tunnel: w3045 -> [_ w3063 w3099]
              tunnel: [w3048 w3057 w3094] -> w3031
              tunnel: w3040 -> [_ w3058 w3097]
              tunnel: w3039 -> [_ w3059 w3095]
              tunnel: w3038 -> [_ _ w3096]
              tunnel: w3037 -> [w3048 w3062 w3098]
              frame Default {
                # "The rest of the modes have no phases, so there's no need to adjust anything."
              }
              frame 5, 6 {
                # "Set the voltage level range to an adequate value depending if the total is within range or if it could have exceeded it."
                # "Two-Phase Modes"
                n1386 = property class="DigNum (strict)"(reference=w3063, error in=w3062) -> (reference out=w3060:refnum<vi>, error out=w3061:errorcluster, "Label.Text"=w3066:string)
                n1387 = Add(x=w3059, y=w3058) -> (x+y=w3068:dbl)
                n1388 = Greater?(x=w3068, y=500.0) -> (0:w3065:bool)
                n1389 = Close Reference(reference=w3060, error in (no error)=w3061) -> (error out=w3057:errorcluster)
                n1390 = case shown="True" w3065 {
                  tunnel: w3066 -> [_ w3085]
                  tunnel: "A-Volts (V)" -> [_ w3084]
                  tunnel: w3059 -> [w3071 w3082]
                  tunnel: w3058 -> [w3070 w3081]
                  tunnel: [w3071 w3080] -> w3049
                  tunnel: [w3070 w3079] -> w3050
                  tunnel: [w3072 u16 1 ("f")] -> w3051
                  tunnel: [w3069 500.0] -> w3052
                  frame False {
                    # "The combined value of both phases generates a value of Vout within valid limits."
                    # "Depending on the combined result of the phase values, adjust to the adequate voltage range level"
                    n1391 = Add(x=w3071, y=w3070) -> (x+y=w3069:dbl)
                    n1392 = Greater?(x=w3069, y=350.0) -> (0:w3075:bool)
                    n1393 = Select(t=u16 1, s=w3075, f=u16 0) -> (s? t:f=w3072:u16)
                  }
                  frame True, Default {
                    n1394 = Equal?(x=w3085, y=w3084) -> (x = y?=w3083:bool)
                    n1395 = case shown="True" w3083 {
                      tunnel: w3082 -> [w3088 w3091]
                      tunnel: w3081 -> [w3086 w3092]
                      tunnel: [w3087 w3091] -> w3080
                      tunnel: [w3086 w3090] -> w3079
                      frame True {
                        # "Adjust it so that the sum of both phases doesn't exceed 500V"
                        # "If Phase-A value exceeded max Two-Phase V range"
                        n1396 = Subtract(x=500.0 ("y"), y=w3088) -> (x-y=w3087:dbl)
                      }
                      frame False {
                        # "Adjust it so that the sum of both phases doesn't exceed 500V"
                        # "If Phase-B value exceeded max Two-Phase V range"
                        n1397 = Subtract(x=500.0 ("y"), y=w3092) -> (x-y=w3090:dbl)
                      }
                    }
                  }
                }
                n1398 = local read "Instr1"() -> (w3056:T2)
                n1399 = Bundle By Name(cluster=w3056, "Vout (V)"=w3052, "Ranges.Voltage (V)"=w3051, "Phases.A-Volts (V)"=w3049, "Phases.B-Volts (V)"=w3050) -> (w3055:T2)
                n1400 = local write "Instr1"(w3055) -> ()
                n1401 = local read "Instr2"() -> (w3053:T2)
                n1402 = Bundle By Name(cluster=w3053, "Vout (V)"=w3052, "Ranges.Voltage (V)"=w3051, "Phases.A-Volts (V)"=w3049, "Phases.B-Volts (V)"=w3050) -> (w3054:T2)
                n1403 = local write "Instr2"(w3054) -> ()
              }
              frame 0 {
                # "Do the phases math to get the present value of Vout"
                # "Check if the contribution all  phase voltages exceeds the 606V three phase maximum."
                # "Three-Phase Mode will check against the possibility of exceeding 606V, and which adequate voltage range level to use."
                n1404 = property class="DigNum (strict)"(reference=w3099, error in=w3098) -> (error out=w3094:errorcluster, "Label.Text"=w3107:string)  [unwired: 1 out]
                n1405 = Compound Arithmetic op=ADD(w3095, w3097, w3096) -> (w3102:dbl)
                n1406 = Square Root(x=3.0) -> (sqrt(x)=w3104:dbl)
                n1407 = Divide(x=w3102, y=3.0) -> (x/y=w3101:dbl)
                n1408 = Multiply(x=w3104, y=w3101) -> (x*y=w3103:dbl)
                n1409 = Greater?(x=w3103, y=606.0) -> (0:w3106:bool)
                n1410 = case shown="True" w3106 {
                  tunnel: w3107 -> [_ w3142]
                  tunnel: w3103 -> [w3113 _]
                  tunnel: w3097 -> [w3110 w3141]
                  tunnel: w3096 -> [w3109 w3140]
                  tunnel: w3095 -> [w3111 w3135]
                  frame False {
                    # "If the total value of all phases combined did not exceed the maximum 606V of the three phase Mode, there's no need to adjust their values. Check instead which is the correct voltage range that can contain the result. Adjust the range to be either 303V or 606V depending on the magnitude of the new total."
                    n1411 = Greater?(x=w3113, y=303.0) -> (0:w3122:bool)
                    n1412 = Select(t=u16 1, s=w3122, f=u16 0) -> (s? t:f=w3112:u16)
                    n1413 = local read "Instr1"() -> (w3118:T2)
                    n1414 = Bundle By Name(cluster=w3118, "Vout (V)"=w3113, "Ranges.Voltage (V)"=w3112, "Phases.A-Volts (V)"=w3111, "Phases.B-Volts (V)"=w3110, "Phases.C-Volts (V)"=w3109) -> (w3119:T2)
                    n1415 = local write "Instr1"(w3119) -> ()
                    n1416 = local read "Instr2"() -> (w3117:T2)
                    n1417 = Bundle By Name(cluster=w3117, "Vout (V)"=w3113, "Ranges.Voltage (V)"=w3112, "Phases.A-Volts (V)"=w3111, "Phases.B-Volts (V)"=w3110, "Phases.C-Volts (V)"=w3109) -> (w3116:T2)
                    n1418 = local write "Instr2"(w3116) -> ()
                    n1419 = local read "Instr3"() -> (w3114:T2)
                    n1420 = Bundle By Name(cluster=w3114, "Vout (V)"=w3113, "Ranges.Voltage (V)"=w3112, "Phases.A-Volts (V)"=w3111, "Phases.B-Volts (V)"=w3110, "Phases.C-Volts (V)"=w3109) -> (w3115:T2)
                    n1421 = local write "Instr3"(w3115) -> ()
                  }
                  frame True, Default {
                    # "Set the Instr1 V range to the 606V choice because the new value would have exceeded it. Due to that, Vout has to be set to the 606V maximum too."
                    n1422 = case shown="\"A-Volts (V)\", Default" w3142 {
                      tunnel: w3141 -> [w3144 _ w3162]
                      tunnel: w3140 -> [w3143 w3152 _]
                      tunnel: [w3145 w3153 w3161] -> w3124
                      tunnel: w3135 -> [_ w3153 w3161]
                      tunnel: [w3144 w3154 w3162] -> w3125
                      tunnel: [w3143 w3152 w3163] -> w3126
                      frame "A-Volts (V)", Default {
                        w3147 = 3.0 ("y")
                        # "Adjust Phase A volts so that the contribution of all phases adds up to 606V"
                        n1423 = Compound Arithmetic op=ADD(w3144, w3143) -> (w3151:dbl)
                        n1424 = Multiply(x=606.0 ("y"), y=w3147) -> (x*y=w3148:dbl)
                        n1425 = Square Root(x=w3147) -> (sqrt(x)=w3149:dbl)
                        n1426 = Divide(x=w3148, y=w3149) -> (x/y=w3150:dbl)
                        n1427 = Subtract(x=w3150, y=w3151) -> (x-y=w3145:dbl)
                      }
                      frame "B-Volts (V)" {
                        w3157 = 3.0 ("y")
                        # "Adjust Phase B volts so that the contribution of all phases adds up to 606V"
                        n1428 = Compound Arithmetic op=ADD(w3153, w3152) -> (w3155:dbl)
                        n1429 = Multiply(x=606.0 ("y"), y=w3157) -> (x*y=w3159:dbl)
                        n1430 = Square Root(x=w3157) -> (sqrt(x)=w3158:dbl)
                        n1431 = Divide(x=w3159, y=w3158) -> (x/y=w3156:dbl)
                        n1432 = Subtract(x=w3156, y=w3155) -> (x-y=w3154:dbl)
                      }
                      frame "C-Volts (V)" {
                        w3165 = 3.0 ("y")
                        # "Adjust Phase C volts so that the contribution of all phases adds up to 606V"
                        n1433 = Compound Arithmetic op=ADD(w3161, w3162) -> (w3169:dbl)
                        n1434 = Multiply(x=606.0 ("y"), y=w3165) -> (x*y=w3166:dbl)
                        n1435 = Square Root(x=w3165) -> (sqrt(x)=w3167:dbl)
                        n1436 = Divide(x=w3166, y=w3167) -> (x/y=w3168:dbl)
                        n1437 = Subtract(x=w3168, y=w3169) -> (x-y=w3163:dbl)
                      }
                    }
                    n1438 = local read "Instr1"() -> (w3139:T2)
                    n1439 = Bundle By Name(cluster=w3139, "Vout (V)"=606.0 ("y"), "Ranges.Voltage (V)"=u16 1 ("Value"), "Phases.A-Volts (V)"=w3124, "Phases.B-Volts (V)"=w3125, "Phases.C-Volts (V)"=w3126) -> (w3138:T2)
                    n1440 = local write "Instr1"(w3138) -> ()
                    n1441 = local read "Instr2"() -> (w3131:T2)
                    n1442 = Bundle By Name(cluster=w3131, "Vout (V)"=606.0 ("y"), "Ranges.Voltage (V)"=u16 1 ("Value"), "Phases.A-Volts (V)"=w3124, "Phases.B-Volts (V)"=w3125, "Phases.C-Volts (V)"=w3126) -> (w3132:T2)
                    n1443 = local write "Instr2"(w3132) -> ()
                    n1444 = local read "Instr3"() -> (w3130:T2)
                    n1445 = Bundle By Name(cluster=w3130, "Vout (V)"=606.0 ("y"), "Ranges.Voltage (V)"=u16 1 ("Value"), "Phases.A-Volts (V)"=w3124, "Phases.B-Volts (V)"=w3125, "Phases.C-Volts (V)"=w3126) -> (w3129:T2)
                    n1446 = local write "Instr3"(w3129) -> ()
                  }
                }
              }
            }
            n1447 = property on="Update" class="Bool (strict)"(error in=w3031) -> (error out=w3043:errorcluster, "Value"=w3036:bool)  [unwired: 1 in, 1 out]
            n1448 = property on="btnSaveAs" class="Bool"(error in=w3031, "DisabledEnum"=w3042) -> (error out=w3033:errorcluster)  [unwired: 1 in, 1 out]
            n1449 = property on="btnSave" class="Bool"(error in=w3031, "DisabledEnum"=w3042) -> (error out=w3034:errorcluster)  [unwired: 1 in, 1 out]
            n1450 = property on="Update" class="Bool (strict)"(error in=w3043, "Val(Sgnl)"=w3036) -> (error out=w3032:errorcluster)  [unwired: 1 in, 1 out]
            n1451 = Merge Errors(w3034, w3033, w3032) -> (w3035:errorcluster)
          }
          event Value Change {
            w3177 = T15."Enabled" ("Disabled")
            w3178 = FALSE ("StartMeas")
            # "No need to \"Update\" here because values are passed directly to Device(s)Settings  in the case select structure."
            # "Get all the present phase angles in Instr1"
            # "Only Instr1 can be configured to be multiphase. Therefore, it's the only instrument which provides user access to modify any phase angles individually. There's no need to check for Instr2 or Instr3 for these controls."
            # "Instr1 is the only one that can change phase angle values. Angles should be coerced already only as integers between 0 and 359, and only available for three-phase and two-phase cases."
            n1452 = event-data() -> ()  [unwired: 1 in, 3 out]
            n1453 = local read "Instr1"() -> (w3171:T2)
            n1454 = Unbundle By Name(w3171) -> ("Phases.B-Angle (Deg)"=w3174:i32, "Phases.C-Angle (Deg)"=w3175:i32)
            n1455 = local read "Mode"() -> (w3179:T8)
            n1456 = case shown="0" w3179 {
              tunnel: [w3181 w3186 w3191] -> w3170
              tunnel: w3175 -> [w3182 _ _]
              tunnel: w3174 -> [w3184 w3189 _]
              tunnel: w3173 -> [w3181 w3186 w3191]
              frame 0 {
                # "Three-phase mode is the only one that uses both angles B and C."
                n1457 = local read "Device(s)Settings"() -> (w3185:T1)
                n1458 = Bundle By Name(cluster=w3185, "Instr1.Phases.B-Angle (Deg)"=w3184, "Instr2.Phases.B-Angle (Deg)"=w3184, "Instr3.Phases.B-Angle (Deg)"=w3184, "Instr1.Phases.C-Angle (Deg)"=w3182, "Instr2.Phases.C-Angle (Deg)"=w3182, "Instr3.Phases.C-Angle (Deg)"=w3182) -> (w3183:T1)
                n1459 = local write "Device(s)Settings"(w3183) -> ()
              }
              frame 5, 6 {
                w3187 = 0 ("Instr2.Phases.C-Angle (Deg)")
                # "Two-phse only uses Instr1 and Instr2 together for the B angle. Everything else has to be 0."
                # "Two-phase mode is the only one that uses only angles B."
                n1460 = local read "Device(s)Settings"() -> (w3190:T1)
                n1461 = Bundle By Name(cluster=w3190, "Instr1.Phases.B-Angle (Deg)"=w3189, "Instr2.Phases.B-Angle (Deg)"=w3189, "Instr3.Phases.B-Angle (Deg)"=w3187, "Instr1.Phases.C-Angle (Deg)"=w3187, "Instr2.Phases.C-Angle (Deg)"=w3187, "Instr3.Phases.C-Angle (Deg)"=w3187) -> (w3188:T1)
                n1462 = local write "Device(s)Settings"(w3188) -> ()
              }
              frame Default {
                w3192 = 0 ("Instr2.Phases.C-Angle (Deg)")
                # "Any other Modes doesn't use phase angles, set them to 0 in all instruments."
                n1463 = local read "Device(s)Settings"() -> (w3194:T1)
                n1464 = Bundle By Name(cluster=w3194, "Instr1.Phases.B-Angle (Deg)"=w3192, "Instr2.Phases.B-Angle (Deg)"=w3192, "Instr3.Phases.B-Angle (Deg)"=w3192, "Instr1.Phases.C-Angle (Deg)"=w3192, "Instr2.Phases.C-Angle (Deg)"=w3192, "Instr3.Phases.C-Angle (Deg)"=w3192) -> (w3193:T1)
                n1465 = local write "Device(s)Settings"(w3193) -> ()
              }
            }
            n1466 = property on="btnSave" class="Bool"(error in=w3170, "DisabledEnum"=w3177) -> (error out=w3176:errorcluster)  [unwired: 1 in, 1 out]
            n1467 = property on="btnSaveAs" class="Bool"(error in=w3176, "DisabledEnum"=w3177) -> (error out=w3172:errorcluster)  [unwired: 1 in, 1 out]
          }
          event Value Change {
            w3203 = T15."Enabled" ("Disabled")
            w3204 = FALSE ("StartMeas")
            # "No need to \"Update\" here because values are passed directly to Device(s)Settings in the case select structure."
            # "Get all the present \"Change at\" values in Instr1"
            # "Since Instr1 may override Instr2 and Instr3 in some modes, and it can be three-phase, two-phase or one phase, evaluate what to do depending on Mode."
            n1468 = event-data() -> ()  [unwired: 1 in, 3 out]
            n1469 = local read "Instr1"() -> (w3197:T2)
            n1470 = Unbundle By Name(w3197) -> ("Phases.A-Change at..."=w3200:i32, "Phases.B-Change at..."=w3201:i32, "Phases.C-Change at..."=w3195:i32)
            n1471 = local read "Mode"() -> (w3205:T8)
            n1472 = case shown="0" w3205 {
              tunnel: [w3208 w3215 w3221 w3226 w3231 w3234] -> w3196
              tunnel: w3201 -> [w3209 w3214 _ _ _ _]
              tunnel: w3200 -> [w3211 w3217 w3220 w3225 w3230 _]
              tunnel: w3199 -> [w3208 w3215 w3221 w3226 w3231 w3234]
              tunnel: w3195 -> [w3207 _ _ _ _ _]
              frame 0 {
                # "In three-phase mode all values are used, and affect Instr2 and Instr3 too."
                n1473 = local read "Device(s)Settings"() -> (w3212:T1)
                n1474 = Bundle By Name(cluster=w3212, "Instr1.Phases.A-Change at..."=w3211, "Instr2.Phases.A-Change at..."=w3211, "Instr3.Phases.A-Change at..."=w3211, "Instr1.Phases.B-Change at..."=w3209, "Instr2.Phases.B-Change at..."=w3209, "Instr3.Phases.B-Change at..."=w3209, "Instr1.Phases.C-Change at..."=w3207, "Instr2.Phases.C-Change at..."=w3207, "Instr3.Phases.C-Change at..."=w3207) -> (w3210:T1)
                n1475 = local write "Device(s)Settings"(w3210) -> ()
              }
              frame 5, 6 {
                w3213 = 0 ("Instr1.Phases.C-Change at...")
                # "In two-phase mode \"Chage at\" C is not used. Instr1 and Instr2 are linked."
                n1476 = local read "Device(s)Settings"() -> (w3218:T1)
                n1477 = Bundle By Name(cluster=w3218, "Instr1.Phases.A-Change at..."=w3217, "Instr2.Phases.A-Change at..."=w3217, "Instr1.Phases.B-Change at..."=w3214, "Instr2.Phases.B-Change at..."=w3214, "Instr1.Phases.C-Change at..."=w3213, "Instr2.Phases.C-Change at..."=w3213) -> (w3216:T1)
                n1478 = local write "Device(s)Settings"(w3216) -> ()
              }
              frame 1 {
                w3219 = 0 ("Instr1.Phases.C-Change at...")
                # "Instr1, Instr2 and Instr3 are a single combined one-phase AC instrument."
                n1479 = local read "Device(s)Settings"() -> (w3223:T1)
                n1480 = Bundle By Name(cluster=w3223, "Instr1.Phases.A-Change at..."=w3220, "Instr2.Phases.A-Change at..."=w3220, "Instr3.Phases.A-Change at..."=w3220, "Instr1.Phases.B-Change at..."=w3219, "Instr2.Phases.B-Change at..."=w3219, "Instr3.Phases.B-Change at..."=w3219, "Instr1.Phases.C-Change at..."=w3219, "Instr2.Phases.C-Change at..."=w3219, "Instr3.Phases.C-Change at..."=w3219) -> (w3222:T1)
                n1481 = local write "Device(s)Settings"(w3222) -> ()
              }
              frame 7, 8 {
                w3224 = 0 ("Instr1.Phases.C-Change at...")
                # "Instr1 and Instr2 are a single combined one-phase AC instrument."
                n1482 = local read "Device(s)Settings"() -> (w3228:T1)
                n1483 = Bundle By Name(cluster=w3228, "Instr1.Phases.A-Change at..."=w3225, "Instr2.Phases.A-Change at..."=w3225, "Instr1.Phases.B-Change at..."=w3224, "Instr2.Phases.B-Change at..."=w3224, "Instr1.Phases.C-Change at..."=w3224, "Instr2.Phases.C-Change at..."=w3224) -> (w3227:T1)
                n1484 = local write "Device(s)Settings"(w3227) -> ()
              }
              frame 3, 9, 10, 13 {
                w3229 = 0 ("Instr1.Phases.C-Change at...")
                # "Instr1 is a single one-phase AC instrument."
                n1485 = local read "Device(s)Settings"() -> (w3233:T1)
                n1486 = Bundle By Name(cluster=w3233, "Instr1.Phases.A-Change at..."=w3230, "Instr1.Phases.B-Change at..."=w3229, "Instr1.Phases.C-Change at..."=w3229) -> (w3232:T1)
                n1487 = local write "Device(s)Settings"(w3232) -> ()
              }
              frame Default {
                # "Don't update any settings, they should all be set to 0 by default in all instrumenst and modes when the event \"Mode change\" occurs."
                # "In all other modes Instr1 is DC and \"Change at\" cannot generate a change event."
              }
            }
            n1488 = property on="btnSave" class="Bool"(error in=w3196, "DisabledEnum"=w3203) -> (error out=w3202:errorcluster)  [unwired: 1 in, 1 out]
            n1489 = property on="btnSaveAs" class="Bool"(error in=w3202, "DisabledEnum"=w3203) -> (error out=w3198:errorcluster)  [unwired: 1 in, 1 out]
          }
          event Value Change {
            w3245 = T15."Enabled" ("Disabled")
            w3246 = FALSE ("StartMeas")
            # "Voltage slew always matters.\nCurrent and Power only matter for DC slews.\nFrequency and Phase only matter for AC slews."
            # "No need to \"Update\" here because values are passed directly to Device(s)Settings in the case select structure."
            # "Since Instr1 may override Instr2 and Instr3 in some modes, and AC and DC don't have the same slews available to the user, evaluate what to do with Slew changes depending on Mode."
            n1490 = event-data() -> ()  [unwired: 1 in, 1 out]
            n1491 = local read "Instr1"() -> (w3242:T2)
            n1492 = Unbundle By Name(w3242) -> ("Slew Rates.Voltage (V/s)"=w3241:dbl, "Slew Rates.Current (A/s)"=w3238:dbl, "Slew Rates.Power (W/s)"=w3237:dbl, "Slew Rates.Frequency (Hz/s)"=w3240:dbl, "Slew Rates.Phase Angle (Deg/s)"=w3239:dbl)
            n1493 = local read "Mode"() -> (w3247:T8)
            n1494 = case shown="0, 1, Default" w3247 {
              tunnel: w3241 -> [w3252 w3258 w3264 w3270 w3276 w3282]
              tunnel: w3240 -> [w3251 w3256 w3262 _ w3274 w3281]
              tunnel: w3239 -> [w3250 _ w3263 _ w3275 _]
              tunnel: w3238 -> [_ w3257 _ w3269 _ w3280]
              tunnel: w3237 -> [_ _ _ w3268 _ _]
              tunnel: [w3249 w3255 w3261 w3267 w3273 w3279] -> w3235
              tunnel: w3236 -> [w3249 w3255 w3261 w3267 w3273 w3279]
              frame 0, 1, Default {
                # "Instr1 is AC and overrides Instr2 and Instr3"
                n1495 = local read "Device(s)Settings"() -> (w3254:T1)
                n1496 = Bundle By Name(cluster=w3254, "Instr1.Slew Rates.Voltage (V/s)"=w3252, "Instr2.Slew Rates.Voltage (V/s)"=w3252, "Instr3.Slew Rates.Voltage (V/s)"=w3252, "Instr1.Slew Rates.Frequency (Hz/s)"=w3251, "Instr2.Slew Rates.Frequency (Hz/s)"=w3251, "Instr3.Slew Rates.Frequency (Hz/s)"=w3251, "Instr1.Slew Rates.Phase Angle (Deg/s)"=w3250, "Instr2.Slew Rates.Phase Angle (Deg/s)"=w3250, "Instr3.Slew Rates.Phase Angle (Deg/s)"=w3250) -> (w3253:T1)
                n1497 = local write "Device(s)Settings"(w3253) -> ()
              }
              frame 2 {
                # "Instr1 is DC and overrides Instr2 and Instr3"
                n1498 = local read "Device(s)Settings"() -> (w3260:T1)
                n1499 = Bundle By Name(cluster=w3260, "Instr1.Slew Rates.Voltage (V/s)"=w3258, "Instr2.Slew Rates.Voltage (V/s)"=w3258, "Instr3.Slew Rates.Voltage (V/s)"=w3258, "Instr1.Slew Rates.Current (A/s)"=w3257, "Instr2.Slew Rates.Current (A/s)"=w3257, "Instr3.Slew Rates.Current (A/s)"=w3257, "Instr1.Slew Rates.Power (W/s)"=w3256, "Instr2.Slew Rates.Power (W/s)"=w3256, "Instr3.Slew Rates.Power (W/s)"=w3256) -> (w3259:T1)
                n1500 = local write "Device(s)Settings"(w3259) -> ()
              }
              frame 3, 9, 10, 13 {
                # "Instr1 is AC working as a single instrument"
                n1501 = local read "Device(s)Settings"() -> (w3266:T1)
                n1502 = Bundle By Name(cluster=w3266, "Instr1.Slew Rates.Voltage (V/s)"=w3264, "Instr1.Slew Rates.Frequency (Hz/s)"=w3262, "Instr1.Slew Rates.Phase Angle (Deg/s)"=w3263) -> (w3265:T1)
                n1503 = local write "Device(s)Settings"(w3265) -> ()
              }
              frame 4, 14, 15 {
                # "Instr1 is DC working as a single instrument"
                n1504 = local read "Device(s)Settings"() -> (w3272:T1)
                n1505 = Bundle By Name(cluster=w3272, "Instr1.Slew Rates.Voltage (V/s)"=w3270, "Instr1.Slew Rates.Current (A/s)"=w3269, "Instr1.Slew Rates.Power (W/s)"=w3268) -> (w3271:T1)
                n1506 = local write "Device(s)Settings"(w3271) -> ()
              }
              frame 5..8 {
                # "Instr1 is AC and overrides Instr2 only"
                n1507 = local read "Device(s)Settings"() -> (w3278:T1)
                n1508 = Bundle By Name(cluster=w3278, "Instr1.Slew Rates.Voltage (V/s)"=w3276, "Instr2.Slew Rates.Voltage (V/s)"=w3276, "Instr1.Slew Rates.Frequency (Hz/s)"=w3274, "Instr2.Slew Rates.Frequency (Hz/s)"=w3274, "Instr1.Slew Rates.Phase Angle (Deg/s)"=w3275, "Instr2.Slew Rates.Phase Angle (Deg/s)"=w3275) -> (w3277:T1)
                n1509 = local write "Device(s)Settings"(w3277) -> ()
              }
              frame 11, 12 {
                # "Instr1 is DC and overrides Instr2 only"
                n1510 = local read "Device(s)Settings"() -> (w3284:T1)
                n1511 = Bundle By Name(cluster=w3284, "Instr1.Slew Rates.Voltage (V/s)"=w3282, "Instr2.Slew Rates.Voltage (V/s)"=w3282, "Instr1.Slew Rates.Current (A/s)"=w3280, "Instr2.Slew Rates.Current (A/s)"=w3280, "Instr1.Slew Rates.Power (W/s)"=w3281, "Instr2.Slew Rates.Power (W/s)"=w3281) -> (w3283:T1)
                n1512 = local write "Device(s)Settings"(w3283) -> ()
              }
            }
            n1513 = property on="btnSave" class="Bool"(error in=w3235, "DisabledEnum"=w3245) -> (error out=w3244:errorcluster)  [unwired: 1 in, 1 out]
            n1514 = property on="btnSaveAs" class="Bool"(error in=w3244, "DisabledEnum"=w3245) -> (error out=w3243:errorcluster)  [unwired: 1 in, 1 out]
          }
          event Value Change {
            w3295 = T15."Enabled" ("Disabled")
            w3296 = FALSE ("StartMeas")
            # "Voltage slew always matters.\nCurrent and Power only matter for DC slews.\nFrequency and Phase only matter for AC slews."
            # "No need to \"Update\" here because values are passed directly to Device(s)Settings in the case select structure."
            # "Instr2 can be configured by the user as  a single instrument only in some modes, and AC and DC don't have the same slews available to the user, evaluate what to do with Slew changes depending on Mode."
            n1515 = event-data() -> ()  [unwired: 1 in, 1 out]
            n1516 = local read "Instr2"() -> (w3292:T2)
            n1517 = Unbundle By Name(w3292) -> ("Slew Rates.Voltage (V/s)"=w3291:dbl, "Slew Rates.Current (A/s)"=w3288:dbl, "Slew Rates.Power (W/s)"=w3287:dbl, "Slew Rates.Frequency (Hz/s)"=w3290:dbl, "Slew Rates.Phase Angle (Deg/s)"=w3289:dbl)
            n1518 = local read "Mode"() -> (w3297:T8)
            n1519 = case shown="3, 9, 15, Default" w3297 {
              tunnel: w3291 -> [w3302 w3308]
              tunnel: w3290 -> [w3300 _]
              tunnel: w3289 -> [w3301 _]
              tunnel: w3288 -> [_ w3307]
              tunnel: w3287 -> [_ w3306]
              tunnel: [w3299 w3305] -> w3285
              tunnel: w3286 -> [w3299 w3305]
              frame 3, 9, 15, Default {
                # "Instr2 is AC working as a single instrument"
                n1520 = local read "Device(s)Settings"() -> (w3304:T1)
                n1521 = Bundle By Name(cluster=w3304, "Instr2.Slew Rates.Voltage (V/s)"=w3302, "Instr2.Slew Rates.Frequency (Hz/s)"=w3300, "Instr2.Slew Rates.Phase Angle (Deg/s)"=w3301) -> (w3303:T1)
                n1522 = local write "Device(s)Settings"(w3303) -> ()
              }
              frame 4, 10, 13 {
                # "Instr2 is DC working as a single instrument"
                n1523 = local read "Device(s)Settings"() -> (w3310:T1)
                n1524 = Bundle By Name(cluster=w3310, "Instr2.Slew Rates.Voltage (V/s)"=w3308, "Instr2.Slew Rates.Current (A/s)"=w3307, "Instr2.Slew Rates.Power (W/s)"=w3306) -> (w3309:T1)
                n1525 = local write "Device(s)Settings"(w3309) -> ()
              }
            }
            n1526 = property on="btnSave" class="Bool"(error in=w3285, "DisabledEnum"=w3295) -> (error out=w3294:errorcluster)  [unwired: 1 in, 1 out]
            n1527 = property on="btnSaveAs" class="Bool"(error in=w3294, "DisabledEnum"=w3295) -> (error out=w3293:errorcluster)  [unwired: 1 in, 1 out]
          }
          event Value Change {
            w3321 = T15."Enabled" ("Disabled")
            w3322 = FALSE ("StartMeas")
            # "Voltage slew always matters.\nCurrent and Power only matter for DC slews.\nFrequency and Phase only matter for AC slews."
            # "No need to \"Update\" here because values are passed directly to Device(s)Settings in the case select structure."
            # "Instr3 can be configured by the user as  a single instrument only in some modes, and AC and DC don't have the same slews available to the user, evaluate what to do with Slew changes depending on Mode."
            n1528 = event-data() -> ()  [unwired: 1 in, 1 out]
            n1529 = local read "Instr3"() -> (w3318:T2)
            n1530 = Unbundle By Name(w3318) -> ("Slew Rates.Voltage (V/s)"=w3317:dbl, "Slew Rates.Current (A/s)"=w3314:dbl, "Slew Rates.Power (W/s)"=w3313:dbl, "Slew Rates.Frequency (Hz/s)"=w3316:dbl, "Slew Rates.Phase Angle (Deg/s)"=w3315:dbl)
            n1531 = local read "Mode"() -> (w3323:T8)
            n1532 = case shown="4, 6, 8..10, 12, 15" w3323 {
              tunnel: w3317 -> [w3328 w3334]
              tunnel: w3316 -> [w3326 _]
              tunnel: w3315 -> [w3327 _]
              tunnel: w3314 -> [_ w3333]
              tunnel: w3313 -> [_ w3332]
              tunnel: [w3325 w3331] -> w3311
              tunnel: w3312 -> [w3325 w3331]
              frame 3, 5, 7, 11, 13, 14, Default {
                # "Instr3 is AC working as a single instrument"
                n1533 = local read "Device(s)Settings"() -> (w3330:T1)
                n1534 = Bundle By Name(cluster=w3330, "Instr3.Slew Rates.Voltage (V/s)"=w3328, "Instr3.Slew Rates.Frequency (Hz/s)"=w3326, "Instr3.Slew Rates.Phase Angle (Deg/s)"=w3327) -> (w3329:T1)
                n1535 = local write "Device(s)Settings"(w3329) -> ()
              }
              frame 4, 6, 8..10, 12, 15 {
                # "Instr3 is DC working as a single instrument"
                n1536 = local read "Device(s)Settings"() -> (w3336:T1)
                n1537 = Bundle By Name(cluster=w3336, "Instr3.Slew Rates.Voltage (V/s)"=w3334, "Instr3.Slew Rates.Current (A/s)"=w3333, "Instr3.Slew Rates.Power (W/s)"=w3332) -> (w3335:T1)
                n1538 = local write "Device(s)Settings"(w3335) -> ()
              }
            }
            n1539 = property on="btnSave" class="Bool"(error in=w3311, "DisabledEnum"=w3321) -> (error out=w3320:errorcluster)  [unwired: 1 in, 1 out]
            n1540 = property on="btnSaveAs" class="Bool"(error in=w3320, "DisabledEnum"=w3321) -> (error out=w3319:errorcluster)  [unwired: 1 in, 1 out]
          }
          event Value Change {
            w3343 = T15."Enabled" ("Disabled")
            w3344 = FALSE ("StartMeas")
            # "No need to \"Update\" here because values are passed directly to Device(s)Settings in the case select structure."
            # "Get all the present \"Change at\" values in Instr2"
            # "Instr2 it's only available as a stand-alone instrument in very few modes, and can only be a single channel instrument, so the call will only affect \"Change at\" A."
            n1541 = event-data() -> ()  [unwired: 1 in, 3 out]
            n1542 = local read "Instr2"() -> (w3338:T2)
            n1543 = Unbundle By Name(w3338) -> ("Phases.A-Change at..."=w3341:i32)
            n1544 = local read "Mode"() -> (w3345:T8)
            n1545 = case shown="3, 9, 14, 15" w3345 {
              tunnel: [w3348 w3351] -> w3337
              tunnel: w3341 -> [_ _]
              tunnel: w3340 -> [w3348 w3351]
              frame 3, 9, 14, 15 {
                w3347 = 0 ("Instr1.Phases.C-Change at...")
                # "The only modes when Instr2 is an avilable single one-phase AC instrument."
                n1546 = local read "Device(s)Settings"() -> (w3350:T1)
                n1547 = Bundle By Name(cluster=w3350, "Instr2.Phases.A-Change at..."=w3347, "Instr2.Phases.B-Change at..."=w3347, "Instr2.Phases.C-Change at..."=w3347) -> (w3349:T1)
                n1548 = local write "Device(s)Settings"(w3349) -> ()
              }
              frame Default {
                # "Don't update any settings, they should all be set to 0 by default in all instrumenst and modes when the event \"Mode change\" occurs."
                # "Instr2 is either DC or doesn't exist as a separate instrument."
              }
            }
            n1549 = property on="btnSave" class="Bool"(error in=w3337, "DisabledEnum"=w3343) -> (error out=w3342:errorcluster)  [unwired: 1 in, 1 out]
            n1550 = property on="btnSaveAs" class="Bool"(error in=w3342, "DisabledEnum"=w3343) -> (error out=w3339:errorcluster)  [unwired: 1 in, 1 out]
          }
          event Value Change {
            w3358 = T15."Enabled" ("Disabled")
            w3359 = FALSE ("StartMeas")
            # "No need to \"Update\" here because values are passed directly to Device(s)Settings in the case select structure."
            # "Get all the present \"Change at\" values in Instr3"
            # "Instr3 it's only available as a stand-alone instrument in some modes, and can only be a single channel instrument, so the call will only affect \"Change at\" A."
            n1551 = event-data() -> ()  [unwired: 1 in, 3 out]
            n1552 = local read "Instr3"() -> (w3353:T2)
            n1553 = Unbundle By Name(w3353) -> ("Phases.A-Change at..."=w3356:i32)
            n1554 = local read "Mode"() -> (w3360:T8)
            n1555 = case shown="3, 5, 7, 11, 13, 14" w3360 {
              tunnel: [w3364 w3367] -> w3352
              tunnel: w3356 -> [w3362 _]
              tunnel: w3355 -> [w3364 w3367]
              frame 3, 5, 7, 11, 13, 14 {
                w3363 = 0 ("Instr1.Phases.C-Change at...")
                # "Instr1 is a single one-phase AC instrument."
                n1556 = local read "Device(s)Settings"() -> (w3366:T1)
                n1557 = Bundle By Name(cluster=w3366, "Instr3.Phases.A-Change at..."=w3362, "Instr3.Phases.B-Change at..."=w3363, "Instr3.Phases.C-Change at..."=w3363) -> (w3365:T1)
                n1558 = local write "Device(s)Settings"(w3365) -> ()
              }
              frame Default {
                # "Don't update any settings, they should all be set to 0 by default in all instrumenst and modes when the event \"Mode change\" occurs."
                # "In all other modes Instr3 is DC and \"Change at\" cannot generate a change event."
              }
            }
            n1559 = property on="btnSave" class="Bool"(error in=w3352, "DisabledEnum"=w3358) -> (error out=w3357:errorcluster)  [unwired: 1 in, 1 out]
            n1560 = property on="btnSaveAs" class="Bool"(error in=w3357, "DisabledEnum"=w3358) -> (error out=w3354:errorcluster)  [unwired: 1 in, 1 out]
          }
          event Value Change {
            w3383 = T15."Enabled" ("Disabled")
            w3384 = FALSE ("StartMeas")
            # "Turn string to numeric."
            # "Check if the V range selection requires adjustments in the instrument(s) voltages."
            # "Instr1"
            # "Instr1 can override Instr2 and Instr3, and it can also have phases settings. Make voltages adjustments if needed depending on Mode."
            n1561 = event-data() -> ()  [unwired: 1 in, 1 out]
            n1562 = property on="Voltage (V)" class="Ring (strict)"(error in=w3372) -> (error out=w3378:errorcluster, "Strings []"=w3380:string[], "Value"=w3371:u16)  [unwired: 1 in, 1 out]
            n1563 = local read "Instr1"() -> (w3379:T2)
            n1564 = Index Array(array=w3380, index=w3371) -> (element=w3377:string)
            n1565 = Unbundle By Name(w3379) -> ("Vout (V)"=w3368:dbl)
            n1566 = Scan From String(format string="%f", input string=w3377, error in=w3378) -> (error out=w3370:errorcluster, output 1=w3381:dbl)  [unwired: 2 in, 2 out]
            n1567 = Less?(x=w3381, y=w3368) -> (x < y?=w3374:bool)
            n1568 = local read "Mode"() -> (w3373:T8)
            n1569 = case shown="False" w3374 {
              tunnel: w3381 -> [_ w3404]
              tunnel: w3373 -> [w3387 w3407]
              tunnel: w3371 -> [w3389 w3408]
              tunnel: [w3388 w3402] -> w3369
              tunnel: w3370 -> [w3388 w3402]
              tunnel: w3368 -> [w3386 _]
              frame False {
                # "Do nothing to adjust voltages, the value of Vout is inside the new range. Just update Device(s)Settings."
                n1570 = case shown="0..2, Default" w3387 {
                  tunnel: w3389 -> [w3391 w3395 w3399]
                  tunnel: w3386 -> [w3390 w3394 w3398]
                  frame 0..2, Default {
                    # "Instr1 overrides Instr2 and Instr3"
                    n1571 = local read "Device(s)Settings"() -> (w3392:T1)
                    n1572 = Bundle By Name(cluster=w3392, "Instr1.Vout (V)"=w3390, "Instr2.Vout (V)"=w3390, "Instr3.Vout (V)"=w3390, "Instr1.Ranges.Voltage (V)"=w3391, "Instr2.Ranges.Voltage (V)"=w3391, "Instr3.Ranges.Voltage (V)"=w3391) -> (w3393:T1)
                    n1573 = local write "Device(s)Settings"(w3393) -> ()
                  }
                  frame 3, 4, 9, 10, 13..15 {
                    # "Instr1 is a single instrument"
                    n1574 = local read "Device(s)Settings"() -> (w3397:T1)
                    n1575 = Bundle By Name(cluster=w3397, "Instr1.Vout (V)"=w3394, "Instr1.Ranges.Voltage (V)"=w3395) -> (w3396:T1)
                    n1576 = local write "Device(s)Settings"(w3396) -> ()
                  }
                  frame 5..8, 11, 12 {
                    # "Instr1 overrides Instr2 only"
                    n1577 = local read "Device(s)Settings"() -> (w3400:T1)
                    n1578 = Bundle By Name(cluster=w3400, "Instr1.Vout (V)"=w3398, "Instr2.Vout (V)"=w3398, "Instr1.Ranges.Voltage (V)"=w3399, "Instr2.Ranges.Voltage (V)"=w3399) -> (w3401:T1)
                    n1579 = local write "Device(s)Settings"(w3401) -> ()
                  }
                }
              }
              frame True {
                # "Since Vout was larger than the new range choice, by default Vout will be set to be the full new range limit to keep it as close as possible to the previous Vout level."
                # "If the new range is lower than Vout, then Vout needs to be lowered to fit inside the new range. Depending on the Mode, the phase voltages may need some adjustments to follow the Vout change too."
                n1580 = case shown="0" w3407 {
                  tunnel: w3404 -> [w3433 w3436 w3440 w3441 w3444]
                  tunnel: [w3432 w3436 w3438 w3441 w3444] -> w3406
                  tunnel: [w3432 w3436 w3438 w3441 w3443] -> w3405
                  tunnel: [w3432 w3436 0.0 ("NewVal") 0.0 ("NewVal") w3443] -> w3403
                  frame 0 {
                    # "The three phase values are equal for (L-N)"
                    n1581 = Square Root(x=3.0) -> (sqrt(x)=w3434:dbl)
                    n1582 = Divide(x=w3433, y=w3434) -> (x/y=w3432:dbl)
                  }
                  frame 1, 2 {
                    # "All three channels joined as a single output"
                  }
                  frame 5, 6 {
                    # "Two channels joined as a split phase output"
                    n1583 = Divide(x=w3440, y=2.0) -> (x/y=w3438:dbl)
                  }
                  frame 7, 8, 11, 12 {
                    # "Two channels joined as a single output"
                  }
                  frame Default {
                    w3443 = 0.0 ("NewVal")
                    # "The instrument uses only one phase/channel"
                  }
                }
                n1584 = local read "Instr1"() -> (w3409:T2)
                n1585 = Bundle By Name(cluster=w3409, "Phases.A-Volts (V)"=w3406, "Phases.B-Volts (V)"=w3405, "Phases.C-Volts (V)"=w3403, "Vout (V)"=w3404) -> (w3410:T2)
                n1586 = local write "Instr1"(w3410) -> ()
                n1587 = case shown="0..2, Default" w3407 {
                  tunnel: w3408 -> [w3415 w3418 w3425]
                  tunnel: w3406 -> [w3414 w3422 w3429]
                  tunnel: w3405 -> [w3413 w3421 w3428]
                  tunnel: w3403 -> [w3411 w3420 w3427]
                  tunnel: w3404 -> [w3412 w3419 w3426]
                  frame 0..2, Default {
                    # "Instr1 overrides Instr2 and Instr3"
                    n1588 = local read "Device(s)Settings"() -> (w3416:T1)
                    n1589 = Bundle By Name(cluster=w3416, "Instr1.Phases.A-Volts (V)"=w3414, "Instr2.Phases.A-Volts (V)"=w3414, "Instr3.Phases.A-Volts (V)"=w3414, "Instr1.Phases.B-Volts (V)"=w3413, "Instr2.Phases.B-Volts (V)"=w3413, "Instr3.Phases.B-Volts (V)"=w3413, "Instr1.Phases.C-Volts (V)"=w3411, "Instr2.Phases.C-Volts (V)"=w3411, "Instr3.Phases.C-Volts (V)"=w3411, "Instr1.Vout (V)"=w3412, "Instr2.Vout (V)"=w3412, "Instr3.Vout (V)"=w3412, "Instr1.Ranges.Voltage (V)"=w3415, "Instr2.Ranges.Voltage (V)"=w3415, "Instr3.Ranges.Voltage (V)"=w3415) -> (w3417:T1)
                    n1590 = local write "Device(s)Settings"(w3417) -> ()
                  }
                  frame 3, 4, 9, 10, 13..15 {
                    # "Instr1 is a single instrument"
                    n1591 = local read "Device(s)Settings"() -> (w3424:T1)
                    n1592 = Bundle By Name(cluster=w3424, "Instr1.Phases.A-Volts (V)"=w3422, "Instr1.Phases.B-Volts (V)"=w3421, "Instr1.Phases.C-Volts (V)"=w3420, "Instr1.Vout (V)"=w3419, "Instr1.Ranges.Voltage (V)"=w3418) -> (w3423:T1)
                    n1593 = local write "Device(s)Settings"(w3423) -> ()
                  }
                  frame 5..8, 11, 12 {
                    # "Instr1 overrides Instr2 only"
                    n1594 = local read "Device(s)Settings"() -> (w3430:T1)
                    n1595 = Bundle By Name(cluster=w3430, "Instr1.Phases.A-Volts (V)"=w3429, "Instr2.Phases.A-Volts (V)"=w3429, "Instr1.Phases.B-Volts (V)"=w3428, "Instr2.Phases.B-Volts (V)"=w3428, "Instr1.Phases.C-Volts (V)"=w3427, "Instr2.Phases.C-Volts (V)"=w3427, "Instr1.Vout (V)"=w3426, "Instr2.Vout (V)"=w3426, "Instr1.Ranges.Voltage (V)"=w3425, "Instr2.Ranges.Voltage (V)"=w3425) -> (w3431:T1)
                    n1596 = local write "Device(s)Settings"(w3431) -> ()
                  }
                }
              }
            }
            n1597 = property on="btnSaveAs" class="Bool"(error in=w3369, "DisabledEnum"=w3383) -> (error out=w3376:errorcluster)  [unwired: 1 in, 1 out]
            n1598 = property on="btnSave" class="Bool"(error in=w3376, "DisabledEnum"=w3383) -> (error out=w3375:errorcluster)  [unwired: 1 in, 1 out]
          }
          event Value Change {
            w3459 = T15."Enabled" ("Disabled")
            w3460 = FALSE ("StartMeas")
            # "No need to \"Update\" because Device(s)Settings were already set inside the case structure."
            # "Turn string to numeric."
            # "Check if the V range selection requires adjustments in the instrument voltage."
            # "Instr2"
            # "Instr2 can only exist as a single phase/channel affecting only itself. So, in which Mode, is irrelevant. Only its own settings need to be adjusted."
            n1599 = event-data() -> ()  [unwired: 1 in, 1 out]
            n1600 = property on="Voltage (V)" class="Ring (strict)"(error in=w3449) -> (error out=w3454:errorcluster, "Strings []"=w3456:string[], "Value"=w3448:u16)  [unwired: 1 in, 1 out]
            n1601 = Index Array(array=w3456, index=w3448) -> (element=w3453:string)
            n1602 = local read "Instr2"() -> (w3455:T2)
            n1603 = Unbundle By Name(w3455) -> ("Vout (V)"=w3445:dbl)
            n1604 = Scan From String(format string="%f", input string=w3453, error in=w3454) -> (error out=w3447:errorcluster, output 1=w3457:dbl)  [unwired: 2 in, 2 out]
            n1605 = Less?(x=w3457, y=w3445) -> (x < y?=w3450:bool)
            n1606 = case shown="True" w3450 {
              tunnel: w3457 -> [_ w3468]
              tunnel: w3448 -> [w3466 w3467]
              tunnel: [w3465 w3471] -> w3446
              tunnel: w3447 -> [w3465 w3471]
              tunnel: w3445 -> [w3462 _]
              frame False {
                # "Do nothing to adjust Vout because it's still inside the new range. Just update Device(s)Settings."
                n1607 = local read "Device(s)Settings"() -> (w3464:T1)
                n1608 = Bundle By Name(cluster=w3464, "Instr2.Vout (V)"=w3462, "Instr2.Ranges.Voltage (V)"=w3466) -> (w3463:T1)
                n1609 = local write "Device(s)Settings"(w3463) -> ()
              }
              frame True {
                # "Since Vout was larger than the new range choice, by default Vout will be set to be the full new range limit to keep it as close as possible to the previous Vout level."
                # "If the new range is lower than Vout, then Vout needs to be lowered to fit inside the new range."
                n1610 = local read "Device(s)Settings"() -> (w3470:T1)
                n1611 = Bundle By Name(cluster=w3470, "Instr2.Vout (V)"=w3468, "Instr2.Ranges.Voltage (V)"=w3467) -> (w3469:T1)
                n1612 = local read "Instr2"() -> (w3472:T2)
                n1613 = Bundle By Name(cluster=w3472, "Vout (V)"=w3468) -> (w3473:T2)
                n1614 = local write "Instr2"(w3473) -> ()
                n1615 = local write "Device(s)Settings"(w3469) -> ()
              }
            }
            n1616 = property on="btnSaveAs" class="Bool"(error in=w3446, "DisabledEnum"=w3459) -> (error out=w3452:errorcluster)  [unwired: 1 in, 1 out]
            n1617 = property on="btnSave" class="Bool"(error in=w3452, "DisabledEnum"=w3459) -> (error out=w3451:errorcluster)  [unwired: 1 in, 1 out]
          }
          event Value Change {
            w3488 = T15."Enabled" ("Disabled")
            w3489 = FALSE ("StartMeas")
            # "No need to \"Update\" because Device(s)Settings were already set inside the case structure."
            # "Turn string to numeric."
            # "Check if the V range selection requires adjustments in the instrument voltage."
            # "Instr3"
            # "Instr3 can only exist as a single phase/channel affecting only itself. So, in which Mode, is irrelevant. Only its own settings need to be adjusted."
            n1618 = event-data() -> ()  [unwired: 1 in, 1 out]
            n1619 = property on="Voltage (V)" class="Ring (strict)"(error in=w3478) -> (error out=w3483:errorcluster, "Strings []"=w3485:string[], "Value"=w3477:u16)  [unwired: 1 in, 1 out]
            n1620 = Index Array(array=w3485, index=w3477) -> (element=w3482:string)
            n1621 = local read "Instr3"() -> (w3484:T2)
            n1622 = Unbundle By Name(w3484) -> ("Vout (V)"=w3474:dbl)
            n1623 = Scan From String(format string="%f", input string=w3482, error in=w3483) -> (error out=w3476:errorcluster, output 1=w3486:dbl)  [unwired: 2 in, 2 out]
            n1624 = Less?(x=w3486, y=w3474) -> (x < y?=w3479:bool)
            n1625 = case shown="False" w3479 {
              tunnel: w3486 -> [_ w3497]
              tunnel: w3477 -> [w3495 w3496]
              tunnel: [w3494 w3500] -> w3475
              tunnel: w3476 -> [w3494 w3500]
              tunnel: w3474 -> [w3491 _]
              frame False {
                # "Do nothing to adjust Vout because it's still inside the new range. Just update Device(s)Settings."
                n1626 = local read "Device(s)Settings"() -> (w3493:T1)
                n1627 = Bundle By Name(cluster=w3493, "Instr3.Vout (V)"=w3491, "Instr3.Ranges.Voltage (V)"=w3495) -> (w3492:T1)
                n1628 = local write "Device(s)Settings"(w3492) -> ()
              }
              frame True {
                # "Since Vout was larger than the new range choice, by default Vout will be set to be the full new range limit to keep it as close as possible to the previous Vout level."
                # "If the new range is lower than Vout, then Vout needs to be lowered to fit inside the new range."
                n1629 = local read "Device(s)Settings"() -> (w3499:T1)
                n1630 = Bundle By Name(cluster=w3499, "Instr3.Vout (V)"=w3497, "Instr3.Ranges.Voltage (V)"=w3496) -> (w3498:T1)
                n1631 = local read "Instr3"() -> (w3501:T2)
                n1632 = Bundle By Name(cluster=w3501, "Vout (V)"=w3497) -> (w3502:T2)
                n1633 = local write "Instr3"(w3502) -> ()
                n1634 = local write "Device(s)Settings"(w3498) -> ()
              }
            }
            n1635 = property on="btnSaveAs" class="Bool"(error in=w3475, "DisabledEnum"=w3488) -> (error out=w3481:errorcluster)  [unwired: 1 in, 1 out]
            n1636 = property on="btnSave" class="Bool"(error in=w3481, "DisabledEnum"=w3488) -> (error out=w3480:errorcluster)  [unwired: 1 in, 1 out]
          }
          event Value Change {
            w3510 = T15."Enabled" ("Disabled")
            w3511 = FALSE ("StartMeas")
            # "Since the current range in the device is dependent on the number of chassis presently turned on in the grid emulator, there's a possibility that the range limits that could have been saved in a recently-loaded configuration file do not match the present state of the grid emulator. To ensure that the present current range limits are correct in case that the user wants to save the present configuration, the list of options that the current range controls show need to be updated to the actual number of chassis turned on in the emulator. Then those values can be passed to Device(s)Settings to be saved."
            # "Update Device(s)Settings"
            # "If any current range control is changed in any instrument, update the list of options that the controls show."
            n1637 = event-data() -> ()  [unwired: 1 in, 6 out]
            n1638 = flat-sequence {
              tunnel: w3505 -> [w3520]
              tunnel: [w3513] -> w3504
              frame #0 {
                # "2"
                # "1"
                # "3"
                # "Refresh the 'Strings[]' array property for the current range control of each instrument."
                # "Instr3"
                # "Instr2"
                # "Instr1"
                # "The frame is to make sure that all data has been updated in the instruments controls before passing the values to the Device(s)Settings cluster."
                n1639 = local read "Chassis"() -> (w3525:i32)
                n1640 = local read "Mode"() -> (w3526:T8)
                n1641 = Multiply(x=w3525, y=6) -> (x*y=w3522:i32)
                n1642 = Multiply(x=30, y=w3525) -> (x*y=w3521:i32)
                n1643 = case shown="Default" w3526 {
                  tunnel: w3522 -> [w3535 w3540 w3554]
                  tunnel: w3521 -> [w3532 w3537 w3553]
                  tunnel: [w3529 w3543 w3550] -> w3519
                  tunnel: [w3528 w3542 w3552] -> w3518
                  tunnel: [w3528 w3542 w3552] -> w3516
                  tunnel: [w3528 w3542 w3551] -> w3514
                  tunnel: w3520 -> [w3527 w3536 w3548]
                  frame Default {
                    w3533 = "%d" ("format string")
                    # "All other modes have the same current range limits regardless of instrument configuration."
                    n1644 = Format Into String(format string=w3533, error in=w3527, w3535) -> (resulting string=w3531:string, error out=w3534:errorcluster)  [unwired: 1 in]
                    n1645 = Format Into String(format string=w3533, error in=w3534, w3532) -> (resulting string=w3530:string, error out=w3529:errorcluster)  [unwired: 1 in]
                    n1646 = Build Array(w3531, w3530) -> (w3528:string[])
                  }
                  frame 1, 2 {
                    w3538 = 3 ("y")
                    w3546 = "%d" ("format string")
                    # "Three single AC or three single DC instruments"
                    n1647 = Multiply(x=w3540, y=w3538) -> (x*y=w3541:i32)
                    n1648 = Multiply(x=w3538, y=w3537) -> (x*y=w3539:i32)
                    n1649 = Format Into String(format string=w3546, error in=w3536, w3541) -> (resulting string=w3545:string, error out=w3547:errorcluster)  [unwired: 1 in]
                    n1650 = Format Into String(format string=w3546, error in=w3547, w3539) -> (resulting string=w3544:string, error out=w3543:errorcluster)  [unwired: 1 in]
                    n1651 = Build Array(w3545, w3544) -> (w3542:string[])
                  }
                  frame 7, 8, 11, 12 {
                    w3555 = "%d" ("format string")
                    w3559 = 2 ("y")
                    # "One double AC or DC, and a third singe AC or DC"
                    n1652 = Format Into String(format string=w3555, error in=w3548, w3554) -> (resulting string=w3557:string, error out=w3558:errorcluster)  [unwired: 1 in]
                    n1653 = Format Into String(format string=w3555, error in=w3558, w3553) -> (resulting string=w3556:string, error out=w3549:errorcluster)  [unwired: 1 in]
                    n1654 = Multiply(x=w3554, y=w3559) -> (x*y=w3561:i32)
                    n1655 = Multiply(x=w3559, y=w3553) -> (x*y=w3560:i32)
                    n1656 = Build Array(w3557, w3556) -> (w3551:string[])
                    n1657 = Format Into String(format string=w3555, error in=w3549, w3561) -> (resulting string=w3563:string, error out=w3564:errorcluster)  [unwired: 1 in]
                    n1658 = Format Into String(format string=w3555, error in=w3564, w3560) -> (resulting string=w3562:string, error out=w3550:errorcluster)  [unwired: 1 in]
                    n1659 = Build Array(w3563, w3562) -> (w3552:string[])
                  }
                }
                n1660 = property on="Current (A)" class="Ring (strict)"(error in=w3519, "Strings []"=w3518) -> (error out=w3517:errorcluster)  [unwired: 1 in, 1 out]
                n1661 = property on="Current (A)" class="Ring (strict)"(error in=w3517, "Strings []"=w3516) -> (error out=w3515:errorcluster)  [unwired: 1 in, 1 out]
                n1662 = property on="Current (A)" class="Ring (strict)"(error in=w3515, "Strings []"=w3514) -> (error out=w3513:errorcluster)  [unwired: 1 in, 1 out]
              }
            }
            n1663 = property on="Update" class="Bool (strict)"(error in=w3504) -> (error out=w3509:errorcluster, "Value"=w3503:bool)  [unwired: 1 in, 1 out]
            n1664 = property on="Update" class="Bool (strict)"(error in=w3509, "Val(Sgnl)"=w3503) -> (error out=w3506:errorcluster)  [unwired: 1 in, 1 out]
            n1665 = property on="btnSaveAs" class="Bool"(error in=w3506, "DisabledEnum"=w3510) -> (error out=w3507:errorcluster)  [unwired: 1 in, 1 out]
            n1666 = property on="btnSave" class="Bool"(error in=w3507, "DisabledEnum"=w3510) -> (error out=w3508:errorcluster)  [unwired: 1 in, 1 out]
          }
          event Value Change {
            w3573 = T15."Enabled" ("Disabled")
            w3574 = FALSE ("StartMeas")
            # "Wave Shapes are only enabled when the instrument is AC. That has been taken care in the \"WaveEnable\" case of the \"Mode Change\" event."
            # "No need to \"Update\" here because values are passed directly to Device(s)Settings in the case select structure."
            # "Since Instr1 exists in all modes and it may override Instr2 and Instr3 in some of them, evaluate what to do with Wave Shape changes depending on Mode."
            n1667 = event-data() -> ()  [unwired: 1 in, 6 out]
            n1668 = local read "Instr1"() -> (w3570:T2)
            n1669 = Unbundle By Name(w3570) -> ("Phases.A-Wave Shape"=w3569:u16, "Phases.B-Wave Shape"=w3568:u16, "Phases.C-Wave Shape"=w3565:u16)
            n1670 = local read "Mode"() -> (w3575:T8)
            n1671 = case shown="3, 4, 9, 10, 13..15" w3575 {
              tunnel: w3569 -> [w3580 w3586 w3592]
              tunnel: w3568 -> [w3578 w3584 w3590]
              tunnel: [w3579 w3585 w3591] -> w3566
              tunnel: w3567 -> [w3579 w3585 w3591]
              tunnel: [w3577 w3583 w3589] -> _
              tunnel: w3565 -> [w3577 w3583 w3589]
              frame 0..2, Default {
                # "Instr1 overrides Instr2 and Instr3"
                n1672 = local read "Device(s)Settings"() -> (w3582:T1)
                n1673 = Bundle By Name(cluster=w3582, "Instr1.Phases.A-Wave Shape"=w3580, "Instr2.Phases.A-Wave Shape"=w3580, "Instr3.Phases.A-Wave Shape"=w3580, "Instr1.Phases.B-Wave Shape"=w3578, "Instr2.Phases.B-Wave Shape"=w3578, "Instr3.Phases.B-Wave Shape"=w3578, "Instr1.Phases.C-Wave Shape"=w3577, "Instr2.Phases.C-Wave Shape"=w3577, "Instr3.Phases.C-Wave Shape"=w3577) -> (w3581:T1)
                n1674 = local write "Device(s)Settings"(w3581) -> ()
              }
              frame 5..8, 11, 12 {
                # "Instr1 overrides Instr2 only"
                n1675 = local read "Device(s)Settings"() -> (w3588:T1)
                n1676 = Bundle By Name(cluster=w3588, "Instr1.Phases.A-Wave Shape"=w3586, "Instr2.Phases.A-Wave Shape"=w3586, "Instr1.Phases.B-Wave Shape"=w3584, "Instr2.Phases.B-Wave Shape"=w3584, "Instr1.Phases.C-Wave Shape"=w3583, "Instr2.Phases.C-Wave Shape"=w3583) -> (w3587:T1)
                n1677 = local write "Device(s)Settings"(w3587) -> ()
              }
              frame 3, 4, 9, 10, 13..15 {
                # "Instr1 is a single instrument by itself"
                n1678 = local read "Device(s)Settings"() -> (w3594:T1)
                n1679 = Bundle By Name(cluster=w3594, "Instr1.Phases.A-Wave Shape"=w3592, "Instr1.Phases.B-Wave Shape"=w3590, "Instr1.Phases.C-Wave Shape"=w3589) -> (w3593:T1)
                n1680 = local write "Device(s)Settings"(w3593) -> ()
              }
            }
            n1681 = property on="btnSave" class="Bool"(error in=w3566, "DisabledEnum"=w3573) -> (error out=w3572:errorcluster)  [unwired: 1 in, 1 out]
            n1682 = property on="btnSaveAs" class="Bool"(error in=w3572, "DisabledEnum"=w3573) -> (error out=w3571:errorcluster)  [unwired: 1 in, 1 out]
          }
          event Value Change {
            w3603 = T15."Enabled" ("Disabled")
            w3604 = FALSE ("StartMeas")
            # "Wave Shapes are only enabled when the instrument is AC. That has been taken care in the \"WaveEnable\" case of the \"Mode Change\" event."
            # "No need to \"Update\" here because values are passed directly to Device(s)Settings in the case select structure."
            # "Instr2 can only exist as itself in a few modes to be able to change its Wave Shapes."
            n1683 = event-data() -> ()  [unwired: 1 in, 6 out]
            n1684 = local read "Instr2"() -> (w3600:T2)
            n1685 = Unbundle By Name(w3600) -> ("Phases.A-Wave Shape"=w3599:u16, "Phases.B-Wave Shape"=w3598:u16, "Phases.C-Wave Shape"=w3595:u16)
            n1686 = local read "Mode"() -> (w3605:T8)
            n1687 = case shown="3, 4, 9, 10, 13..15" w3605 {
              tunnel: w3599 -> [_ w3612]
              tunnel: w3598 -> [_ w3610]
              tunnel: [w3608 w3611] -> w3596
              tunnel: w3597 -> [w3608 w3611]
              tunnel: [w3607 w3609] -> _
              tunnel: w3595 -> [w3607 w3609]
              frame Default {
                # "Instr2 is unavailable in the other modes."
              }
              frame 3, 4, 9, 10, 13..15 {
                # "Modes in which Instr2 can be accessed by the user as a single instrument."
                n1688 = local read "Device(s)Settings"() -> (w3614:T1)
                n1689 = Bundle By Name(cluster=w3614, "Instr2.Phases.A-Wave Shape"=w3612, "Instr2.Phases.B-Wave Shape"=w3610, "Instr2.Phases.C-Wave Shape"=w3609) -> (w3613:T1)
                n1690 = local write "Device(s)Settings"(w3613) -> ()
              }
            }
            n1691 = property on="btnSave" class="Bool"(error in=w3596, "DisabledEnum"=w3603) -> (error out=w3602:errorcluster)  [unwired: 1 in, 1 out]
            n1692 = property on="btnSaveAs" class="Bool"(error in=w3602, "DisabledEnum"=w3603) -> (error out=w3601:errorcluster)  [unwired: 1 in, 1 out]
          }
          event Value Change {
            w3623 = T15."Enabled" ("Disabled")
            w3624 = FALSE ("StartMeas")
            # "Wave Shapes are only enabled when the instrument is AC. That has been taken care in the \"WaveEnable\" case of the \"Mode Change\" event."
            # "No need to \"Update\" here because values are passed directly to Device(s)Settings in the case select structure."
            # "Instr3 can only exist as itself in a few modes to be able to change its Wave Shapes."
            n1693 = event-data() -> ()  [unwired: 1 in, 6 out]
            n1694 = local read "Instr3"() -> (w3620:T2)
            n1695 = Unbundle By Name(w3620) -> ("Phases.A-Wave Shape"=w3619:u16, "Phases.B-Wave Shape"=w3618:u16, "Phases.C-Wave Shape"=w3615:u16)
            n1696 = local read "Mode"() -> (w3625:T8)
            n1697 = case shown="3..15" w3625 {
              tunnel: w3619 -> [_ w3632]
              tunnel: w3618 -> [_ w3630]
              tunnel: [w3628 w3631] -> w3616
              tunnel: w3617 -> [w3628 w3631]
              tunnel: [w3627 w3629] -> _
              tunnel: w3615 -> [w3627 w3629]
              frame Default {
                # "Instr3 is unavailable in the other modes."
              }
              frame 3..15 {
                # "Modes in which Instr3 can be accessed by the user as a single instrument."
                n1698 = local read "Device(s)Settings"() -> (w3634:T1)
                n1699 = Bundle By Name(cluster=w3634, "Instr3.Phases.A-Wave Shape"=w3632, "Instr3.Phases.B-Wave Shape"=w3630, "Instr3.Phases.C-Wave Shape"=w3629) -> (w3633:T1)
                n1700 = local write "Device(s)Settings"(w3633) -> ()
              }
            }
            n1701 = property on="btnSave" class="Bool"(error in=w3616, "DisabledEnum"=w3623) -> (error out=w3622:errorcluster)  [unwired: 1 in, 1 out]
            n1702 = property on="btnSaveAs" class="Bool"(error in=w3622, "DisabledEnum"=w3623) -> (error out=w3621:errorcluster)  [unwired: 1 in, 1 out]
          }
        }
        n1703 = Or(x=w406, y=w407) -> (x .or. y?=w408:bool)
      }
      "Changed" <- w25
      "Save As" <- w19
      n1704 = call <vilib>:"Clear Errors.vi"("error in (no error)"=w15) -> ("error out"=w14:errorcluster)  [unwired: 5 in, 1 out]
      n1705 = property class="VI"(error in=w14, "FP.Behavior"=T11."Default" ("Front Panel Window:Behavior")) -> (error out=w23:errorcluster)  [unwired: 1 in, 1 out]
      n1706 = property class="VI"(error in=w23, "FP.State"=T12."Closed" ("Front Panel Window:State")) -> ()  [unwired: 1 in, 2 out]
    }
    frame Error {
    }
  }
  "MyPluginsBase out" <- w3
  "error out" <- w2
